vi "Convert VIP License to SBOM Licenses with SPDX Lookup.vi"(6 "Additional Custom Aliases (empty = defaults only)":T1[](array[typedef]), 7 "SPDX License List (JSON) (\"\" = use built-in)":path, 8 "error in (no error)":errorcluster, 11 "VIP License Type in":string) -> (0 "error out":errorcluster, 3 "License(s) out":refnum<class "CycloneDX License.lvclass">[](array[class]))   [LabVIEW 2017, in "VIP SBOM Support.lvlib"]
doc: "Tries to match the VIP license information against the SPDX license types and returns a license with the SPDX license set. If there's no match, returns the license by name."
uses:
  VIP SBOM Support.lvlib
  CycloneDX/CycloneDX License/CycloneDX License.lvclass
  C:/LabVIEW Working Directory/VIPC Software BOM/CycloneDX/CycloneDX JSON/CycloneDX JSON.lvclass
  VIP License Alias.ctl
  c58193e4-58a4-4b31-ba60-9ddf4fa8120d.vi
  <vilib>/JDP Science/JSONtext/Find Item.vi
  <vilib>/JDP Science/JSONtext/String Subset.vi
  <vilib>/JDP Science/JSONtext/Parsing/Parse Full Path or Item Name.vi
  <vilib>/JDP Science/JSONtext/Next JSON Value.vi
  <vilib>/JDP Science/JSONtext/support/Error Cluster From Code.vi
  <vilib>/JDP Science/JSONtext/Offset/Find Item Locations by Path.vi
  <vilib>/JDP Science/JSONtext/JSON text to Variant.vi
  CycloneDX/CycloneDX JSON/CycloneDX JSON.lvclass
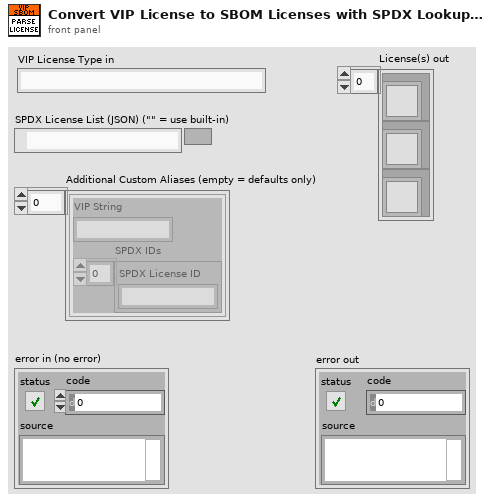
[diagram p1: front panel]
types:
  T1 = typedef "VIP SBOM Support.lvlib/VIP License Alias.ctl" = cluster{"VIP String":string, "SPDX IDs":string[]}
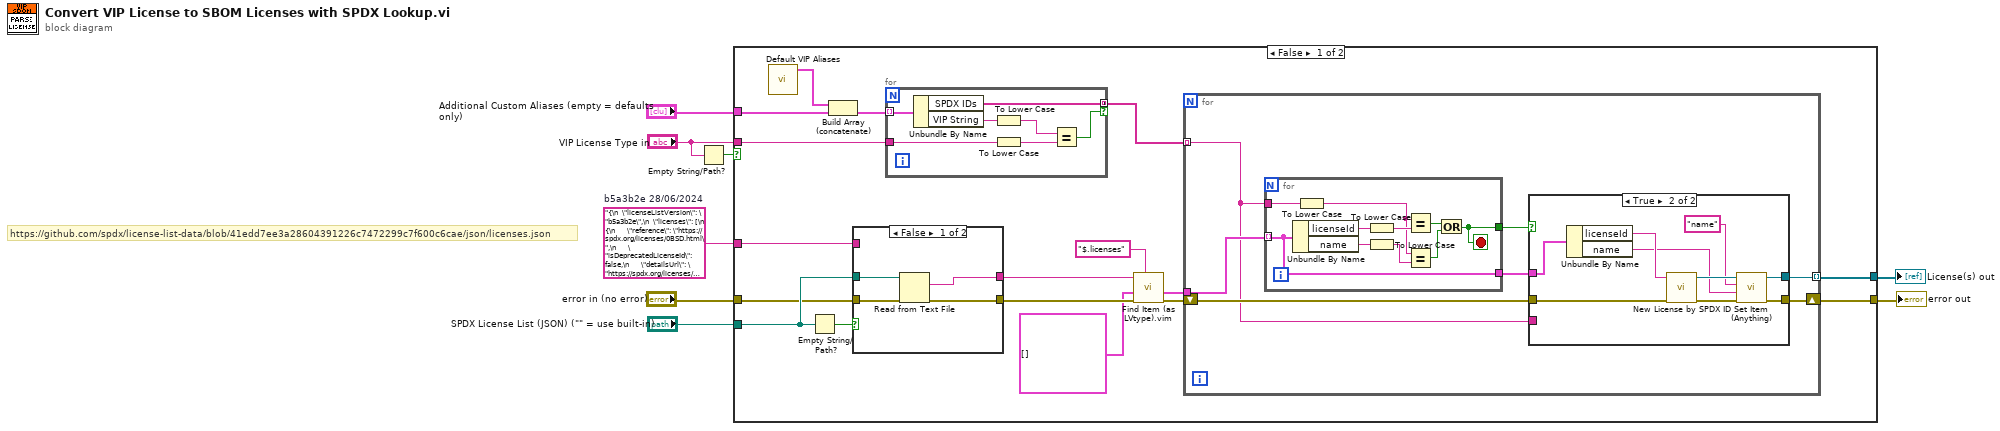
[diagram p0: block diagram]
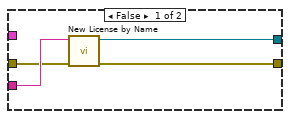
[diagram p3: hidden frame]
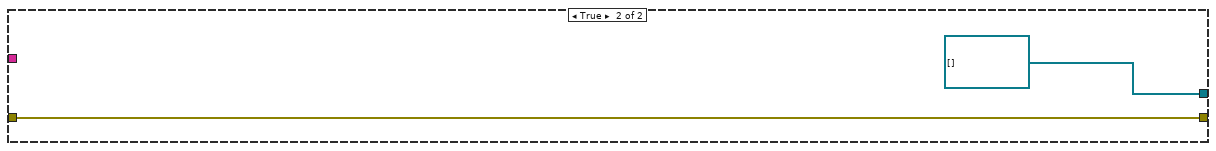
[diagram p4: hidden frame]
diagram:
  w2 = "{\n  \"licenseListVersion\": \"b5a3b2e\",\n  \"licenses\": [\n    {\n      \"reference\": \"https://spdx.org/licenses/0BSD.html\",\n      \"isDeprecatedLicenseId\": false,\n      \"detailsUrl\": \"https://spdx.org/licenses/0BSD.json\",\n      \"referenceNumber\": 430,\n      \"name\": \"BSD Zero Clause License\",\n      \"licenseId\": \"0BSD\",\n      \"seeAlso\": [\n        \"http://landley.net/toybox/license.html\",\n        \"https://opensource.org/licenses/0BSD\"\n      ],\n      \"isOsiApproved\": true\n    },\n    {\n      \"reference\": \"https://spdx.org/licenses/3D-Slicer-1.0.html\",\n      \"isDeprecatedLicenseId\": false,\n      \"detailsUrl\": \"https://spdx.org/licenses/3D-Slicer-1.0.json\",\n      \"referenceNumber\": 448,\n      \"name\": \"3D Slicer License v1.0\",\n      \"licenseId\": \"3D-Slicer-1.0\",\n      \"seeAlso\": [\n        \"https://slicer.org/LICENSE\",\n        \"https://github.com/Slicer/Slicer/blob/main/License.txt\"\n      ],\n      \"isOsiApproved\": false\n    },\n    {\n      \"reference\": \"https://spdx.org/licenses/AAL.html\",\n      \"isDeprecatedLicenseId\": false,\n      \"detailsUrl\": \"https://spdx.org/licenses/AAL.json\",\n      \"referenceNumber\": 515,\n      \"name\": \"Attribution Assurance License\",\n      \"licenseId\": \"AAL\",\n      \"seeAlso\": [\n        \"https://opensource.org/licenses/attribution\"\n      ],\n      \"isOsiApproved\": true\n    },\n    {\n      \"reference\": \"https://spdx.org/licenses/Abstyles.html\",\n      \"isDeprecatedLicenseId\": false,\n      \"detailsUrl\": \"https://spdx.org/licenses/Abstyles.json\",\n      \"referenceNumber\": 561,\n      \"name\": \"Abstyles License\",\n      \"licenseId\": \"Abstyles\",\n      \"seeAlso\": [\n        \"https://fedoraproject.org/wiki/Licensing/Abstyles\"\n      ],\n      \"isOsiApproved\": false\n    },\n    {\n      \"reference\": \"https://spdx.org/licenses/AdaCore-doc.html\",\n      \"isDeprecatedLicenseId\": false,\n      \"detailsUrl\": \"https://spdx.org/licenses/AdaCore-doc.json\",\n      \"referenceNumber\": 641,\n      \"name\": \"AdaCore Doc License\",\n      \"licenseId\": \"AdaCore-doc\",\n      \"seeAlso\": [\n        \"https://github.com/AdaCore/xmlada/blob/master/docs/index.rst\",\n        \"https://github.com/AdaCore/gnatcoll-core/blob/master/docs/index.rst\",\n        \"https://github.com/AdaCore/gnatcoll-db/blob/master/docs/index.rst\"\n      ],\n      \"isOsiApproved\": false\n    },\n    {\n      \"reference\": \"https://spdx.org/licenses/Adobe-2006.html\",\n      \"isDeprecatedLicenseId\": false,\n      \"detailsUrl\": \"https://spdx.org/licenses/Adobe-2006.json\",\n      \"referenceNumber\": 241,\n      \"name\": \"Adobe Systems Incorporated Source Code License Agreement\",\n      \"licenseId\": \"Adobe-2006\",\n      \"seeAlso\": [\n        \"https://fedoraproject.org/wiki/Licensing/AdobeLicense\"\n      ],\n      \"isOsiApproved\": false\n    },\n    {\n      \"reference\": \"https://spdx.org/licenses/Adobe-Display-PostScript.html\",\n      \"isDeprecatedLicenseId\": false,\n      \"detailsUrl\": \"https://spdx.org/licenses/Adobe-Display-PostScript.json\",\n      \"referenceNumber\": 198,\n      \"name\": \"Adobe Display PostScript License\",\n      \"licenseId\": \"Adobe-Display-PostScript\",\n      \"seeAlso\": [\n        \"https://gitlab.freedesktop.org/xorg/xserver/-/blob/master/COPYING?ref_type\\u003dheads#L752\"\n      ],\n      \"isOsiApproved\": false\n    },\n    {\n      \"reference\": \"https://spdx.org/licenses/Adobe-Glyph.html\",\n      \"isDeprecatedLicenseId\": false,\n      \"detailsUrl\": \"https://spdx.org/licenses/Adobe-Glyph.json\",\n      \"referenceNumber\": 506,\n      \"name\": \"Adobe Glyph List License\",\n      \"licenseId\": \"Adobe-Glyph\",\n      \"seeAlso\": [\n        \"https://fedoraproject.org/wiki/Licensing/MIT#AdobeGlyph\"\n      ],\n      \"isOsiApproved\": false\n    },\n    {\n      \"reference\": \"https://spdx.org/licenses/Adobe-Utopia.html\",\n      \"isDeprecatedLicenseId\": false,\n      \"detailsUrl\": \"https://spdx.org/licenses/Adobe-Utopia.json\",\n      \"referenceNumber\": 519,\n      \"name\": \"Adobe Utopia Font License\",\n      \"licenseId\": \"Adobe-Utopia\",\n      \"seeAlso\": [\n        \"https://gitlab.freedesktop.org/xorg/font/adobe-utopia-100dpi/-/blob/master/COPYING?ref_type\\u003dheads\"\n      ],\n      \"isOsiApproved\": false\n    },\n    {\n      \"reference\": \"https://spdx.org/licenses/ADSL.html\",\n      \"isDeprecatedLicenseId\": false,\n      \"detailsUrl\": \"https://spdx.org/licenses/ADSL.json\",\n      \"referenceNumber\": 266,\n      \"name\": \"Amazon Digital Services License\",\n      \"licenseId\": \"ADSL\",\n      \"seeAlso\": [\n        \"https://fedoraproject.org/wiki/Licensing/AmazonDigitalServicesLicense\"\n      ],\n      \"isOsiApproved\": false\n    },\n    {\n      \"reference\": \"https://spdx.org/licenses/AFL-1.1.html\",\n      \"isDeprecatedLicenseId\": false,\n      \"detailsUrl\": \"https://spdx.org/licenses/AFL-1.1.json\",\n      \"referenceNumber\": 120,\n      \"name\": \"Academic Free License v1.1\",\n      \"licenseId\": \"AFL-1.1\",\n      \"seeAlso\": [\n        \"http://opensource.linux-mirror.org/licenses/afl-1.1.txt\",\n        \"http://wayback.archive.org/web/20021004124254/http://www.opensource.org/licenses/academic.php\"\n      ],\n      \"isOsiApproved\": true,\n      \"isFsfLibre\": true\n    },\n    {\n      \"reference\": \"https://spdx.org/licenses/AFL-1.2.html\",\n      \"isDeprecatedLicenseId\": false,\n      \"detailsUrl\": \"https://spdx.org/licenses/AFL-1.2.json\",\n      \"referenceNumber\": 127,\n      \"name\": \"Academic Free License v1.2\",\n      \"licenseId\": \"AFL-1.2\",\n      \"seeAlso\": [\n        \"http://opensource.linux-mirror.org/licenses/afl-1.2.txt\",\n        \"http://wayback.archive.org/web/20021204204652/http://www.opensource.org/licenses/academic.php\"\n      ],\n      \"isOsiApproved\": true,\n      \"isFsfLibre\": true\n    },\n    {\n      \"reference\": \"https://spdx.org/licenses/AFL-2.0.html\",\n      \"isDeprecatedLicenseId\": false,\n      \"detailsUrl\": \"https://spdx.org/licenses/AFL-2.0.json\",\n      \"referenceNumber\": 371,\n      \"name\": \"Academic Free License v2.0\",\n      \"licenseId\": \"AFL-2.0\",\n      \"seeAlso\": [\n        \"http://wayback.archive.org/web/20060924134533/http://www.opensource.org/licenses/afl-2.0.txt\"\n      ],\n      \"isOsiApproved\": true,\n      \"isFsfLibre\": true\n    },\n    {\n      \"reference\": \"https://spdx.org/licenses/AFL-2.1.html\",\n      \"isDeprecatedLicenseId\": false,\n      \"detailsUrl\": \"https://spdx.org/licenses/AFL-2.1.json\",\n      \"referenceNumber\": 355,\n      \"name\": \"Academic Free License v2.1\",\n      \"licenseId\": \"AFL-2.1\",\n      \"seeAlso\": [\n        \"http://opensource.linux-mirror.org/licenses/afl-2.1.txt\"\n      ],\n      \"isOsiApproved\": true,\n      \"isFsfLibre\": true\n    },\n    {\n      \"reference\": \"https://spdx.org/licenses/AFL-3.0.html\",\n      \"isDeprecatedLicenseId\": false,\n      \"detailsUrl\": \"https://spdx.org/licenses/AFL-3.0.json\",\n      \"referenceNumber\": 169,\n      \"name\": \"Academic Free License v3.0\",\n      \"licenseId\": \"AFL-3.0\",\n      \"seeAlso\": [\n        \"http://www.rosenlaw.com/AFL3.0.htm\",\n        \"https://opensource.org/licenses/afl-3.0\"\n      ],\n      \"isOsiApproved\": true,\n      \"isFsfLibre\": true\n    },\n    {\n      \"reference\": \"https://spdx.org/licenses/Afmparse.html\",\n      \"isDeprecatedLicenseId\": false,\n      \"detailsUrl\": \"https://spdx.org/licenses/Afmparse.json\",\n      \"referenceNumber\": 485,\n      \"name\": \"Afmparse License\",\n      \"licenseId\": \"Afmparse\",\n      \"seeAlso\": [\n        \"https://fedoraproject.org/wiki/Licensing/Afmparse\"\n      ],\n      \"isOsiApproved\": false\n    },\n    {\n      \"reference\": \"https://spdx.org/licenses/AGPL-1.0.html\",\n      \"isDeprecatedLicenseId\": true,\n      \"detailsUrl\": \"https://spdx.org/licenses/AGPL-1.0.json\",\n      \"referenceNumber\": 251,\n      \"name\": \"Affero General Public License v1.0\",\n      \"licenseId\": \"AGPL-1.0\",\n      \"seeAlso\": [\n        \"http://www.affero.org/oagpl.html\"\n      ],\n      \"isOsiApproved\": false,\n      \"isFsfLibre\": true\n    },\n    {\n      \"reference\": \"https://spdx.org/licenses/AGPL-1.0-only.html\",\n      \"isDeprecatedLicenseId\": false,\n      \"detailsUrl\": \"https://spdx.org/licenses/AGPL-1.0-only.json\",\n      \"referenceNumber\": 552,\n      \"name\": \"Affero General Public License v1.0 only\",\n      \"licenseId\": \"AGPL-1.0-only\",\n      \"seeAlso\": [\n        \"http://www.affero.org/oagpl.html\"\n      ],\n      \"isOsiApproved\": false\n    },\n    {\n      \"reference\": \"https://spdx.org/licenses/AGPL-1.0-or-later.html\",\n      \"isDeprecatedLicenseId\": false,\n      \"detailsUrl\": \"https://spdx.org/licenses/AGPL-1.0-or-later.json\",\n      \"referenceNumber\": 608,\n      \"name\": \"Affero General Public License v1.0 or later\",\n      \"licenseId\": \"AGPL-1.0-or-later\",\n      \"seeAlso\": [\n        \"http://www.affero.org/oagpl.html\"\n      ],\n      \"isOsiApproved\": false\n    },\n    {\n      \"reference\": \"https://spdx.org/licenses/AGPL-3.0.html\",\n      \"isDeprecatedLicenseId\": true,\n      \"detailsUrl\": \"https://spdx.org/licenses/AGPL-3.0.json\",\n      \"referenceNumber\": 213,\n      \"name\": \"GNU Affero General Public License v3.0\",\n      \"licenseId\": \"AGPL-3.0\",\n      \"seeAlso\": [\n        \"https://www.gnu.org/licenses/agpl.txt\",\n        \"https://opensource.org/licenses/AGPL-3.0\"\n      ],\n      \"isOsiApproved\": true,\n      \"isFsfLibre\": true\n    },\n    {\n      \"reference\": \"https://spdx.org/licenses/AGPL-3.0-only.html\",\n      \"isDeprecatedLicenseId\": false,\n      \"detailsUrl\": \"https://spdx.org/licenses/AGPL-3.0-only.json\",\n      \"referenceNumber\": 2,\n      \"name\": \"GNU Affero General Public License v3.0 only\",\n      \"licenseId\": \"AGPL-3.0-only\",\n      \"seeAlso\": [\n        \"https://www.gnu.org/licenses/agpl.txt\",\n        \"https://opensource.org/licenses/AGPL-3.0\"\n      ],\n      \"isOsiApproved\": true,\n      \"isFsfLibre\": true\n    },\n    {\n      \"reference\": \"https://spdx.org/licenses/AGPL-3.0-or-later.html\",\n      \"isDeprecatedLicenseId\": false,\n      \"detailsUrl\": \"https://spdx.org/licenses/AGPL-3.0-or-later.json\",\n      \"referenceNumber\": 390,\n      \"name\": \"GNU Affero General Public License v3.0 or later\",\n      \"licenseId\": \"AGPL-3.0-or-later\",\n      \"seeAlso\": [\n        \"https://www.gnu.org/licenses/agpl.txt\",\n        \"https://opensource.org/licenses/AGPL-3.0\"\n      ],\n      \"isOsiApproved\": true,\n      \"isFsfLibre\": true\n    },\n    {\n      \"reference\": \"https://spdx.org/licenses/Aladdin.html\",\n      \"isDeprecatedLicenseId\": false,\n      \"detailsUrl\": \"https://spdx.org/licenses/Aladdin.json\",\n      \"referenceNumber\": 272,\n      \"name\": \"Aladdin Free Public License\",\n      \"licenseId\": \"Aladdin\",\n      \"seeAlso\": [\n        \"http://pages.cs.wisc.edu/~ghost/doc/AFPL/6.01/Public.htm\"\n      ],\n      \"isOsiApproved\": false,\n      \"isFsfLibre\": false\n    },\n    {\n      \"reference\": \"https://spdx.org/licenses/AMD-newlib.html\",\n      \"isDeprecatedLicenseId\": false,\n      \"detailsUrl\": \"https://spdx.org/licenses/AMD-newlib.json\",\n      \"referenceNumber\": 536,\n      \"name\": \"AMD newlib License\",\n      \"licenseId\": \"AMD-newlib\",\n      \"seeAlso\": [\n        \"https://sourceware.org/git/?p\\u003dnewlib-cygwin.git;a\\u003dblob;f\\u003dnewlib/libc/sys/a29khif/_close.S;h\\u003d04f52ae00de1dafbd9055ad8d73c5c697a3aae7f;hb\\u003dHEAD\"\n      ],\n      \"isOsiApproved\": false\n    },\n    {\n      \"reference\": \"https://spdx.org/licenses/AMDPLPA.html\",\n      \"isDeprecatedLicenseId\": false,\n      \"detailsUrl\": \"https://spdx.org/licenses/AMDPLPA.json\",\n      \"referenceNumber\": 440,\n      \"name\": \"AMD\\u0027s plpa_map.c License\",\n      \"licenseId\": \"AMDPLPA\",\n      \"seeAlso\": [\n        \"https://fedoraproject.org/wiki/Licensing/AMD_plpa_map_License\"\n      ],\n      \"isOsiApproved\": false\n    },\n    {\n      \"reference\": \"https://spdx.org/licenses/AML.html\",\n      \"isDeprecatedLicenseId\": false,\n      \"detailsUrl\": \"https://spdx.org/licenses/AML.json\",\n      \"referenceNumber\": 361,\n      \"name\": \"Apple MIT License\",\n      \"licenseId\": \"AML\",\n      \"seeAlso\": [\n        \"https://fedoraproject.org/wiki/Licensing/Apple_MIT_License\"\n      ],\n      \"isOsiApproved\": false\n    },\n    {\n      \"reference\": \"https://spdx.org/licenses/AML-glslang.html\",\n      \"isDeprecatedLicenseId\": false,\n      \"detailsUrl\": \"https://spdx.org/licenses/AML-glslang.json\",\n      \"referenceNumber\": 151,\n      \"name\": \"AML glslang variant License\",\n      \"licenseId\": \"AML-glslang\",\n      \"seeAlso\": [\n        \"https://github.com/KhronosGroup/glslang/blob/main/LICENSE.txt#L949\",\n        \"https://docs.omniverse.nvidia.com/install-guide/latest/common/licenses.html\"\n      ],\n      \"isOsiApproved\": false\n    },\n    {\n      \"reference\": \"https://spdx.org/licenses/AMPAS.html\",\n      \"isDeprecatedLicenseId\": false,\n      \"detailsUrl\": \"https://spdx.org/licenses/AMPAS.json\",\n      \"referenceNumber\": 276,\n      \"name\": \"Academy of Motion Picture Arts and Sciences BSD\",\n      \"licenseId\": \"AMPAS\",\n      \"seeAlso\": [\n        \"https://fedoraproject.org/wiki/Licensing/BSD#AMPASBSD\"\n      ],\n      \"isOsiApproved\": false\n    },\n    {\n      \"reference\": \"https://spdx.org/licenses/ANTLR-PD.html\",\n      \"isDeprecatedLicenseId\": false,\n      \"detailsUrl\": \"https://spdx.org/licenses/ANTLR-PD.json\",\n      \"referenceNumber\": 370,\n      \"name\": \"ANTLR Software Rights Notice\",\n      \"licenseId\": \"ANTLR-PD\",\n      \"seeAlso\": [\n        \"http://www.antlr2.org/license.html\"\n      ],\n      \"isOsiApproved\": false\n    },\n    {\n      \"reference\": \"https://spdx.org/licenses/ANTLR-PD-fallback.html\",\n      \"isDeprecatedLicenseId\": false,\n      \"detailsUrl\": \"https://spdx.org/licenses/ANTLR-PD-fallback.json\",\n      \"referenceNumber\": 10,\n      \"name\": \"ANTLR Software Rights Notice with license fallback\",\n      \"licenseId\": \"ANTLR-PD-fallback\",\n      \"seeAlso\": [\n        \"http://www.antlr2.org/license.html\"\n      ],\n      \"isOsiApproved\": false\n    },\n    {\n      \"reference\": \"https://spdx.org/licenses/any-OSI.html\",\n      \"isDeprecatedLicenseId\": false,\n      \"detailsUrl\": \"https://spdx.org/licenses/any-OSI.json\",\n      \"referenceNumber\": 297,\n      \"name\": \"Any OSI License\",\n      \"licenseId\": \"any-OSI\",\n      \"seeAlso\": [\n        \"https://metacpan.org/pod/Exporter::Tidy#LICENSE\"\n      ],\n      \"isOsiApproved\": false\n    },\n    {\n      \"reference\": \"https://spdx.org/licenses/Apache-1.0.html\",\n      \"isDeprecatedLicenseId\": false,\n      \"detailsUrl\": \"https://spdx.org/licenses/Apache-1.0.json\",\n      \"referenceNumber\": 521,\n      \"name\": \"Apache License 1.0\",\n      \"licenseId\": \"Apache-1.0\",\n      \"seeAlso\": [\n        \"http://www.apache.org/licenses/LICENSE-1.0\"\n      ],\n      \"isOsiApproved\": false,\n      \"isFsfLibre\": true\n    },\n    {\n      \"reference\": \"https://spdx.org/licenses/Apache-1.1.html\",\n      \"isDeprecatedLicenseId\": false,\n      \"detailsUrl\": \"https://spdx.org/licenses/Apache-1.1.json\",\n      \"referenceNumber\": 452,\n      \"name\": \"Apache License 1.1\",\n      \"licenseId\": \"Apache-1.1\",\n      \"seeAlso\": [\n        \"http://apache.org/licenses/LICENSE-1.1\",\n        \"https://opensource.org/licenses/Apache-1.1\"\n      ],\n      \"isOsiApproved\": true,\n      \"isFsfLibre\": true\n    },\n    {\n      \"reference\": \"https://spdx.org/licenses/Apache-2.0.html\",\n      \"isDeprecatedLicenseId\": false,\n      \"detailsUrl\": \"https://spdx.org/licenses/Apache-2.0.json\",\n      \"referenceNumber\": 168,\n      \"name\": \"Apache License 2.0\",\n      \"licenseId\": \"Apache-2.0\",\n      \"seeAlso\": [\n        \"https://www.apache.org/licenses/LICENSE-2.0\",\n        \"https://opensource.org/licenses/Apache-2.0\"\n      ],\n      \"isOsiApproved\": true,\n      \"isFsfLibre\": true\n    },\n    {\n      \"reference\": \"https://spdx.org/licenses/APAFML.html\",\n      \"isDeprecatedLicenseId\": false,\n      \"detailsUrl\": \"https://spdx.org/licenses/APAFML.json\",\n      \"referenceNumber\": 456,\n      \"name\": \"Adobe Postscript AFM License\",\n      \"licenseId\": \"APAFML\",\n      \"seeAlso\": [\n        \"https://fedoraproject.org/wiki/Licensing/AdobePostscriptAFM\"\n      ],\n      \"isOsiApproved\": false\n    },\n    {\n      \"reference\": \"https://spdx.org/licenses/APL-1.0.html\",\n      \"isDeprecatedLicenseId\": false,\n      \"detailsUrl\": \"https://spdx.org/licenses/APL-1.0.json\",\n      \"referenceNumber\": 58,\n      \"name\": \"Adaptive Public License 1.0\",\n      \"licenseId\": \"APL-1.0\",\n      \"seeAlso\": [\n        \"https://opensource.org/licenses/APL-1.0\"\n      ],\n      \"isOsiApproved\": true\n    },\n    {\n      \"reference\": \"https://spdx.org/licenses/App-s2p.html\",\n      \"isDeprecatedLicenseId\": false,\n      \"detailsUrl\": \"https://spdx.org/licenses/App-s2p.json\",\n      \"referenceNumber\": 186,\n      \"name\": \"App::s2p License\",\n      \"licenseId\": \"App-s2p\",\n      \"seeAlso\": [\n        \"https://fedoraproject.org/wiki/Licensing/App-s2p\"\n      ],\n      \"isOsiApproved\": false\n    },\n    {\n      \"reference\": \"https://spdx.org/licenses/APSL-1.0.html\",\n      \"isDeprecatedLicenseId\": false,\n      \"detailsUrl\": \"https://spdx.org/licenses/APSL-1.0.json\",\n      \"referenceNumber\": 166,\n      \"name\": \"Apple Public Source License 1.0\",\n      \"licenseId\": \"APSL-1.0\",\n      \"seeAlso\": [\n        \"https://fedoraproject.org/wiki/Licensing/Apple_Public_Source_License_1.0\"\n      ],\n      \"isOsiApproved\": true,\n      \"isFsfLibre\": false\n    },\n    {\n      \"reference\": \"https://spdx.org/licenses/APSL-1.1.html\",\n      \"isDeprecatedLicenseId\": false,\n      \"detailsUrl\": \"https://spdx.org/licenses/APSL-1.1.json\",\n      \"referenceNumber\": 114,\n      \"name\": \"Apple Public Source License 1.1\",\n      \"licenseId\": \"APSL-1.1\",\n      \"seeAlso\": [\n        \"http://www.opensource.apple.com/source/IOSerialFamily/IOSerialFamily-7/APPLE_LICENSE\"\n      ],\n      \"isOsiApproved\": true\n    },\n    {\n      \"reference\": \"https://spdx.org/licenses/APSL-1.2.html\",\n      \"isDeprecatedLicenseId\": false,\n      \"detailsUrl\": \"https://spdx.org/licenses/APSL-1.2.json\",\n      \"referenceNumber\": 393,\n      \"name\": \"Apple Public Source License 1.2\",\n      \"licenseId\": \"APSL-1.2\",\n      \"seeAlso\": [\n        \"http://www.samurajdata.se/opensource/mirror/licenses/apsl.php\"\n      ],\n      \"isOsiApproved\": true\n    },\n    {\n      \"reference\": \"https://spdx.org/licenses/APSL-2.0.html\",\n      \"isDeprecatedLicenseId\": false,\n      \"detailsUrl\": \"https://spdx.org/licenses/APSL-2.0.json\",\n      \"referenceNumber\": 267,\n      \"name\": \"Apple Public Source License 2.0\",\n      \"licenseId\": \"APSL-2.0\",\n      \"seeAlso\": [\n        \"http://www.opensource.apple.com/license/apsl/\"\n      ],\n      \"isOsiApproved\": true,\n      \"isFsfLibre\": true\n    },\n    {\n      \"reference\": \"https://spdx.org/licenses/Arphic-1999.html\",\n      \"isDeprecatedLicenseId\": false,\n      \"detailsUrl\": \"https://spdx.org/licenses/Arphic-1999.json\",\n      \"referenceNumber\": 117,\n      \"name\": \"Arphic Public License\",\n      \"licenseId\": \"Arphic-1999\",\n      \"seeAlso\": [\n        \"http://ftp.gnu.org/gnu/non-gnu/chinese-fonts-truetype/LICENSE\"\n      ],\n      \"isOsiApproved\": false\n    },\n    {\n      \"reference\": \"https://spdx.org/licenses/Artistic-1.0.html\",\n      \"isDeprecatedLicenseId\": false,\n      \"detailsUrl\": \"https://spdx.org/licenses/Artistic-1.0.json\",\n      \"referenceNumber\": 468,\n      \"name\": \"Artistic License 1.0\",\n      \"licenseId\": \"Artistic-1.0\",\n      \"seeAlso\": [\n        \"https://opensource.org/licenses/Artistic-1.0\"\n      ],\n      \"isOsiApproved\": true,\n      \"isFsfLibre\": false\n    },\n    {\n      \"reference\": \"https://spdx.org/licenses/Artistic-1.0-cl8.html\",\n      \"isDeprecatedLicenseId\": false,\n      \"detailsUrl\": \"https://spdx.org/licenses/Artistic-1.0-cl8.json\",\n      \"referenceNumber\": 507,\n      \"name\": \"Artistic License 1.0 w/clause 8\",\n      \"licenseId\": \"Artistic-1.0-cl8\",\n      \"seeAlso\": [\n        \"https://opensource.org/licenses/Artistic-1.0\"\n      ],\n      \"isOsiApproved\": true\n    },\n    {\n      \"reference\": \"https://spdx.org/licenses/Artistic-1.0-Perl.html\",\n      \"isDeprecatedLicenseId\": false,\n      \"detailsUrl\": \"https://spdx.org/licenses/Artistic-1.0-Perl.json\",\n      \"referenceNumber\": 574,\n      \"name\": \"Artistic License 1.0 (Perl)\",\n      \"licenseId\": \"Artistic-1.0-Perl\",\n      \"seeAlso\": [\n        \"http://dev.perl.org/licenses/artistic.html\"\n      ],\n      \"isOsiApproved\": true\n    },\n    {\n      \"reference\": \"https://spdx.org/licenses/Artistic-2.0.html\",\n      \"isDeprecatedLicenseId\": false,\n      \"detailsUrl\": \"https://spdx.org/licenses/Artistic-2.0.json\",\n      \"referenceNumber\": 232,\n      \"name\": \"Artistic License 2.0\",\n      \"licenseId\": \"Artistic-2.0\",\n      \"seeAlso\": [\n        \"http://www.perlfoundation.org/artistic_license_2_0\",\n        \"https://www.perlfoundation.org/artistic-license-20.html\",\n        \"https://opensource.org/licenses/artistic-license-2.0\"\n      ],\n      \"isOsiApproved\": true,\n      \"isFsfLibre\": true\n    },\n    {\n      \"reference\": \"https://spdx.org/licenses/ASWF-Digital-Assets-1.0.html\",\n      \"isDeprecatedLicenseId\": false,\n      \"detailsUrl\": \"https://spdx.org/licenses/ASWF-Digital-Assets-1.0.json\",\n      \"referenceNumber\": 577,\n      \"name\": \"ASWF Digital Assets License version 1.0\",\n      \"licenseId\": \"ASWF-Digital-Assets-1.0\",\n      \"seeAlso\": [\n        \"https://github.com/AcademySoftwareFoundation/foundation/blob/main/digital_assets/aswf_digital_assets_license_v1.0.txt\"\n      ],\n      \"isOsiApproved\": false\n    },\n    {\n      \"reference\": \"https://spdx.org/licenses/ASWF-Digital-Assets-1.1.html\",\n      \"isDeprecatedLicenseId\": false,\n      \"detailsUrl\": \"https://spdx.org/licenses/ASWF-Digital-Assets-1.1.json\",\n      \"referenceNumber\": 508,\n      \"name\": \"ASWF Digital Assets License 1.1\",\n      \"licenseId\": \"ASWF-Digital-Assets-1.1\",\n      \"seeAlso\": [\n        \"https://github.com/AcademySoftwareFoundation/foundation/blob/main/digital_assets/aswf_digital_assets_license_v1.1.txt\"\n      ],\n      \"isOsiApproved\": false\n    },\n    {\n      \"reference\": \"https://spdx.org/licenses/Baekmuk.html\",\n      \"isDeprecatedLicenseId\": false,\n      \"detailsUrl\": \"https://spdx.org/licenses/Baekmuk.json\",\n      \"referenceNumber\": 504,\n      \"name\": \"Baekmuk License\",\n      \"licenseId\": \"Baekmuk\",\n      \"seeAlso\": [\n        \"https://fedoraproject.org/wiki/Licensing:Baekmuk?rd\\u003dLicensing/Baekmuk\"\n      ],\n      \"isOsiApproved\": false\n    },\n    {\n      \"reference\": \"https://spdx.org/licenses/Bahyph.html\",\n      \"isDeprecatedLicenseId\": false,\n      \"detailsUrl\": \"https://spdx.org/licenses/Bahyph.json\",\n      \"referenceNumber\": 604,\n      \"name\": \"Bahyph License\",\n      \"licenseId\": \"Bahyph\",\n      \"seeAlso\": [\n        \"https://fedoraproject.org/wiki/Licensing/Bahyph\"\n      ],\n      \"isOsiApproved\": false\n    },\n    {\n      \"reference\": \"https://spdx.org/licenses/Barr.html\",\n      \"isDeprecatedLicenseId\": false,\n      \"detailsUrl\": \"https://spdx.org/licenses/Barr.json\",\n      \"referenceNumber\": 136,\n      \"name\": \"Barr License\",\n      \"licenseId\": \"Barr\",\n      \"seeAlso\": [\n        \"https://fedoraproject.org/wiki/Licensing/Barr\"\n      ],\n      \"isOsiApproved\": false\n    },\n    {\n      \"reference\": \"https://spdx.org/licenses/bcrypt-Solar-Designer.html\",\n      \"isDeprecatedLicenseId\": false,\n      \"detailsUrl\": \"https://spdx.org/licenses/bcrypt-Solar-Designer.json\",\n      \"referenceNumber\": 402,\n      \"name\": \"bcrypt Solar Designer License\",\n      \"licenseId\": \"bcrypt-Solar-Designer\",\n      \"seeAlso\": [\n        \"https://github.com/bcrypt-ruby/bcrypt-ruby/blob/master/ext/mri/crypt_blowfish.c\"\n      ],\n      \"isOsiApproved\": false\n    },\n    {\n      \"reference\": \"https://spdx.org/licenses/Beerware.html\",\n      \"isDeprecatedLicenseId\": false,\n      \"detailsUrl\": \"https://spdx.org/licenses/Beerware.json\",\n      \"referenceNumber\": 303,\n      \"name\": \"Beerware License\",\n      \"licenseId\": \"Beerware\",\n      \"seeAlso\": [\n        \"https://fedoraproject.org/wiki/Licensing/Beerware\",\n        \"https://people.freebsd.org/~phk/\"\n      ],\n      \"isOsiApproved\": false\n    },\n    {\n      \"reference\": \"https://spdx.org/licenses/Bitstream-Charter.html\",\n      \"isDeprecatedLicenseId\": false,\n      \"detailsUrl\": \"https://spdx.org/licenses/Bitstream-Charter.json\",\n      \"referenceNumber\": 441,\n      \"name\": \"Bitstream Charter Font License\",\n      \"licenseId\": \"Bitstream-Charter\",\n      \"seeAlso\": [\n        \"https://fedoraproject.org/wiki/Licensing/Charter#License_Text\",\n        \"https://raw.githubusercontent.com/blackhole89/notekit/master/data/fonts/Charter%20license.txt\"\n      ],\n      \"isOsiApproved\": false\n    },\n    {\n      \"reference\": \"https://spdx.org/licenses/Bitstream-Vera.html\",\n      \"isDeprecatedLicenseId\": false,\n      \"detailsUrl\": \"https://spdx.org/licenses/Bitstream-Vera.json\",\n      \"referenceNumber\": 579,\n      \"name\": \"Bitstream Vera Font License\",\n      \"licenseId\": \"Bitstream-Vera\",\n      \"seeAlso\": [\n        \"https://web.archive.org/web/20080207013128/http://www.gnome.org/fonts/\",\n        \"https://docubrain.com/sites/default/files/licenses/bitstream-vera.html\"\n      ],\n      \"isOsiApproved\": false\n    },\n    {\n      \"reference\": \"https://spdx.org/licenses/BitTorrent-1.0.html\",\n      \"isDeprecatedLicenseId\": false,\n      \"detailsUrl\": \"https://spdx.org/licenses/BitTorrent-1.0.json\",\n      \"referenceNumber\": 47,\n      \"name\": \"BitTorrent Open Source License v1.0\",\n      \"licenseId\": \"BitTorrent-1.0\",\n      \"seeAlso\": [\n        \"http://sources.gentoo.org/cgi-bin/viewvc.cgi/gentoo-x86/licenses/BitTorrent?r1\\u003d1.1\\u0026r2\\u003d1.1.1.1\\u0026diff_format\\u003ds\"\n      ],\n      \"isOsiApproved\": false\n    },\n    {\n      \"reference\": \"https://spdx.org/licenses/BitTorrent-1.1.html\",\n      \"isDeprecatedLicenseId\": false,\n      \"detailsUrl\": \"https://spdx.org/licenses/BitTorrent-1.1.json\",\n      \"referenceNumber\": 387,\n      \"name\": \"BitTorrent Open Source License v1.1\",\n      \"licenseId\": \"BitTorrent-1.1\",\n      \"seeAlso\": [\n        \"http://directory.fsf.org/wiki/License:BitTorrentOSL1.1\"\n      ],\n      \"isOsiApproved\": false,\n      \"isFsfLibre\": true\n    },\n    {\n      \"reference\": \"https://spdx.org/licenses/blessing.html\",\n      \"isDeprecatedLicenseId\": false,\n      \"detailsUrl\": \"https://spdx.org/licenses/blessing.json\",\n      \"referenceNumber\": 21,\n      \"name\": \"SQLite Blessing\",\n      \"licenseId\": \"blessing\",\n      \"seeAlso\": [\n        \"https://www.sqlite.org/src/artifact/e33a4df7e32d742a?ln\\u003d4-9\",\n        \"https://sqlite.org/src/artifact/df5091916dbb40e6\"\n      ],\n      \"isOsiApproved\": false\n    },\n    {\n      \"reference\": \"https://spdx.org/licenses/BlueOak-1.0.0.html\",\n      \"isDeprecatedLicenseId\": false,\n      \"detailsUrl\": \"https://spdx.org/licenses/BlueOak-1.0.0.json\",\n      \"referenceNumber\": 620,\n      \"name\": \"Blue Oak Model License 1.0.0\",\n      \"licenseId\": \"BlueOak-1.0.0\",\n      \"seeAlso\": [\n        \"https://blueoakcouncil.org/license/1.0.0\"\n      ],\n      \"isOsiApproved\": true\n    },\n    {\n      \"reference\": \"https://spdx.org/licenses/Boehm-GC.html\",\n      \"isDeprecatedLicenseId\": false,\n      \"detailsUrl\": \"https://spdx.org/licenses/Boehm-GC.json\",\n      \"referenceNumber\": 530,\n      \"name\": \"Boehm-Demers-Weiser GC License\",\n      \"licenseId\": \"Boehm-GC\",\n      \"seeAlso\": [\n        \"https://fedoraproject.org/wiki/Licensing:MIT#Another_Minimal_variant_(found_in_libatomic_ops)\",\n        \"https://github.com/uim/libgcroots/blob/master/COPYING\",\n        \"https://github.com/ivmai/libatomic_ops/blob/master/LICENSE\"\n      ],\n      \"isOsiApproved\": false\n    },\n    {\n      \"reference\": \"https://spdx.org/licenses/Borceux.html\",\n      \"isDeprecatedLicenseId\": false,\n      \"detailsUrl\": \"https://spdx.org/licenses/Borceux.json\",\n      \"referenceNumber\": 190,\n      \"name\": \"Borceux license\",\n      \"licenseId\": \"Borceux\",\n      \"seeAlso\": [\n        \"https://fedoraproject.org/wiki/Licensing/Borceux\"\n      ],\n      \"isOsiApproved\": false\n    },\n    {\n      \"reference\": \"https://spdx.org/licenses/Brian-Gladman-2-Clause.html\",\n      \"isDeprecatedLicenseId\": false,\n      \"detailsUrl\": \"https://spdx.org/licenses/Brian-Gladman-2-Clause.json\",\n      \"referenceNumber\": 52,\n      \"name\": \"Brian Gladman 2-Clause License\",\n      \"licenseId\": \"Brian-Gladman-2-Clause\",\n      \"seeAlso\": [\n        \"https://github.com/krb5/krb5/blob/krb5-1.21.2-final/NOTICE#L140-L156\",\n        \"https://web.mit.edu/kerberos/krb5-1.21/doc/mitK5license.html\"\n      ],\n      \"isOsiApproved\": false\n    },\n    {\n      \"reference\": \"https://spdx.org/licenses/Brian-Gladman-3-Clause.html\",\n      \"isDeprecatedLicenseId\": false,\n      \"detailsUrl\": \"https://spdx.org/licenses/Brian-Gladman-3-Clause.json\",\n      \"referenceNumber\": 201,\n      \"name\": \"Brian Gladman 3-Clause License\",\n      \"licenseId\": \"Brian-Gladman-3-Clause\",\n      \"seeAlso\": [\n        \"https://github.com/SWI-Prolog/packages-clib/blob/master/sha1/brg_endian.h\"\n      ],\n      \"isOsiApproved\": false\n    },\n    {\n      \"reference\": \"https://spdx.org/licenses/BSD-1-Clause.html\",\n      \"isDeprecatedLicenseId\": false,\n      \"detailsUrl\": \"https://spdx.org/licenses/BSD-1-Clause.json\",\n      \"referenceNumber\": 404,\n      \"name\": \"BSD 1-Clause License\",\n      \"licenseId\": \"BSD-1-Clause\",\n      \"seeAlso\": [\n        \"https://svnweb.freebsd.org/base/head/include/ifaddrs.h?revision\\u003d326823\"\n      ],\n      \"isOsiApproved\": true\n    },\n    {\n      \"reference\": \"https://spdx.org/licenses/BSD-2-Clause.html\",\n      \"isDeprecatedLicenseId\": false,\n      \"detailsUrl\": \"https://spdx.org/licenses/BSD-2-Clause.json\",\n      \"referenceNumber\": 425,\n      \"name\": \"BSD 2-Clause \\\"Simplified\\\" License\",\n      \"licenseId\": \"BSD-2-Clause\",\n      \"seeAlso\": [\n        \"https://opensource.org/licenses/BSD-2-Clause\"\n      ],\n      \"isOsiApproved\": true,\n      \"isFsfLibre\": true\n    },\n    {\n      \"reference\": \"https://spdx.org/licenses/BSD-2-Clause-Darwin.html\",\n      \"isDeprecatedLicenseId\": false,\n      \"detailsUrl\": \"https://spdx.org/licenses/BSD-2-Clause-Darwin.json\",\n      \"referenceNumber\": 435,\n      \"name\": \"BSD 2-Clause - Ian Darwin variant\",\n      \"licenseId\": \"BSD-2-Clause-Darwin\",\n      \"seeAlso\": [\n        \"https://github.com/file/file/blob/master/COPYING\"\n      ],\n      \"isOsiApproved\": false\n    },\n    {\n      \"reference\": \"https://spdx.org/licenses/BSD-2-Clause-first-lines.html\",\n      \"isDeprecatedLicenseId\": false,\n      \"detailsUrl\": \"https://spdx.org/licenses/BSD-2-Clause-first-lines.json\",\n      \"referenceNumber\": 5,\n      \"name\": \"BSD 2-Clause - first lines requirement\",\n      \"licenseId\": \"BSD-2-Clause-first-lines\",\n      \"seeAlso\": [\n        \"https://github.com/krb5/krb5/blob/krb5-1.21.2-final/NOTICE#L664-L690\",\n        \"https://web.mit.edu/kerberos/krb5-1.21/doc/mitK5license.html\"\n      ],\n      \"isOsiApproved\": false\n    },\n    {\n      \"reference\": \"https://spdx.org/licenses/BSD-2-Clause-FreeBSD.html\",\n      \"isDeprecatedLicenseId\": true,\n      \"detailsUrl\": \"https://spdx.org/licenses/BSD-2-Clause-FreeBSD.json\",\n      \"referenceNumber\": 126,\n      \"name\": \"BSD 2-Clause FreeBSD License\",\n      \"licenseId\": \"BSD-2-Clause-FreeBSD\",\n      \"seeAlso\": [\n        \"http://www.freebsd.org/copyright/freebsd-license.html\"\n      ],\n      \"isOsiApproved\": false,\n      \"isFsfLibre\": true\n    },\n    {\n      \"reference\": \"https://spdx.org/licenses/BSD-2-Clause-NetBSD.html\",\n      \"isDeprecatedLicenseId\": true,\n      \"detailsUrl\": \"https://spdx.org/licenses/BSD-2-Clause-NetBSD.json\",\n      \"referenceNumber\": 446,\n      \"name\": \"BSD 2-Clause NetBSD License\",\n      \"licenseId\": \"BSD-2-Clause-NetBSD\",\n      \"seeAlso\": [\n        \"http://www.netbsd.org/about/redistribution.html#default\"\n      ],\n      \"isOsiApproved\": false,\n      \"isFsfLibre\": true\n    },\n    {\n      \"reference\": \"https://spdx.org/licenses/BSD-2-Clause-Patent.html\",\n      \"isDeprecatedLicenseId\": false,\n      \"detailsUrl\": \"https://spdx.org/licenses/BSD-2-Clause-Patent.json\",\n      \"referenceNumber\": 510,\n      \"name\": \"BSD-2-Clause Plus Patent License\",\n      \"licenseId\": \"BSD-2-Clause-Patent\",\n      \"seeAlso\": [\n        \"https://opensource.org/licenses/BSDplusPatent\"\n      ],\n      \"isOsiApproved\": true\n    },\n    {\n      \"reference\": \"https://spdx.org/licenses/BSD-2-Clause-Views.html\",\n      \"isDeprecatedLicenseId\": false,\n      \"detailsUrl\": \"https://spdx.org/licenses/BSD-2-Clause-Views.json\",\n      \"referenceNumber\": 654,\n      \"name\": \"BSD 2-Clause with views sentence\",\n      \"licenseId\": \"BSD-2-Clause-Views\",\n      \"seeAlso\": [\n        \"http://www.freebsd.org/copyright/freebsd-license.html\",\n        \"https://people.freebsd.org/~ivoras/wine/patch-wine-nvidia.sh\",\n        \"https://github.com/protegeproject/protege/blob/master/license.txt\"\n      ],\n      \"isOsiApproved\": false\n    },\n    {\n      \"reference\": \"https://spdx.org/licenses/BSD-3-Clause.html\",\n      \"isDeprecatedLicenseId\": false,\n      \"detailsUrl\": \"https://spdx.org/licenses/BSD-3-Clause.json\",\n      \"referenceNumber\": 442,\n      \"name\": \"BSD 3-Clause \\\"New\\\" or \\\"Revised\\\" License\",\n      \"licenseId\": \"BSD-3-Clause\",\n      \"seeAlso\": [\n        \"https://opensource.org/licenses/BSD-3-Clause\",\n        \"https://www.eclipse.org/org/documents/edl-v10.php\"\n      ],\n      \"isOsiApproved\": true,\n      \"isFsfLibre\": true\n    },\n    {\n      \"reference\": \"https://spdx.org/licenses/BSD-3-Clause-acpica.html\",\n      \"isDeprecatedLicenseId\": false,\n      \"detailsUrl\": \"https://spdx.org/licenses/BSD-3-Clause-acpica.json\",\n      \"referenceNumber\": 306,\n      \"name\": \"BSD 3-Clause acpica variant\",\n      \"licenseId\": \"BSD-3-Clause-acpica\",\n      \"seeAlso\": [\n        \"https://github.com/acpica/acpica/blob/master/source/common/acfileio.c#L119\"\n      ],\n      \"isOsiApproved\": false\n    },\n    {\n      \"reference\": \"https://spdx.org/licenses/BSD-3-Clause-Attribution.html\",\n      \"isDeprecatedLicenseId\": false,\n      \"detailsUrl\": \"https://spdx.org/licenses/BSD-3-Clause-Attribution.json\",\n      \"referenceNumber\": 39,\n      \"name\": \"BSD with attribution\",\n      \"licenseId\": \"BSD-3-Clause-Attribution\",\n      \"seeAlso\": [\n        \"https://fedoraproject.org/wiki/Licensing/BSD_with_Attribution\"\n      ],\n      \"isOsiApproved\": false\n    },\n    {\n      \"reference\": \"https://spdx.org/licenses/BSD-3-Clause-Clear.html\",\n      \"isDeprecatedLicenseId\": false,\n      \"detailsUrl\": \"https://spdx.org/licenses/BSD-3-Clause-Clear.json\",\n      \"referenceNumber\": 332,\n      \"name\": \"BSD 3-Clause Clear License\",\n      \"licenseId\": \"BSD-3-Clause-Clear\",\n      \"seeAlso\": [\n        \"http://labs.metacarta.com/license-explanation.html#license\"\n      ],\n      \"isOsiApproved\": false,\n      \"isFsfLibre\": true\n    },\n    {\n      \"reference\": \"https://spdx.org/licenses/BSD-3-Clause-flex.html\",\n      \"isDeprecatedLicenseId\": false,\n      \"detailsUrl\": \"https://spdx.org/licenses/BSD-3-Clause-flex.json\",\n      \"referenceNumber\": 135,\n      \"name\": \"BSD 3-Clause Flex variant\",\n      \"licenseId\": \"BSD-3-Clause-flex\",\n      \"seeAlso\": [\n        \"https://github.com/westes/flex/blob/master/COPYING\"\n      ],\n      \"isOsiApproved\": false\n    },\n    {\n      \"reference\": \"https://spdx.org/licenses/BSD-3-Clause-HP.html\",\n      \"isDeprecatedLicenseId\": false,\n      \"detailsUrl\": \"https://spdx.org/licenses/BSD-3-Clause-HP.json\",\n      \"referenceNumber\": 380,\n      \"name\": \"Hewlett-Packard BSD variant license\",\n      \"licenseId\": \"BSD-3-Clause-HP\",\n      \"seeAlso\": [\n        \"https://github.com/zdohnal/hplip/blob/master/COPYING#L939\"\n      ],\n      \"isOsiApproved\": false\n    },\n    {\n      \"reference\": \"https://spdx.org/licenses/BSD-3-Clause-LBNL.html\",\n      \"isDeprecatedLicenseId\": false,\n      \"detailsUrl\": \"https://spdx.org/licenses/BSD-3-Clause-LBNL.json\",\n      \"referenceNumber\": 433,\n      \"name\": \"Lawrence Berkeley National Labs BSD variant license\",\n      \"licenseId\": \"BSD-3-Clause-LBNL\",\n      \"seeAlso\": [\n        \"https://fedoraproject.org/wiki/Licensing/LBNLBSD\"\n      ],\n      \"isOsiApproved\": true\n    },\n    {\n      \"reference\": \"https://spdx.org/licenses/BSD-3-Clause-Modification.html\",\n      \"isDeprecatedLicenseId\": false,\n      \"detailsUrl\": \"https://spdx.org/licenses/BSD-3-Clause-Modification.json\",\n      \"referenceNumber\": 603,\n      \"name\": \"BSD 3-Clause Modification\",\n      \"licenseId\": \"BSD-3-Clause-Modification\",\n      \"seeAlso\": [\n        \"https://fedoraproject.org/wiki/Licensing:BSD#Modification_Variant\"\n      ],\n      \"isOsiApproved\": false\n    },\n    {\n      \"reference\": \"https://spdx.org/licenses/BSD-3-Clause-No-Military-License.html\",\n      \"isDeprecatedLicenseId\": false,\n      \"detailsUrl\": \"https://spdx.org/licenses/BSD-3-Clause-No-Military-License.json\",\n      \"referenceNumber\": 478,\n      \"name\": \"BSD 3-Clause No Military License\",\n      \"licenseId\": \"BSD-3-Clause-No-Military-License\",\n      \"seeAlso\": [\n        \"https://gitlab.syncad.com/hive/dhive/-/blob/master/LICENSE\",\n        \"https://github.com/greymass/swift-eosio/blob/master/LICENSE\"\n      ],\n      \"isOsiApproved\": false\n    },\n    {\n      \"reference\": \"https://spdx.org/licenses/BSD-3-Clause-No-Nuclear-License.html\",\n      \"isDeprecatedLicenseId\": false,\n      \"detailsUrl\": \"https://spdx.org/licenses/BSD-3-Clause-No-Nuclear-License.json\",\n      \"referenceNumber\": 17,\n      \"name\": \"BSD 3-Clause No Nuclear License\",\n      \"licenseId\": \"BSD-3-Clause-No-Nuclear-License\",\n      \"seeAlso\": [\n        \"http://download.oracle.com/otn-pub/java/licenses/bsd.txt\"\n      ],\n      \"isOsiApproved\": false\n    },\n    {\n      \"reference\": \"https://spdx.org/licenses/BSD-3-Clause-No-Nuclear-License-2014.html\",\n      \"isDeprecatedLicenseId\": false,\n      \"detailsUrl\": \"https://spdx.org/licenses/BSD-3-Clause-No-Nuclear-License-2014.json\",\n      \"referenceNumber\": 551,\n      \"name\": \"BSD 3-Clause No Nuclear License 2014\",\n      \"licenseId\": \"BSD-3-Clause-No-Nuclear-License-2014\",\n      \"seeAlso\": [\n        \"https://java.net/projects/javaeetutorial/pages/BerkeleyLicense\"\n      ],\n      \"isOsiApproved\": false\n    },\n    {\n      \"reference\": \"https://spdx.org/licenses/BSD-3-Clause-No-Nuclear-Warranty.html\",\n      \"isDeprecatedLicenseId\": false,\n      \"detailsUrl\": \"https://spdx.org/licenses/BSD-3-Clause-No-Nuclear-Warranty.json\",\n      \"referenceNumber\": 599,\n      \"name\": \"BSD 3-Clause No Nuclear Warranty\",\n      \"licenseId\": \"BSD-3-Clause-No-Nuclear-Warranty\",\n      \"seeAlso\": [\n        \"https://jogamp.org/git/?p\\u003dgluegen.git;a\\u003dblob_plain;f\\u003dLICENSE.txt\"\n      ],\n      \"isOsiApproved\": false\n    },\n    {\n      \"reference\": \"https://spdx.org/licenses/BSD-3-Clause-Open-MPI.html\",\n      \"isDeprecatedLicenseId\": false,\n      \"detailsUrl\": \"https://spdx.org/licenses/BSD-3-Clause-Open-MPI.json\",\n      \"referenceNumber\": 615,\n      \"name\": \"BSD 3-Clause Open MPI variant\",\n      \"licenseId\": \"BSD-3-Clause-Open-MPI\",\n      \"seeAlso\": [\n        \"https://www.open-mpi.org/community/license.php\",\n        \"http://www.netlib.org/lapack/LICENSE.txt\"\n      ],\n      \"isOsiApproved\": false\n    },\n    {\n      \"reference\": \"https://spdx.org/licenses/BSD-3-Clause-Sun.html\",\n      \"isDeprecatedLicenseId\": false,\n      \"detailsUrl\": \"https://spdx.org/licenses/BSD-3-Clause-Sun.json\",\n      \"referenceNumber\": 316,\n      \"name\": \"BSD 3-Clause Sun Microsystems\",\n      \"licenseId\": \"BSD-3-Clause-Sun\",\n      \"seeAlso\": [\n        \"https://github.com/xmlark/msv/blob/b9316e2f2270bc1606952ea4939ec87fbba157f3/xsdlib/src/main/java/com/sun/msv/datatype/regexp/InternalImpl.java\"\n      ],\n      \"isOsiApproved\": false\n    },\n    {\n      \"reference\": \"https://spdx.org/licenses/BSD-4-Clause.html\",\n      \"isDeprecatedLicenseId\": false,\n      \"detailsUrl\": \"https://spdx.org/licenses/BSD-4-Clause.json\",\n      \"referenceNumber\": 652,\n      \"name\": \"BSD 4-Clause \\\"Original\\\" or \\\"Old\\\" License\",\n      \"licenseId\": \"BSD-4-Clause\",\n      \"seeAlso\": [\n        \"http://directory.fsf.org/wiki/License:BSD_4Clause\"\n      ],\n      \"isOsiApproved\": false,\n      \"isFsfLibre\": true\n    },\n    {\n      \"reference\": \"https://spdx.org/licenses/BSD-4-Clause-Shortened.html\",\n      \"isDeprecatedLicenseId\": false,\n      \"detailsUrl\": \"https://spdx.org/licenses/BSD-4-Clause-Shortened.json\",\n      \"referenceNumber\": 216,\n      \"name\": \"BSD 4 Clause Shortened\",\n      \"licenseId\": \"BSD-4-Clause-Shortened\",\n      \"seeAlso\": [\n        \"https://metadata.ftp-master.debian.org/changelogs//main/a/arpwatch/arpwatch_2.1a15-7_copyright\"\n      ],\n      \"isOsiApproved\": false\n    },\n    {\n      \"reference\": \"https://spdx.org/licenses/BSD-4-Clause-UC.html\",\n      \"isDeprecatedLicenseId\": false,\n      \"detailsUrl\": \"https://spdx.org/licenses/BSD-4-Clause-UC.json\",\n      \"referenceNumber\": 291,\n      \"name\": \"BSD-4-Clause (University of California-Specific)\",\n      \"licenseId\": \"BSD-4-Clause-UC\",\n      \"seeAlso\": [\n        \"http://www.freebsd.org/copyright/license.html\"\n      ],\n      \"isOsiApproved\": false\n    },\n    {\n      \"reference\": \"https://spdx.org/licenses/BSD-4.3RENO.html\",\n      \"isDeprecatedLicenseId\": false,\n      \"detailsUrl\": \"https://spdx.org/licenses/BSD-4.3RENO.json\",\n      \"referenceNumber\": 550,\n      \"name\": \"BSD 4.3 RENO License\",\n      \"licenseId\": \"BSD-4.3RENO\",\n      \"seeAlso\": [\n        \"https://sourceware.org/git/?p\\u003dbinutils-gdb.git;a\\u003dblob;f\\u003dlibiberty/strcasecmp.c;h\\u003d131d81c2ce7881fa48c363dc5bf5fb302c61ce0b;hb\\u003dHEAD\",\n        \"https://git.openldap.org/openldap/openldap/-/blob/master/COPYRIGHT#L55-63\"\n      ],\n      \"isOsiApproved\": false\n    },\n    {\n      \"reference\": \"https://spdx.org/licenses/BSD-4.3TAHOE.html\",\n      \"isDeprecatedLicenseId\": false,\n      \"detailsUrl\": \"https://spdx.org/licenses/BSD-4.3TAHOE.json\",\n      \"referenceNumber\": 109,\n      \"name\": \"BSD 4.3 TAHOE License\",\n      \"licenseId\": \"BSD-4.3TAHOE\",\n      \"seeAlso\": [\n        \"https://github.com/389ds/389-ds-base/blob/main/ldap/include/sysexits-compat.h#L15\",\n        \"https://git.savannah.gnu.org/cgit/indent.git/tree/doc/indent.texi?id\\u003da74c6b4ee49397cf330b333da1042bffa60ed14f#n1788\"\n      ],\n      \"isOsiApproved\": false\n    },\n    {\n      \"reference\": \"https://spdx.org/licenses/BSD-Advertising-Acknowledgement.html\",\n      \"isDeprecatedLicenseId\": false,\n      \"detailsUrl\": \"https://spdx.org/licenses/BSD-Advertising-Acknowledgement.json\",\n      \"referenceNumber\": 605,\n      \"name\": \"BSD Advertising Acknowledgement License\",\n      \"licenseId\": \"BSD-Advertising-Acknowledgement\",\n      \"seeAlso\": [\n        \"https://github.com/python-excel/xlrd/blob/master/LICENSE#L33\"\n      ],\n      \"isOsiApproved\": false\n    },\n    {\n      \"reference\": \"https://spdx.org/licenses/BSD-Attribution-HPND-disclaimer.html\",\n      \"isDeprecatedLicenseId\": false,\n      \"detailsUrl\": \"https://spdx.org/licenses/BSD-Attribution-HPND-disclaimer.json\",\n      \"referenceNumber\": 206,\n      \"name\": \"BSD with Attribution and HPND disclaimer\",\n      \"licenseId\": \"BSD-Attribution-HPND-disclaimer\",\n      \"seeAlso\": [\n        \"https://github.com/cyrusimap/cyrus-sasl/blob/master/COPYING\"\n      ],\n      \"isOsiApproved\": false\n    },\n    {\n      \"reference\": \"https://spdx.org/licenses/BSD-Inferno-Nettverk.html\",\n      \"isDeprecatedLicenseId\": false,\n      \"detailsUrl\": \"https://spdx.org/licenses/BSD-Inferno-Nettverk.json\",\n      \"referenceNumber\": 183,\n      \"name\": \"BSD-Inferno-Nettverk\",\n      \"licenseId\": \"BSD-Inferno-Nettverk\",\n      \"seeAlso\": [\n        \"https://www.inet.no/dante/LICENSE\"\n      ],\n      \"isOsiApproved\": false\n    },\n    {\n      \"reference\": \"https://spdx.org/licenses/BSD-Protection.html\",\n      \"isDeprecatedLicenseId\": false,\n      \"detailsUrl\": \"https://spdx.org/licenses/BSD-Protection.json\",\n      \"referenceNumber\": 115,\n      \"name\": \"BSD Protection License\",\n      \"licenseId\": \"BSD-Protection\",\n      \"seeAlso\": [\n        \"https://fedoraproject.org/wiki/Licensing/BSD_Protection_License\"\n      ],\n      \"isOsiApproved\": false\n    },\n    {\n      \"reference\": \"https://spdx.org/licenses/BSD-Source-beginning-file.html\",\n      \"isDeprecatedLicenseId\": false,\n      \"detailsUrl\": \"https://spdx.org/licenses/BSD-Source-beginning-file.json\",\n      \"referenceNumber\": 362,\n      \"name\": \"BSD Source Code Attribution - beginning of file variant\",\n      \"licenseId\": \"BSD-Source-beginning-file\",\n      \"seeAlso\": [\n        \"https://github.com/lattera/freebsd/blob/master/sys/cam/cam.c#L4\"\n      ],\n      \"isOsiApproved\": false\n    },\n    {\n      \"reference\": \"https://spdx.org/licenses/BSD-Source-Code.html\",\n      \"isDeprecatedLicenseId\": false,\n      \"detailsUrl\": \"https://spdx.org/licenses/BSD-Source-Code.json\",\n      \"referenceNumber\": 146,\n      \"name\": \"BSD Source Code Attribution\",\n      \"licenseId\": \"BSD-Source-Code\",\n      \"seeAlso\": [\n        \"https://github.com/robbiehanson/CocoaHTTPServer/blob/master/LICENSE.txt\"\n      ],\n      \"isOsiApproved\": false\n    },\n    {\n      \"reference\": \"https://spdx.org/licenses/BSD-Systemics.html\",\n      \"isDeprecatedLicenseId\": false,\n      \"detailsUrl\": \"https://spdx.org/licenses/BSD-Systemics.json\",\n      \"referenceNumber\": 499,\n      \"name\": \"Systemics BSD variant license\",\n      \"licenseId\": \"BSD-Systemics\",\n      \"seeAlso\": [\n        \"https://metacpan.org/release/DPARIS/Crypt-DES-2.07/source/COPYRIGHT\"\n      ],\n      \"isOsiApproved\": false\n    },\n    {\n      \"reference\": \"https://spdx.org/licenses/BSD-Systemics-W3Works.html\",\n      \"isDeprecatedLicenseId\": false,\n      \"detailsUrl\": \"https://spdx.org/licenses/BSD-Systemics-W3Works.json\",\n      \"referenceNumber\": 299,\n      \"name\": \"Systemics W3Works BSD variant license\",\n      \"licenseId\": \"BSD-Systemics-W3Works\",\n      \"seeAlso\": [\n        \"https://metacpan.org/release/DPARIS/Crypt-Blowfish-2.14/source/COPYRIGHT#L7\"\n      ],\n      \"isOsiApproved\": false\n    },\n    {\n      \"reference\": \"https://spdx.org/licenses/BSL-1.0.html\",\n      \"isDeprecatedLicenseId\": false,\n      \"detailsUrl\": \"https://spdx.org/licenses/BSL-1.0.json\",\n      \"referenceNumber\": 313,\n      \"name\": \"Boost Software License 1.0\",\n      \"licenseId\": \"BSL-1.0\",\n      \"seeAlso\": [\n        \"http://www.boost.org/LICENSE_1_0.txt\",\n        \"https://opensource.org/licenses/BSL-1.0\"\n      ],\n      \"isOsiApproved\": true,\n      \"isFsfLibre\": true\n    },\n    {\n      \"reference\": \"https://spdx.org/licenses/BUSL-1.1.html\",\n      \"isDeprecatedLicenseId\": false,\n      \"detailsUrl\": \"https://spdx.org/licenses/BUSL-1.1.json\",\n      \"referenceNumber\": 558,\n      \"name\": \"Business Source License 1.1\",\n      \"licenseId\": \"BUSL-1.1\",\n      \"seeAlso\": [\n        \"https://mariadb.com/bsl11/\"\n      ],\n      \"isOsiApproved\": false\n    },\n    {\n      \"reference\": \"https://spdx.org/licenses/bzip2-1.0.5.html\",\n      \"isDeprecatedLicenseId\": true,\n      \"detailsUrl\": \"https://spdx.org/licenses/bzip2-1.0.5.json\",\n      \"referenceNumber\": 71,\n      \"name\": \"bzip2 and libbzip2 License v1.0.5\",\n      \"licenseId\": \"bzip2-1.0.5\",\n      \"seeAlso\": [\n        \"https://sourceware.org/bzip2/1.0.5/bzip2-manual-1.0.5.html\",\n        \"http://bzip.org/1.0.5/bzip2-manual-1.0.5.html\"\n      ],\n      \"isOsiApproved\": false\n    },\n    {\n      \"reference\": \"https://spdx.org/licenses/bzip2-1.0.6.html\",\n      \"isDeprecatedLicenseId\": false,\n      \"detailsUrl\": \"https://spdx.org/licenses/bzip2-1.0.6.json\",\n      \"referenceNumber\": 113,\n      \"name\": \"bzip2 and libbzip2 License v1.0.6\",\n      \"licenseId\": \"bzip2-1.0.6\",\n      \"seeAlso\": [\n        \"https://sourceware.org/git/?p\\u003dbzip2.git;a\\u003dblob;f\\u003dLICENSE;hb\\u003dbzip2-1.0.6\",\n        \"http://bzip.org/1.0.5/bzip2-manual-1.0.5.html\",\n        \"https://sourceware.org/cgit/valgrind/tree/mpi/libmpiwrap.c\"\n      ],\n      \"isOsiApproved\": false\n    },\n    {\n      \"reference\": \"https://spdx.org/licenses/C-UDA-1.0.html\",\n      \"isDeprecatedLicenseId\": false,\n      \"detailsUrl\": \"https://spdx.org/licenses/C-UDA-1.0.json\",\n      \"referenceNumber\": 225,\n      \"name\": \"Computational Use of Data Agreement v1.0\",\n      \"licenseId\": \"C-UDA-1.0\",\n      \"seeAlso\": [\n        \"https://github.com/microsoft/Computational-Use-of-Data-Agreement/blob/master/C-UDA-1.0.md\",\n        \"https://cdla.dev/computational-use-of-data-agreement-v1-0/\"\n      ],\n      \"isOsiApproved\": false\n    },\n    {\n      \"reference\": \"https://spdx.org/licenses/CAL-1.0.html\",\n      \"isDeprecatedLicenseId\": false,\n      \"detailsUrl\": \"https://spdx.org/licenses/CAL-1.0.json\",\n      \"referenceNumber\": 658,\n      \"name\": \"Cryptographic Autonomy License 1.0\",\n      \"licenseId\": \"CAL-1.0\",\n      \"seeAlso\": [\n        \"http://cryptographicautonomylicense.com/license-text.html\",\n        \"https://opensource.org/licenses/CAL-1.0\"\n      ],\n      \"isOsiApproved\": true\n    },\n    {\n      \"reference\": \"https://spdx.org/licenses/CAL-1.0-Combined-Work-Exception.html\",\n      \"isDeprecatedLicenseId\": false,\n      \"detailsUrl\": \"https://spdx.org/licenses/CAL-1.0-Combined-Work-Exception.json\",\n      \"referenceNumber\": 269,\n      \"name\": \"Cryptographic Autonomy License 1.0 (Combined Work Exception)\",\n      \"licenseId\": \"CAL-1.0-Combined-Work-Exception\",\n      \"seeAlso\": [\n        \"http://cryptographicautonomylicense.com/license-text.html\",\n        \"https://opensource.org/licenses/CAL-1.0\"\n      ],\n      \"isOsiApproved\": true\n    },\n    {\n      \"reference\": \"https://spdx.org/licenses/Caldera.html\",\n      \"isDeprecatedLicenseId\": false,\n      \"detailsUrl\": \"https://spdx.org/licenses/Caldera.json\",\n      \"referenceNumber\": 321,\n      \"name\": \"Caldera License\",\n      \"licenseId\": \"Caldera\",\n      \"seeAlso\": [\n        \"http://www.lemis.com/grog/UNIX/ancient-source-all.pdf\"\n      ],\n      \"isOsiApproved\": false\n    },\n    {\n      \"reference\": \"https://spdx.org/licenses/Caldera-no-preamble.html\",\n      \"isDeprecatedLicenseId\": false,\n      \"detailsUrl\": \"https://spdx.org/licenses/Caldera-no-preamble.json\",\n      \"referenceNumber\": 245,\n      \"name\": \"Caldera License (without preamble)\",\n      \"licenseId\": \"Caldera-no-preamble\",\n      \"seeAlso\": [\n        \"https://github.com/apache/apr/blob/trunk/LICENSE#L298C6-L298C29\"\n      ],\n      \"isOsiApproved\": false\n    },\n    {\n      \"reference\": \"https://spdx.org/licenses/Catharon.html\",\n      \"isDeprecatedLicenseId\": false,\n      \"detailsUrl\": \"https://spdx.org/licenses/Catharon.json\",\n      \"referenceNumber\": 252,\n      \"name\": \"Catharon License\",\n      \"licenseId\": \"Catharon\",\n      \"seeAlso\": [\n        \"https://github.com/scummvm/scummvm/blob/v2.8.0/LICENSES/CatharonLicense.txt\"\n      ],\n      \"isOsiApproved\": false\n    },\n    {\n      \"reference\": \"https://spdx.org/licenses/CATOSL-1.1.html\",\n      \"isDeprecatedLicenseId\": false,\n      \"detailsUrl\": \"https://spdx.org/licenses/CATOSL-1.1.json\",\n      \"referenceNumber\": 94,\n      \"name\": \"Computer Associates Trusted Open Source License 1.1\",\n      \"licenseId\": \"CATOSL-1.1\",\n      \"seeAlso\": [\n        \"https://opensource.org/licenses/CATOSL-1.1\"\n      ],\n      \"isOsiApproved\": true\n    },\n    {\n      \"reference\": \"https://spdx.org/licenses/CC-BY-1.0.html\",\n      \"isDeprecatedLicenseId\": false,\n      \"detailsUrl\": \"https://spdx.org/licenses/CC-BY-1.0.json\",\n      \"referenceNumber\": 431,\n      \"name\": \"Creative Commons Attribution 1.0 Generic\",\n      \"licenseId\": \"CC-BY-1.0\",\n      \"seeAlso\": [\n        \"https://creativecommons.org/licenses/by/1.0/legalcode\"\n      ],\n      \"isOsiApproved\": false\n    },\n    {\n      \"reference\": \"https://spdx.org/licenses/CC-BY-2.0.html\",\n      \"isDeprecatedLicenseId\": false,\n      \"detailsUrl\": \"https://spdx.org/licenses/CC-BY-2.0.json\",\n      \"referenceNumber\": 237,\n      \"name\": \"Creative Commons Attribution 2.0 Generic\",\n      \"licenseId\": \"CC-BY-2.0\",\n      \"seeAlso\": [\n        \"https://creativecommons.org/licenses/by/2.0/legalcode\"\n      ],\n      \"isOsiApproved\": false\n    },\n    {\n      \"reference\": \"https://spdx.org/licenses/CC-BY-2.5.html\",\n      \"isDeprecatedLicenseId\": false,\n      \"detailsUrl\": \"https://spdx.org/licenses/CC-BY-2.5.json\",\n      \"referenceNumber\": 144,\n      \"name\": \"Creative Commons Attribution 2.5 Generic\",\n      \"licenseId\": \"CC-BY-2.5\",\n      \"seeAlso\": [\n        \"https://creativecommons.org/licenses/by/2.5/legalcode\"\n      ],\n      \"isOsiApproved\": false\n    },\n    {\n      \"reference\": \"https://spdx.org/licenses/CC-BY-2.5-AU.html\",\n      \"isDeprecatedLicenseId\": false,\n      \"detailsUrl\": \"https://spdx.org/licenses/CC-BY-2.5-AU.json\",\n      \"referenceNumber\": 184,\n      \"name\": \"Creative Commons Attribution 2.5 Australia\",\n      \"licenseId\": \"CC-BY-2.5-AU\",\n      \"seeAlso\": [\n        \"https://creativecommons.org/licenses/by/2.5/au/legalcode\"\n      ],\n      \"isOsiApproved\": false\n    },\n    {\n      \"reference\": \"https://spdx.org/licenses/CC-BY-3.0.html\",\n      \"isDeprecatedLicenseId\": false,\n      \"detailsUrl\": \"https://spdx.org/licenses/CC-BY-3.0.json\",\n      \"referenceNumber\": 36,\n      \"name\": \"Creative Commons Attribution 3.0 Unported\",\n      \"licenseId\": \"CC-BY-3.0\",\n      \"seeAlso\": [\n        \"https://creativecommons.org/licenses/by/3.0/legalcode\"\n      ],\n      \"isOsiApproved\": false\n    },\n    {\n      \"reference\": \"https://spdx.org/licenses/CC-BY-3.0-AT.html\",\n      \"isDeprecatedLicenseId\": false,\n      \"detailsUrl\": \"https://spdx.org/licenses/CC-BY-3.0-AT.json\",\n      \"referenceNumber\": 165,\n      \"name\": \"Creative Commons Attribution 3.0 Austria\",\n      \"licenseId\": \"CC-BY-3.0-AT\",\n      \"seeAlso\": [\n        \"https://creativecommons.org/licenses/by/3.0/at/legalcode\"\n      ],\n      \"isOsiApproved\": false\n    },\n    {\n      \"reference\": \"https://spdx.org/licenses/CC-BY-3.0-AU.html\",\n      \"isDeprecatedLicenseId\": false,\n      \"detailsUrl\": \"https://spdx.org/licenses/CC-BY-3.0-AU.json\",\n      \"referenceNumber\": 295,\n      \"name\": \"Creative Commons Attribution 3.0 Australia\",\n      \"licenseId\": \"CC-BY-3.0-AU\",\n      \"seeAlso\": [\n        \"https://creativecommons.org/licenses/by/3.0/au/legalcode\"\n      ],\n      \"isOsiApproved\": false\n    },\n    {\n      \"reference\": \"https://spdx.org/licenses/CC-BY-3.0-DE.html\",\n      \"isDeprecatedLicenseId\": false,\n      \"detailsUrl\": \"https://spdx.org/licenses/CC-BY-3.0-DE.json\",\n      \"referenceNumber\": 638,\n      \"name\": \"Creative Commons Attribution 3.0 Germany\",\n      \"licenseId\": \"CC-BY-3.0-DE\",\n      \"seeAlso\": [\n        \"https://creativecommons.org/licenses/by/3.0/de/legalcode\"\n      ],\n      \"isOsiApproved\": false\n    },\n    {\n      \"reference\": \"https://spdx.org/licenses/CC-BY-3.0-IGO.html\",\n      \"isDeprecatedLicenseId\": false,\n      \"detailsUrl\": \"https://spdx.org/licenses/CC-BY-3.0-IGO.json\",\n      \"referenceNumber\": 317,\n      \"name\": \"Creative Commons Attribution 3.0 IGO\",\n      \"licenseId\": \"CC-BY-3.0-IGO\",\n      \"seeAlso\": [\n        \"https://creativecommons.org/licenses/by/3.0/igo/legalcode\"\n      ],\n      \"isOsiApproved\": false\n    },\n    {\n      \"reference\": \"https://spdx.org/licenses/CC-BY-3.0-NL.html\",\n      \"isDeprecatedLicenseId\": false,\n      \"detailsUrl\": \"https://spdx.org/licenses/CC-BY-3.0-NL.json\",\n      \"referenceNumber\": 121,\n      \"name\": \"Creative Commons Attribution 3.0 Netherlands\",\n      \"licenseId\": \"CC-BY-3.0-NL\",\n      \"seeAlso\": [\n        \"https://creativecommons.org/licenses/by/3.0/nl/legalcode\"\n      ],\n      \"isOsiApproved\": false\n    },\n    {\n      \"reference\": \"https://spdx.org/licenses/CC-BY-3.0-US.html\",\n      \"isDeprecatedLicenseId\": false,\n      \"detailsUrl\": \"https://spdx.org/licenses/CC-BY-3.0-US.json\",\n      \"referenceNumber\": 130,\n      \"name\": \"Creative Commons Attribution 3.0 United States\",\n      \"licenseId\": \"CC-BY-3.0-US\",\n      \"seeAlso\": [\n        \"https://creativecommons.org/licenses/by/3.0/us/legalcode\"\n      ],\n      \"isOsiApproved\": false\n    },\n    {\n      \"reference\": \"https://spdx.org/licenses/CC-BY-4.0.html\",\n      \"isDeprecatedLicenseId\": false,\n      \"detailsUrl\": \"https://spdx.org/licenses/CC-BY-4.0.json\",\n      \"referenceNumber\": 443,\n      \"name\": \"Creative Commons Attribution 4.0 International\",\n      \"licenseId\": \"CC-BY-4.0\",\n      \"seeAlso\": [\n        \"https://creativecommons.org/licenses/by/4.0/legalcode\"\n      ],\n      \"isOsiApproved\": false,\n      \"isFsfLibre\": true\n    },\n    {\n      \"reference\": \"https://spdx.org/licenses/CC-BY-NC-1.0.html\",\n      \"isDeprecatedLicenseId\": false,\n      \"detailsUrl\": \"https://spdx.org/licenses/CC-BY-NC-1.0.json\",\n      \"referenceNumber\": 644,\n      \"name\": \"Creative Commons Attribution Non Commercial 1.0 Generic\",\n      \"licenseId\": \"CC-BY-NC-1.0\",\n      \"seeAlso\": [\n        \"https://creativecommons.org/licenses/by-nc/1.0/legalcode\"\n      ],\n      \"isOsiApproved\": false,\n      \"isFsfLibre\": false\n    },\n    {\n      \"reference\": \"https://spdx.org/licenses/CC-BY-NC-2.0.html\",\n      \"isDeprecatedLicenseId\": false,\n      \"detailsUrl\": \"https://spdx.org/licenses/CC-BY-NC-2.0.json\",\n      \"referenceNumber\": 242,\n      \"name\": \"Creative Commons Attribution Non Commercial 2.0 Generic\",\n      \"licenseId\": \"CC-BY-NC-2.0\",\n      \"seeAlso\": [\n        \"https://creativecommons.org/licenses/by-nc/2.0/legalcode\"\n      ],\n      \"isOsiApproved\": false,\n      \"isFsfLibre\": false\n    },\n    {\n      \"reference\": \"https://spdx.org/licenses/CC-BY-NC-2.5.html\",\n      \"isDeprecatedLicenseId\": false,\n      \"detailsUrl\": \"https://spdx.org/licenses/CC-BY-NC-2.5.json\",\n      \"referenceNumber\": 349,\n      \"name\": \"Creative Commons Attribution Non Commercial 2.5 Generic\",\n      \"licenseId\": \"CC-BY-NC-2.5\",\n      \"seeAlso\": [\n        \"https://creativecommons.org/licenses/by-nc/2.5/legalcode\"\n      ],\n      \"isOsiApproved\": false,\n      \"isFsfLibre\": false\n    },\n    {\n      \"reference\": \"https://spdx.org/licenses/CC-BY-NC-3.0.html\",\n      \"isDeprecatedLicenseId\": false,\n      \"detailsUrl\": \"https://spdx.org/licenses/CC-BY-NC-3.0.json\",\n      \"referenceNumber\": 152,\n      \"name\": \"Creative Commons Attribution Non Commercial 3.0 Unported\",\n      \"licenseId\": \"CC-BY-NC-3.0\",\n      \"seeAlso\": [\n        \"https://creativecommons.org/licenses/by-nc/3.0/legalcode\"\n      ],\n      \"isOsiApproved\": false,\n      \"isFsfLibre\": false\n    },\n    {\n      \"reference\": \"https://spdx.org/licenses/CC-BY-NC-3.0-DE.html\",\n      \"isDeprecatedLicenseId\": false,\n      \"detailsUrl\": \"https://spdx.org/licenses/CC-BY-NC-3.0-DE.json\",\n      \"referenceNumber\": 263,\n      \"name\": \"Creative Commons Attribution Non Commercial 3.0 Germany\",\n      \"licenseId\": \"CC-BY-NC-3.0-DE\",\n      \"seeAlso\": [\n        \"https://creativecommons.org/licenses/by-nc/3.0/de/legalcode\"\n      ],\n      \"isOsiApproved\": false\n    },\n    {\n      \"reference\": \"https://spdx.org/licenses/CC-BY-NC-4.0.html\",\n      \"isDeprecatedLicenseId\": false,\n      \"detailsUrl\": \"https://spdx.org/licenses/CC-BY-NC-4.0.json\",\n      \"referenceNumber\": 397,\n      \"name\": \"Creative Commons Attribution Non Commercial 4.0 International\",\n      \"licenseId\": \"CC-BY-NC-4.0\",\n      \"seeAlso\": [\n        \"https://creativecommons.org/licenses/by-nc/4.0/legalcode\"\n      ],\n      \"isOsiApproved\": false,\n      \"isFsfLibre\": false\n    },\n    {\n      \"reference\": \"https://spdx.org/licenses/CC-BY-NC-ND-1.0.html\",\n      \"isDeprecatedLicenseId\": false,\n      \"detailsUrl\": \"https://spdx.org/licenses/CC-BY-NC-ND-1.0.json\",\n      \"referenceNumber\": 417,\n      \"name\": \"Creative Commons Attribution Non Commercial No Derivatives 1.0 Generic\",\n      \"licenseId\": \"CC-BY-NC-ND-1.0\",\n      \"seeAlso\": [\n        \"https://creativecommons.org/licenses/by-nd-nc/1.0/legalcode\"\n      ],\n      \"isOsiApproved\": false\n    },\n    {\n      \"reference\": \"https://spdx.org/licenses/CC-BY-NC-ND-2.0.html\",\n      \"isDeprecatedLicenseId\": false,\n      \"detailsUrl\": \"https://spdx.org/licenses/CC-BY-NC-ND-2.0.json\",\n      \"referenceNumber\": 513,\n      \"name\": \"Creative Commons Attribution Non Commercial No Derivatives 2.0 Generic\",\n      \"licenseId\": \"CC-BY-NC-ND-2.0\",\n      \"seeAlso\": [\n        \"https://creativecommons.org/licenses/by-nc-nd/2.0/legalcode\"\n      ],\n      \"isOsiApproved\": false\n    },\n    {\n      \"reference\": \"https://spdx.org/licenses/CC-BY-NC-ND-2.5.html\",\n      \"isDeprecatedLicenseId\": false,\n      \"detailsUrl\": \"https://spdx.org/licenses/CC-BY-NC-ND-2.5.json\",\n      \"referenceNumber\": 233,\n      \"name\": \"Creative Commons Attribution Non Commercial No Derivatives 2.5 Generic\",\n      \"licenseId\": \"CC-BY-NC-ND-2.5\",\n      \"seeAlso\": [\n        \"https://creativecommons.org/licenses/by-nc-nd/2.5/legalcode\"\n      ],\n      \"isOsiApproved\": false\n    },\n    {\n      \"reference\": \"https://spdx.org/licenses/CC-BY-NC-ND-3.0.html\",\n      \"isDeprecatedLicenseId\": false,\n      \"detailsUrl\": \"https://spdx.org/licenses/CC-BY-NC-ND-3.0.json\",\n      \"referenceNumber\": 556,\n      \"name\": \"Creative Commons Attribution Non Commercial No Derivatives 3.0 Unported\",\n      \"licenseId\": \"CC-BY-NC-ND-3.0\",\n      \"seeAlso\": [\n        \"https://creativecommons.org/licenses/by-nc-nd/3.0/legalcode\"\n      ],\n      \"isOsiApproved\": false\n    },\n    {\n      \"reference\": \"https://spdx.org/licenses/CC-BY-NC-ND-3.0-DE.html\",\n      \"isDeprecatedLicenseId\": false,\n      \"detailsUrl\": \"https://spdx.org/licenses/CC-BY-NC-ND-3.0-DE.json\",\n      \"referenceNumber\": 569,\n      \"name\": \"Creative Commons Attribution Non Commercial No Derivatives 3.0 Germany\",\n      \"licenseId\": \"CC-BY-NC-ND-3.0-DE\",\n      \"seeAlso\": [\n        \"https://creativecommons.org/licenses/by-nc-nd/3.0/de/legalcode\"\n      ],\n      \"isOsiApproved\": false\n    },\n    {\n      \"reference\": \"https://spdx.org/licenses/CC-BY-NC-ND-3.0-IGO.html\",\n      \"isDeprecatedLicenseId\": false,\n      \"detailsUrl\": \"https://spdx.org/licenses/CC-BY-NC-ND-3.0-IGO.json\",\n      \"referenceNumber\": 607,\n      \"name\": \"Creative Commons Attribution Non Commercial No Derivatives 3.0 IGO\",\n      \"licenseId\": \"CC-BY-NC-ND-3.0-IGO\",\n      \"seeAlso\": [\n        \"https://creativecommons.org/licenses/by-nc-nd/3.0/igo/legalcode\"\n      ],\n      \"isOsiApproved\": false\n    },\n    {\n      \"reference\": \"https://spdx.org/licenses/CC-BY-NC-ND-4.0.html\",\n      \"isDeprecatedLicenseId\": false,\n      \"detailsUrl\": \"https://spdx.org/licenses/CC-BY-NC-ND-4.0.json\",\n      \"referenceNumber\": 334,\n      \"name\": \"Creative Commons Attribution Non Commercial No Derivatives 4.0 International\",\n      \"licenseId\": \"CC-BY-NC-ND-4.0\",\n      \"seeAlso\": [\n        \"https://creativecommons.org/licenses/by-nc-nd/4.0/legalcode\"\n      ],\n      \"isOsiApproved\": false\n    },\n    {\n      \"reference\": \"https://spdx.org/licenses/CC-BY-NC-SA-1.0.html\",\n      \"isDeprecatedLicenseId\": false,\n      \"detailsUrl\": \"https://spdx.org/licenses/CC-BY-NC-SA-1.0.json\",\n      \"referenceNumber\": 42,\n      \"name\": \"Creative Commons Attribution Non Commercial Share Alike 1.0 Generic\",\n      \"licenseId\": \"CC-BY-NC-SA-1.0\",\n      \"seeAlso\": [\n        \"https://creativecommons.org/licenses/by-nc-sa/1.0/legalcode\"\n      ],\n      \"isOsiApproved\": false\n    },\n    {\n      \"reference\": \"https://spdx.org/licenses/CC-BY-NC-SA-2.0.html\",\n      \"isDeprecatedLicenseId\": false,\n      \"detailsUrl\": \"https://spdx.org/licenses/CC-BY-NC-SA-2.0.json\",\n      \"referenceNumber\": 420,\n      \"name\": \"Creative Commons Attribution Non Commercial Share Alike 2.0 Generic\",\n      \"licenseId\": \"CC-BY-NC-SA-2.0\",\n      \"seeAlso\": [\n        \"https://creativecommons.org/licenses/by-nc-sa/2.0/legalcode\"\n      ],\n      \"isOsiApproved\": false\n    },\n    {\n      \"reference\": \"https://spdx.org/licenses/CC-BY-NC-SA-2.0-DE.html\",\n      \"isDeprecatedLicenseId\": false,\n      \"detailsUrl\": \"https://spdx.org/licenses/CC-BY-NC-SA-2.0-DE.json\",\n      \"referenceNumber\": 381,\n      \"name\": \"Creative Commons Attribution Non Commercial Share Alike 2.0 Germany\",\n      \"licenseId\": \"CC-BY-NC-SA-2.0-DE\",\n      \"seeAlso\": [\n        \"https://creativecommons.org/licenses/by-nc-sa/2.0/de/legalcode\"\n      ],\n      \"isOsiApproved\": false\n    },\n    {\n      \"reference\": \"https://spdx.org/licenses/CC-BY-NC-SA-2.0-FR.html\",\n      \"isDeprecatedLicenseId\": false,\n      \"detailsUrl\": \"https://spdx.org/licenses/CC-BY-NC-SA-2.0-FR.json\",\n      \"referenceNumber\": 226,\n      \"name\": \"Creative Commons Attribution-NonCommercial-ShareAlike 2.0 France\",\n      \"licenseId\": \"CC-BY-NC-SA-2.0-FR\",\n      \"seeAlso\": [\n        \"https://creativecommons.org/licenses/by-nc-sa/2.0/fr/legalcode\"\n      ],\n      \"isOsiApproved\": false\n    },\n    {\n      \"reference\": \"https://spdx.org/licenses/CC-BY-NC-SA-2.0-UK.html\",\n      \"isDeprecatedLicenseId\": false,\n      \"detailsUrl\": \"https://spdx.org/licenses/CC-BY-NC-SA-2.0-UK.json\",\n      \"referenceNumber\": 590,\n      \"name\": \"Creative Commons Attribution Non Commercial Share Alike 2.0 England and Wales\",\n      \"licenseId\": \"CC-BY-NC-SA-2.0-UK\",\n      \"seeAlso\": [\n        \"https://creativecommons.org/licenses/by-nc-sa/2.0/uk/legalcode\"\n      ],\n      \"isOsiApproved\": false\n    },\n    {\n      \"reference\": \"https://spdx.org/licenses/CC-BY-NC-SA-2.5.html\",\n      \"isDeprecatedLicenseId\": false,\n      \"detailsUrl\": \"https://spdx.org/licenses/CC-BY-NC-SA-2.5.json\",\n      \"referenceNumber\": 66,\n      \"name\": \"Creative Commons Attribution Non Commercial Share Alike 2.5 Generic\",\n      \"licenseId\": \"CC-BY-NC-SA-2.5\",\n      \"seeAlso\": [\n        \"https://creativecommons.org/licenses/by-nc-sa/2.5/legalcode\"\n      ],\n      \"isOsiApproved\": false\n    },\n    {\n      \"reference\": \"https://spdx.org/licenses/CC-BY-NC-SA-3.0.html\",\n      \"isDeprecatedLicenseId\": false,\n      \"detailsUrl\": \"https://spdx.org/licenses/CC-BY-NC-SA-3.0.json\",\n      \"referenceNumber\": 374,\n      \"name\": \"Creative Commons Attribution Non Commercial Share Alike 3.0 Unported\",\n      \"licenseId\": \"CC-BY-NC-SA-3.0\",\n      \"seeAlso\": [\n        \"https://creativecommons.org/licenses/by-nc-sa/3.0/legalcode\"\n      ],\n      \"isOsiApproved\": false\n    },\n    {\n      \"reference\": \"https://spdx.org/licenses/CC-BY-NC-SA-3.0-DE.html\",\n      \"isDeprecatedLicenseId\": false,\n      \"detailsUrl\": \"https://spdx.org/licenses/CC-BY-NC-SA-3.0-DE.json\",\n      \"referenceNumber\": 172,\n      \"name\": \"Creative Commons Attribution Non Commercial Share Alike 3.0 Germany\",\n      \"licenseId\": \"CC-BY-NC-SA-3.0-DE\",\n      \"seeAlso\": [\n        \"https://creativecommons.org/licenses/by-nc-sa/3.0/de/legalcode\"\n      ],\n      \"isOsiApproved\": false\n    },\n    {\n      \"reference\": \"https://spdx.org/licenses/CC-BY-NC-SA-3.0-IGO.html\",\n      \"isDeprecatedLicenseId\": false,\n      \"detailsUrl\": \"https://spdx.org/licenses/CC-BY-NC-SA-3.0-IGO.json\",\n      \"referenceNumber\": 154,\n      \"name\": \"Creative Commons Attribution Non Commercial Share Alike 3.0 IGO\",\n      \"licenseId\": \"CC-BY-NC-SA-3.0-IGO\",\n      \"seeAlso\": [\n        \"https://creativecommons.org/licenses/by-nc-sa/3.0/igo/legalcode\"\n      ],\n      \"isOsiApproved\": false\n    },\n    {\n      \"reference\": \"https://spdx.org/licenses/CC-BY-NC-SA-4.0.html\",\n      \"isDeprecatedLicenseId\": false,\n      \"detailsUrl\": \"https://spdx.org/licenses/CC-BY-NC-SA-4.0.json\",\n      \"referenceNumber\": 142,\n      \"name\": \"Creative Commons Attribution Non Commercial Share Alike 4.0 International\",\n      \"licenseId\": \"CC-BY-NC-SA-4.0\",\n      \"seeAlso\": [\n        \"https://creativecommons.org/licenses/by-nc-sa/4.0/legalcode\"\n      ],\n      \"isOsiApproved\": false\n    },\n    {\n      \"reference\": \"https://spdx.org/licenses/CC-BY-ND-1.0.html\",\n      \"isDeprecatedLicenseId\": false,\n      \"detailsUrl\": \"https://spdx.org/licenses/CC-BY-ND-1.0.json\",\n      \"referenceNumber\": 98,\n      \"name\": \"Creative Commons Attribution No Derivatives 1.0 Generic\",\n      \"licenseId\": \"CC-BY-ND-1.0\",\n      \"seeAlso\": [\n        \"https://creativecommons.org/licenses/by-nd/1.0/legalcode\"\n      ],\n      \"isOsiApproved\": false,\n      \"isFsfLibre\": false\n    },\n    {\n      \"reference\": \"https://spdx.org/licenses/CC-BY-ND-2.0.html\",\n      \"isDeprecatedLicenseId\": false,\n      \"detailsUrl\": \"https://spdx.org/licenses/CC-BY-ND-2.0.json\",\n      \"referenceNumber\": 7,\n      \"name\": \"Creative Commons Attribution No Derivatives 2.0 Generic\",\n      \"licenseId\": \"CC-BY-ND-2.0\",\n      \"seeAlso\": [\n        \"https://creativecommons.org/licenses/by-nd/2.0/legalcode\"\n      ],\n      \"isOsiApproved\": false,\n      \"isFsfLibre\": false\n    },\n    {\n      \"reference\": \"https://spdx.org/licenses/CC-BY-ND-2.5.html\",\n      \"isDeprecatedLicenseId\": false,\n      \"detailsUrl\": \"https://spdx.org/licenses/CC-BY-ND-2.5.json\",\n      \"referenceNumber\": 228,\n      \"name\": \"Creative Commons Attribution No Derivatives 2.5 Generic\",\n      \"licenseId\": \"CC-BY-ND-2.5\",\n      \"seeAlso\": [\n        \"https://creativecommons.org/licenses/by-nd/2.5/legalcode\"\n      ],\n      \"isOsiApproved\": false,\n      \"isFsfLibre\": false\n    },\n    {\n      \"reference\": \"https://spdx.org/licenses/CC-BY-ND-3.0.html\",\n      \"isDeprecatedLicenseId\": false,\n      \"detailsUrl\": \"https://spdx.org/licenses/CC-BY-ND-3.0.json\",\n      \"referenceNumber\": 258,\n      \"name\": \"Creative Commons Attribution No Derivatives 3.0 Unported\",\n      \"licenseId\": \"CC-BY-ND-3.0\",\n      \"seeAlso\": [\n        \"https://creativecommons.org/licenses/by-nd/3.0/legalcode\"\n      ],\n      \"isOsiApproved\": false,\n      \"isFsfLibre\": false\n    },\n    {\n      \"reference\": \"https://spdx.org/licenses/CC-BY-ND-3.0-DE.html\",\n      \"isDeprecatedLicenseId\": false,\n      \"detailsUrl\": \"https://spdx.org/licenses/CC-BY-ND-3.0-DE.json\",\n      \"referenceNumber\": 222,\n      \"name\": \"Creative Commons Attribution No Derivatives 3.0 Germany\",\n      \"licenseId\": \"CC-BY-ND-3.0-DE\",\n      \"seeAlso\": [\n        \"https://creativecommons.org/licenses/by-nd/3.0/de/legalcode\"\n      ],\n      \"isOsiApproved\": false\n    },\n    {\n      \"reference\": \"https://spdx.org/licenses/CC-BY-ND-4.0.html\",\n      \"isDeprecatedLicenseId\": false,\n      \"detailsUrl\": \"https://spdx.org/licenses/CC-BY-ND-4.0.json\",\n      \"referenceNumber\": 125,\n      \"name\": \"Creative Commons Attribution No Derivatives 4.0 International\",\n      \"licenseId\": \"CC-BY-ND-4.0\",\n      \"seeAlso\": [\n        \"https://creativecommons.org/licenses/by-nd/4.0/legalcode\"\n      ],\n      \"isOsiApproved\": false,\n      \"isFsfLibre\": false\n    },\n    {\n      \"reference\": \"https://spdx.org/licenses/CC-BY-SA-1.0.html\",\n      \"isDeprecatedLicenseId\": false,\n      \"detailsUrl\": \"https://spdx.org/licenses/CC-BY-SA-1.0.json\",\n      \"referenceNumber\": 254,\n      \"name\": \"Creative Commons Attribution Share Alike 1.0 Generic\",\n      \"licenseId\": \"CC-BY-SA-1.0\",\n      \"seeAlso\": [\n        \"https://creativecommons.org/licenses/by-sa/1.0/legalcode\"\n      ],\n      \"isOsiApproved\": false\n    },\n    {\n      \"reference\": \"https://spdx.org/licenses/CC-BY-SA-2.0.html\",\n      \"isDeprecatedLicenseId\": false,\n      \"detailsUrl\": \"https://spdx.org/licenses/CC-BY-SA-2.0.json\",\n      \"referenceNumber\": 192,\n      \"name\": \"Creative Commons Attribution Share Alike 2.0 Generic\",\n      \"licenseId\": \"CC-BY-SA-2.0\",\n      \"seeAlso\": [\n        \"https://creativecommons.org/licenses/by-sa/2.0/legalcode\"\n      ],\n      \"isOsiApproved\": false\n    },\n    {\n      \"reference\": \"https://spdx.org/licenses/CC-BY-SA-2.0-UK.html\",\n      \"isDeprecatedLicenseId\": false,\n      \"detailsUrl\": \"https://spdx.org/licenses/CC-BY-SA-2.0-UK.json\",\n      \"referenceNumber\": 134,\n      \"name\": \"Creative Commons Attribution Share Alike 2.0 England and Wales\",\n      \"licenseId\": \"CC-BY-SA-2.0-UK\",\n      \"seeAlso\": [\n        \"https://creativecommons.org/licenses/by-sa/2.0/uk/legalcode\"\n      ],\n      \"isOsiApproved\": false\n    },\n    {\n      \"reference\": \"https://spdx.org/licenses/CC-BY-SA-2.1-JP.html\",\n      \"isDeprecatedLicenseId\": false,\n      \"detailsUrl\": \"https://spdx.org/licenses/CC-BY-SA-2.1-JP.json\",\n      \"referenceNumber\": 461,\n      \"name\": \"Creative Commons Attribution Share Alike 2.1 Japan\",\n      \"licenseId\": \"CC-BY-SA-2.1-JP\",\n      \"seeAlso\": [\n        \"https://creativecommons.org/licenses/by-sa/2.1/jp/legalcode\"\n      ],\n      \"isOsiApproved\": false\n    },\n    {\n      \"reference\": \"https://spdx.org/licenses/CC-BY-SA-2.5.html\",\n      \"isDeprecatedLicenseId\": false,\n      \"detailsUrl\": \"https://spdx.org/licenses/CC-BY-SA-2.5.json\",\n      \"referenceNumber\": 503,\n      \"name\": \"Creative Commons Attribution Share Alike 2.5 Generic\",\n      \"licenseId\": \"CC-BY-SA-2.5\",\n      \"seeAlso\": [\n        \"https://creativecommons.org/licenses/by-sa/2.5/legalcode\"\n      ],\n      \"isOsiApproved\": false\n    },\n    {\n      \"reference\": \"https://spdx.org/licenses/CC-BY-SA-3.0.html\",\n      \"isDeprecatedLicenseId\": false,\n      \"detailsUrl\": \"https://spdx.org/licenses/CC-BY-SA-3.0.json\",\n      \"referenceNumber\": 26,\n      \"name\": \"Creative Commons Attribution Share Alike 3.0 Unported\",\n      \"licenseId\": \"CC-BY-SA-3.0\",\n      \"seeAlso\": [\n        \"https://creativecommons.org/licenses/by-sa/3.0/legalcode\"\n      ],\n      \"isOsiApproved\": false\n    },\n    {\n      \"reference\": \"https://spdx.org/licenses/CC-BY-SA-3.0-AT.html\",\n      \"isDeprecatedLicenseId\": false,\n      \"detailsUrl\": \"https://spdx.org/licenses/CC-BY-SA-3.0-AT.json\",\n      \"referenceNumber\": 549,\n      \"name\": \"Creative Commons Attribution Share Alike 3.0 Austria\",\n      \"licenseId\": \"CC-BY-SA-3.0-AT\",\n      \"seeAlso\": [\n        \"https://creativecommons.org/licenses/by-sa/3.0/at/legalcode\"\n      ],\n      \"isOsiApproved\": false\n    },\n    {\n      \"reference\": \"https://spdx.org/licenses/CC-BY-SA-3.0-DE.html\",\n      \"isDeprecatedLicenseId\": false,\n      \"detailsUrl\": \"https://spdx.org/licenses/CC-BY-SA-3.0-DE.json\",\n      \"referenceNumber\": 546,\n      \"name\": \"Creative Commons Attribution Share Alike 3.0 Germany\",\n      \"licenseId\": \"CC-BY-SA-3.0-DE\",\n      \"seeAlso\": [\n        \"https://creativecommons.org/licenses/by-sa/3.0/de/legalcode\"\n      ],\n      \"isOsiApproved\": false\n    },\n    {\n      \"reference\": \"https://spdx.org/licenses/CC-BY-SA-3.0-IGO.html\",\n      \"isDeprecatedLicenseId\": false,\n      \"detailsUrl\": \"https://spdx.org/licenses/CC-BY-SA-3.0-IGO.json\",\n      \"referenceNumber\": 572,\n      \"name\": \"Creative Commons Attribution-ShareAlike 3.0 IGO\",\n      \"licenseId\": \"CC-BY-SA-3.0-IGO\",\n      \"seeAlso\": [\n        \"https://creativecommons.org/licenses/by-sa/3.0/igo/legalcode\"\n      ],\n      \"isOsiApproved\": false\n    },\n    {\n      \"reference\": \"https://spdx.org/licenses/CC-BY-SA-4.0.html\",\n      \"isDeprecatedLicenseId\": false,\n      \"detailsUrl\": \"https://spdx.org/licenses/CC-BY-SA-4.0.json\",\n      \"referenceNumber\": 582,\n      \"name\": \"Creative Commons Attribution Share Alike 4.0 International\",\n      \"licenseId\": \"CC-BY-SA-4.0\",\n      \"seeAlso\": [\n        \"https://creativecommons.org/licenses/by-sa/4.0/legalcode\"\n      ],\n      \"isOsiApproved\": false,\n      \"isFsfLibre\": true\n    },\n    {\n      \"reference\": \"https://spdx.org/licenses/CC-PDDC.html\",\n      \"isDeprecatedLicenseId\": false,\n      \"detailsUrl\": \"https://spdx.org/licenses/CC-PDDC.json\",\n      \"referenceNumber\": 624,\n      \"name\": \"Creative Commons Public Domain Dedication and Certification\",\n      \"licenseId\": \"CC-PDDC\",\n      \"seeAlso\": [\n        \"https://creativecommons.org/licenses/publicdomain/\"\n      ],\n      \"isOsiApproved\": false\n    },\n    {\n      \"reference\": \"https://spdx.org/licenses/CC0-1.0.html\",\n      \"isDeprecatedLicenseId\": false,\n      \"detailsUrl\": \"https://spdx.org/licenses/CC0-1.0.json\",\n      \"referenceNumber\": 262,\n      \"name\": \"Creative Commons Zero v1.0 Universal\",\n      \"licenseId\": \"CC0-1.0\",\n      \"seeAlso\": [\n        \"https://creativecommons.org/publicdomain/zero/1.0/legalcode\"\n      ],\n      \"isOsiApproved\": false,\n      \"isFsfLibre\": true\n    },\n    {\n      \"reference\": \"https://spdx.org/licenses/CDDL-1.0.html\",\n      \"isDeprecatedLicenseId\": false,\n      \"detailsUrl\": \"https://spdx.org/licenses/CDDL-1.0.json\",\n      \"referenceNumber\": 562,\n      \"name\": \"Common Development and Distribution License 1.0\",\n      \"licenseId\": \"CDDL-1.0\",\n      \"seeAlso\": [\n        \"https://opensource.org/licenses/cddl1\"\n      ],\n      \"isOsiApproved\": true,\n      \"isFsfLibre\": true\n    },\n    {\n      \"reference\": \"https://spdx.org/licenses/CDDL-1.1.html\",\n      \"isDeprecatedLicenseId\": false,\n      \"detailsUrl\": \"https://spdx.org/licenses/CDDL-1.1.json\",\n      \"referenceNumber\": 85,\n      \"name\": \"Common Development and Distribution License 1.1\",\n      \"licenseId\": \"CDDL-1.1\",\n      \"seeAlso\": [\n        \"http://glassfish.java.net/public/CDDL+GPL_1_1.html\",\n        \"https://javaee.github.io/glassfish/LICENSE\"\n      ],\n      \"isOsiApproved\": false\n    },\n    {\n      \"reference\": \"https://spdx.org/licenses/CDL-1.0.html\",\n      \"isDeprecatedLicenseId\": false,\n      \"detailsUrl\": \"https://spdx.org/licenses/CDL-1.0.json\",\n      \"referenceNumber\": 22,\n      \"name\": \"Common Documentation License 1.0\",\n      \"licenseId\": \"CDL-1.0\",\n      \"seeAlso\": [\n        \"http://www.opensource.apple.com/cdl/\",\n        \"https://fedoraproject.org/wiki/Licensing/Common_Documentation_License\",\n        \"https://www.gnu.org/licenses/license-list.html#ACDL\"\n      ],\n      \"isOsiApproved\": false\n    },\n    {\n      \"reference\": \"https://spdx.org/licenses/CDLA-Permissive-1.0.html\",\n      \"isDeprecatedLicenseId\": false,\n      \"detailsUrl\": \"https://spdx.org/licenses/CDLA-Permissive-1.0.json\",\n      \"referenceNumber\": 445,\n      \"name\": \"Community Data License Agreement Permissive 1.0\",\n      \"licenseId\": \"CDLA-Permissive-1.0\",\n      \"seeAlso\": [\n        \"https://cdla.io/permissive-1-0\"\n      ],\n      \"isOsiApproved\": false\n    },\n    {\n      \"reference\": \"https://spdx.org/licenses/CDLA-Permissive-2.0.html\",\n      \"isDeprecatedLicenseId\": false,\n      \"detailsUrl\": \"https://spdx.org/licenses/CDLA-Permissive-2.0.json\",\n      \"referenceNumber\": 110,\n      \"name\": \"Community Data License Agreement Permissive 2.0\",\n      \"licenseId\": \"CDLA-Permissive-2.0\",\n      \"seeAlso\": [\n        \"https://cdla.dev/permissive-2-0\"\n      ],\n      \"isOsiApproved\": false\n    },\n    {\n      \"reference\": \"https://spdx.org/licenses/CDLA-Sharing-1.0.html\",\n      \"isDeprecatedLicenseId\": false,\n      \"detailsUrl\": \"https://spdx.org/licenses/CDLA-Sharing-1.0.json\",\n      \"referenceNumber\": 336,\n      \"name\": \"Community Data License Agreement Sharing 1.0\",\n      \"licenseId\": \"CDLA-Sharing-1.0\",\n      \"seeAlso\": [\n        \"https://cdla.io/sharing-1-0\"\n      ],\n      \"isOsiApproved\": false\n    },\n    {\n      \"reference\": \"https://spdx.org/licenses/CECILL-1.0.html\",\n      \"isDeprecatedLicenseId\": false,\n      \"detailsUrl\": \"https://spdx.org/licenses/CECILL-1.0.json\",\n      \"referenceNumber\": 124,\n      \"name\": \"CeCILL Free Software License Agreement v1.0\",\n      \"licenseId\": \"CECILL-1.0\",\n      \"seeAlso\": [\n        \"http://www.cecill.info/licences/Licence_CeCILL_V1-fr.html\"\n      ],\n      \"isOsiApproved\": false\n    },\n    {\n      \"reference\": \"https://spdx.org/licenses/CECILL-1.1.html\",\n      \"isDeprecatedLicenseId\": false,\n      \"detailsUrl\": \"https://spdx.org/licenses/CECILL-1.1.json\",\n      \"referenceNumber\": 568,\n      \"name\": \"CeCILL Free Software License Agreement v1.1\",\n      \"licenseId\": \"CECILL-1.1\",\n      \"seeAlso\": [\n        \"http://www.cecill.info/licences/Licence_CeCILL_V1.1-US.html\"\n      ],\n      \"isOsiApproved\": false\n    },\n    {\n      \"reference\": \"https://spdx.org/licenses/CECILL-2.0.html\",\n      \"isDeprecatedLicenseId\": false,\n      \"detailsUrl\": \"https://spdx.org/licenses/CECILL-2.0.json\",\n      \"referenceNumber\": 598,\n      \"name\": \"CeCILL Free Software License Agreement v2.0\",\n      \"licenseId\": \"CECILL-2.0\",\n      \"seeAlso\": [\n        \"http://www.cecill.info/licences/Licence_CeCILL_V2-en.html\"\n      ],\n      \"isOsiApproved\": false,\n      \"isFsfLibre\": true\n    },\n    {\n      \"reference\": \"https://spdx.org/licenses/CECILL-2.1.html\",\n      \"isDeprecatedLicenseId\": false,\n      \"detailsUrl\": \"https://spdx.org/licenses/CECILL-2.1.json\",\n      \"referenceNumber\": 501,\n      \"name\": \"CeCILL Free Software License Agreement v2.1\",\n      \"licenseId\": \"CECILL-2.1\",\n      \"seeAlso\": [\n        \"http://www.cecill.info/licences/Licence_CeCILL_V2.1-en.html\"\n      ],\n      \"isOsiApproved\": true\n    },\n    {\n      \"reference\": \"https://spdx.org/licenses/CECILL-B.html\",\n      \"isDeprecatedLicenseId\": false,\n      \"detailsUrl\": \"https://spdx.org/licenses/CECILL-B.json\",\n      \"referenceNumber\": 554,\n      \"name\": \"CeCILL-B Free Software License Agreement\",\n      \"licenseId\": \"CECILL-B\",\n      \"seeAlso\": [\n        \"http://www.cecill.info/licences/Licence_CeCILL-B_V1-en.html\"\n      ],\n      \"isOsiApproved\": false,\n      \"isFsfLibre\": true\n    },\n    {\n      \"reference\": \"https://spdx.org/licenses/CECILL-C.html\",\n      \"isDeprecatedLicenseId\": false,\n      \"detailsUrl\": \"https://spdx.org/licenses/CECILL-C.json\",\n      \"referenceNumber\": 278,\n      \"name\": \"CeCILL-C Free Software License Agreement\",\n      \"licenseId\": \"CECILL-C\",\n      \"seeAlso\": [\n        \"http://www.cecill.info/licences/Licence_CeCILL-C_V1-en.html\"\n      ],\n      \"isOsiApproved\": false,\n      \"isFsfLibre\": true\n    },\n    {\n      \"reference\": \"https://spdx.org/licenses/CERN-OHL-1.1.html\",\n      \"isDeprecatedLicenseId\": false,\n      \"detailsUrl\": \"https://spdx.org/licenses/CERN-OHL-1.1.json\",\n      \"referenceNumber\": 367,\n      \"name\": \"CERN Open Hardware Licence v1.1\",\n      \"licenseId\": \"CERN-OHL-1.1\",\n      \"seeAlso\": [\n        \"https://www.ohwr.org/project/licenses/wikis/cern-ohl-v1.1\"\n      ],\n      \"isOsiApproved\": false\n    },\n    {\n      \"reference\": \"https://spdx.org/licenses/CERN-OHL-1.2.html\",\n      \"isDeprecatedLicenseId\": false,\n      \"detailsUrl\": \"https://spdx.org/licenses/CERN-OHL-1.2.json\",\n      \"referenceNumber\": 415,\n      \"name\": \"CERN Open Hardware Licence v1.2\",\n      \"licenseId\": \"CERN-OHL-1.2\",\n      \"seeAlso\": [\n        \"https://www.ohwr.org/project/licenses/wikis/cern-ohl-v1.2\"\n      ],\n      \"isOsiApproved\": false\n    },\n    {\n      \"reference\": \"https://spdx.org/licenses/CERN-OHL-P-2.0.html\",\n      \"isDeprecatedLicenseId\": false,\n      \"detailsUrl\": \"https://spdx.org/licenses/CERN-OHL-P-2.0.json\",\n      \"referenceNumber\": 96,\n      \"name\": \"CERN Open Hardware Licence Version 2 - Permissive\",\n      \"licenseId\": \"CERN-OHL-P-2.0\",\n      \"seeAlso\": [\n        \"https://www.ohwr.org/project/cernohl/wikis/Documents/CERN-OHL-version-2\"\n      ],\n      \"isOsiApproved\": true\n    },\n    {\n      \"reference\": \"https://spdx.org/licenses/CERN-OHL-S-2.0.html\",\n      \"isDeprecatedLicenseId\": false,\n      \"detailsUrl\": \"https://spdx.org/licenses/CERN-OHL-S-2.0.json\",\n      \"referenceNumber\": 326,\n      \"name\": \"CERN Open Hardware Licence Version 2 - Strongly Reciprocal\",\n      \"licenseId\": \"CERN-OHL-S-2.0\",\n      \"seeAlso\": [\n        \"https://www.ohwr.org/project/cernohl/wikis/Documents/CERN-OHL-version-2\"\n      ],\n      \"isOsiApproved\": true\n    },\n    {\n      \"reference\": \"https://spdx.org/licenses/CERN-OHL-W-2.0.html\",\n      \"isDeprecatedLicenseId\": false,\n      \"detailsUrl\": \"https://spdx.org/licenses/CERN-OHL-W-2.0.json\",\n      \"referenceNumber\": 589,\n      \"name\": \"CERN Open Hardware Licence Version 2 - Weakly Reciprocal\",\n      \"licenseId\": \"CERN-OHL-W-2.0\",\n      \"seeAlso\": [\n        \"https://www.ohwr.org/project/cernohl/wikis/Documents/CERN-OHL-version-2\"\n      ],\n      \"isOsiApproved\": true\n    },\n    {\n      \"reference\": \"https://spdx.org/licenses/CFITSIO.html\",\n      \"isDeprecatedLicenseId\": false,\n      \"detailsUrl\": \"https://spdx.org/licenses/CFITSIO.json\",\n      \"referenceNumber\": 178,\n      \"name\": \"CFITSIO License\",\n      \"licenseId\": \"CFITSIO\",\n      \"seeAlso\": [\n        \"https://heasarc.gsfc.nasa.gov/docs/software/fitsio/c/f_user/node9.html\",\n        \"https://heasarc.gsfc.nasa.gov/docs/software/ftools/fv/doc/license.html\"\n      ],\n      \"isOsiApproved\": false\n    },\n    {\n      \"reference\": \"https://spdx.org/licenses/check-cvs.html\",\n      \"isDeprecatedLicenseId\": false,\n      \"detailsUrl\": \"https://spdx.org/licenses/check-cvs.json\",\n      \"referenceNumber\": 28,\n      \"name\": \"check-cvs License\",\n      \"licenseId\": \"check-cvs\",\n      \"seeAlso\": [\n        \"http://cvs.savannah.gnu.org/viewvc/cvs/ccvs/contrib/check_cvs.in?revision\\u003d1.1.4.3\\u0026view\\u003dmarkup\\u0026pathrev\\u003dcvs1-11-23#l2\"\n      ],\n      \"isOsiApproved\": false\n    },\n    {\n      \"reference\": \"https://spdx.org/licenses/checkmk.html\",\n      \"isDeprecatedLicenseId\": false,\n      \"detailsUrl\": \"https://spdx.org/licenses/checkmk.json\",\n      \"referenceNumber\": 57,\n      \"name\": \"Checkmk License\",\n      \"licenseId\": \"checkmk\",\n      \"seeAlso\": [\n        \"https://github.com/libcheck/check/blob/master/checkmk/checkmk.in\"\n      ],\n      \"isOsiApproved\": false\n    },\n    {\n      \"reference\": \"https://spdx.org/licenses/ClArtistic.html\",\n      \"isDeprecatedLicenseId\": false,\n      \"detailsUrl\": \"https://spdx.org/licenses/ClArtistic.json\",\n      \"referenceNumber\": 592,\n      \"name\": \"Clarified Artistic License\",\n      \"licenseId\": \"ClArtistic\",\n      \"seeAlso\": [\n        \"http://gianluca.dellavedova.org/2011/01/03/clarified-artistic-license/\",\n        \"http://www.ncftp.com/ncftp/doc/LICENSE.txt\"\n      ],\n      \"isOsiApproved\": false,\n      \"isFsfLibre\": true\n    },\n    {\n      \"reference\": \"https://spdx.org/licenses/Clips.html\",\n      \"isDeprecatedLicenseId\": false,\n      \"detailsUrl\": \"https://spdx.org/licenses/Clips.json\",\n      \"referenceNumber\": 143,\n      \"name\": \"Clips License\",\n      \"licenseId\": \"Clips\",\n      \"seeAlso\": [\n        \"https://github.com/DrItanium/maya/blob/master/LICENSE.CLIPS\"\n      ],\n      \"isOsiApproved\": false\n    },\n    {\n      \"reference\": \"https://spdx.org/licenses/CMU-Mach.html\",\n      \"isDeprecatedLicenseId\": false,\n      \"detailsUrl\": \"https://spdx.org/licenses/CMU-Mach.json\",\n      \"referenceNumber\": 119,\n      \"name\": \"CMU Mach License\",\n      \"licenseId\": \"CMU-Mach\",\n      \"seeAlso\": [\n        \"https://www.cs.cmu.edu/~410/licenses.html\"\n      ],\n      \"isOsiApproved\": false\n    },\n    {\n      \"reference\": \"https://spdx.org/licenses/CMU-Mach-nodoc.html\",\n      \"isDeprecatedLicenseId\": false,\n      \"detailsUrl\": \"https://spdx.org/licenses/CMU-Mach-nodoc.json\",\n      \"referenceNumber\": 524,\n      \"name\": \"CMU    Mach - no notices-in-documentation variant\",\n      \"licenseId\": \"CMU-Mach-nodoc\",\n      \"seeAlso\": [\n        \"https://github.com/krb5/krb5/blob/krb5-1.21.2-final/NOTICE#L718-L728\",\n        \"https://web.mit.edu/kerberos/krb5-1.21/doc/mitK5license.html\"\n      ],\n      \"isOsiApproved\": false\n    },\n    {\n      \"reference\": \"https://spdx.org/licenses/CNRI-Jython.html\",\n      \"isDeprecatedLicenseId\": false,\n      \"detailsUrl\": \"https://spdx.org/licenses/CNRI-Jython.json\",\n      \"referenceNumber\": 281,\n      \"name\": \"CNRI Jython License\",\n      \"licenseId\": \"CNRI-Jython\",\n      \"seeAlso\": [\n        \"http://www.jython.org/license.html\"\n      ],\n      \"isOsiApproved\": false\n    },\n    {\n      \"reference\": \"https://spdx.org/licenses/CNRI-Python.html\",\n      \"isDeprecatedLicenseId\": false,\n      \"detailsUrl\": \"https://spdx.org/licenses/CNRI-Python.json\",\n      \"referenceNumber\": 623,\n      \"name\": \"CNRI Python License\",\n      \"licenseId\": \"CNRI-Python\",\n      \"seeAlso\": [\n        \"https://opensource.org/licenses/CNRI-Python\"\n      ],\n      \"isOsiApproved\": true\n    },\n    {\n      \"reference\": \"https://spdx.org/licenses/CNRI-Python-GPL-Compatible.html\",\n      \"isDeprecatedLicenseId\": false,\n      \"detailsUrl\": \"https://spdx.org/licenses/CNRI-Python-GPL-Compatible.json\",\n      \"referenceNumber\": 173,\n      \"name\": \"CNRI Python Open Source GPL Compatible License Agreement\",\n      \"licenseId\": \"CNRI-Python-GPL-Compatible\",\n      \"seeAlso\": [\n        \"http://www.python.org/download/releases/1.6.1/download_win/\"\n      ],\n      \"isOsiApproved\": false\n    },\n    {\n      \"reference\": \"https://spdx.org/licenses/COIL-1.0.html\",\n      \"isDeprecatedLicenseId\": false,\n      \"detailsUrl\": \"https://spdx.org/licenses/COIL-1.0.json\",\n      \"referenceNumber\": 573,\n      \"name\": \"Copyfree Open Innovation License\",\n      \"licenseId\": \"COIL-1.0\",\n      \"seeAlso\": [\n        \"https://coil.apotheon.org/plaintext/01.0.txt\"\n      ],\n      \"isOsiApproved\": false\n    },\n    {\n      \"reference\": \"https://spdx.org/licenses/Community-Spec-1.0.html\",\n      \"isDeprecatedLicenseId\": false,\n      \"detailsUrl\": \"https://spdx.org/licenses/Community-Spec-1.0.json\",\n      \"referenceNumber\": 385,\n      \"name\": \"Community Specification License 1.0\",\n      \"licenseId\": \"Community-Spec-1.0\",\n      \"seeAlso\": [\n        \"https://github.com/CommunitySpecification/1.0/blob/master/1._Community_Specification_License-v1.md\"\n      ],\n      \"isOsiApproved\": false\n    },\n    {\n      \"reference\": \"https://spdx.org/licenses/Condor-1.1.html\",\n      \"isDeprecatedLicenseId\": false,\n      \"detailsUrl\": \"https://spdx.org/licenses/Condor-1.1.json\",\n      \"referenceNumber\": 208,\n      \"name\": \"Condor Public License v1.1\",\n      \"licenseId\": \"Condor-1.1\",\n      \"seeAlso\": [\n        \"http://research.cs.wisc.edu/condor/license.html#condor\",\n        \"http://web.archive.org/web/20111123062036/http://research.cs.wisc.edu/condor/license.html#condor\"\n      ],\n      \"isOsiApproved\": false,\n      \"isFsfLibre\": true\n    },\n    {\n      \"reference\": \"https://spdx.org/licenses/copyleft-next-0.3.0.html\",\n      \"isDeprecatedLicenseId\": false,\n      \"detailsUrl\": \"https://spdx.org/licenses/copyleft-next-0.3.0.json\",\n      \"referenceNumber\": 427,\n      \"name\": \"copyleft-next 0.3.0\",\n      \"licenseId\": \"copyleft-next-0.3.0\",\n      \"seeAlso\": [\n        \"https://github.com/copyleft-next/copyleft-next/blob/master/Releases/copyleft-next-0.3.0\"\n      ],\n      \"isOsiApproved\": false\n    },\n    {\n      \"reference\": \"https://spdx.org/licenses/copyleft-next-0.3.1.html\",\n      \"isDeprecatedLicenseId\": false,\n      \"detailsUrl\": \"https://spdx.org/licenses/copyleft-next-0.3.1.json\",\n      \"referenceNumber\": 649,\n      \"name\": \"copyleft-next 0.3.1\",\n      \"licenseId\": \"copyleft-next-0.3.1\",\n      \"seeAlso\": [\n        \"https://github.com/copyleft-next/copyleft-next/blob/master/Releases/copyleft-next-0.3.1\"\n      ],\n      \"isOsiApproved\": false\n    },\n    {\n      \"reference\": \"https://spdx.org/licenses/Cornell-Lossless-JPEG.html\",\n      \"isDeprecatedLicenseId\": false,\n      \"detailsUrl\": \"https://spdx.org/licenses/Cornell-Lossless-JPEG.json\",\n      \"referenceNumber\": 181,\n      \"name\": \"Cornell Lossless JPEG License\",\n      \"licenseId\": \"Cornell-Lossless-JPEG\",\n      \"seeAlso\": [\n        \"https://android.googlesource.com/platform/external/dng_sdk/+/refs/heads/master/source/dng_lossless_jpeg.cpp#16\",\n        \"https://www.mssl.ucl.ac.uk/~mcrw/src/20050920/proto.h\",\n        \"https://gitlab.freedesktop.org/libopenraw/libopenraw/blob/master/lib/ljpegdecompressor.cpp#L32\"\n      ],\n      \"isOsiApproved\": false\n    },\n    {\n      \"reference\": \"https://spdx.org/licenses/CPAL-1.0.html\",\n      \"isDeprecatedLicenseId\": false,\n      \"detailsUrl\": \"https://spdx.org/licenses/CPAL-1.0.json\",\n      \"referenceNumber\": 230,\n      \"name\": \"Common Public Attribution License 1.0\",\n      \"licenseId\": \"CPAL-1.0\",\n      \"seeAlso\": [\n        \"https://opensource.org/licenses/CPAL-1.0\"\n      ],\n      \"isOsiApproved\": true,\n      \"isFsfLibre\": true\n    },\n    {\n      \"reference\": \"https://spdx.org/licenses/CPL-1.0.html\",\n      \"isDeprecatedLicenseId\": false,\n      \"detailsUrl\": \"https://spdx.org/licenses/CPL-1.0.json\",\n      \"referenceNumber\": 97,\n      \"name\": \"Common Public License 1.0\",\n      \"licenseId\": \"CPL-1.0\",\n      \"seeAlso\": [\n        \"https://opensource.org/licenses/CPL-1.0\"\n      ],\n      \"isOsiApproved\": true,\n      \"isFsfLibre\": true\n    },\n    {\n      \"reference\": \"https://spdx.org/licenses/CPOL-1.02.html\",\n      \"isDeprecatedLicenseId\": false,\n      \"detailsUrl\": \"https://spdx.org/licenses/CPOL-1.02.json\",\n      \"referenceNumber\": 399,\n      \"name\": \"Code Project Open License 1.02\",\n      \"licenseId\": \"CPOL-1.02\",\n      \"seeAlso\": [\n        \"http://www.codeproject.com/info/cpol10.aspx\"\n      ],\n      \"isOsiApproved\": false,\n      \"isFsfLibre\": false\n    },\n    {\n      \"reference\": \"https://spdx.org/licenses/Cronyx.html\",\n      \"isDeprecatedLicenseId\": false,\n      \"detailsUrl\": \"https://spdx.org/licenses/Cronyx.json\",\n      \"referenceNumber\": 535,\n      \"name\": \"Cronyx License\",\n      \"licenseId\": \"Cronyx\",\n      \"seeAlso\": [\n        \"https://gitlab.freedesktop.org/xorg/font/alias/-/blob/master/COPYING\",\n        \"https://gitlab.freedesktop.org/xorg/font/cronyx-cyrillic/-/blob/master/COPYING\",\n        \"https://gitlab.freedesktop.org/xorg/font/misc-cyrillic/-/blob/master/COPYING\",\n        \"https://gitlab.freedesktop.org/xorg/font/screen-cyrillic/-/blob/master/COPYING\"\n      ],\n      \"isOsiApproved\": false\n    },\n    {\n      \"reference\": \"https://spdx.org/licenses/Crossword.html\",\n      \"isDeprecatedLicenseId\": false,\n      \"detailsUrl\": \"https://spdx.org/licenses/Crossword.json\",\n      \"referenceNumber\": 482,\n      \"name\": \"Crossword License\",\n      \"licenseId\": \"Crossword\",\n      \"seeAlso\": [\n        \"https://fedoraproject.org/wiki/Licensing/Crossword\"\n      ],\n      \"isOsiApproved\": false\n    },\n    {\n      \"reference\": \"https://spdx.org/licenses/CrystalStacker.html\",\n      \"isDeprecatedLicenseId\": false,\n      \"detailsUrl\": \"https://spdx.org/licenses/CrystalStacker.json\",\n      \"referenceNumber\": 236,\n      \"name\": \"CrystalStacker License\",\n      \"licenseId\": \"CrystalStacker\",\n      \"seeAlso\": [\n        \"https://fedoraproject.org/wiki/Licensing:CrystalStacker?rd\\u003dLicensing/CrystalStacker\"\n      ],\n      \"isOsiApproved\": false\n    },\n    {\n      \"reference\": \"https://spdx.org/licenses/CUA-OPL-1.0.html\",\n      \"isDeprecatedLicenseId\": false,\n      \"detailsUrl\": \"https://spdx.org/licenses/CUA-OPL-1.0.json\",\n      \"referenceNumber\": 275,\n      \"name\": \"CUA Office Public License v1.0\",\n      \"licenseId\": \"CUA-OPL-1.0\",\n      \"seeAlso\": [\n        \"https://opensource.org/licenses/CUA-OPL-1.0\"\n      ],\n      \"isOsiApproved\": true\n    },\n    {\n      \"reference\": \"https://spdx.org/licenses/Cube.html\",\n      \"isDeprecatedLicenseId\": false,\n      \"detailsUrl\": \"https://spdx.org/licenses/Cube.json\",\n      \"referenceNumber\": 270,\n      \"name\": \"Cube License\",\n      \"licenseId\": \"Cube\",\n      \"seeAlso\": [\n        \"https://fedoraproject.org/wiki/Licensing/Cube\"\n      ],\n      \"isOsiApproved\": false\n    },\n    {\n      \"reference\": \"https://spdx.org/licenses/curl.html\",\n      \"isDeprecatedLicenseId\": false,\n      \"detailsUrl\": \"https://spdx.org/licenses/curl.json\",\n      \"referenceNumber\": 118,\n      \"name\": \"curl License\",\n      \"licenseId\": \"curl\",\n      \"seeAlso\": [\n        \"https://github.com/bagder/curl/blob/master/COPYING\"\n      ],\n      \"isOsiApproved\": false\n    },\n    {\n      \"reference\": \"https://spdx.org/licenses/cve-tou.html\",\n      \"isDeprecatedLicenseId\": false,\n      \"detailsUrl\": \"https://spdx.org/licenses/cve-tou.json\",\n      \"referenceNumber\": 74,\n      \"name\": \"Common Vulnerability Enumeration ToU License\",\n      \"licenseId\": \"cve-tou\",\n      \"seeAlso\": [\n        \"https://www.cve.org/Legal/TermsOfUse\"\n      ],\n      \"isOsiApproved\": false\n    },\n    {\n      \"reference\": \"https://spdx.org/licenses/D-FSL-1.0.html\",\n      \"isDeprecatedLicenseId\": false,\n      \"detailsUrl\": \"https://spdx.org/licenses/D-FSL-1.0.json\",\n      \"referenceNumber\": 490,\n      \"name\": \"Deutsche Freie Software Lizenz\",\n      \"licenseId\": \"D-FSL-1.0\",\n      \"seeAlso\": [\n        \"http://www.dipp.nrw.de/d-fsl/lizenzen/\",\n        \"http://www.dipp.nrw.de/d-fsl/index_html/lizenzen/de/D-FSL-1_0_de.txt\",\n        \"http://www.dipp.nrw.de/d-fsl/index_html/lizenzen/en/D-FSL-1_0_en.txt\",\n        \"https://www.hbz-nrw.de/produkte/open-access/lizenzen/dfsl\",\n        \"https://www.hbz-nrw.de/produkte/open-access/lizenzen/dfsl/deutsche-freie-software-lizenz\",\n        \"https://www.hbz-nrw.de/produkte/open-access/lizenzen/dfsl/german-free-software-license\",\n        \"https://www.hbz-nrw.de/produkte/open-access/lizenzen/dfsl/D-FSL-1_0_de.txt/at_download/file\",\n        \"https://www.hbz-nrw.de/produkte/open-access/lizenzen/dfsl/D-FSL-1_0_en.txt/at_download/file\"\n      ],\n      \"isOsiApproved\": false\n    },\n    {\n      \"reference\": \"https://spdx.org/licenses/DEC-3-Clause.html\",\n      \"isDeprecatedLicenseId\": false,\n      \"detailsUrl\": \"https://spdx.org/licenses/DEC-3-Clause.json\",\n      \"referenceNumber\": 494,\n      \"name\": \"DEC 3-Clause License\",\n      \"licenseId\": \"DEC-3-Clause\",\n      \"seeAlso\": [\n        \"https://gitlab.freedesktop.org/xorg/xserver/-/blob/master/COPYING?ref_type\\u003dheads#L239\"\n      ],\n      \"isOsiApproved\": false\n    },\n    {\n      \"reference\": \"https://spdx.org/licenses/diffmark.html\",\n      \"isDeprecatedLicenseId\": false,\n      \"detailsUrl\": \"https://spdx.org/licenses/diffmark.json\",\n      \"referenceNumber\": 584,\n      \"name\": \"diffmark license\",\n      \"licenseId\": \"diffmark\",\n      \"seeAlso\": [\n        \"https://fedoraproject.org/wiki/Licensing/diffmark\"\n      ],\n      \"isOsiApproved\": false\n    },\n    {\n      \"reference\": \"https://spdx.org/licenses/DL-DE-BY-2.0.html\",\n      \"isDeprecatedLicenseId\": false,\n      \"detailsUrl\": \"https://spdx.org/licenses/DL-DE-BY-2.0.json\",\n      \"referenceNumber\": 560,\n      \"name\": \"Data licence Germany – attribution – version 2.0\",\n      \"licenseId\": \"DL-DE-BY-2.0\",\n      \"seeAlso\": [\n        \"https://www.govdata.de/dl-de/by-2-0\"\n      ],\n      \"isOsiApproved\": false\n    },\n    {\n      \"reference\": \"https://spdx.org/licenses/DL-DE-ZERO-2.0.html\",\n      \"isDeprecatedLicenseId\": false,\n      \"detailsUrl\": \"https://spdx.org/licenses/DL-DE-ZERO-2.0.json\",\n      \"referenceNumber\": 86,\n      \"name\": \"Data licence Germany – zero – version 2.0\",\n      \"licenseId\": \"DL-DE-ZERO-2.0\",\n      \"seeAlso\": [\n        \"https://www.govdata.de/dl-de/zero-2-0\"\n      ],\n      \"isOsiApproved\": false\n    },\n    {\n      \"reference\": \"https://spdx.org/licenses/DOC.html\",\n      \"isDeprecatedLicenseId\": false,\n      \"detailsUrl\": \"https://spdx.org/licenses/DOC.json\",\n      \"referenceNumber\": 426,\n      \"name\": \"DOC License\",\n      \"licenseId\": \"DOC\",\n      \"seeAlso\": [\n        \"http://www.cs.wustl.edu/~schmidt/ACE-copying.html\",\n        \"https://www.dre.vanderbilt.edu/~schmidt/ACE-copying.html\"\n      ],\n      \"isOsiApproved\": false\n    },\n    {\n      \"reference\": \"https://spdx.org/licenses/Dotseqn.html\",\n      \"isDeprecatedLicenseId\": false,\n      \"detailsUrl\": \"https://spdx.org/licenses/Dotseqn.json\",\n      \"referenceNumber\": 525,\n      \"name\": \"Dotseqn License\",\n      \"licenseId\": \"Dotseqn\",\n      \"seeAlso\": [\n        \"https://fedoraproject.org/wiki/Licensing/Dotseqn\"\n      ],\n      \"isOsiApproved\": false\n    },\n    {\n      \"reference\": \"https://spdx.org/licenses/DRL-1.0.html\",\n      \"isDeprecatedLicenseId\": false,\n      \"detailsUrl\": \"https://spdx.org/licenses/DRL-1.0.json\",\n      \"referenceNumber\": 61,\n      \"name\": \"Detection Rule License 1.0\",\n      \"licenseId\": \"DRL-1.0\",\n      \"seeAlso\": [\n        \"https://github.com/Neo23x0/sigma/blob/master/LICENSE.Detection.Rules.md\"\n      ],\n      \"isOsiApproved\": false\n    },\n    {\n      \"reference\": \"https://spdx.org/licenses/DRL-1.1.html\",\n      \"isDeprecatedLicenseId\": false,\n      \"detailsUrl\": \"https://spdx.org/licenses/DRL-1.1.json\",\n      \"referenceNumber\": 646,\n      \"name\": \"Detection Rule License 1.1\",\n      \"licenseId\": \"DRL-1.1\",\n      \"seeAlso\": [\n        \"https://github.com/SigmaHQ/Detection-Rule-License/blob/6ec7fbde6101d101b5b5d1fcb8f9b69fbc76c04a/LICENSE.Detection.Rules.md\"\n      ],\n      \"isOsiApproved\": false\n    },\n    {\n      \"reference\": \"https://spdx.org/licenses/DSDP.html\",\n      \"isDeprecatedLicenseId\": false,\n      \"detailsUrl\": \"https://spdx.org/licenses/DSDP.json\",\n      \"referenceNumber\": 15,\n      \"name\": \"DSDP License\",\n      \"licenseId\": \"DSDP\",\n      \"seeAlso\": [\n        \"https://fedoraproject.org/wiki/Licensing/DSDP\"\n      ],\n      \"isOsiApproved\": false\n    },\n    {\n      \"reference\": \"https://spdx.org/licenses/dtoa.html\",\n      \"isDeprecatedLicenseId\": false,\n      \"detailsUrl\": \"https://spdx.org/licenses/dtoa.json\",\n      \"referenceNumber\": 544,\n      \"name\": \"David M. Gay dtoa License\",\n      \"licenseId\": \"dtoa\",\n      \"seeAlso\": [\n        \"https://github.com/SWI-Prolog/swipl-devel/blob/master/src/os/dtoa.c\",\n        \"https://sourceware.org/git/?p\\u003dnewlib-cygwin.git;a\\u003dblob;f\\u003dnewlib/libc/stdlib/mprec.h;hb\\u003dHEAD\"\n      ],\n      \"isOsiApproved\": false\n    },\n    {\n      \"reference\": \"https://spdx.org/licenses/dvipdfm.html\",\n      \"isDeprecatedLicenseId\": false,\n      \"detailsUrl\": \"https://spdx.org/licenses/dvipdfm.json\",\n      \"referenceNumber\": 358,\n      \"name\": \"dvipdfm License\",\n      \"licenseId\": \"dvipdfm\",\n      \"seeAlso\": [\n        \"https://fedoraproject.org/wiki/Licensing/dvipdfm\"\n      ],\n      \"isOsiApproved\": false\n    },\n    {\n      \"reference\": \"https://spdx.org/licenses/ECL-1.0.html\",\n      \"isDeprecatedLicenseId\": false,\n      \"detailsUrl\": \"https://spdx.org/licenses/ECL-1.0.json\",\n      \"referenceNumber\": 470,\n      \"name\": \"Educational Community License v1.0\",\n      \"licenseId\": \"ECL-1.0\",\n      \"seeAlso\": [\n        \"https://opensource.org/licenses/ECL-1.0\"\n      ],\n      \"isOsiApproved\": true\n    },\n    {\n      \"reference\": \"https://spdx.org/licenses/ECL-2.0.html\",\n      \"isDeprecatedLicenseId\": false,\n      \"detailsUrl\": \"https://spdx.org/licenses/ECL-2.0.json\",\n      \"referenceNumber\": 256,\n      \"name\": \"Educational Community License v2.0\",\n      \"licenseId\": \"ECL-2.0\",\n      \"seeAlso\": [\n        \"https://opensource.org/licenses/ECL-2.0\"\n      ],\n      \"isOsiApproved\": true,\n      \"isFsfLibre\": true\n    },\n    {\n      \"reference\": \"https://spdx.org/licenses/eCos-2.0.html\",\n      \"isDeprecatedLicenseId\": true,\n      \"detailsUrl\": \"https://spdx.org/licenses/eCos-2.0.json\",\n      \"referenceNumber\": 211,\n      \"name\": \"eCos license version 2.0\",\n      \"licenseId\": \"eCos-2.0\",\n      \"seeAlso\": [\n        \"https://www.gnu.org/licenses/ecos-license.html\"\n      ],\n      \"isOsiApproved\": false,\n      \"isFsfLibre\": true\n    },\n    {\n      \"reference\": \"https://spdx.org/licenses/EFL-1.0.html\",\n      \"isDeprecatedLicenseId\": false,\n      \"detailsUrl\": \"https://spdx.org/licenses/EFL-1.0.json\",\n      \"referenceNumber\": 422,\n      \"name\": \"Eiffel Forum License v1.0\",\n      \"licenseId\": \"EFL-1.0\",\n      \"seeAlso\": [\n        \"http://www.eiffel-nice.org/license/forum.txt\",\n        \"https://opensource.org/licenses/EFL-1.0\"\n      ],\n      \"isOsiApproved\": true\n    },\n    {\n      \"reference\": \"https://spdx.org/licenses/EFL-2.0.html\",\n      \"isDeprecatedLicenseId\": false,\n      \"detailsUrl\": \"https://spdx.org/licenses/EFL-2.0.json\",\n      \"referenceNumber\": 107,\n      \"name\": \"Eiffel Forum License v2.0\",\n      \"licenseId\": \"EFL-2.0\",\n      \"seeAlso\": [\n        \"http://www.eiffel-nice.org/license/eiffel-forum-license-2.html\",\n        \"https://opensource.org/licenses/EFL-2.0\"\n      ],\n      \"isOsiApproved\": true,\n      \"isFsfLibre\": true\n    },\n    {\n      \"reference\": \"https://spdx.org/licenses/eGenix.html\",\n      \"isDeprecatedLicenseId\": false,\n      \"detailsUrl\": \"https://spdx.org/licenses/eGenix.json\",\n      \"referenceNumber\": 29,\n      \"name\": \"eGenix.com Public License 1.1.0\",\n      \"licenseId\": \"eGenix\",\n      \"seeAlso\": [\n        \"http://www.egenix.com/products/eGenix.com-Public-License-1.1.0.pdf\",\n        \"https://fedoraproject.org/wiki/Licensing/eGenix.com_Public_License_1.1.0\"\n      ],\n      \"isOsiApproved\": false\n    },\n    {\n      \"reference\": \"https://spdx.org/licenses/Elastic-2.0.html\",\n      \"isDeprecatedLicenseId\": false,\n      \"detailsUrl\": \"https://spdx.org/licenses/Elastic-2.0.json\",\n      \"referenceNumber\": 264,\n      \"name\": \"Elastic License 2.0\",\n      \"licenseId\": \"Elastic-2.0\",\n      \"seeAlso\": [\n        \"https://www.elastic.co/licensing/elastic-license\",\n        \"https://github.com/elastic/elasticsearch/blob/master/licenses/ELASTIC-LICENSE-2.0.txt\"\n      ],\n      \"isOsiApproved\": false\n    },\n    {\n      \"reference\": \"https://spdx.org/licenses/Entessa.html\",\n      \"isDeprecatedLicenseId\": false,\n      \"detailsUrl\": \"https://spdx.org/licenses/Entessa.json\",\n      \"referenceNumber\": 247,\n      \"name\": \"Entessa Public License v1.0\",\n      \"licenseId\": \"Entessa\",\n      \"seeAlso\": [\n        \"https://opensource.org/licenses/Entessa\"\n      ],\n      \"isOsiApproved\": true\n    },\n    {\n      \"reference\": \"https://spdx.org/licenses/EPICS.html\",\n      \"isDeprecatedLicenseId\": false,\n      \"detailsUrl\": \"https://spdx.org/licenses/EPICS.json\",\n      \"referenceNumber\": 141,\n      \"name\": \"EPICS Open License\",\n      \"licenseId\": \"EPICS\",\n      \"seeAlso\": [\n        \"https://epics.anl.gov/license/open.php\"\n      ],\n      \"isOsiApproved\": false\n    },\n    {\n      \"reference\": \"https://spdx.org/licenses/EPL-1.0.html\",\n      \"isDeprecatedLicenseId\": false,\n      \"detailsUrl\": \"https://spdx.org/licenses/EPL-1.0.json\",\n      \"referenceNumber\": 346,\n      \"name\": \"Eclipse Public License 1.0\",\n      \"licenseId\": \"EPL-1.0\",\n      \"seeAlso\": [\n        \"http://www.eclipse.org/legal/epl-v10.html\",\n        \"https://opensource.org/licenses/EPL-1.0\"\n      ],\n      \"isOsiApproved\": true,\n      \"isFsfLibre\": true\n    },\n    {\n      \"reference\": \"https://spdx.org/licenses/EPL-2.0.html\",\n      \"isDeprecatedLicenseId\": false,\n      \"detailsUrl\": \"https://spdx.org/licenses/EPL-2.0.json\",\n      \"referenceNumber\": 523,\n      \"name\": \"Eclipse Public License 2.0\",\n      \"licenseId\": \"EPL-2.0\",\n      \"seeAlso\": [\n        \"https://www.eclipse.org/legal/epl-2.0\",\n        \"https://www.opensource.org/licenses/EPL-2.0\"\n      ],\n      \"isOsiApproved\": true,\n      \"isFsfLibre\": true\n    },\n    {\n      \"reference\": \"https://spdx.org/licenses/ErlPL-1.1.html\",\n      \"isDeprecatedLicenseId\": false,\n      \"detailsUrl\": \"https://spdx.org/licenses/ErlPL-1.1.json\",\n      \"referenceNumber\": 580,\n      \"name\": \"Erlang Public License v1.1\",\n      \"licenseId\": \"ErlPL-1.1\",\n      \"seeAlso\": [\n        \"http://www.erlang.org/EPLICENSE\"\n      ],\n      \"isOsiApproved\": false\n    },\n    {\n      \"reference\": \"https://spdx.org/licenses/etalab-2.0.html\",\n      \"isDeprecatedLicenseId\": false,\n      \"detailsUrl\": \"https://spdx.org/licenses/etalab-2.0.json\",\n      \"referenceNumber\": 444,\n      \"name\": \"Etalab Open License 2.0\",\n      \"licenseId\": \"etalab-2.0\",\n      \"seeAlso\": [\n        \"https://github.com/DISIC/politique-de-contribution-open-source/blob/master/LICENSE.pdf\",\n        \"https://raw.githubusercontent.com/DISIC/politique-de-contribution-open-source/master/LICENSE\"\n      ],\n      \"isOsiApproved\": false\n    },\n    {\n      \"reference\": \"https://spdx.org/licenses/EUDatagrid.html\",\n      \"isDeprecatedLicenseId\": false,\n      \"detailsUrl\": \"https://spdx.org/licenses/EUDatagrid.json\",\n      \"referenceNumber\": 463,\n      \"name\": \"EU DataGrid Software License\",\n      \"licenseId\": \"EUDatagrid\",\n      \"seeAlso\": [\n        \"http://eu-datagrid.web.cern.ch/eu-datagrid/license.html\",\n        \"https://opensource.org/licenses/EUDatagrid\"\n      ],\n      \"isOsiApproved\": true,\n      \"isFsfLibre\": true\n    },\n    {\n      \"reference\": \"https://spdx.org/licenses/EUPL-1.0.html\",\n      \"isDeprecatedLicenseId\": false,\n      \"detailsUrl\": \"https://spdx.org/licenses/EUPL-1.0.json\",\n      \"referenceNumber\": 639,\n      \"name\": \"European Union Public License 1.0\",\n      \"licenseId\": \"EUPL-1.0\",\n      \"seeAlso\": [\n        \"http://ec.europa.eu/idabc/en/document/7330.html\",\n        \"http://ec.europa.eu/idabc/servlets/Doc027f.pdf?id\\u003d31096\"\n      ],\n      \"isOsiApproved\": false\n    },\n    {\n      \"reference\": \"https://spdx.org/licenses/EUPL-1.1.html\",\n      \"isDeprecatedLicenseId\": false,\n      \"detailsUrl\": \"https://spdx.org/licenses/EUPL-1.1.json\",\n      \"referenceNumber\": 610,\n      \"name\": \"European Union Public License 1.1\",\n      \"licenseId\": \"EUPL-1.1\",\n      \"seeAlso\": [\n        \"https://joinup.ec.europa.eu/software/page/eupl/licence-eupl\",\n        \"https://joinup.ec.europa.eu/sites/default/files/custom-page/attachment/eupl1.1.-licence-en_0.pdf\",\n        \"https://opensource.org/licenses/EUPL-1.1\"\n      ],\n      \"isOsiApproved\": true,\n      \"isFsfLibre\": true\n    },\n    {\n      \"reference\": \"https://spdx.org/licenses/EUPL-1.2.html\",\n      \"isDeprecatedLicenseId\": false,\n      \"detailsUrl\": \"https://spdx.org/licenses/EUPL-1.2.json\",\n      \"referenceNumber\": 150,\n      \"name\": \"European Union Public License 1.2\",\n      \"licenseId\": \"EUPL-1.2\",\n      \"seeAlso\": [\n        \"https://joinup.ec.europa.eu/page/eupl-text-11-12\",\n        \"https://joinup.ec.europa.eu/sites/default/files/custom-page/attachment/eupl_v1.2_en.pdf\",\n        \"https://joinup.ec.europa.eu/sites/default/files/custom-page/attachment/2020-03/EUPL-1.2%20EN.txt\",\n        \"https://joinup.ec.europa.eu/sites/default/files/inline-files/EUPL%20v1_2%20EN(1).txt\",\n        \"http://eur-lex.europa.eu/legal-content/EN/TXT/HTML/?uri\\u003dCELEX:32017D0863\",\n        \"https://opensource.org/licenses/EUPL-1.2\"\n      ],\n      \"isOsiApproved\": true,\n      \"isFsfLibre\": true\n    },\n    {\n      \"reference\": \"https://spdx.org/licenses/Eurosym.html\",\n      \"isDeprecatedLicenseId\": false,\n      \"detailsUrl\": \"https://spdx.org/licenses/Eurosym.json\",\n      \"referenceNumber\": 388,\n      \"name\": \"Eurosym License\",\n      \"licenseId\": \"Eurosym\",\n      \"seeAlso\": [\n        \"https://fedoraproject.org/wiki/Licensing/Eurosym\"\n      ],\n      \"isOsiApproved\": false\n    },\n    {\n      \"reference\": \"https://spdx.org/licenses/Fair.html\",\n      \"isDeprecatedLicenseId\": false,\n      \"detailsUrl\": \"https://spdx.org/licenses/Fair.json\",\n      \"referenceNumber\": 483,\n      \"name\": \"Fair License\",\n      \"licenseId\": \"Fair\",\n      \"seeAlso\": [\n        \"https://web.archive.org/web/20150926120323/http://fairlicense.org/\",\n        \"https://opensource.org/licenses/Fair\"\n      ],\n      \"isOsiApproved\": true\n    },\n    {\n      \"reference\": \"https://spdx.org/licenses/FBM.html\",\n      \"isDeprecatedLicenseId\": false,\n      \"detailsUrl\": \"https://spdx.org/licenses/FBM.json\",\n      \"referenceNumber\": 27,\n      \"name\": \"Fuzzy Bitmap License\",\n      \"licenseId\": \"FBM\",\n      \"seeAlso\": [\n        \"https://github.com/SWI-Prolog/packages-xpce/blob/161a40cd82004f731ba48024f9d30af388a7edf5/src/img/gifwrite.c#L21-L26\"\n      ],\n      \"isOsiApproved\": false\n    },\n    {\n      \"reference\": \"https://spdx.org/licenses/FDK-AAC.html\",\n      \"isDeprecatedLicenseId\": false,\n      \"detailsUrl\": \"https://spdx.org/licenses/FDK-AAC.json\",\n      \"referenceNumber\": 625,\n      \"name\": \"Fraunhofer FDK AAC Codec Library\",\n      \"licenseId\": \"FDK-AAC\",\n      \"seeAlso\": [\n        \"https://fedoraproject.org/wiki/Licensing/FDK-AAC\",\n        \"https://directory.fsf.org/wiki/License:Fdk\"\n      ],\n      \"isOsiApproved\": false\n    },\n    {\n      \"reference\": \"https://spdx.org/licenses/Ferguson-Twofish.html\",\n      \"isDeprecatedLicenseId\": false,\n      \"detailsUrl\": \"https://spdx.org/licenses/Ferguson-Twofish.json\",\n      \"referenceNumber\": 45,\n      \"name\": \"Ferguson Twofish License\",\n      \"licenseId\": \"Ferguson-Twofish\",\n      \"seeAlso\": [\n        \"https://github.com/wernerd/ZRTPCPP/blob/6b3cd8e6783642292bad0c21e3e5e5ce45ff3e03/cryptcommon/twofish.c#L113C3-L127\"\n      ],\n      \"isOsiApproved\": false\n    },\n    {\n      \"reference\": \"https://spdx.org/licenses/Frameworx-1.0.html\",\n      \"isDeprecatedLicenseId\": false,\n      \"detailsUrl\": \"https://spdx.org/licenses/Frameworx-1.0.json\",\n      \"referenceNumber\": 51,\n      \"name\": \"Frameworx Open License 1.0\",\n      \"licenseId\": \"Frameworx-1.0\",\n      \"seeAlso\": [\n        \"https://opensource.org/licenses/Frameworx-1.0\"\n      ],\n      \"isOsiApproved\": true\n    },\n    {\n      \"reference\": \"https://spdx.org/licenses/FreeBSD-DOC.html\",\n      \"isDeprecatedLicenseId\": false,\n      \"detailsUrl\": \"https://spdx.org/licenses/FreeBSD-DOC.json\",\n      \"referenceNumber\": 637,\n      \"name\": \"FreeBSD Documentation License\",\n      \"licenseId\": \"FreeBSD-DOC\",\n      \"seeAlso\": [\n        \"https://www.freebsd.org/copyright/freebsd-doc-license/\"\n      ],\n      \"isOsiApproved\": false\n    },\n    {\n      \"reference\": \"https://spdx.org/licenses/FreeImage.html\",\n      \"isDeprecatedLicenseId\": false,\n      \"detailsUrl\": \"https://spdx.org/licenses/FreeImage.json\",\n      \"referenceNumber\": 139,\n      \"name\": \"FreeImage Public License v1.0\",\n      \"licenseId\": \"FreeImage\",\n      \"seeAlso\": [\n        \"http://freeimage.sourceforge.net/freeimage-license.txt\"\n      ],\n      \"isOsiApproved\": false\n    },\n    {\n      \"reference\": \"https://spdx.org/licenses/FSFAP.html\",\n      \"isDeprecatedLicenseId\": false,\n      \"detailsUrl\": \"https://spdx.org/licenses/FSFAP.json\",\n      \"referenceNumber\": 271,\n      \"name\": \"FSF All Permissive License\",\n      \"licenseId\": \"FSFAP\",\n      \"seeAlso\": [\n        \"https://www.gnu.org/prep/maintain/html_node/License-Notices-for-Other-Files.html\"\n      ],\n      \"isOsiApproved\": false,\n      \"isFsfLibre\": true\n    },\n    {\n      \"reference\": \"https://spdx.org/licenses/FSFAP-no-warranty-disclaimer.html\",\n      \"isDeprecatedLicenseId\": false,\n      \"detailsUrl\": \"https://spdx.org/licenses/FSFAP-no-warranty-disclaimer.json\",\n      \"referenceNumber\": 324,\n      \"name\": \"FSF All Permissive License (without Warranty)\",\n      \"licenseId\": \"FSFAP-no-warranty-disclaimer\",\n      \"seeAlso\": [\n        \"https://git.savannah.gnu.org/cgit/wget.git/tree/util/trunc.c?h\\u003dv1.21.3\\u0026id\\u003d40747a11e44ced5a8ac628a41f879ced3e2ebce9#n6\"\n      ],\n      \"isOsiApproved\": false\n    },\n    {\n      \"reference\": \"https://spdx.org/licenses/FSFUL.html\",\n      \"isDeprecatedLicenseId\": false,\n      \"detailsUrl\": \"https://spdx.org/licenses/FSFUL.json\",\n      \"referenceNumber\": 454,\n      \"name\": \"FSF Unlimited License\",\n      \"licenseId\": \"FSFUL\",\n      \"seeAlso\": [\n        \"https://fedoraproject.org/wiki/Licensing/FSF_Unlimited_License\"\n      ],\n      \"isOsiApproved\": false\n    },\n    {\n      \"reference\": \"https://spdx.org/licenses/FSFULLR.html\",\n      \"isDeprecatedLicenseId\": false,\n      \"detailsUrl\": \"https://spdx.org/licenses/FSFULLR.json\",\n      \"referenceNumber\": 533,\n      \"name\": \"FSF Unlimited License (with License Retention)\",\n      \"licenseId\": \"FSFULLR\",\n      \"seeAlso\": [\n        \"https://fedoraproject.org/wiki/Licensing/FSF_Unlimited_License#License_Retention_Variant\"\n      ],\n      \"isOsiApproved\": false\n    },\n    {\n      \"reference\": \"https://spdx.org/licenses/FSFULLRWD.html\",\n      \"isDeprecatedLicenseId\": false,\n      \"detailsUrl\": \"https://spdx.org/licenses/FSFULLRWD.json\",\n      \"referenceNumber\": 566,\n      \"name\": \"FSF Unlimited License (With License Retention and Warranty Disclaimer)\",\n      \"licenseId\": \"FSFULLRWD\",\n      \"seeAlso\": [\n        \"https://lists.gnu.org/archive/html/autoconf/2012-04/msg00061.html\"\n      ],\n      \"isOsiApproved\": false\n    },\n    {\n      \"reference\": \"https://spdx.org/licenses/FTL.html\",\n      \"isDeprecatedLicenseId\": false,\n      \"detailsUrl\": \"https://spdx.org/licenses/FTL.json\",\n      \"referenceNumber\": 394,\n      \"name\": \"Freetype Project License\",\n      \"licenseId\": \"FTL\",\n      \"seeAlso\": [\n        \"http://freetype.fis.uniroma2.it/FTL.TXT\",\n        \"http://git.savannah.gnu.org/cgit/freetype/freetype2.git/tree/docs/FTL.TXT\",\n        \"http://gitlab.freedesktop.org/freetype/freetype/-/raw/master/docs/FTL.TXT\"\n      ],\n      \"isOsiApproved\": false,\n      \"isFsfLibre\": true\n    },\n    {\n      \"reference\": \"https://spdx.org/licenses/Furuseth.html\",\n      \"isDeprecatedLicenseId\": false,\n      \"detailsUrl\": \"https://spdx.org/licenses/Furuseth.json\",\n      \"referenceNumber\": 396,\n      \"name\": \"Furuseth License\",\n      \"licenseId\": \"Furuseth\",\n      \"seeAlso\": [\n        \"https://git.openldap.org/openldap/openldap/-/blob/master/COPYRIGHT?ref_type\\u003dheads#L39-51\"\n      ],\n      \"isOsiApproved\": false\n    },\n    {\n      \"reference\": \"https://spdx.org/licenses/fwlw.html\",\n      \"isDeprecatedLicenseId\": false,\n      \"detailsUrl\": \"https://spdx.org/licenses/fwlw.json\",\n      \"referenceNumber\": 203,\n      \"name\": \"fwlw License\",\n      \"licenseId\": \"fwlw\",\n      \"seeAlso\": [\n        \"https://mirrors.nic.cz/tex-archive/macros/latex/contrib/fwlw/README\"\n      ],\n      \"isOsiApproved\": false\n    },\n    {\n      \"reference\": \"https://spdx.org/licenses/GCR-docs.html\",\n      \"isDeprecatedLicenseId\": false,\n      \"detailsUrl\": \"https://spdx.org/licenses/GCR-docs.json\",\n      \"referenceNumber\": 418,\n      \"name\": \"Gnome GCR Documentation License\",\n      \"licenseId\": \"GCR-docs\",\n      \"seeAlso\": [\n        \"https://github.com/GNOME/gcr/blob/master/docs/COPYING\"\n      ],\n      \"isOsiApproved\": false\n    },\n    {\n      \"reference\": \"https://spdx.org/licenses/GD.html\",\n      \"isDeprecatedLicenseId\": false,\n      \"detailsUrl\": \"https://spdx.org/licenses/GD.json\",\n      \"referenceNumber\": 352,\n      \"name\": \"GD License\",\n      \"licenseId\": \"GD\",\n      \"seeAlso\": [\n        \"https://libgd.github.io/manuals/2.3.0/files/license-txt.html\"\n      ],\n      \"isOsiApproved\": false\n    },\n    {\n      \"reference\": \"https://spdx.org/licenses/GFDL-1.1.html\",\n      \"isDeprecatedLicenseId\": true,\n      \"detailsUrl\": \"https://spdx.org/licenses/GFDL-1.1.json\",\n      \"referenceNumber\": 368,\n      \"name\": \"GNU Free Documentation License v1.1\",\n      \"licenseId\": \"GFDL-1.1\",\n      \"seeAlso\": [\n        \"https://www.gnu.org/licenses/old-licenses/fdl-1.1.txt\"\n      ],\n      \"isOsiApproved\": false,\n      \"isFsfLibre\": true\n    },\n    {\n      \"reference\": \"https://spdx.org/licenses/GFDL-1.1-invariants-only.html\",\n      \"isDeprecatedLicenseId\": false,\n      \"detailsUrl\": \"https://spdx.org/licenses/GFDL-1.1-invariants-only.json\",\n      \"referenceNumber\": 616,\n      \"name\": \"GNU Free Documentation License v1.1 only - invariants\",\n      \"licenseId\": \"GFDL-1.1-invariants-only\",\n      \"seeAlso\": [\n        \"https://www.gnu.org/licenses/old-licenses/fdl-1.1.txt\"\n      ],\n      \"isOsiApproved\": false\n    },\n    {\n      \"reference\": \"https://spdx.org/licenses/GFDL-1.1-invariants-or-later.html\",\n      \"isDeprecatedLicenseId\": false,\n      \"detailsUrl\": \"https://spdx.org/licenses/GFDL-1.1-invariants-or-later.json\",\n      \"referenceNumber\": 365,\n      \"name\": \"GNU Free Documentation License v1.1 or later - invariants\",\n      \"licenseId\": \"GFDL-1.1-invariants-or-later\",\n      \"seeAlso\": [\n        \"https://www.gnu.org/licenses/old-licenses/fdl-1.1.txt\"\n      ],\n      \"isOsiApproved\": false\n    },\n    {\n      \"reference\": \"https://spdx.org/licenses/GFDL-1.1-no-invariants-only.html\",\n      \"isDeprecatedLicenseId\": false,\n      \"detailsUrl\": \"https://spdx.org/licenses/GFDL-1.1-no-invariants-only.json\",\n      \"referenceNumber\": 373,\n      \"name\": \"GNU Free Documentation License v1.1 only - no invariants\",\n      \"licenseId\": \"GFDL-1.1-no-invariants-only\",\n      \"seeAlso\": [\n        \"https://www.gnu.org/licenses/old-licenses/fdl-1.1.txt\"\n      ],\n      \"isOsiApproved\": false\n    },\n    {\n      \"reference\": \"https://spdx.org/licenses/GFDL-1.1-no-invariants-or-later.html\",\n      \"isDeprecatedLicenseId\": false,\n      \"detailsUrl\": \"https://spdx.org/licenses/GFDL-1.1-no-invariants-or-later.json\",\n      \"referenceNumber\": 234,\n      \"name\": \"GNU Free Documentation License v1.1 or later - no invariants\",\n      \"licenseId\": \"GFDL-1.1-no-invariants-or-later\",\n      \"seeAlso\": [\n        \"https://www.gnu.org/licenses/old-licenses/fdl-1.1.txt\"\n      ],\n      \"isOsiApproved\": false\n    },\n    {\n      \"reference\": \"https://spdx.org/licenses/GFDL-1.1-only.html\",\n      \"isDeprecatedLicenseId\": false,\n      \"detailsUrl\": \"https://spdx.org/licenses/GFDL-1.1-only.json\",\n      \"referenceNumber\": 405,\n      \"name\": \"GNU Free Documentation License v1.1 only\",\n      \"licenseId\": \"GFDL-1.1-only\",\n      \"seeAlso\": [\n        \"https://www.gnu.org/licenses/old-licenses/fdl-1.1.txt\"\n      ],\n      \"isOsiApproved\": false,\n      \"isFsfLibre\": true\n    },\n    {\n      \"reference\": \"https://spdx.org/licenses/GFDL-1.1-or-later.html\",\n      \"isDeprecatedLicenseId\": false,\n      \"detailsUrl\": \"https://spdx.org/licenses/GFDL-1.1-or-later.json\",\n      \"referenceNumber\": 93,\n      \"name\": \"GNU Free Documentation License v1.1 or later\",\n      \"licenseId\": \"GFDL-1.1-or-later\",\n      \"seeAlso\": [\n        \"https://www.gnu.org/licenses/old-licenses/fdl-1.1.txt\"\n      ],\n      \"isOsiApproved\": false,\n      \"isFsfLibre\": true\n    },\n    {\n      \"reference\": \"https://spdx.org/licenses/GFDL-1.2.html\",\n      \"isDeprecatedLicenseId\": true,\n      \"detailsUrl\": \"https://spdx.org/licenses/GFDL-1.2.json\",\n      \"referenceNumber\": 512,\n      \"name\": \"GNU Free Documentation License v1.2\",\n      \"licenseId\": \"GFDL-1.2\",\n      \"seeAlso\": [\n        \"https://www.gnu.org/licenses/old-licenses/fdl-1.2.txt\"\n      ],\n      \"isOsiApproved\": false,\n      \"isFsfLibre\": true\n    },\n    {\n      \"reference\": \"https://spdx.org/licenses/GFDL-1.2-invariants-only.html\",\n      \"isDeprecatedLicenseId\": false,\n      \"detailsUrl\": \"https://spdx.org/licenses/GFDL-1.2-invariants-only.json\",\n      \"referenceNumber\": 411,\n      \"name\": \"GNU Free Documentation License v1.2 only - invariants\",\n      \"licenseId\": \"GFDL-1.2-invariants-only\",\n      \"seeAlso\": [\n        \"https://www.gnu.org/licenses/old-licenses/fdl-1.2.txt\"\n      ],\n      \"isOsiApproved\": false\n    },\n    {\n      \"reference\": \"https://spdx.org/licenses/GFDL-1.2-invariants-or-later.html\",\n      \"isDeprecatedLicenseId\": false,\n      \"detailsUrl\": \"https://spdx.org/licenses/GFDL-1.2-invariants-or-later.json\",\n      \"referenceNumber\": 645,\n      \"name\": \"GNU Free Documentation License v1.2 or later - invariants\",\n      \"licenseId\": \"GFDL-1.2-invariants-or-later\",\n      \"seeAlso\": [\n        \"https://www.gnu.org/licenses/old-licenses/fdl-1.2.txt\"\n      ],\n      \"isOsiApproved\": false\n    },\n    {\n      \"reference\": \"https://spdx.org/licenses/GFDL-1.2-no-invariants-only.html\",\n      \"isDeprecatedLicenseId\": false,\n      \"detailsUrl\": \"https://spdx.org/licenses/GFDL-1.2-no-invariants-only.json\",\n      \"referenceNumber\": 509,\n      \"name\": \"GNU Free Documentation License v1.2 only - no invariants\",\n      \"licenseId\": \"GFDL-1.2-no-invariants-only\",\n      \"seeAlso\": [\n        \"https://www.gnu.org/licenses/old-licenses/fdl-1.2.txt\"\n      ],\n      \"isOsiApproved\": false\n    },\n    {\n      \"reference\": \"https://spdx.org/licenses/GFDL-1.2-no-invariants-or-later.html\",\n      \"isDeprecatedLicenseId\": false,\n      \"detailsUrl\": \"https://spdx.org/licenses/GFDL-1.2-no-invariants-or-later.json\",\n      \"referenceNumber\": 450,\n      \"name\": \"GNU Free Documentation License v1.2 or later - no invariants\",\n      \"licenseId\": \"GFDL-1.2-no-invariants-or-later\",\n      \"seeAlso\": [\n        \"https://www.gnu.org/licenses/old-licenses/fdl-1.2.txt\"\n      ],\n      \"isOsiApproved\": false\n    },\n    {\n      \"reference\": \"https://spdx.org/licenses/GFDL-1.2-only.html\",\n      \"isDeprecatedLicenseId\": false,\n      \"detailsUrl\": \"https://spdx.org/licenses/GFDL-1.2-only.json\",\n      \"referenceNumber\": 541,\n      \"name\": \"GNU Free Documentation License v1.2 only\",\n      \"licenseId\": \"GFDL-1.2-only\",\n      \"seeAlso\": [\n        \"https://www.gnu.org/licenses/old-licenses/fdl-1.2.txt\"\n      ],\n      \"isOsiApproved\": false,\n      \"isFsfLibre\": true\n    },\n    {\n      \"reference\": \"https://spdx.org/licenses/GFDL-1.2-or-later.html\",\n      \"isDeprecatedLicenseId\": false,\n      \"detailsUrl\": \"https://spdx.org/licenses/GFDL-1.2-or-later.json\",\n      \"referenceNumber\": 480,\n      \"name\": \"GNU Free Documentation License v1.2 or later\",\n      \"licenseId\": \"GFDL-1.2-or-later\",\n      \"seeAlso\": [\n        \"https://www.gnu.org/licenses/old-licenses/fdl-1.2.txt\"\n      ],\n      \"isOsiApproved\": false,\n      \"isFsfLibre\": true\n    },\n    {\n      \"reference\": \"https://spdx.org/licenses/GFDL-1.3.html\",\n      \"isDeprecatedLicenseId\": true,\n      \"detailsUrl\": \"https://spdx.org/licenses/GFDL-1.3.json\",\n      \"referenceNumber\": 339,\n      \"name\": \"GNU Free Documentation License v1.3\",\n      \"licenseId\": \"GFDL-1.3\",\n      \"seeAlso\": [\n        \"https://www.gnu.org/licenses/fdl-1.3.txt\"\n      ],\n      \"isOsiApproved\": false,\n      \"isFsfLibre\": true\n    },\n    {\n      \"reference\": \"https://spdx.org/licenses/GFDL-1.3-invariants-only.html\",\n      \"isDeprecatedLicenseId\": false,\n      \"detailsUrl\": \"https://spdx.org/licenses/GFDL-1.3-invariants-only.json\",\n      \"referenceNumber\": 354,\n      \"name\": \"GNU Free Documentation License v1.3 only - invariants\",\n      \"licenseId\": \"GFDL-1.3-invariants-only\",\n      \"seeAlso\": [\n        \"https://www.gnu.org/licenses/fdl-1.3.txt\"\n      ],\n      \"isOsiApproved\": false\n    },\n    {\n      \"reference\": \"https://spdx.org/licenses/GFDL-1.3-invariants-or-later.html\",\n      \"isDeprecatedLicenseId\": false,\n      \"detailsUrl\": \"https://spdx.org/licenses/GFDL-1.3-invariants-or-later.json\",\n      \"referenceNumber\": 466,\n      \"name\": \"GNU Free Documentation License v1.3 or later - invariants\",\n      \"licenseId\": \"GFDL-1.3-invariants-or-later\",\n      \"seeAlso\": [\n        \"https://www.gnu.org/licenses/fdl-1.3.txt\"\n      ],\n      \"isOsiApproved\": false\n    },\n    {\n      \"reference\": \"https://spdx.org/licenses/GFDL-1.3-no-invariants-only.html\",\n      \"isDeprecatedLicenseId\": false,\n      \"detailsUrl\": \"https://spdx.org/licenses/GFDL-1.3-no-invariants-only.json\",\n      \"referenceNumber\": 224,\n      \"name\": \"GNU Free Documentation License v1.3 only - no invariants\",\n      \"licenseId\": \"GFDL-1.3-no-invariants-only\",\n      \"seeAlso\": [\n        \"https://www.gnu.org/licenses/fdl-1.3.txt\"\n      ],\n      \"isOsiApproved\": false\n    },\n    {\n      \"reference\": \"https://spdx.org/licenses/GFDL-1.3-no-invariants-or-later.html\",\n      \"isDeprecatedLicenseId\": false,\n      \"detailsUrl\": \"https://spdx.org/licenses/GFDL-1.3-no-invariants-or-later.json\",\n      \"referenceNumber\": 493,\n      \"name\": \"GNU Free Documentation License v1.3 or later - no invariants\",\n      \"licenseId\": \"GFDL-1.3-no-invariants-or-later\",\n      \"seeAlso\": [\n        \"https://www.gnu.org/licenses/fdl-1.3.txt\"\n      ],\n      \"isOsiApproved\": false\n    },\n    {\n      \"reference\": \"https://spdx.org/licenses/GFDL-1.3-only.html\",\n      \"isDeprecatedLicenseId\": false,\n      \"detailsUrl\": \"https://spdx.org/licenses/GFDL-1.3-only.json\",\n      \"referenceNumber\": 500,\n      \"name\": \"GNU Free Documentation License v1.3 only\",\n      \"licenseId\": \"GFDL-1.3-only\",\n      \"seeAlso\": [\n        \"https://www.gnu.org/licenses/fdl-1.3.txt\"\n      ],\n      \"isOsiApproved\": false,\n      \"isFsfLibre\": true\n    },\n    {\n      \"reference\": \"https://spdx.org/licenses/GFDL-1.3-or-later.html\",\n      \"isDeprecatedLicenseId\": false,\n      \"detailsUrl\": \"https://spdx.org/licenses/GFDL-1.3-or-later.json\",\n      \"referenceNumber\": 414,\n      \"name\": \"GNU Free Documentation License v1.3 or later\",\n      \"licenseId\": \"GFDL-1.3-or-later\",\n      \"seeAlso\": [\n        \"https://www.gnu.org/licenses/fdl-1.3.txt\"\n      ],\n      \"isOsiApproved\": false,\n      \"isFsfLibre\": true\n    },\n    {\n      \"reference\": \"https://spdx.org/licenses/Giftware.html\",\n      \"isDeprecatedLicenseId\": false,\n      \"detailsUrl\": \"https://spdx.org/licenses/Giftware.json\",\n      \"referenceNumber\": 391,\n      \"name\": \"Giftware License\",\n      \"licenseId\": \"Giftware\",\n      \"seeAlso\": [\n        \"http://liballeg.org/license.html#allegro-4-the-giftware-license\"\n      ],\n      \"isOsiApproved\": false\n    },\n    {\n      \"reference\": \"https://spdx.org/licenses/GL2PS.html\",\n      \"isDeprecatedLicenseId\": false,\n      \"detailsUrl\": \"https://spdx.org/licenses/GL2PS.json\",\n      \"referenceNumber\": 648,\n      \"name\": \"GL2PS License\",\n      \"licenseId\": \"GL2PS\",\n      \"seeAlso\": [\n        \"http://www.geuz.org/gl2ps/COPYING.GL2PS\"\n      ],\n      \"isOsiApproved\": false\n    },\n    {\n      \"reference\": \"https://spdx.org/licenses/Glide.html\",\n      \"isDeprecatedLicenseId\": false,\n      \"detailsUrl\": \"https://spdx.org/licenses/Glide.json\",\n      \"referenceNumber\": 95,\n      \"name\": \"3dfx Glide License\",\n      \"licenseId\": \"Glide\",\n      \"seeAlso\": [\n        \"http://www.users.on.net/~triforce/glidexp/COPYING.txt\"\n      ],\n      \"isOsiApproved\": false\n    },\n    {\n      \"reference\": \"https://spdx.org/licenses/Glulxe.html\",\n      \"isDeprecatedLicenseId\": false,\n      \"detailsUrl\": \"https://spdx.org/licenses/Glulxe.json\",\n      \"referenceNumber\": 538,\n      \"name\": \"Glulxe License\",\n      \"licenseId\": \"Glulxe\",\n      \"seeAlso\": [\n        \"https://fedoraproject.org/wiki/Licensing/Glulxe\"\n      ],\n      \"isOsiApproved\": false\n    },\n    {\n      \"reference\": \"https://spdx.org/licenses/GLWTPL.html\",\n      \"isDeprecatedLicenseId\": false,\n      \"detailsUrl\": \"https://spdx.org/licenses/GLWTPL.json\",\n      \"referenceNumber\": 37,\n      \"name\": \"Good Luck With That Public License\",\n      \"licenseId\": \"GLWTPL\",\n      \"seeAlso\": [\n        \"https://github.com/me-shaon/GLWTPL/commit/da5f6bc734095efbacb442c0b31e33a65b9d6e85\"\n      ],\n      \"isOsiApproved\": false\n    },\n    {\n      \"reference\": \"https://spdx.org/licenses/gnuplot.html\",\n      \"isDeprecatedLicenseId\": false,\n      \"detailsUrl\": \"https://spdx.org/licenses/gnuplot.json\",\n      \"referenceNumber\": 453,\n      \"name\": \"gnuplot License\",\n      \"licenseId\": \"gnuplot\",\n      \"seeAlso\": [\n        \"https://fedoraproject.org/wiki/Licensing/Gnuplot\"\n      ],\n      \"isOsiApproved\": false,\n      \"isFsfLibre\": true\n    },\n    {\n      \"reference\": \"https://spdx.org/licenses/GPL-1.0.html\",\n      \"isDeprecatedLicenseId\": true,\n      \"detailsUrl\": \"https://spdx.org/licenses/GPL-1.0.json\",\n      \"referenceNumber\": 319,\n      \"name\": \"GNU General Public License v1.0 only\",\n      \"licenseId\": \"GPL-1.0\",\n      \"seeAlso\": [\n        \"https://www.gnu.org/licenses/old-licenses/gpl-1.0-standalone.html\"\n      ],\n      \"isOsiApproved\": false\n    },\n    {\n      \"reference\": \"https://spdx.org/licenses/GPL-1.0+.html\",\n      \"isDeprecatedLicenseId\": true,\n      \"detailsUrl\": \"https://spdx.org/licenses/GPL-1.0+.json\",\n      \"referenceNumber\": 273,\n      \"name\": \"GNU General Public License v1.0 or later\",\n      \"licenseId\": \"GPL-1.0+\",\n      \"seeAlso\": [\n        \"https://www.gnu.org/licenses/old-licenses/gpl-1.0-standalone.html\"\n      ],\n      \"isOsiApproved\": false\n    },\n    {\n      \"reference\": \"https://spdx.org/licenses/GPL-1.0-only.html\",\n      \"isDeprecatedLicenseId\": false,\n      \"detailsUrl\": \"https://spdx.org/licenses/GPL-1.0-only.json\",\n      \"referenceNumber\": 123,\n      \"name\": \"GNU General Public License v1.0 only\",\n      \"licenseId\": \"GPL-1.0-only\",\n      \"seeAlso\": [\n        \"https://www.gnu.org/licenses/old-licenses/gpl-1.0-standalone.html\"\n      ],\n      \"isOsiApproved\": false\n    },\n    {\n      \"reference\": \"https://spdx.org/licenses/GPL-1.0-or-later.html\",\n      \"isDeprecatedLicenseId\": false,\n      \"detailsUrl\": \"https://spdx.org/licenses/GPL-1.0-or-later.json\",\n      \"referenceNumber\": 138,\n      \"name\": \"GNU General Public License v1.0 or later\",\n      \"licenseId\": \"GPL-1.0-or-later\",\n      \"seeAlso\": [\n        \"https://www.gnu.org/licenses/old-licenses/gpl-1.0-standalone.html\"\n      ],\n      \"isOsiApproved\": false\n    },\n    {\n      \"reference\": \"https://spdx.org/licenses/GPL-2.0.html\",\n      \"isDeprecatedLicenseId\": true,\n      \"detailsUrl\": \"https://spdx.org/licenses/GPL-2.0.json\",\n      \"referenceNumber\": 159,\n      \"name\": \"GNU General Public License v2.0 only\",\n      \"licenseId\": \"GPL-2.0\",\n      \"seeAlso\": [\n        \"https://www.gnu.org/licenses/old-licenses/gpl-2.0-standalone.html\",\n        \"https://opensource.org/licenses/GPL-2.0\"\n      ],\n      \"isOsiApproved\": true,\n      \"isFsfLibre\": true\n    },\n    {\n      \"reference\": \"https://spdx.org/licenses/GPL-2.0+.html\",\n      \"isDeprecatedLicenseId\": true,\n      \"detailsUrl\": \"https://spdx.org/licenses/GPL-2.0+.json\",\n      \"referenceNumber\": 633,\n      \"name\": \"GNU General Public License v2.0 or later\",\n      \"licenseId\": \"GPL-2.0+\",\n      \"seeAlso\": [\n        \"https://www.gnu.org/licenses/old-licenses/gpl-2.0-standalone.html\",\n        \"https://opensource.org/licenses/GPL-2.0\"\n      ],\n      \"isOsiApproved\": true,\n      \"isFsfLibre\": true\n    },\n    {\n      \"reference\": \"https://spdx.org/licenses/GPL-2.0-only.html\",\n      \"isDeprecatedLicenseId\": false,\n      \"detailsUrl\": \"https://spdx.org/licenses/GPL-2.0-only.json\",\n      \"referenceNumber\": 318,\n      \"name\": \"GNU General Public License v2.0 only\",\n      \"licenseId\": \"GPL-2.0-only\",\n      \"seeAlso\": [\n        \"https://www.gnu.org/licenses/old-licenses/gpl-2.0-standalone.html\",\n        \"https://www.gnu.org/licenses/old-licenses/gpl-2.0.txt\",\n        \"https://opensource.org/licenses/GPL-2.0\"\n      ],\n      \"isOsiApproved\": true,\n      \"isFsfLibre\": true\n    },\n    {\n      \"reference\": \"https://spdx.org/licenses/GPL-2.0-or-later.html\",\n      \"isDeprecatedLicenseId\": false,\n      \"detailsUrl\": \"https://spdx.org/licenses/GPL-2.0-or-later.json\",\n      \"referenceNumber\": 629,\n      \"name\": \"GNU General Public License v2.0 or later\",\n      \"licenseId\": \"GPL-2.0-or-later\",\n      \"seeAlso\": [\n        \"https://www.gnu.org/licenses/old-licenses/gpl-2.0-standalone.html\",\n        \"https://opensource.org/licenses/GPL-2.0\"\n      ],\n      \"isOsiApproved\": true,\n      \"isFsfLibre\": true\n    },\n    {\n      \"reference\": \"https://spdx.org/licenses/GPL-2.0-with-autoconf-exception.html\",\n      \"isDeprecatedLicenseId\": true,\n      \"detailsUrl\": \"https://spdx.org/licenses/GPL-2.0-with-autoconf-exception.json\",\n      \"referenceNumber\": 48,\n      \"name\": \"GNU General Public License v2.0 w/Autoconf exception\",\n      \"licenseId\": \"GPL-2.0-with-autoconf-exception\",\n      \"seeAlso\": [\n        \"http://ac-archive.sourceforge.net/doc/copyright.html\"\n      ],\n      \"isOsiApproved\": false\n    },\n    {\n      \"reference\": \"https://spdx.org/licenses/GPL-2.0-with-bison-exception.html\",\n      \"isDeprecatedLicenseId\": true,\n      \"detailsUrl\": \"https://spdx.org/licenses/GPL-2.0-with-bison-exception.json\",\n      \"referenceNumber\": 292,\n      \"name\": \"GNU General Public License v2.0 w/Bison exception\",\n      \"licenseId\": \"GPL-2.0-with-bison-exception\",\n      \"seeAlso\": [\n        \"http://git.savannah.gnu.org/cgit/bison.git/tree/data/yacc.c?id\\u003d193d7c7054ba7197b0789e14965b739162319b5e#n141\"\n      ],\n      \"isOsiApproved\": false\n    },\n    {\n      \"reference\": \"https://spdx.org/licenses/GPL-2.0-with-classpath-exception.html\",\n      \"isDeprecatedLicenseId\": true,\n      \"detailsUrl\": \"https://spdx.org/licenses/GPL-2.0-with-classpath-exception.json\",\n      \"referenceNumber\": 424,\n      \"name\": \"GNU General Public License v2.0 w/Classpath exception\",\n      \"licenseId\": \"GPL-2.0-with-classpath-exception\",\n      \"seeAlso\": [\n        \"https://www.gnu.org/software/classpath/license.html\"\n      ],\n      \"isOsiApproved\": false\n    },\n    {\n      \"reference\": \"https://spdx.org/licenses/GPL-2.0-with-font-exception.html\",\n      \"isDeprecatedLicenseId\": true,\n      \"detailsUrl\": \"https://spdx.org/licenses/GPL-2.0-with-font-exception.json\",\n      \"referenceNumber\": 438,\n      \"name\": \"GNU General Public License v2.0 w/Font exception\",\n      \"licenseId\": \"GPL-2.0-with-font-exception\",\n      \"seeAlso\": [\n        \"https://www.gnu.org/licenses/gpl-faq.html#FontException\"\n      ],\n      \"isOsiApproved\": false\n    },\n    {\n      \"reference\": \"https://spdx.org/licenses/GPL-2.0-with-GCC-exception.html\",\n      \"isDeprecatedLicenseId\": true,\n      \"detailsUrl\": \"https://spdx.org/licenses/GPL-2.0-with-GCC-exception.json\",\n      \"referenceNumber\": 76,\n      \"name\": \"GNU General Public License v2.0 w/GCC Runtime Library exception\",\n      \"licenseId\": \"GPL-2.0-with-GCC-exception\",\n      \"seeAlso\": [\n        \"https://gcc.gnu.org/git/?p\\u003dgcc.git;a\\u003dblob;f\\u003dgcc/libgcc1.c;h\\u003d762f5143fc6eed57b6797c82710f3538aa52b40b;hb\\u003dcb143a3ce4fb417c68f5fa2691a1b1b1053dfba9#l10\"\n      ],\n      \"isOsiApproved\": false\n    },\n    {\n      \"reference\": \"https://spdx.org/licenses/GPL-3.0.html\",\n      \"isDeprecatedLicenseId\": true,\n      \"detailsUrl\": \"https://spdx.org/licenses/GPL-3.0.json\",\n      \"referenceNumber\": 632,\n      \"name\": \"GNU General Public License v3.0 only\",\n      \"licenseId\": \"GPL-3.0\",\n      \"seeAlso\": [\n        \"https://www.gnu.org/licenses/gpl-3.0-standalone.html\",\n        \"https://opensource.org/licenses/GPL-3.0\"\n      ],\n      \"isOsiApproved\": true,\n      \"isFsfLibre\": true\n    },\n    {\n      \"reference\": \"https://spdx.org/licenses/GPL-3.0+.html\",\n      \"isDeprecatedLicenseId\": true,\n      \"detailsUrl\": \"https://spdx.org/licenses/GPL-3.0+.json\",\n      \"referenceNumber\": 72,\n      \"name\": \"GNU General Public License v3.0 or later\",\n      \"licenseId\": \"GPL-3.0+\",\n      \"seeAlso\": [\n        \"https://www.gnu.org/licenses/gpl-3.0-standalone.html\",\n        \"https://opensource.org/licenses/GPL-3.0\"\n      ],\n      \"isOsiApproved\": true,\n      \"isFsfLibre\": true\n    },\n    {\n      \"reference\": \"https://spdx.org/licenses/GPL-3.0-only.html\",\n      \"isDeprecatedLicenseId\": false,\n      \"detailsUrl\": \"https://spdx.org/licenses/GPL-3.0-only.json\",\n      \"referenceNumber\": 81,\n      \"name\": \"GNU General Public License v3.0 only\",\n      \"licenseId\": \"GPL-3.0-only\",\n      \"seeAlso\": [\n        \"https://www.gnu.org/licenses/gpl-3.0-standalone.html\",\n        \"https://opensource.org/licenses/GPL-3.0\"\n      ],\n      \"isOsiApproved\": true,\n      \"isFsfLibre\": true\n    },\n    {\n      \"reference\": \"https://spdx.org/licenses/GPL-3.0-or-later.html\",\n      \"isDeprecatedLicenseId\": false,\n      \"detailsUrl\": \"https://spdx.org/licenses/GPL-3.0-or-later.json\",\n      \"referenceNumber\": 378,\n      \"name\": \"GNU General Public License v3.0 or later\",\n      \"licenseId\": \"GPL-3.0-or-later\",\n      \"seeAlso\": [\n        \"https://www.gnu.org/licenses/gpl-3.0-standalone.html\",\n        \"https://opensource.org/licenses/GPL-3.0\"\n      ],\n      \"isOsiApproved\": true,\n      \"isFsfLibre\": true\n    },\n    {\n      \"reference\": \"https://spdx.org/licenses/GPL-3.0-with-autoconf-exception.html\",\n      \"isDeprecatedLicenseId\": true,\n      \"detailsUrl\": \"https://spdx.org/licenses/GPL-3.0-with-autoconf-exception.json\",\n      \"referenceNumber\": 122,\n      \"name\": \"GNU General Public License v3.0 w/Autoconf exception\",\n      \"licenseId\": \"GPL-3.0-with-autoconf-exception\",\n      \"seeAlso\": [\n        \"https://www.gnu.org/licenses/autoconf-exception-3.0.html\"\n      ],\n      \"isOsiApproved\": false\n    },\n    {\n      \"reference\": \"https://spdx.org/licenses/GPL-3.0-with-GCC-exception.html\",\n      \"isDeprecatedLicenseId\": true,\n      \"detailsUrl\": \"https://spdx.org/licenses/GPL-3.0-with-GCC-exception.json\",\n      \"referenceNumber\": 458,\n      \"name\": \"GNU General Public License v3.0 w/GCC Runtime Library exception\",\n      \"licenseId\": \"GPL-3.0-with-GCC-exception\",\n      \"seeAlso\": [\n        \"https://www.gnu.org/licenses/gcc-exception-3.1.html\"\n      ],\n      \"isOsiApproved\": true\n    },\n    {\n      \"reference\": \"https://spdx.org/licenses/Graphics-Gems.html\",\n      \"isDeprecatedLicenseId\": false,\n      \"detailsUrl\": \"https://spdx.org/licenses/Graphics-Gems.json\",\n      \"referenceNumber\": 147,\n      \"name\": \"Graphics Gems License\",\n      \"licenseId\": \"Graphics-Gems\",\n      \"seeAlso\": [\n        \"https://github.com/erich666/GraphicsGems/blob/master/LICENSE.md\"\n      ],\n      \"isOsiApproved\": false\n    },\n    {\n      \"reference\": \"https://spdx.org/licenses/gSOAP-1.3b.html\",\n      \"isDeprecatedLicenseId\": false,\n      \"detailsUrl\": \"https://spdx.org/licenses/gSOAP-1.3b.json\",\n      \"referenceNumber\": 576,\n      \"name\": \"gSOAP Public License v1.3b\",\n      \"licenseId\": \"gSOAP-1.3b\",\n      \"seeAlso\": [\n        \"http://www.cs.fsu.edu/~engelen/license.html\"\n      ],\n      \"isOsiApproved\": false\n    },\n    {\n      \"reference\": \"https://spdx.org/licenses/gtkbook.html\",\n      \"isDeprecatedLicenseId\": false,\n      \"detailsUrl\": \"https://spdx.org/licenses/gtkbook.json\",\n      \"referenceNumber\": 588,\n      \"name\": \"gtkbook License\",\n      \"licenseId\": \"gtkbook\",\n      \"seeAlso\": [\n        \"https://github.com/slogan621/gtkbook\",\n        \"https://github.com/oetiker/rrdtool-1.x/blob/master/src/plbasename.c#L8-L11\"\n      ],\n      \"isOsiApproved\": false\n    },\n    {\n      \"reference\": \"https://spdx.org/licenses/Gutmann.html\",\n      \"isDeprecatedLicenseId\": false,\n      \"detailsUrl\": \"https://spdx.org/licenses/Gutmann.json\",\n      \"referenceNumber\": 89,\n      \"name\": \"Gutmann License\",\n      \"licenseId\": \"Gutmann\",\n      \"seeAlso\": [\n        \"https://www.cs.auckland.ac.nz/~pgut001/dumpasn1.c\"\n      ],\n      \"isOsiApproved\": false\n    },\n    {\n      \"reference\": \"https://spdx.org/licenses/HaskellReport.html\",\n      \"isDeprecatedLicenseId\": false,\n      \"detailsUrl\": \"https://spdx.org/licenses/HaskellReport.json\",\n      \"referenceNumber\": 308,\n      \"name\": \"Haskell Language Report License\",\n      \"licenseId\": \"HaskellReport\",\n      \"seeAlso\": [\n        \"https://fedoraproject.org/wiki/Licensing/Haskell_Language_Report_License\"\n      ],\n      \"isOsiApproved\": false\n    },\n    {\n      \"reference\": \"https://spdx.org/licenses/hdparm.html\",\n      \"isDeprecatedLicenseId\": false,\n      \"detailsUrl\": \"https://spdx.org/licenses/hdparm.json\",\n      \"referenceNumber\": 581,\n      \"name\": \"hdparm License\",\n      \"licenseId\": \"hdparm\",\n      \"seeAlso\": [\n        \"https://github.com/Distrotech/hdparm/blob/4517550db29a91420fb2b020349523b1b4512df2/LICENSE.TXT\"\n      ],\n      \"isOsiApproved\": false\n    },\n    {\n      \"reference\": \"https://spdx.org/licenses/Hippocratic-2.1.html\",\n      \"isDeprecatedLicenseId\": false,\n      \"detailsUrl\": \"https://spdx.org/licenses/Hippocratic-2.1.json\",\n      \"referenceNumber\": 570,\n      \"name\": \"Hippocratic License 2.1\",\n      \"licenseId\": \"Hippocratic-2.1\",\n      \"seeAlso\": [\n        \"https://firstdonoharm.dev/version/2/1/license.html\",\n        \"https://github.com/EthicalSource/hippocratic-license/blob/58c0e646d64ff6fbee275bfe2b9492f914e3ab2a/LICENSE.txt\"\n      ],\n      \"isOsiApproved\": false\n    },\n    {\n      \"reference\": \"https://spdx.org/licenses/HP-1986.html\",\n      \"isDeprecatedLicenseId\": false,\n      \"detailsUrl\": \"https://spdx.org/licenses/HP-1986.json\",\n      \"referenceNumber\": 3,\n      \"name\": \"Hewlett-Packard 1986 License\",\n      \"licenseId\": \"HP-1986\",\n      \"seeAlso\": [\n        \"https://sourceware.org/git/?p\\u003dnewlib-cygwin.git;a\\u003dblob;f\\u003dnewlib/libc/machine/hppa/memchr.S;h\\u003d1cca3e5e8867aa4bffef1f75a5c1bba25c0c441e;hb\\u003dHEAD#l2\"\n      ],\n      \"isOsiApproved\": false\n    },\n    {\n      \"reference\": \"https://spdx.org/licenses/HP-1989.html\",\n      \"isDeprecatedLicenseId\": false,\n      \"detailsUrl\": \"https://spdx.org/licenses/HP-1989.json\",\n      \"referenceNumber\": 43,\n      \"name\": \"Hewlett-Packard 1989 License\",\n      \"licenseId\": \"HP-1989\",\n      \"seeAlso\": [\n        \"https://github.com/bleargh45/Data-UUID/blob/master/LICENSE\"\n      ],\n      \"isOsiApproved\": false\n    },\n    {\n      \"reference\": \"https://spdx.org/licenses/HPND.html\",\n      \"isDeprecatedLicenseId\": false,\n      \"detailsUrl\": \"https://spdx.org/licenses/HPND.json\",\n      \"referenceNumber\": 640,\n      \"name\": \"Historical Permission Notice and Disclaimer\",\n      \"licenseId\": \"HPND\",\n      \"seeAlso\": [\n        \"https://opensource.org/licenses/HPND\",\n        \"http://lists.opensource.org/pipermail/license-discuss_lists.opensource.org/2002-November/006304.html\"\n      ],\n      \"isOsiApproved\": true,\n      \"isFsfLibre\": true\n    },\n    {\n      \"reference\": \"https://spdx.org/licenses/HPND-DEC.html\",\n      \"isDeprecatedLicenseId\": false,\n      \"detailsUrl\": \"https://spdx.org/licenses/HPND-DEC.json\",\n      \"referenceNumber\": 44,\n      \"name\": \"Historical Permission Notice and Disclaimer - DEC variant\",\n      \"licenseId\": \"HPND-DEC\",\n      \"seeAlso\": [\n        \"https://gitlab.freedesktop.org/xorg/app/xkbcomp/-/blob/master/COPYING?ref_type\\u003dheads#L69\"\n      ],\n      \"isOsiApproved\": false\n    },\n    {\n      \"reference\": \"https://spdx.org/licenses/HPND-doc.html\",\n      \"isDeprecatedLicenseId\": false,\n      \"detailsUrl\": \"https://spdx.org/licenses/HPND-doc.json\",\n      \"referenceNumber\": 310,\n      \"name\": \"Historical Permission Notice and Disclaimer - documentation variant\",\n      \"licenseId\": \"HPND-doc\",\n      \"seeAlso\": [\n        \"https://gitlab.freedesktop.org/xorg/lib/libxext/-/blob/master/COPYING?ref_type\\u003dheads#L185-197\",\n        \"https://gitlab.freedesktop.org/xorg/lib/libxtst/-/blob/master/COPYING?ref_type\\u003dheads#L70-77\"\n      ],\n      \"isOsiApproved\": false\n    },\n    {\n      \"reference\": \"https://spdx.org/licenses/HPND-doc-sell.html\",\n      \"isDeprecatedLicenseId\": false,\n      \"detailsUrl\": \"https://spdx.org/licenses/HPND-doc-sell.json\",\n      \"referenceNumber\": 522,\n      \"name\": \"Historical Permission Notice and Disclaimer - documentation sell variant\",\n      \"licenseId\": \"HPND-doc-sell\",\n      \"seeAlso\": [\n        \"https://gitlab.freedesktop.org/xorg/lib/libxtst/-/blob/master/COPYING?ref_type\\u003dheads#L108-117\",\n        \"https://gitlab.freedesktop.org/xorg/lib/libxext/-/blob/master/COPYING?ref_type\\u003dheads#L153-162\"\n      ],\n      \"isOsiApproved\": false\n    },\n    {\n      \"reference\": \"https://spdx.org/licenses/HPND-export-US.html\",\n      \"isDeprecatedLicenseId\": false,\n      \"detailsUrl\": \"https://spdx.org/licenses/HPND-export-US.json\",\n      \"referenceNumber\": 305,\n      \"name\": \"HPND with US Government export control warning\",\n      \"licenseId\": \"HPND-export-US\",\n      \"seeAlso\": [\n        \"https://www.kermitproject.org/ck90.html#source\"\n      ],\n      \"isOsiApproved\": false\n    },\n    {\n      \"reference\": \"https://spdx.org/licenses/HPND-export-US-acknowledgement.html\",\n      \"isDeprecatedLicenseId\": false,\n      \"detailsUrl\": \"https://spdx.org/licenses/HPND-export-US-acknowledgement.json\",\n      \"referenceNumber\": 416,\n      \"name\": \"HPND with US Government export control warning and acknowledgment\",\n      \"licenseId\": \"HPND-export-US-acknowledgement\",\n      \"seeAlso\": [\n        \"https://github.com/krb5/krb5/blob/krb5-1.21.2-final/NOTICE#L831-L852\",\n        \"https://web.mit.edu/kerberos/krb5-1.21/doc/mitK5license.html\"\n      ],\n      \"isOsiApproved\": false\n    },\n    {\n      \"reference\": \"https://spdx.org/licenses/HPND-export-US-modify.html\",\n      \"isDeprecatedLicenseId\": false,\n      \"detailsUrl\": \"https://spdx.org/licenses/HPND-export-US-modify.json\",\n      \"referenceNumber\": 153,\n      \"name\": \"HPND with US Government export control warning and modification rqmt\",\n      \"licenseId\": \"HPND-export-US-modify\",\n      \"seeAlso\": [\n        \"https://github.com/krb5/krb5/blob/krb5-1.21.2-final/NOTICE#L1157-L1182\",\n        \"https://github.com/pythongssapi/k5test/blob/v0.10.3/K5TEST-LICENSE.txt\"\n      ],\n      \"isOsiApproved\": false\n    },\n    {\n      \"reference\": \"https://spdx.org/licenses/HPND-export2-US.html\",\n      \"isDeprecatedLicenseId\": false,\n      \"detailsUrl\": \"https://spdx.org/licenses/HPND-export2-US.json\",\n      \"referenceNumber\": 621,\n      \"name\": \"HPND with US Government export control and 2 disclaimers\",\n      \"licenseId\": \"HPND-export2-US\",\n      \"seeAlso\": [\n        \"https://github.com/krb5/krb5/blob/krb5-1.21.2-final/NOTICE#L111-L133\",\n        \"https://web.mit.edu/kerberos/krb5-1.21/doc/mitK5license.html\"\n      ],\n      \"isOsiApproved\": false\n    },\n    {\n      \"reference\": \"https://spdx.org/licenses/HPND-Fenneberg-Livingston.html\",\n      \"isDeprecatedLicenseId\": false,\n      \"detailsUrl\": \"https://spdx.org/licenses/HPND-Fenneberg-Livingston.json\",\n      \"referenceNumber\": 529,\n      \"name\": \"Historical Permission Notice and Disclaimer - Fenneberg-Livingston variant\",\n      \"licenseId\": \"HPND-Fenneberg-Livingston\",\n      \"seeAlso\": [\n        \"https://github.com/FreeRADIUS/freeradius-client/blob/master/COPYRIGHT#L32\",\n        \"https://github.com/radcli/radcli/blob/master/COPYRIGHT#L34\"\n      ],\n      \"isOsiApproved\": false\n    },\n    {\n      \"reference\": \"https://spdx.org/licenses/HPND-INRIA-IMAG.html\",\n      \"isDeprecatedLicenseId\": false,\n      \"detailsUrl\": \"https://spdx.org/licenses/HPND-INRIA-IMAG.json\",\n      \"referenceNumber\": 70,\n      \"name\": \"Historical Permission Notice and Disclaimer    - INRIA-IMAG variant\",\n      \"licenseId\": \"HPND-INRIA-IMAG\",\n      \"seeAlso\": [\n        \"https://github.com/ppp-project/ppp/blob/master/pppd/ipv6cp.c#L75-L83\"\n      ],\n      \"isOsiApproved\": false\n    },\n    {\n      \"reference\": \"https://spdx.org/licenses/HPND-Intel.html\",\n      \"isDeprecatedLicenseId\": false,\n      \"detailsUrl\": \"https://spdx.org/licenses/HPND-Intel.json\",\n      \"referenceNumber\": 526,\n      \"name\": \"Historical Permission Notice and Disclaimer - Intel variant\",\n      \"licenseId\": \"HPND-Intel\",\n      \"seeAlso\": [\n        \"https://sourceware.org/git/?p\\u003dnewlib-cygwin.git;a\\u003dblob;f\\u003dnewlib/libc/machine/i960/memcpy.S;hb\\u003dHEAD\"\n      ],\n      \"isOsiApproved\": false\n    },\n    {\n      \"reference\": \"https://spdx.org/licenses/HPND-Kevlin-Henney.html\",\n      \"isDeprecatedLicenseId\": false,\n      \"detailsUrl\": \"https://spdx.org/licenses/HPND-Kevlin-Henney.json\",\n      \"referenceNumber\": 559,\n      \"name\": \"Historical Permission Notice and Disclaimer - Kevlin Henney variant\",\n      \"licenseId\": \"HPND-Kevlin-Henney\",\n      \"seeAlso\": [\n        \"https://github.com/mruby/mruby/blob/83d12f8d52522cdb7c8cc46fad34821359f453e6/mrbgems/mruby-dir/src/Win/dirent.c#L127-L140\"\n      ],\n      \"isOsiApproved\": false\n    },\n    {\n      \"reference\": \"https://spdx.org/licenses/HPND-Markus-Kuhn.html\",\n      \"isDeprecatedLicenseId\": false,\n      \"detailsUrl\": \"https://spdx.org/licenses/HPND-Markus-Kuhn.json\",\n      \"referenceNumber\": 155,\n      \"name\": \"Historical Permission Notice and Disclaimer - Markus Kuhn variant\",\n      \"licenseId\": \"HPND-Markus-Kuhn\",\n      \"seeAlso\": [\n        \"https://www.cl.cam.ac.uk/~mgk25/ucs/wcwidth.c\",\n        \"https://sourceware.org/git/?p\\u003dbinutils-gdb.git;a\\u003dblob;f\\u003dreadline/readline/support/wcwidth.c;h\\u003d0f5ec995796f4813abbcf4972aec0378ab74722a;hb\\u003dHEAD#l55\"\n      ],\n      \"isOsiApproved\": false\n    },\n    {\n      \"reference\": \"https://spdx.org/licenses/HPND-merchantability-variant.html\",\n      \"isDeprecatedLicenseId\": false,\n      \"detailsUrl\": \"https://spdx.org/licenses/HPND-merchantability-variant.json\",\n      \"referenceNumber\": 407,\n      \"name\": \"Historical Permission Notice and Disclaimer - merchantability variant\",\n      \"licenseId\": \"HPND-merchantability-variant\",\n      \"seeAlso\": [\n        \"https://sourceware.org/git/?p\\u003dnewlib-cygwin.git;a\\u003dblob;f\\u003dnewlib/libc/misc/fini.c;hb\\u003dHEAD\"\n      ],\n      \"isOsiApproved\": false\n    },\n    {\n      \"reference\": \"https://spdx.org/licenses/HPND-MIT-disclaimer.html\",\n      \"isDeprecatedLicenseId\": false,\n      \"detailsUrl\": \"https://spdx.org/licenses/HPND-MIT-disclaimer.json\",\n      \"referenceNumber\": 75,\n      \"name\": \"Historical Permission Notice and Disclaimer with MIT disclaimer\",\n      \"licenseId\": \"HPND-MIT-disclaimer\",\n      \"seeAlso\": [\n        \"https://metacpan.org/release/NLNETLABS/Net-DNS-SEC-1.22/source/LICENSE\"\n      ],\n      \"isOsiApproved\": false\n    },\n    {\n      \"reference\": \"https://spdx.org/licenses/HPND-Pbmplus.html\",\n      \"isDeprecatedLicenseId\": false,\n      \"detailsUrl\": \"https://spdx.org/licenses/HPND-Pbmplus.json\",\n      \"referenceNumber\": 13,\n      \"name\": \"Historical Permission Notice and Disclaimer - Pbmplus variant\",\n      \"licenseId\": \"HPND-Pbmplus\",\n      \"seeAlso\": [\n        \"https://sourceforge.net/p/netpbm/code/HEAD/tree/super_stable/netpbm.c#l8\"\n      ],\n      \"isOsiApproved\": false\n    },\n    {\n      \"reference\": \"https://spdx.org/licenses/HPND-sell-MIT-disclaimer-xserver.html\",\n      \"isDeprecatedLicenseId\": false,\n      \"detailsUrl\": \"https://spdx.org/licenses/HPND-sell-MIT-disclaimer-xserver.json\",\n      \"referenceNumber\": 400,\n      \"name\": \"Historical Permission Notice and Disclaimer - sell xserver variant with MIT disclaimer\",\n      \"licenseId\": \"HPND-sell-MIT-disclaimer-xserver\",\n      \"seeAlso\": [\n        \"https://gitlab.freedesktop.org/xorg/xserver/-/blob/master/COPYING?ref_type\\u003dheads#L1781\"\n      ],\n      \"isOsiApproved\": false\n    },\n    {\n      \"reference\": \"https://spdx.org/licenses/HPND-sell-regexpr.html\",\n      \"isDeprecatedLicenseId\": false,\n      \"detailsUrl\": \"https://spdx.org/licenses/HPND-sell-regexpr.json\",\n      \"referenceNumber\": 11,\n      \"name\": \"Historical Permission Notice and Disclaimer - sell regexpr variant\",\n      \"licenseId\": \"HPND-sell-regexpr\",\n      \"seeAlso\": [\n        \"https://gitlab.com/bacula-org/bacula/-/blob/Branch-11.0/bacula/LICENSE-FOSS?ref_type\\u003dheads#L245\"\n      ],\n      \"isOsiApproved\": false\n    },\n    {\n      \"reference\": \"https://spdx.org/licenses/HPND-sell-variant.html\",\n      \"isDeprecatedLicenseId\": false,\n      \"detailsUrl\": \"https://spdx.org/licenses/HPND-sell-variant.json\",\n      \"referenceNumber\": 595,\n      \"name\": \"Historical Permission Notice and Disclaimer - sell variant\",\n      \"licenseId\": \"HPND-sell-variant\",\n      \"seeAlso\": [\n        \"https://git.kernel.org/pub/scm/linux/kernel/git/torvalds/linux.git/tree/net/sunrpc/auth_gss/gss_generic_token.c?h\\u003dv4.19\"\n      ],\n      \"isOsiApproved\": false\n    },\n    {\n      \"reference\": \"https://spdx.org/licenses/HPND-sell-variant-MIT-disclaimer.html\",\n      \"isDeprecatedLicenseId\": false,\n      \"detailsUrl\": \"https://spdx.org/licenses/HPND-sell-variant-MIT-disclaimer.json\",\n      \"referenceNumber\": 331,\n      \"name\": \"HPND sell variant with MIT disclaimer\",\n      \"licenseId\": \"HPND-sell-variant-MIT-disclaimer\",\n      \"seeAlso\": [\n        \"https://github.com/sigmavirus24/x11-ssh-askpass/blob/master/README\"\n      ],\n      \"isOsiApproved\": false\n    },\n    {\n      \"reference\": \"https://spdx.org/licenses/HPND-sell-variant-MIT-disclaimer-rev.html\",\n      \"isDeprecatedLicenseId\": false,\n      \"detailsUrl\": \"https://spdx.org/licenses/HPND-sell-variant-MIT-disclaimer-rev.json\",\n      \"referenceNumber\": 1,\n      \"name\": \"HPND sell variant with MIT disclaimer - reverse\",\n      \"licenseId\": \"HPND-sell-variant-MIT-disclaimer-rev\",\n      \"seeAlso\": [\n        \"https://github.com/sigmavirus24/x11-ssh-askpass/blob/master/dynlist.c\"\n      ],\n      \"isOsiApproved\": false\n    },\n    {\n      \"reference\": \"https://spdx.org/licenses/HPND-UC.html\",\n      \"isDeprecatedLicenseId\": false,\n      \"detailsUrl\": \"https://spdx.org/licenses/HPND-UC.json\",\n      \"referenceNumber\": 280,\n      \"name\": \"Historical Permission Notice and Disclaimer - University of California variant\",\n      \"licenseId\": \"HPND-UC\",\n      \"seeAlso\": [\n        \"https://core.tcl-lang.org/tk/file?name\\u003dcompat/unistd.h\"\n      ],\n      \"isOsiApproved\": false\n    },\n    {\n      \"reference\": \"https://spdx.org/licenses/HPND-UC-export-US.html\",\n      \"isDeprecatedLicenseId\": false,\n      \"detailsUrl\": \"https://spdx.org/licenses/HPND-UC-export-US.json\",\n      \"referenceNumber\": 215,\n      \"name\": \"Historical Permission Notice and Disclaimer - University of California, US export warning\",\n      \"licenseId\": \"HPND-UC-export-US\",\n      \"seeAlso\": [\n        \"https://github.com/RTimothyEdwards/magic/blob/master/LICENSE\"\n      ],\n      \"isOsiApproved\": false\n    },\n    {\n      \"reference\": \"https://spdx.org/licenses/HTMLTIDY.html\",\n      \"isDeprecatedLicenseId\": false,\n      \"detailsUrl\": \"https://spdx.org/licenses/HTMLTIDY.json\",\n      \"referenceNumber\": 545,\n      \"name\": \"HTML Tidy License\",\n      \"licenseId\": \"HTMLTIDY\",\n      \"seeAlso\": [\n        \"https://github.com/htacg/tidy-html5/blob/next/README/LICENSE.md\"\n      ],\n      \"isOsiApproved\": false\n    },\n    {\n      \"reference\": \"https://spdx.org/licenses/IBM-pibs.html\",\n      \"isDeprecatedLicenseId\": false,\n      \"detailsUrl\": \"https://spdx.org/licenses/IBM-pibs.json\",\n      \"referenceNumber\": 156,\n      \"name\": \"IBM PowerPC Initialization and Boot Software\",\n      \"licenseId\": \"IBM-pibs\",\n      \"seeAlso\": [\n        \"http://git.denx.de/?p\\u003du-boot.git;a\\u003dblob;f\\u003darch/powerpc/cpu/ppc4xx/miiphy.c;h\\u003d297155fdafa064b955e53e9832de93bfb0cfb85b;hb\\u003d9fab4bf4cc077c21e43941866f3f2c196f28670d\"\n      ],\n      \"isOsiApproved\": false\n    },\n    {\n      \"reference\": \"https://spdx.org/licenses/ICU.html\",\n      \"isDeprecatedLicenseId\": false,\n      \"detailsUrl\": \"https://spdx.org/licenses/ICU.json\",\n      \"referenceNumber\": 78,\n      \"name\": \"ICU License\",\n      \"licenseId\": \"ICU\",\n      \"seeAlso\": [\n        \"http://source.icu-project.org/repos/icu/icu/trunk/license.html\"\n      ],\n      \"isOsiApproved\": true\n    },\n    {\n      \"reference\": \"https://spdx.org/licenses/IEC-Code-Components-EULA.html\",\n      \"isDeprecatedLicenseId\": false,\n      \"detailsUrl\": \"https://spdx.org/licenses/IEC-Code-Components-EULA.json\",\n      \"referenceNumber\": 180,\n      \"name\": \"IEC    Code Components End-user licence agreement\",\n      \"licenseId\": \"IEC-Code-Components-EULA\",\n      \"seeAlso\": [\n        \"https://www.iec.ch/webstore/custserv/pdf/CC-EULA.pdf\",\n        \"https://www.iec.ch/CCv1\",\n        \"https://www.iec.ch/copyright\"\n      ],\n      \"isOsiApproved\": false\n    },\n    {\n      \"reference\": \"https://spdx.org/licenses/IJG.html\",\n      \"isDeprecatedLicenseId\": false,\n      \"detailsUrl\": \"https://spdx.org/licenses/IJG.json\",\n      \"referenceNumber\": 375,\n      \"name\": \"Independent JPEG Group License\",\n      \"licenseId\": \"IJG\",\n      \"seeAlso\": [\n        \"http://dev.w3.org/cvsweb/Amaya/libjpeg/Attic/README?rev\\u003d1.2\"\n      ],\n      \"isOsiApproved\": false,\n      \"isFsfLibre\": true\n    },\n    {\n      \"reference\": \"https://spdx.org/licenses/IJG-short.html\",\n      \"isDeprecatedLicenseId\": false,\n      \"detailsUrl\": \"https://spdx.org/licenses/IJG-short.json\",\n      \"referenceNumber\": 200,\n      \"name\": \"Independent JPEG Group License - short\",\n      \"licenseId\": \"IJG-short\",\n      \"seeAlso\": [\n        \"https://sourceforge.net/p/xmedcon/code/ci/master/tree/libs/ljpg/\"\n      ],\n      \"isOsiApproved\": false\n    },\n    {\n      \"reference\": \"https://spdx.org/licenses/ImageMagick.html\",\n      \"isDeprecatedLicenseId\": false,\n      \"detailsUrl\": \"https://spdx.org/licenses/ImageMagick.json\",\n      \"referenceNumber\": 25,\n      \"name\": \"ImageMagick License\",\n      \"licenseId\": \"ImageMagick\",\n      \"seeAlso\": [\n        \"http://www.imagemagick.org/script/license.php\"\n      ],\n      \"isOsiApproved\": false\n    },\n    {\n      \"reference\": \"https://spdx.org/licenses/iMatix.html\",\n      \"isDeprecatedLicenseId\": false,\n      \"detailsUrl\": \"https://spdx.org/licenses/iMatix.json\",\n      \"referenceNumber\": 547,\n      \"name\": \"iMatix Standard Function Library Agreement\",\n      \"licenseId\": \"iMatix\",\n      \"seeAlso\": [\n        \"http://legacy.imatix.com/html/sfl/sfl4.htm#license\"\n      ],\n      \"isOsiApproved\": false,\n      \"isFsfLibre\": true\n    },\n    {\n      \"reference\": \"https://spdx.org/licenses/Imlib2.html\",\n      \"isDeprecatedLicenseId\": false,\n      \"detailsUrl\": \"https://spdx.org/licenses/Imlib2.json\",\n      \"referenceNumber\": 174,\n      \"name\": \"Imlib2 License\",\n      \"licenseId\": \"Imlib2\",\n      \"seeAlso\": [\n        \"http://trac.enlightenment.org/e/browser/trunk/imlib2/COPYING\",\n        \"https://git.enlightenment.org/legacy/imlib2.git/tree/COPYING\"\n      ],\n      \"isOsiApproved\": false,\n      \"isFsfLibre\": true\n    },\n    {\n      \"reference\": \"https://spdx.org/licenses/Info-ZIP.html\",\n      \"isDeprecatedLicenseId\": false,\n      \"detailsUrl\": \"https://spdx.org/licenses/Info-ZIP.json\",\n      \"referenceNumber\": 137,\n      \"name\": \"Info-ZIP License\",\n      \"licenseId\": \"Info-ZIP\",\n      \"seeAlso\": [\n        \"http://www.info-zip.org/license.html\"\n      ],\n      \"isOsiApproved\": false\n    },\n    {\n      \"reference\": \"https://spdx.org/licenses/Inner-Net-2.0.html\",\n      \"isDeprecatedLicenseId\": false,\n      \"detailsUrl\": \"https://spdx.org/licenses/Inner-Net-2.0.json\",\n      \"referenceNumber\": 564,\n      \"name\": \"Inner Net License v2.0\",\n      \"licenseId\": \"Inner-Net-2.0\",\n      \"seeAlso\": [\n        \"https://fedoraproject.org/wiki/Licensing/Inner_Net_License\",\n        \"https://sourceware.org/git/?p\\u003dglibc.git;a\\u003dblob;f\\u003dLICENSES;h\\u003d530893b1dc9ea00755603c68fb36bd4fc38a7be8;hb\\u003dHEAD#l207\"\n      ],\n      \"isOsiApproved\": false\n    },\n    {\n      \"reference\": \"https://spdx.org/licenses/Intel.html\",\n      \"isDeprecatedLicenseId\": false,\n      \"detailsUrl\": \"https://spdx.org/licenses/Intel.json\",\n      \"referenceNumber\": 80,\n      \"name\": \"Intel Open Source License\",\n      \"licenseId\": \"Intel\",\n      \"seeAlso\": [\n        \"https://opensource.org/licenses/Intel\"\n      ],\n      \"isOsiApproved\": true,\n      \"isFsfLibre\": true\n    },\n    {\n      \"reference\": \"https://spdx.org/licenses/Intel-ACPI.html\",\n      \"isDeprecatedLicenseId\": false,\n      \"detailsUrl\": \"https://spdx.org/licenses/Intel-ACPI.json\",\n      \"referenceNumber\": 87,\n      \"name\": \"Intel ACPI Software License Agreement\",\n      \"licenseId\": \"Intel-ACPI\",\n      \"seeAlso\": [\n        \"https://fedoraproject.org/wiki/Licensing/Intel_ACPI_Software_License_Agreement\"\n      ],\n      \"isOsiApproved\": false\n    },\n    {\n      \"reference\": \"https://spdx.org/licenses/Interbase-1.0.html\",\n      \"isDeprecatedLicenseId\": false,\n      \"detailsUrl\": \"https://spdx.org/licenses/Interbase-1.0.json\",\n      \"referenceNumber\": 518,\n      \"name\": \"Interbase Public License v1.0\",\n      \"licenseId\": \"Interbase-1.0\",\n      \"seeAlso\": [\n        \"https://web.archive.org/web/20060319014854/http://info.borland.com/devsupport/interbase/opensource/IPL.html\"\n      ],\n      \"isOsiApproved\": false\n    },\n    {\n      \"reference\": \"https://spdx.org/licenses/IPA.html\",\n      \"isDeprecatedLicenseId\": false,\n      \"detailsUrl\": \"https://spdx.org/licenses/IPA.json\",\n      \"referenceNumber\": 14,\n      \"name\": \"IPA Font License\",\n      \"licenseId\": \"IPA\",\n      \"seeAlso\": [\n        \"https://opensource.org/licenses/IPA\"\n      ],\n      \"isOsiApproved\": true,\n      \"isFsfLibre\": true\n    },\n    {\n      \"reference\": \"https://spdx.org/licenses/IPL-1.0.html\",\n      \"isDeprecatedLicenseId\": false,\n      \"detailsUrl\": \"https://spdx.org/licenses/IPL-1.0.json\",\n      \"referenceNumber\": 205,\n      \"name\": \"IBM Public License v1.0\",\n      \"licenseId\": \"IPL-1.0\",\n      \"seeAlso\": [\n        \"https://opensource.org/licenses/IPL-1.0\"\n      ],\n      \"isOsiApproved\": true,\n      \"isFsfLibre\": true\n    },\n    {\n      \"reference\": \"https://spdx.org/licenses/ISC.html\",\n      \"isDeprecatedLicenseId\": false,\n      \"detailsUrl\": \"https://spdx.org/licenses/ISC.json\",\n      \"referenceNumber\": 457,\n      \"name\": \"ISC License\",\n      \"licenseId\": \"ISC\",\n      \"seeAlso\": [\n        \"https://www.isc.org/licenses/\",\n        \"https://www.isc.org/downloads/software-support-policy/isc-license/\",\n        \"https://opensource.org/licenses/ISC\"\n      ],\n      \"isOsiApproved\": true,\n      \"isFsfLibre\": true\n    },\n    {\n      \"reference\": \"https://spdx.org/licenses/ISC-Veillard.html\",\n      \"isDeprecatedLicenseId\": false,\n      \"detailsUrl\": \"https://spdx.org/licenses/ISC-Veillard.json\",\n      \"referenceNumber\": 372,\n      \"name\": \"ISC Veillard variant\",\n      \"licenseId\": \"ISC-Veillard\",\n      \"seeAlso\": [\n        \"https://raw.githubusercontent.com/GNOME/libxml2/4c2e7c651f6c2f0d1a74f350cbda95f7df3e7017/hash.c\",\n        \"https://github.com/GNOME/libxml2/blob/master/dict.c\",\n        \"https://sourceforge.net/p/ctrio/git/ci/master/tree/README\"\n      ],\n      \"isOsiApproved\": false\n    },\n    {\n      \"reference\": \"https://spdx.org/licenses/Jam.html\",\n      \"isDeprecatedLicenseId\": false,\n      \"detailsUrl\": \"https://spdx.org/licenses/Jam.json\",\n      \"referenceNumber\": 194,\n      \"name\": \"Jam License\",\n      \"licenseId\": \"Jam\",\n      \"seeAlso\": [\n        \"https://www.boost.org/doc/libs/1_35_0/doc/html/jam.html\",\n        \"https://web.archive.org/web/20160330173339/https://swarm.workshop.perforce.com/files/guest/perforce_software/jam/src/README\"\n      ],\n      \"isOsiApproved\": true\n    },\n    {\n      \"reference\": \"https://spdx.org/licenses/JasPer-2.0.html\",\n      \"isDeprecatedLicenseId\": false,\n      \"detailsUrl\": \"https://spdx.org/licenses/JasPer-2.0.json\",\n      \"referenceNumber\": 462,\n      \"name\": \"JasPer License\",\n      \"licenseId\": \"JasPer-2.0\",\n      \"seeAlso\": [\n        \"http://www.ece.uvic.ca/~mdadams/jasper/LICENSE\"\n      ],\n      \"isOsiApproved\": false\n    },\n    {\n      \"reference\": \"https://spdx.org/licenses/JPL-image.html\",\n      \"isDeprecatedLicenseId\": false,\n      \"detailsUrl\": \"https://spdx.org/licenses/JPL-image.json\",\n      \"referenceNumber\": 23,\n      \"name\": \"JPL Image Use Policy\",\n      \"licenseId\": \"JPL-image\",\n      \"seeAlso\": [\n        \"https://www.jpl.nasa.gov/jpl-image-use-policy\"\n      ],\n      \"isOsiApproved\": false\n    },\n    {\n      \"reference\": \"https://spdx.org/licenses/JPNIC.html\",\n      \"isDeprecatedLicenseId\": false,\n      \"detailsUrl\": \"https://spdx.org/licenses/JPNIC.json\",\n      \"referenceNumber\": 99,\n      \"name\": \"Japan Network Information Center License\",\n      \"licenseId\": \"JPNIC\",\n      \"seeAlso\": [\n        \"https://gitlab.isc.org/isc-projects/bind9/blob/master/COPYRIGHT#L366\"\n      ],\n      \"isOsiApproved\": false\n    },\n    {\n      \"reference\": \"https://spdx.org/licenses/JSON.html\",\n      \"isDeprecatedLicenseId\": false,\n      \"detailsUrl\": \"https://spdx.org/licenses/JSON.json\",\n      \"referenceNumber\": 323,\n      \"name\": \"JSON License\",\n      \"licenseId\": \"JSON\",\n      \"seeAlso\": [\n        \"http://www.json.org/license.html\"\n      ],\n      \"isOsiApproved\": false,\n      \"isFsfLibre\": false\n    },\n    {\n      \"reference\": \"https://spdx.org/licenses/Kastrup.html\",\n      \"isDeprecatedLicenseId\": false,\n      \"detailsUrl\": \"https://spdx.org/licenses/Kastrup.json\",\n      \"referenceNumber\": 600,\n      \"name\": \"Kastrup License\",\n      \"licenseId\": \"Kastrup\",\n      \"seeAlso\": [\n        \"https://ctan.math.utah.edu/ctan/tex-archive/macros/generic/kastrup/binhex.dtx\"\n      ],\n      \"isOsiApproved\": false\n    },\n    {\n      \"reference\": \"https://spdx.org/licenses/Kazlib.html\",\n      \"isDeprecatedLicenseId\": false,\n      \"detailsUrl\": \"https://spdx.org/licenses/Kazlib.json\",\n      \"referenceNumber\": 217,\n      \"name\": \"Kazlib License\",\n      \"licenseId\": \"Kazlib\",\n      \"seeAlso\": [\n        \"http://git.savannah.gnu.org/cgit/kazlib.git/tree/except.c?id\\u003d0062df360c2d17d57f6af19b0e444c51feb99036\"\n      ],\n      \"isOsiApproved\": false\n    },\n    {\n      \"reference\": \"https://spdx.org/licenses/Knuth-CTAN.html\",\n      \"isDeprecatedLicenseId\": false,\n      \"detailsUrl\": \"https://spdx.org/licenses/Knuth-CTAN.json\",\n      \"referenceNumber\": 347,\n      \"name\": \"Knuth CTAN License\",\n      \"licenseId\": \"Knuth-CTAN\",\n      \"seeAlso\": [\n        \"https://ctan.org/license/knuth\"\n      ],\n      \"isOsiApproved\": false\n    },\n    {\n      \"reference\": \"https://spdx.org/licenses/LAL-1.2.html\",\n      \"isDeprecatedLicenseId\": false,\n      \"detailsUrl\": \"https://spdx.org/licenses/LAL-1.2.json\",\n      \"referenceNumber\": 132,\n      \"name\": \"Licence Art Libre 1.2\",\n      \"licenseId\": \"LAL-1.2\",\n      \"seeAlso\": [\n        \"http://artlibre.org/licence/lal/licence-art-libre-12/\"\n      ],\n      \"isOsiApproved\": false\n    },\n    {\n      \"reference\": \"https://spdx.org/licenses/LAL-1.3.html\",\n      \"isDeprecatedLicenseId\": false,\n      \"detailsUrl\": \"https://spdx.org/licenses/LAL-1.3.json\",\n      \"referenceNumber\": 532,\n      \"name\": \"Licence Art Libre 1.3\",\n      \"licenseId\": \"LAL-1.3\",\n      \"seeAlso\": [\n        \"https://artlibre.org/\"\n      ],\n      \"isOsiApproved\": false\n    },\n    {\n      \"reference\": \"https://spdx.org/licenses/Latex2e.html\",\n      \"isDeprecatedLicenseId\": false,\n      \"detailsUrl\": \"https://spdx.org/licenses/Latex2e.json\",\n      \"referenceNumber\": 92,\n      \"name\": \"Latex2e License\",\n      \"licenseId\": \"Latex2e\",\n      \"seeAlso\": [\n        \"https://fedoraproject.org/wiki/Licensing/Latex2e\"\n      ],\n      \"isOsiApproved\": false\n    },\n    {\n      \"reference\": \"https://spdx.org/licenses/Latex2e-translated-notice.html\",\n      \"isDeprecatedLicenseId\": false,\n      \"detailsUrl\": \"https://spdx.org/licenses/Latex2e-translated-notice.json\",\n      \"referenceNumber\": 62,\n      \"name\": \"Latex2e with translated notice permission\",\n      \"licenseId\": \"Latex2e-translated-notice\",\n      \"seeAlso\": [\n        \"https://git.savannah.gnu.org/cgit/indent.git/tree/doc/indent.texi?id\\u003da74c6b4ee49397cf330b333da1042bffa60ed14f#n74\"\n      ],\n      \"isOsiApproved\": false\n    },\n    {\n      \"reference\": \"https://spdx.org/licenses/Leptonica.html\",\n      \"isDeprecatedLicenseId\": false,\n      \"detailsUrl\": \"https://spdx.org/licenses/Leptonica.json\",\n      \"referenceNumber\": 149,\n      \"name\": \"Leptonica License\",\n      \"licenseId\": \"Leptonica\",\n      \"seeAlso\": [\n        \"https://fedoraproject.org/wiki/Licensing/Leptonica\"\n      ],\n      \"isOsiApproved\": false\n    },\n    {\n      \"reference\": \"https://spdx.org/licenses/LGPL-2.0.html\",\n      \"isDeprecatedLicenseId\": true,\n      \"detailsUrl\": \"https://spdx.org/licenses/LGPL-2.0.json\",\n      \"referenceNumber\": 651,\n      \"name\": \"GNU Library General Public License v2 only\",\n      \"licenseId\": \"LGPL-2.0\",\n      \"seeAlso\": [\n        \"https://www.gnu.org/licenses/old-licenses/lgpl-2.0-standalone.html\"\n      ],\n      \"isOsiApproved\": true\n    },\n    {\n      \"reference\": \"https://spdx.org/licenses/LGPL-2.0+.html\",\n      \"isDeprecatedLicenseId\": true,\n      \"detailsUrl\": \"https://spdx.org/licenses/LGPL-2.0+.json\",\n      \"referenceNumber\": 84,\n      \"name\": \"GNU Library General Public License v2 or later\",\n      \"licenseId\": \"LGPL-2.0+\",\n      \"seeAlso\": [\n        \"https://www.gnu.org/licenses/old-licenses/lgpl-2.0-standalone.html\"\n      ],\n      \"isOsiApproved\": true\n    },\n    {\n      \"reference\": \"https://spdx.org/licenses/LGPL-2.0-only.html\",\n      \"isDeprecatedLicenseId\": false,\n      \"detailsUrl\": \"https://spdx.org/licenses/LGPL-2.0-only.json\",\n      \"referenceNumber\": 585,\n      \"name\": \"GNU Library General Public License v2 only\",\n      \"licenseId\": \"LGPL-2.0-only\",\n      \"seeAlso\": [\n        \"https://www.gnu.org/licenses/old-licenses/lgpl-2.0-standalone.html\"\n      ],\n      \"isOsiApproved\": true\n    },\n    {\n      \"reference\": \"https://spdx.org/licenses/LGPL-2.0-or-later.html\",\n      \"isDeprecatedLicenseId\": false,\n      \"detailsUrl\": \"https://spdx.org/licenses/LGPL-2.0-or-later.json\",\n      \"referenceNumber\": 345,\n      \"name\": \"GNU Library General Public License v2 or later\",\n      \"licenseId\": \"LGPL-2.0-or-later\",\n      \"seeAlso\": [\n        \"https://www.gnu.org/licenses/old-licenses/lgpl-2.0-standalone.html\"\n      ],\n      \"isOsiApproved\": true\n    },\n    {\n      \"reference\": \"https://spdx.org/licenses/LGPL-2.1.html\",\n      \"isDeprecatedLicenseId\": true,\n      \"detailsUrl\": \"https://spdx.org/licenses/LGPL-2.1.json\",\n      \"referenceNumber\": 653,\n      \"name\": \"GNU Lesser General Public License v2.1 only\",\n      \"licenseId\": \"LGPL-2.1\",\n      \"seeAlso\": [\n        \"https://www.gnu.org/licenses/old-licenses/lgpl-2.1-standalone.html\",\n        \"https://opensource.org/licenses/LGPL-2.1\"\n      ],\n      \"isOsiApproved\": true,\n      \"isFsfLibre\": true\n    },\n    {\n      \"reference\": \"https://spdx.org/licenses/LGPL-2.1+.html\",\n      \"isDeprecatedLicenseId\": true,\n      \"detailsUrl\": \"https://spdx.org/licenses/LGPL-2.1+.json\",\n      \"referenceNumber\": 428,\n      \"name\": \"GNU Lesser General Public License v2.1 or later\",\n      \"licenseId\": \"LGPL-2.1+\",\n      \"seeAlso\": [\n        \"https://www.gnu.org/licenses/old-licenses/lgpl-2.1-standalone.html\",\n        \"https://opensource.org/licenses/LGPL-2.1\"\n      ],\n      \"isOsiApproved\": true,\n      \"isFsfLibre\": true\n    },\n    {\n      \"reference\": \"https://spdx.org/licenses/LGPL-2.1-only.html\",\n      \"isDeprecatedLicenseId\": false,\n      \"detailsUrl\": \"https://spdx.org/licenses/LGPL-2.1-only.json\",\n      \"referenceNumber\": 429,\n      \"name\": \"GNU Lesser General Public License v2.1 only\",\n      \"licenseId\": \"LGPL-2.1-only\",\n      \"seeAlso\": [\n        \"https://www.gnu.org/licenses/old-licenses/lgpl-2.1-standalone.html\",\n        \"https://opensource.org/licenses/LGPL-2.1\"\n      ],\n      \"isOsiApproved\": true,\n      \"isFsfLibre\": true\n    },\n    {\n      \"reference\": \"https://spdx.org/licenses/LGPL-2.1-or-later.html\",\n      \"isDeprecatedLicenseId\": false,\n      \"detailsUrl\": \"https://spdx.org/licenses/LGPL-2.1-or-later.json\",\n      \"referenceNumber\": 160,\n      \"name\": \"GNU Lesser General Public License v2.1 or later\",\n      \"licenseId\": \"LGPL-2.1-or-later\",\n      \"seeAlso\": [\n        \"https://www.gnu.org/licenses/old-licenses/lgpl-2.1-standalone.html\",\n        \"https://opensource.org/licenses/LGPL-2.1\"\n      ],\n      \"isOsiApproved\": true,\n      \"isFsfLibre\": true\n    },\n    {\n      \"reference\": \"https://spdx.org/licenses/LGPL-3.0.html\",\n      \"isDeprecatedLicenseId\": true,\n      \"detailsUrl\": \"https://spdx.org/licenses/LGPL-3.0.json\",\n      \"referenceNumber\": 340,\n      \"name\": \"GNU Lesser General Public License v3.0 only\",\n      \"licenseId\": \"LGPL-3.0\",\n      \"seeAlso\": [\n        \"https://www.gnu.org/licenses/lgpl-3.0-standalone.html\",\n        \"https://www.gnu.org/licenses/lgpl+gpl-3.0.txt\",\n        \"https://opensource.org/licenses/LGPL-3.0\"\n      ],\n      \"isOsiApproved\": true,\n      \"isFsfLibre\": true\n    },\n    {\n      \"reference\": \"https://spdx.org/licenses/LGPL-3.0+.html\",\n      \"isDeprecatedLicenseId\": true,\n      \"detailsUrl\": \"https://spdx.org/licenses/LGPL-3.0+.json\",\n      \"referenceNumber\": 103,\n      \"name\": \"GNU Lesser General Public License v3.0 or later\",\n      \"licenseId\": \"LGPL-3.0+\",\n      \"seeAlso\": [\n        \"https://www.gnu.org/licenses/lgpl-3.0-standalone.html\",\n        \"https://www.gnu.org/licenses/lgpl+gpl-3.0.txt\",\n        \"https://opensource.org/licenses/LGPL-3.0\"\n      ],\n      \"isOsiApproved\": true,\n      \"isFsfLibre\": true\n    },\n    {\n      \"reference\": \"https://spdx.org/licenses/LGPL-3.0-only.html\",\n      \"isDeprecatedLicenseId\": false,\n      \"detailsUrl\": \"https://spdx.org/licenses/LGPL-3.0-only.json\",\n      \"referenceNumber\": 593,\n      \"name\": \"GNU Lesser General Public License v3.0 only\",\n      \"licenseId\": \"LGPL-3.0-only\",\n      \"seeAlso\": [\n        \"https://www.gnu.org/licenses/lgpl-3.0-standalone.html\",\n        \"https://www.gnu.org/licenses/lgpl+gpl-3.0.txt\",\n        \"https://opensource.org/licenses/LGPL-3.0\"\n      ],\n      \"isOsiApproved\": true,\n      \"isFsfLibre\": true\n    },\n    {\n      \"reference\": \"https://spdx.org/licenses/LGPL-3.0-or-later.html\",\n      \"isDeprecatedLicenseId\": false,\n      \"detailsUrl\": \"https://spdx.org/licenses/LGPL-3.0-or-later.json\",\n      \"referenceNumber\": 647,\n      \"name\": \"GNU Lesser General Public License v3.0 or later\",\n      \"licenseId\": \"LGPL-3.0-or-later\",\n      \"seeAlso\": [\n        \"https://www.gnu.org/licenses/lgpl-3.0-standalone.html\",\n        \"https://www.gnu.org/licenses/lgpl+gpl-3.0.txt\",\n        \"https://opensource.org/licenses/LGPL-3.0\"\n      ],\n      \"isOsiApproved\": true,\n      \"isFsfLibre\": true\n    },\n    {\n      \"reference\": \"https://spdx.org/licenses/LGPLLR.html\",\n      \"isDeprecatedLicenseId\": false,\n      \"detailsUrl\": \"https://spdx.org/licenses/LGPLLR.json\",\n      \"referenceNumber\": 476,\n      \"name\": \"Lesser General Public License For Linguistic Resources\",\n      \"licenseId\": \"LGPLLR\",\n      \"seeAlso\": [\n        \"http://www-igm.univ-mlv.fr/~unitex/lgpllr.html\"\n      ],\n      \"isOsiApproved\": false\n    },\n    {\n      \"reference\": \"https://spdx.org/licenses/Libpng.html\",\n      \"isDeprecatedLicenseId\": false,\n      \"detailsUrl\": \"https://spdx.org/licenses/Libpng.json\",\n      \"referenceNumber\": 128,\n      \"name\": \"libpng License\",\n      \"licenseId\": \"Libpng\",\n      \"seeAlso\": [\n        \"http://www.libpng.org/pub/png/src/libpng-LICENSE.txt\"\n      ],\n      \"isOsiApproved\": false\n    },\n    {\n      \"reference\": \"https://spdx.org/licenses/libpng-2.0.html\",\n      \"isDeprecatedLicenseId\": false,\n      \"detailsUrl\": \"https://spdx.org/licenses/libpng-2.0.json\",\n      \"referenceNumber\": 249,\n      \"name\": \"PNG Reference Library version 2\",\n      \"licenseId\": \"libpng-2.0\",\n      \"seeAlso\": [\n        \"http://www.libpng.org/pub/png/src/libpng-LICENSE.txt\"\n      ],\n      \"isOsiApproved\": false\n    },\n    {\n      \"reference\": \"https://spdx.org/licenses/libselinux-1.0.html\",\n      \"isDeprecatedLicenseId\": false,\n      \"detailsUrl\": \"https://spdx.org/licenses/libselinux-1.0.json\",\n      \"referenceNumber\": 63,\n      \"name\": \"libselinux public domain notice\",\n      \"licenseId\": \"libselinux-1.0\",\n      \"seeAlso\": [\n        \"https://github.com/SELinuxProject/selinux/blob/master/libselinux/LICENSE\"\n      ],\n      \"isOsiApproved\": false\n    },\n    {\n      \"reference\": \"https://spdx.org/licenses/libtiff.html\",\n      \"isDeprecatedLicenseId\": false,\n      \"detailsUrl\": \"https://spdx.org/licenses/libtiff.json\",\n      \"referenceNumber\": 437,\n      \"name\": \"libtiff License\",\n      \"licenseId\": \"libtiff\",\n      \"seeAlso\": [\n        \"https://fedoraproject.org/wiki/Licensing/libtiff\"\n      ],\n      \"isOsiApproved\": false\n    },\n    {\n      \"reference\": \"https://spdx.org/licenses/libutil-David-Nugent.html\",\n      \"isDeprecatedLicenseId\": false,\n      \"detailsUrl\": \"https://spdx.org/licenses/libutil-David-Nugent.json\",\n      \"referenceNumber\": 337,\n      \"name\": \"libutil David Nugent License\",\n      \"licenseId\": \"libutil-David-Nugent\",\n      \"seeAlso\": [\n        \"http://web.mit.edu/freebsd/head/lib/libutil/login_ok.3\",\n        \"https://cgit.freedesktop.org/libbsd/tree/man/setproctitle.3bsd\"\n      ],\n      \"isOsiApproved\": false\n    },\n    {\n      \"reference\": \"https://spdx.org/licenses/LiLiQ-P-1.1.html\",\n      \"isDeprecatedLicenseId\": false,\n      \"detailsUrl\": \"https://spdx.org/licenses/LiLiQ-P-1.1.json\",\n      \"referenceNumber\": 335,\n      \"name\": \"Licence Libre du Québec – Permissive version 1.1\",\n      \"licenseId\": \"LiLiQ-P-1.1\",\n      \"seeAlso\": [\n        \"https://forge.gouv.qc.ca/licence/fr/liliq-v1-1/\",\n        \"http://opensource.org/licenses/LiLiQ-P-1.1\"\n      ],\n      \"isOsiApproved\": true\n    },\n    {\n      \"reference\": \"https://spdx.org/licenses/LiLiQ-R-1.1.html\",\n      \"isDeprecatedLicenseId\": false,\n      \"detailsUrl\": \"https://spdx.org/licenses/LiLiQ-R-1.1.json\",\n      \"referenceNumber\": 282,\n      \"name\": \"Licence Libre du Québec – Réciprocité version 1.1\",\n      \"licenseId\": \"LiLiQ-R-1.1\",\n      \"seeAlso\": [\n        \"https://www.forge.gouv.qc.ca/participez/licence-logicielle/licence-libre-du-quebec-liliq-en-francais/licence-libre-du-quebec-reciprocite-liliq-r-v1-1/\",\n        \"http://opensource.org/licenses/LiLiQ-R-1.1\"\n      ],\n      \"isOsiApproved\": true\n    },\n    {\n      \"reference\": \"https://spdx.org/licenses/LiLiQ-Rplus-1.1.html\",\n      \"isDeprecatedLicenseId\": false,\n      \"detailsUrl\": \"https://spdx.org/licenses/LiLiQ-Rplus-1.1.json\",\n      \"referenceNumber\": 578,\n      \"name\": \"Licence Libre du Québec – Réciprocité forte version 1.1\",\n      \"licenseId\": \"LiLiQ-Rplus-1.1\",\n      \"seeAlso\": [\n        \"https://www.forge.gouv.qc.ca/participez/licence-logicielle/licence-libre-du-quebec-liliq-en-francais/licence-libre-du-quebec-reciprocite-forte-liliq-r-v1-1/\",\n        \"http://opensource.org/licenses/LiLiQ-Rplus-1.1\"\n      ],\n      \"isOsiApproved\": true\n    },\n    {\n      \"reference\": \"https://spdx.org/licenses/Linux-man-pages-1-para.html\",\n      \"isDeprecatedLicenseId\": false,\n      \"detailsUrl\": \"https://spdx.org/licenses/Linux-man-pages-1-para.json\",\n      \"referenceNumber\": 350,\n      \"name\": \"Linux man-pages - 1 paragraph\",\n      \"licenseId\": \"Linux-man-pages-1-para\",\n      \"seeAlso\": [\n        \"https://git.kernel.org/pub/scm/docs/man-pages/man-pages.git/tree/man2/getcpu.2#n4\"\n      ],\n      \"isOsiApproved\": false\n    },\n    {\n      \"reference\": \"https://spdx.org/licenses/Linux-man-pages-copyleft.html\",\n      \"isDeprecatedLicenseId\": false,\n      \"detailsUrl\": \"https://spdx.org/licenses/Linux-man-pages-copyleft.json\",\n      \"referenceNumber\": 467,\n      \"name\": \"Linux man-pages Copyleft\",\n      \"licenseId\": \"Linux-man-pages-copyleft\",\n      \"seeAlso\": [\n        \"https://www.kernel.org/doc/man-pages/licenses.html\"\n      ],\n      \"isOsiApproved\": false\n    },\n    {\n      \"reference\": \"https://spdx.org/licenses/Linux-man-pages-copyleft-2-para.html\",\n      \"isDeprecatedLicenseId\": false,\n      \"detailsUrl\": \"https://spdx.org/licenses/Linux-man-pages-copyleft-2-para.json\",\n      \"referenceNumber\": 618,\n      \"name\": \"Linux man-pages Copyleft - 2 paragraphs\",\n      \"licenseId\": \"Linux-man-pages-copyleft-2-para\",\n      \"seeAlso\": [\n        \"https://git.kernel.org/pub/scm/docs/man-pages/man-pages.git/tree/man2/move_pages.2#n5\",\n        \"https://git.kernel.org/pub/scm/docs/man-pages/man-pages.git/tree/man2/migrate_pages.2#n8\"\n      ],\n      \"isOsiApproved\": false\n    },\n    {\n      \"reference\": \"https://spdx.org/licenses/Linux-man-pages-copyleft-var.html\",\n      \"isDeprecatedLicenseId\": false,\n      \"detailsUrl\": \"https://spdx.org/licenses/Linux-man-pages-copyleft-var.json\",\n      \"referenceNumber\": 244,\n      \"name\": \"Linux man-pages Copyleft Variant\",\n      \"licenseId\": \"Linux-man-pages-copyleft-var\",\n      \"seeAlso\": [\n        \"https://git.kernel.org/pub/scm/docs/man-pages/man-pages.git/tree/man2/set_mempolicy.2#n5\"\n      ],\n      \"isOsiApproved\": false\n    },\n    {\n      \"reference\": \"https://spdx.org/licenses/Linux-OpenIB.html\",\n      \"isDeprecatedLicenseId\": false,\n      \"detailsUrl\": \"https://spdx.org/licenses/Linux-OpenIB.json\",\n      \"referenceNumber\": 301,\n      \"name\": \"Linux Kernel Variant of OpenIB.org license\",\n      \"licenseId\": \"Linux-OpenIB\",\n      \"seeAlso\": [\n        \"https://git.kernel.org/pub/scm/linux/kernel/git/torvalds/linux.git/tree/drivers/infiniband/core/sa.h\"\n      ],\n      \"isOsiApproved\": false\n    },\n    {\n      \"reference\": \"https://spdx.org/licenses/LOOP.html\",\n      \"isDeprecatedLicenseId\": false,\n      \"detailsUrl\": \"https://spdx.org/licenses/LOOP.json\",\n      \"referenceNumber\": 320,\n      \"name\": \"Common Lisp LOOP License\",\n      \"licenseId\": \"LOOP\",\n      \"seeAlso\": [\n        \"https://gitlab.com/embeddable-common-lisp/ecl/-/blob/develop/src/lsp/loop.lsp\",\n        \"http://git.savannah.gnu.org/cgit/gcl.git/tree/gcl/lsp/gcl_loop.lsp?h\\u003dVersion_2_6_13pre\",\n        \"https://sourceforge.net/p/sbcl/sbcl/ci/master/tree/src/code/loop.lisp\",\n        \"https://github.com/cl-adams/adams/blob/master/LICENSE.md\",\n        \"https://github.com/blakemcbride/eclipse-lisp/blob/master/lisp/loop.lisp\",\n        \"https://gitlab.common-lisp.net/cmucl/cmucl/-/blob/master/src/code/loop.lisp\"\n      ],\n      \"isOsiApproved\": false\n    },\n    {\n      \"reference\": \"https://spdx.org/licenses/LPD-document.html\",\n      \"isDeprecatedLicenseId\": false,\n      \"detailsUrl\": \"https://spdx.org/licenses/LPD-document.json\",\n      \"referenceNumber\": 627,\n      \"name\": \"LPD Documentation License\",\n      \"licenseId\": \"LPD-document\",\n      \"seeAlso\": [\n        \"https://github.com/Cyan4973/xxHash/blob/dev/doc/xxhash_spec.md\",\n        \"https://www.ietf.org/rfc/rfc1952.txt\"\n      ],\n      \"isOsiApproved\": false\n    },\n    {\n      \"reference\": \"https://spdx.org/licenses/LPL-1.0.html\",\n      \"isDeprecatedLicenseId\": false,\n      \"detailsUrl\": \"https://spdx.org/licenses/LPL-1.0.json\",\n      \"referenceNumber\": 30,\n      \"name\": \"Lucent Public License Version 1.0\",\n      \"licenseId\": \"LPL-1.0\",\n      \"seeAlso\": [\n        \"https://opensource.org/licenses/LPL-1.0\"\n      ],\n      \"isOsiApproved\": true\n    },\n    {\n      \"reference\": \"https://spdx.org/licenses/LPL-1.02.html\",\n      \"isDeprecatedLicenseId\": false,\n      \"detailsUrl\": \"https://spdx.org/licenses/LPL-1.02.json\",\n      \"referenceNumber\": 53,\n      \"name\": \"Lucent Public License v1.02\",\n      \"licenseId\": \"LPL-1.02\",\n      \"seeAlso\": [\n        \"http://plan9.bell-labs.com/plan9/license.html\",\n        \"https://opensource.org/licenses/LPL-1.02\"\n      ],\n      \"isOsiApproved\": true,\n      \"isFsfLibre\": true\n    },\n    {\n      \"reference\": \"https://spdx.org/licenses/LPPL-1.0.html\",\n      \"isDeprecatedLicenseId\": false,\n      \"detailsUrl\": \"https://spdx.org/licenses/LPPL-1.0.json\",\n      \"referenceNumber\": 104,\n      \"name\": \"LaTeX Project Public License v1.0\",\n      \"licenseId\": \"LPPL-1.0\",\n      \"seeAlso\": [\n        \"http://www.latex-project.org/lppl/lppl-1-0.txt\"\n      ],\n      \"isOsiApproved\": false\n    },\n    {\n      \"reference\": \"https://spdx.org/licenses/LPPL-1.1.html\",\n      \"isDeprecatedLicenseId\": false,\n      \"detailsUrl\": \"https://spdx.org/licenses/LPPL-1.1.json\",\n      \"referenceNumber\": 419,\n      \"name\": \"LaTeX Project Public License v1.1\",\n      \"licenseId\": \"LPPL-1.1\",\n      \"seeAlso\": [\n        \"http://www.latex-project.org/lppl/lppl-1-1.txt\"\n      ],\n      \"isOsiApproved\": false\n    },\n    {\n      \"reference\": \"https://spdx.org/licenses/LPPL-1.2.html\",\n      \"isDeprecatedLicenseId\": false,\n      \"detailsUrl\": \"https://spdx.org/licenses/LPPL-1.2.json\",\n      \"referenceNumber\": 285,\n      \"name\": \"LaTeX Project Public License v1.2\",\n      \"licenseId\": \"LPPL-1.2\",\n      \"seeAlso\": [\n        \"http://www.latex-project.org/lppl/lppl-1-2.txt\"\n      ],\n      \"isOsiApproved\": false,\n      \"isFsfLibre\": true\n    },\n    {\n      \"reference\": \"https://spdx.org/licenses/LPPL-1.3a.html\",\n      \"isDeprecatedLicenseId\": false,\n      \"detailsUrl\": \"https://spdx.org/licenses/LPPL-1.3a.json\",\n      \"referenceNumber\": 534,\n      \"name\": \"LaTeX Project Public License v1.3a\",\n      \"licenseId\": \"LPPL-1.3a\",\n      \"seeAlso\": [\n        \"http://www.latex-project.org/lppl/lppl-1-3a.txt\"\n      ],\n      \"isOsiApproved\": false,\n      \"isFsfLibre\": true\n    },\n    {\n      \"reference\": \"https://spdx.org/licenses/LPPL-1.3c.html\",\n      \"isDeprecatedLicenseId\": false,\n      \"detailsUrl\": \"https://spdx.org/licenses/LPPL-1.3c.json\",\n      \"referenceNumber\": 91,\n      \"name\": \"LaTeX Project Public License v1.3c\",\n      \"licenseId\": \"LPPL-1.3c\",\n      \"seeAlso\": [\n        \"http://www.latex-project.org/lppl/lppl-1-3c.txt\",\n        \"https://opensource.org/licenses/LPPL-1.3c\"\n      ],\n      \"isOsiApproved\": true\n    },\n    {\n      \"reference\": \"https://spdx.org/licenses/lsof.html\",\n      \"isDeprecatedLicenseId\": false,\n      \"detailsUrl\": \"https://spdx.org/licenses/lsof.json\",\n      \"referenceNumber\": 250,\n      \"name\": \"lsof License\",\n      \"licenseId\": \"lsof\",\n      \"seeAlso\": [\n        \"https://github.com/lsof-org/lsof/blob/master/COPYING\"\n      ],\n      \"isOsiApproved\": false\n    },\n    {\n      \"reference\": \"https://spdx.org/licenses/Lucida-Bitmap-Fonts.html\",\n      \"isDeprecatedLicenseId\": false,\n      \"detailsUrl\": \"https://spdx.org/licenses/Lucida-Bitmap-Fonts.json\",\n      \"referenceNumber\": 260,\n      \"name\": \"Lucida Bitmap Fonts License\",\n      \"licenseId\": \"Lucida-Bitmap-Fonts\",\n      \"seeAlso\": [\n        \"https://gitlab.freedesktop.org/xorg/font/bh-100dpi/-/blob/master/COPYING?ref_type\\u003dheads\"\n      ],\n      \"isOsiApproved\": false\n    },\n    {\n      \"reference\": \"https://spdx.org/licenses/LZMA-SDK-9.11-to-9.20.html\",\n      \"isDeprecatedLicenseId\": false,\n      \"detailsUrl\": \"https://spdx.org/licenses/LZMA-SDK-9.11-to-9.20.json\",\n      \"referenceNumber\": 395,\n      \"name\": \"LZMA SDK License (versions 9.11 to 9.20)\",\n      \"licenseId\": \"LZMA-SDK-9.11-to-9.20\",\n      \"seeAlso\": [\n        \"https://www.7-zip.org/sdk.html\",\n        \"https://sourceforge.net/projects/sevenzip/files/LZMA%20SDK/\"\n      ],\n      \"isOsiApproved\": false\n    },\n    {\n      \"reference\": \"https://spdx.org/licenses/LZMA-SDK-9.22.html\",\n      \"isDeprecatedLicenseId\": false,\n      \"detailsUrl\": \"https://spdx.org/licenses/LZMA-SDK-9.22.json\",\n      \"referenceNumber\": 59,\n      \"name\": \"LZMA SDK License (versions 9.22 and beyond)\",\n      \"licenseId\": \"LZMA-SDK-9.22\",\n      \"seeAlso\": [\n        \"https://www.7-zip.org/sdk.html\",\n        \"https://sourceforge.net/projects/sevenzip/files/LZMA%20SDK/\"\n      ],\n      \"isOsiApproved\": false\n    },\n    {\n      \"reference\": \"https://spdx.org/licenses/Mackerras-3-Clause.html\",\n      \"isDeprecatedLicenseId\": false,\n      \"detailsUrl\": \"https://spdx.org/licenses/Mackerras-3-Clause.json\",\n      \"referenceNumber\": 612,\n      \"name\": \"Mackerras 3-Clause License\",\n      \"licenseId\": \"Mackerras-3-Clause\",\n      \"seeAlso\": [\n        \"https://github.com/ppp-project/ppp/blob/master/pppd/chap_ms.c#L6-L28\"\n      ],\n      \"isOsiApproved\": false\n    },\n    {\n      \"reference\": \"https://spdx.org/licenses/Mackerras-3-Clause-acknowledgment.html\",\n      \"isDeprecatedLicenseId\": false,\n      \"detailsUrl\": \"https://spdx.org/licenses/Mackerras-3-Clause-acknowledgment.json\",\n      \"referenceNumber\": 304,\n      \"name\": \"Mackerras 3-Clause - acknowledgment variant\",\n      \"licenseId\": \"Mackerras-3-Clause-acknowledgment\",\n      \"seeAlso\": [\n        \"https://github.com/ppp-project/ppp/blob/master/pppd/auth.c#L6-L28\"\n      ],\n      \"isOsiApproved\": false\n    },\n    {\n      \"reference\": \"https://spdx.org/licenses/magaz.html\",\n      \"isDeprecatedLicenseId\": false,\n      \"detailsUrl\": \"https://spdx.org/licenses/magaz.json\",\n      \"referenceNumber\": 479,\n      \"name\": \"magaz License\",\n      \"licenseId\": \"magaz\",\n      \"seeAlso\": [\n        \"https://mirrors.nic.cz/tex-archive/macros/latex/contrib/magaz/magaz.tex\"\n      ],\n      \"isOsiApproved\": false\n    },\n    {\n      \"reference\": \"https://spdx.org/licenses/mailprio.html\",\n      \"isDeprecatedLicenseId\": false,\n      \"detailsUrl\": \"https://spdx.org/licenses/mailprio.json\",\n      \"referenceNumber\": 481,\n      \"name\": \"mailprio License\",\n      \"licenseId\": \"mailprio\",\n      \"seeAlso\": [\n        \"https://fossies.org/linux/sendmail/contrib/mailprio\"\n      ],\n      \"isOsiApproved\": false\n    },\n    {\n      \"reference\": \"https://spdx.org/licenses/MakeIndex.html\",\n      \"isDeprecatedLicenseId\": false,\n      \"detailsUrl\": \"https://spdx.org/licenses/MakeIndex.json\",\n      \"referenceNumber\": 73,\n      \"name\": \"MakeIndex License\",\n      \"licenseId\": \"MakeIndex\",\n      \"seeAlso\": [\n        \"https://fedoraproject.org/wiki/Licensing/MakeIndex\"\n      ],\n      \"isOsiApproved\": false\n    },\n    {\n      \"reference\": \"https://spdx.org/licenses/Martin-Birgmeier.html\",\n      \"isDeprecatedLicenseId\": false,\n      \"detailsUrl\": \"https://spdx.org/licenses/Martin-Birgmeier.json\",\n      \"referenceNumber\": 643,\n      \"name\": \"Martin Birgmeier License\",\n      \"licenseId\": \"Martin-Birgmeier\",\n      \"seeAlso\": [\n        \"https://github.com/Perl/perl5/blob/blead/util.c#L6136\"\n      ],\n      \"isOsiApproved\": false\n    },\n    {\n      \"reference\": \"https://spdx.org/licenses/McPhee-slideshow.html\",\n      \"isDeprecatedLicenseId\": false,\n      \"detailsUrl\": \"https://spdx.org/licenses/McPhee-slideshow.json\",\n      \"referenceNumber\": 105,\n      \"name\": \"McPhee Slideshow License\",\n      \"licenseId\": \"McPhee-slideshow\",\n      \"seeAlso\": [\n        \"https://mirror.las.iastate.edu/tex-archive/graphics/metapost/contrib/macros/slideshow/slideshow.mp\"\n      ],\n      \"isOsiApproved\": false\n    },\n    {\n      \"reference\": \"https://spdx.org/licenses/metamail.html\",\n      \"isDeprecatedLicenseId\": false,\n      \"detailsUrl\": \"https://spdx.org/licenses/metamail.json\",\n      \"referenceNumber\": 171,\n      \"name\": \"metamail License\",\n      \"licenseId\": \"metamail\",\n      \"seeAlso\": [\n        \"https://github.com/Dual-Life/mime-base64/blob/master/Base64.xs#L12\"\n      ],\n      \"isOsiApproved\": false\n    },\n    {\n      \"reference\": \"https://spdx.org/licenses/Minpack.html\",\n      \"isDeprecatedLicenseId\": false,\n      \"detailsUrl\": \"https://spdx.org/licenses/Minpack.json\",\n      \"referenceNumber\": 655,\n      \"name\": \"Minpack License\",\n      \"licenseId\": \"Minpack\",\n      \"seeAlso\": [\n        \"http://www.netlib.org/minpack/disclaimer\",\n        \"https://gitlab.com/libeigen/eigen/-/blob/master/COPYING.MINPACK\"\n      ],\n      \"isOsiApproved\": false\n    },\n    {\n      \"reference\": \"https://spdx.org/licenses/MirOS.html\",\n      \"isDeprecatedLicenseId\": false,\n      \"detailsUrl\": \"https://spdx.org/licenses/MirOS.json\",\n      \"referenceNumber\": 293,\n      \"name\": \"The MirOS Licence\",\n      \"licenseId\": \"MirOS\",\n      \"seeAlso\": [\n        \"https://opensource.org/licenses/MirOS\"\n      ],\n      \"isOsiApproved\": true\n    },\n    {\n      \"reference\": \"https://spdx.org/licenses/MIT.html\",\n      \"isDeprecatedLicenseId\": false,\n      \"detailsUrl\": \"https://spdx.org/licenses/MIT.json\",\n      \"referenceNumber\": 243,\n      \"name\": \"MIT License\",\n      \"licenseId\": \"MIT\",\n      \"seeAlso\": [\n        \"https://opensource.org/license/mit/\"\n      ],\n      \"isOsiApproved\": true,\n      \"isFsfLibre\": true\n    },\n    {\n      \"reference\": \"https://spdx.org/licenses/MIT-0.html\",\n      \"isDeprecatedLicenseId\": false,\n      \"detailsUrl\": \"https://spdx.org/licenses/MIT-0.json\",\n      \"referenceNumber\": 469,\n      \"name\": \"MIT No Attribution\",\n      \"licenseId\": \"MIT-0\",\n      \"seeAlso\": [\n        \"https://github.com/aws/mit-0\",\n        \"https://romanrm.net/mit-zero\",\n        \"https://github.com/awsdocs/aws-cloud9-user-guide/blob/master/LICENSE-SAMPLECODE\"\n      ],\n      \"isOsiApproved\": true\n    },\n    {\n      \"reference\": \"https://spdx.org/licenses/MIT-advertising.html\",\n      \"isDeprecatedLicenseId\": false,\n      \"detailsUrl\": \"https://spdx.org/licenses/MIT-advertising.json\",\n      \"referenceNumber\": 253,\n      \"name\": \"Enlightenment License (e16)\",\n      \"licenseId\": \"MIT-advertising\",\n      \"seeAlso\": [\n        \"https://fedoraproject.org/wiki/Licensing/MIT_With_Advertising\"\n      ],\n      \"isOsiApproved\": false\n    },\n    {\n      \"reference\": \"https://spdx.org/licenses/MIT-CMU.html\",\n      \"isDeprecatedLicenseId\": false,\n      \"detailsUrl\": \"https://spdx.org/licenses/MIT-CMU.json\",\n      \"referenceNumber\": 601,\n      \"name\": \"CMU License\",\n      \"licenseId\": \"MIT-CMU\",\n      \"seeAlso\": [\n        \"https://fedoraproject.org/wiki/Licensing:MIT?rd\\u003dLicensing/MIT#CMU_Style\",\n        \"https://github.com/python-pillow/Pillow/blob/fffb426092c8db24a5f4b6df243a8a3c01fb63cd/LICENSE\"\n      ],\n      \"isOsiApproved\": false\n    },\n    {\n      \"reference\": \"https://spdx.org/licenses/MIT-enna.html\",\n      \"isDeprecatedLicenseId\": false,\n      \"detailsUrl\": \"https://spdx.org/licenses/MIT-enna.json\",\n      \"referenceNumber\": 19,\n      \"name\": \"enna License\",\n      \"licenseId\": \"MIT-enna\",\n      \"seeAlso\": [\n        \"https://fedoraproject.org/wiki/Licensing/MIT#enna\"\n      ],\n      \"isOsiApproved\": false\n    },\n    {\n      \"reference\": \"https://spdx.org/licenses/MIT-feh.html\",\n      \"isDeprecatedLicenseId\": false,\n      \"detailsUrl\": \"https://spdx.org/licenses/MIT-feh.json\",\n      \"referenceNumber\": 516,\n      \"name\": \"feh License\",\n      \"licenseId\": \"MIT-feh\",\n      \"seeAlso\": [\n        \"https://fedoraproject.org/wiki/Licensing/MIT#feh\"\n      ],\n      \"isOsiApproved\": false\n    },\n    {\n      \"reference\": \"https://spdx.org/licenses/MIT-Festival.html\",\n      \"isDeprecatedLicenseId\": false,\n      \"detailsUrl\": \"https://spdx.org/licenses/MIT-Festival.json\",\n      \"referenceNumber\": 140,\n      \"name\": \"MIT Festival Variant\",\n      \"licenseId\": \"MIT-Festival\",\n      \"seeAlso\": [\n        \"https://github.com/festvox/flite/blob/master/COPYING\",\n        \"https://github.com/festvox/speech_tools/blob/master/COPYING\"\n      ],\n      \"isOsiApproved\": false\n    },\n    {\n      \"reference\": \"https://spdx.org/licenses/MIT-Khronos-old.html\",\n      \"isDeprecatedLicenseId\": false,\n      \"detailsUrl\": \"https://spdx.org/licenses/MIT-Khronos-old.json\",\n      \"referenceNumber\": 294,\n      \"name\": \"MIT Khronos - old variant\",\n      \"licenseId\": \"MIT-Khronos-old\",\n      \"seeAlso\": [\n        \"https://github.com/KhronosGroup/SPIRV-Cross/blob/main/LICENSES/LicenseRef-KhronosFreeUse.txt\"\n      ],\n      \"isOsiApproved\": false\n    },\n    {\n      \"reference\": \"https://spdx.org/licenses/MIT-Modern-Variant.html\",\n      \"isDeprecatedLicenseId\": false,\n      \"detailsUrl\": \"https://spdx.org/licenses/MIT-Modern-Variant.json\",\n      \"referenceNumber\": 277,\n      \"name\": \"MIT License Modern Variant\",\n      \"licenseId\": \"MIT-Modern-Variant\",\n      \"seeAlso\": [\n        \"https://fedoraproject.org/wiki/Licensing:MIT#Modern_Variants\",\n        \"https://ptolemy.berkeley.edu/copyright.htm\",\n        \"https://pirlwww.lpl.arizona.edu/resources/guide/software/PerlTk/Tixlic.html\"\n      ],\n      \"isOsiApproved\": true\n    },\n    {\n      \"reference\": \"https://spdx.org/licenses/MIT-open-group.html\",\n      \"isDeprecatedLicenseId\": false,\n      \"detailsUrl\": \"https://spdx.org/licenses/MIT-open-group.json\",\n      \"referenceNumber\": 511,\n      \"name\": \"MIT Open Group variant\",\n      \"licenseId\": \"MIT-open-group\",\n      \"seeAlso\": [\n        \"https://gitlab.freedesktop.org/xorg/app/iceauth/-/blob/master/COPYING\",\n        \"https://gitlab.freedesktop.org/xorg/app/xvinfo/-/blob/master/COPYING\",\n        \"https://gitlab.freedesktop.org/xorg/app/xsetroot/-/blob/master/COPYING\",\n        \"https://gitlab.freedesktop.org/xorg/app/xauth/-/blob/master/COPYING\"\n      ],\n      \"isOsiApproved\": false\n    },\n    {\n      \"reference\": \"https://spdx.org/licenses/MIT-testregex.html\",\n      \"isDeprecatedLicenseId\": false,\n      \"detailsUrl\": \"https://spdx.org/licenses/MIT-testregex.json\",\n      \"referenceNumber\": 389,\n      \"name\": \"MIT testregex Variant\",\n      \"licenseId\": \"MIT-testregex\",\n      \"seeAlso\": [\n        \"https://github.com/dotnet/runtime/blob/55e1ac7c07df62c4108d4acedf78f77574470ce5/src/libraries/System.Text.RegularExpressions/tests/FunctionalTests/AttRegexTests.cs#L12-L28\"\n      ],\n      \"isOsiApproved\": false\n    },\n    {\n      \"reference\": \"https://spdx.org/licenses/MIT-Wu.html\",\n      \"isDeprecatedLicenseId\": false,\n      \"detailsUrl\": \"https://spdx.org/licenses/MIT-Wu.json\",\n      \"referenceNumber\": 486,\n      \"name\": \"MIT Tom Wu Variant\",\n      \"licenseId\": \"MIT-Wu\",\n      \"seeAlso\": [\n        \"https://github.com/chromium/octane/blob/master/crypto.js\"\n      ],\n      \"isOsiApproved\": false\n    },\n    {\n      \"reference\": \"https://spdx.org/licenses/MITNFA.html\",\n      \"isDeprecatedLicenseId\": false,\n      \"detailsUrl\": \"https://spdx.org/licenses/MITNFA.json\",\n      \"referenceNumber\": 571,\n      \"name\": \"MIT +no-false-attribs license\",\n      \"licenseId\": \"MITNFA\",\n      \"seeAlso\": [\n        \"https://fedoraproject.org/wiki/Licensing/MITNFA\"\n      ],\n      \"isOsiApproved\": false\n    },\n    {\n      \"reference\": \"https://spdx.org/licenses/MMIXware.html\",\n      \"isDeprecatedLicenseId\": false,\n      \"detailsUrl\": \"https://spdx.org/licenses/MMIXware.json\",\n      \"referenceNumber\": 199,\n      \"name\": \"MMIXware License\",\n      \"licenseId\": \"MMIXware\",\n      \"seeAlso\": [\n        \"https://gitlab.lrz.de/mmix/mmixware/-/blob/master/boilerplate.w\"\n      ],\n      \"isOsiApproved\": false\n    },\n    {\n      \"reference\": \"https://spdx.org/licenses/Motosoto.html\",\n      \"isDeprecatedLicenseId\": false,\n      \"detailsUrl\": \"https://spdx.org/licenses/Motosoto.json\",\n      \"referenceNumber\": 209,\n      \"name\": \"Motosoto License\",\n      \"licenseId\": \"Motosoto\",\n      \"seeAlso\": [\n        \"https://opensource.org/licenses/Motosoto\"\n      ],\n      \"isOsiApproved\": true\n    },\n    {\n      \"reference\": \"https://spdx.org/licenses/MPEG-SSG.html\",\n      \"isDeprecatedLicenseId\": false,\n      \"detailsUrl\": \"https://spdx.org/licenses/MPEG-SSG.json\",\n      \"referenceNumber\": 65,\n      \"name\": \"MPEG Software Simulation\",\n      \"licenseId\": \"MPEG-SSG\",\n      \"seeAlso\": [\n        \"https://sourceforge.net/p/netpbm/code/HEAD/tree/super_stable/converter/ppm/ppmtompeg/jrevdct.c#l1189\"\n      ],\n      \"isOsiApproved\": false\n    },\n    {\n      \"reference\": \"https://spdx.org/licenses/mpi-permissive.html\",\n      \"isDeprecatedLicenseId\": false,\n      \"detailsUrl\": \"https://spdx.org/licenses/mpi-permissive.json\",\n      \"referenceNumber\": 636,\n      \"name\": \"mpi Permissive License\",\n      \"licenseId\": \"mpi-permissive\",\n      \"seeAlso\": [\n        \"https://sources.debian.org/src/openmpi/4.1.0-10/ompi/debuggers/msgq_interface.h/?hl\\u003d19#L19\"\n      ],\n      \"isOsiApproved\": false\n    },\n    {\n      \"reference\": \"https://spdx.org/licenses/mpich2.html\",\n      \"isDeprecatedLicenseId\": false,\n      \"detailsUrl\": \"https://spdx.org/licenses/mpich2.json\",\n      \"referenceNumber\": 451,\n      \"name\": \"mpich2 License\",\n      \"licenseId\": \"mpich2\",\n      \"seeAlso\": [\n        \"https://fedoraproject.org/wiki/Licensing/MIT\"\n      ],\n      \"isOsiApproved\": false\n    },\n    {\n      \"reference\": \"https://spdx.org/licenses/MPL-1.0.html\",\n      \"isDeprecatedLicenseId\": false,\n      \"detailsUrl\": \"https://spdx.org/licenses/MPL-1.0.json\",\n      \"referenceNumber\": 382,\n      \"name\": \"Mozilla Public License 1.0\",\n      \"licenseId\": \"MPL-1.0\",\n      \"seeAlso\": [\n        \"http://www.mozilla.org/MPL/MPL-1.0.html\",\n        \"https://opensource.org/licenses/MPL-1.0\"\n      ],\n      \"isOsiApproved\": true\n    },\n    {\n      \"reference\": \"https://spdx.org/licenses/MPL-1.1.html\",\n      \"isDeprecatedLicenseId\": false,\n      \"detailsUrl\": \"https://spdx.org/licenses/MPL-1.1.json\",\n      \"referenceNumber\": 279,\n      \"name\": \"Mozilla Public License 1.1\",\n      \"licenseId\": \"MPL-1.1\",\n      \"seeAlso\": [\n        \"http://www.mozilla.org/MPL/MPL-1.1.html\",\n        \"https://opensource.org/licenses/MPL-1.1\"\n      ],\n      \"isOsiApproved\": true,\n      \"isFsfLibre\": true\n    },\n    {\n      \"reference\": \"https://spdx.org/licenses/MPL-2.0.html\",\n      \"isDeprecatedLicenseId\": false,\n      \"detailsUrl\": \"https://spdx.org/licenses/MPL-2.0.json\",\n      \"referenceNumber\": 298,\n      \"name\": \"Mozilla Public License 2.0\",\n      \"licenseId\": \"MPL-2.0\",\n      \"seeAlso\": [\n        \"https://www.mozilla.org/MPL/2.0/\",\n        \"https://opensource.org/licenses/MPL-2.0\"\n      ],\n      \"isOsiApproved\": true,\n      \"isFsfLibre\": true\n    },\n    {\n      \"reference\": \"https://spdx.org/licenses/MPL-2.0-no-copyleft-exception.html\",\n      \"isDeprecatedLicenseId\": false,\n      \"detailsUrl\": \"https://spdx.org/licenses/MPL-2.0-no-copyleft-exception.json\",\n      \"referenceNumber\": 288,\n      \"name\": \"Mozilla Public License 2.0 (no copyleft exception)\",\n      \"licenseId\": \"MPL-2.0-no-copyleft-exception\",\n      \"seeAlso\": [\n        \"https://www.mozilla.org/MPL/2.0/\",\n        \"https://opensource.org/licenses/MPL-2.0\"\n      ],\n      \"isOsiApproved\": true\n    },\n    {\n      \"reference\": \"https://spdx.org/licenses/mplus.html\",\n      \"isDeprecatedLicenseId\": false,\n      \"detailsUrl\": \"https://spdx.org/licenses/mplus.json\",\n      \"referenceNumber\": 342,\n      \"name\": \"mplus Font License\",\n      \"licenseId\": \"mplus\",\n      \"seeAlso\": [\n        \"https://fedoraproject.org/wiki/Licensing:Mplus?rd\\u003dLicensing/mplus\"\n      ],\n      \"isOsiApproved\": false\n    },\n    {\n      \"reference\": \"https://spdx.org/licenses/MS-LPL.html\",\n      \"isDeprecatedLicenseId\": false,\n      \"detailsUrl\": \"https://spdx.org/licenses/MS-LPL.json\",\n      \"referenceNumber\": 421,\n      \"name\": \"Microsoft Limited Public License\",\n      \"licenseId\": \"MS-LPL\",\n      \"seeAlso\": [\n        \"https://www.openhub.net/licenses/mslpl\",\n        \"https://github.com/gabegundy/atlserver/blob/master/License.txt\",\n        \"https://en.wikipedia.org/wiki/Shared_Source_Initiative#Microsoft_Limited_Public_License_(Ms-LPL)\"\n      ],\n      \"isOsiApproved\": false\n    },\n    {\n      \"reference\": \"https://spdx.org/licenses/MS-PL.html\",\n      \"isDeprecatedLicenseId\": false,\n      \"detailsUrl\": \"https://spdx.org/licenses/MS-PL.json\",\n      \"referenceNumber\": 613,\n      \"name\": \"Microsoft Public License\",\n      \"licenseId\": \"MS-PL\",\n      \"seeAlso\": [\n        \"http://www.microsoft.com/opensource/licenses.mspx\",\n        \"https://opensource.org/licenses/MS-PL\"\n      ],\n      \"isOsiApproved\": true,\n      \"isFsfLibre\": true\n    },\n    {\n      \"reference\": \"https://spdx.org/licenses/MS-RL.html\",\n      \"isDeprecatedLicenseId\": false,\n      \"detailsUrl\": \"https://spdx.org/licenses/MS-RL.json\",\n      \"referenceNumber\": 398,\n      \"name\": \"Microsoft Reciprocal License\",\n      \"licenseId\": \"MS-RL\",\n      \"seeAlso\": [\n        \"http://www.microsoft.com/opensource/licenses.mspx\",\n        \"https://opensource.org/licenses/MS-RL\"\n      ],\n      \"isOsiApproved\": true,\n      \"isFsfLibre\": true\n    },\n    {\n      \"reference\": \"https://spdx.org/licenses/MTLL.html\",\n      \"isDeprecatedLicenseId\": false,\n      \"detailsUrl\": \"https://spdx.org/licenses/MTLL.json\",\n      \"referenceNumber\": 594,\n      \"name\": \"Matrix Template Library License\",\n      \"licenseId\": \"MTLL\",\n      \"seeAlso\": [\n        \"https://fedoraproject.org/wiki/Licensing/Matrix_Template_Library_License\"\n      ],\n      \"isOsiApproved\": false\n    },\n    {\n      \"reference\": \"https://spdx.org/licenses/MulanPSL-1.0.html\",\n      \"isDeprecatedLicenseId\": false,\n      \"detailsUrl\": \"https://spdx.org/licenses/MulanPSL-1.0.json\",\n      \"referenceNumber\": 64,\n      \"name\": \"Mulan Permissive Software License, Version 1\",\n      \"licenseId\": \"MulanPSL-1.0\",\n      \"seeAlso\": [\n        \"https://license.coscl.org.cn/MulanPSL/\",\n        \"https://github.com/yuwenlong/longphp/blob/25dfb70cc2a466dc4bb55ba30901cbce08d164b5/LICENSE\"\n      ],\n      \"isOsiApproved\": false\n    },\n    {\n      \"reference\": \"https://spdx.org/licenses/MulanPSL-2.0.html\",\n      \"isDeprecatedLicenseId\": false,\n      \"detailsUrl\": \"https://spdx.org/licenses/MulanPSL-2.0.json\",\n      \"referenceNumber\": 383,\n      \"name\": \"Mulan Permissive Software License, Version 2\",\n      \"licenseId\": \"MulanPSL-2.0\",\n      \"seeAlso\": [\n        \"https://license.coscl.org.cn/MulanPSL2\"\n      ],\n      \"isOsiApproved\": true\n    },\n    {\n      \"reference\": \"https://spdx.org/licenses/Multics.html\",\n      \"isDeprecatedLicenseId\": false,\n      \"detailsUrl\": \"https://spdx.org/licenses/Multics.json\",\n      \"referenceNumber\": 102,\n      \"name\": \"Multics License\",\n      \"licenseId\": \"Multics\",\n      \"seeAlso\": [\n        \"https://opensource.org/licenses/Multics\"\n      ],\n      \"isOsiApproved\": true\n    },\n    {\n      \"reference\": \"https://spdx.org/licenses/Mup.html\",\n      \"isDeprecatedLicenseId\": false,\n      \"detailsUrl\": \"https://spdx.org/licenses/Mup.json\",\n      \"referenceNumber\": 18,\n      \"name\": \"Mup License\",\n      \"licenseId\": \"Mup\",\n      \"seeAlso\": [\n        \"https://fedoraproject.org/wiki/Licensing/Mup\"\n      ],\n      \"isOsiApproved\": false\n    },\n    {\n      \"reference\": \"https://spdx.org/licenses/NAIST-2003.html\",\n      \"isDeprecatedLicenseId\": false,\n      \"detailsUrl\": \"https://spdx.org/licenses/NAIST-2003.json\",\n      \"referenceNumber\": 307,\n      \"name\": \"Nara Institute of Science and Technology License (2003)\",\n      \"licenseId\": \"NAIST-2003\",\n      \"seeAlso\": [\n        \"https://enterprise.dejacode.com/licenses/public/naist-2003/#license-text\",\n        \"https://github.com/nodejs/node/blob/4a19cc8947b1bba2b2d27816ec3d0edf9b28e503/LICENSE#L343\"\n      ],\n      \"isOsiApproved\": false\n    },\n    {\n      \"reference\": \"https://spdx.org/licenses/NASA-1.3.html\",\n      \"isDeprecatedLicenseId\": false,\n      \"detailsUrl\": \"https://spdx.org/licenses/NASA-1.3.json\",\n      \"referenceNumber\": 495,\n      \"name\": \"NASA Open Source Agreement 1.3\",\n      \"licenseId\": \"NASA-1.3\",\n      \"seeAlso\": [\n        \"http://ti.arc.nasa.gov/opensource/nosa/\",\n        \"https://opensource.org/licenses/NASA-1.3\"\n      ],\n      \"isOsiApproved\": true,\n      \"isFsfLibre\": false\n    },\n    {\n      \"reference\": \"https://spdx.org/licenses/Naumen.html\",\n      \"isDeprecatedLicenseId\": false,\n      \"detailsUrl\": \"https://spdx.org/licenses/Naumen.json\",\n      \"referenceNumber\": 69,\n      \"name\": \"Naumen Public License\",\n      \"licenseId\": \"Naumen\",\n      \"seeAlso\": [\n        \"https://opensource.org/licenses/Naumen\"\n      ],\n      \"isOsiApproved\": true\n    },\n    {\n      \"reference\": \"https://spdx.org/licenses/NBPL-1.0.html\",\n      \"isDeprecatedLicenseId\": false,\n      \"detailsUrl\": \"https://spdx.org/licenses/NBPL-1.0.json\",\n      \"referenceNumber\": 409,\n      \"name\": \"Net Boolean Public License v1\",\n      \"licenseId\": \"NBPL-1.0\",\n      \"seeAlso\": [\n        \"http://www.openldap.org/devel/gitweb.cgi?p\\u003dopenldap.git;a\\u003dblob;f\\u003dLICENSE;hb\\u003d37b4b3f6cc4bf34e1d3dec61e69914b9819d8894\"\n      ],\n      \"isOsiApproved\": false\n    },\n    {\n      \"reference\": \"https://spdx.org/licenses/NCBI-PD.html\",\n      \"isDeprecatedLicenseId\": false,\n      \"detailsUrl\": \"https://spdx.org/licenses/NCBI-PD.json\",\n      \"referenceNumber\": 491,\n      \"name\": \"NCBI Public Domain Notice\",\n      \"licenseId\": \"NCBI-PD\",\n      \"seeAlso\": [\n        \"https://github.com/ncbi/sra-tools/blob/e8e5b6af4edc460156ad9ce5902d0779cffbf685/LICENSE\",\n        \"https://github.com/ncbi/datasets/blob/0ea4cd16b61e5b799d9cc55aecfa016d6c9bd2bf/LICENSE.md\",\n        \"https://github.com/ncbi/gprobe/blob/de64d30fee8b4c4013094d7d3139ea89b5dd1ace/LICENSE\",\n        \"https://github.com/ncbi/egapx/blob/08930b9dec0c69b2d1a05e5153c7b95ef0a3eb0f/LICENSE\",\n        \"https://github.com/ncbi/datasets/blob/master/LICENSE.md\"\n      ],\n      \"isOsiApproved\": false\n    },\n    {\n      \"reference\": \"https://spdx.org/licenses/NCGL-UK-2.0.html\",\n      \"isDeprecatedLicenseId\": false,\n      \"detailsUrl\": \"https://spdx.org/licenses/NCGL-UK-2.0.json\",\n      \"referenceNumber\": 517,\n      \"name\": \"Non-Commercial Government Licence\",\n      \"licenseId\": \"NCGL-UK-2.0\",\n      \"seeAlso\": [\n        \"http://www.nationalarchives.gov.uk/doc/non-commercial-government-licence/version/2/\"\n      ],\n      \"isOsiApproved\": false\n    },\n    {\n      \"reference\": \"https://spdx.org/licenses/NCL.html\",\n      \"isDeprecatedLicenseId\": false,\n      \"detailsUrl\": \"https://spdx.org/licenses/NCL.json\",\n      \"referenceNumber\": 406,\n      \"name\": \"NCL Source Code License\",\n      \"licenseId\": \"NCL\",\n      \"seeAlso\": [\n        \"https://gitlab.freedesktop.org/pipewire/pipewire/-/blob/master/src/modules/module-filter-chain/pffft.c?ref_type\\u003dheads#L1-52\"\n      ],\n      \"isOsiApproved\": false\n    },\n    {\n      \"reference\": \"https://spdx.org/licenses/NCSA.html\",\n      \"isDeprecatedLicenseId\": false,\n      \"detailsUrl\": \"https://spdx.org/licenses/NCSA.json\",\n      \"referenceNumber\": 41,\n      \"name\": \"University of Illinois/NCSA Open Source License\",\n      \"licenseId\": \"NCSA\",\n      \"seeAlso\": [\n        \"http://otm.illinois.edu/uiuc_openSource\",\n        \"https://opensource.org/licenses/NCSA\"\n      ],\n      \"isOsiApproved\": true,\n      \"isFsfLibre\": true\n    },\n    {\n      \"reference\": \"https://spdx.org/licenses/Net-SNMP.html\",\n      \"isDeprecatedLicenseId\": false,\n      \"detailsUrl\": \"https://spdx.org/licenses/Net-SNMP.json\",\n      \"referenceNumber\": 287,\n      \"name\": \"Net-SNMP License\",\n      \"licenseId\": \"Net-SNMP\",\n      \"seeAlso\": [\n        \"http://net-snmp.sourceforge.net/about/license.html\"\n      ],\n      \"isOsiApproved\": false\n    },\n    {\n      \"reference\": \"https://spdx.org/licenses/NetCDF.html\",\n      \"isDeprecatedLicenseId\": false,\n      \"detailsUrl\": \"https://spdx.org/licenses/NetCDF.json\",\n      \"referenceNumber\": 514,\n      \"name\": \"NetCDF license\",\n      \"licenseId\": \"NetCDF\",\n      \"seeAlso\": [\n        \"http://www.unidata.ucar.edu/software/netcdf/copyright.html\"\n      ],\n      \"isOsiApproved\": false\n    },\n    {\n      \"reference\": \"https://spdx.org/licenses/Newsletr.html\",\n      \"isDeprecatedLicenseId\": false,\n      \"detailsUrl\": \"https://spdx.org/licenses/Newsletr.json\",\n      \"referenceNumber\": 283,\n      \"name\": \"Newsletr License\",\n      \"licenseId\": \"Newsletr\",\n      \"seeAlso\": [\n        \"https://fedoraproject.org/wiki/Licensing/Newsletr\"\n      ],\n      \"isOsiApproved\": false\n    },\n    {\n      \"reference\": \"https://spdx.org/licenses/NGPL.html\",\n      \"isDeprecatedLicenseId\": false,\n      \"detailsUrl\": \"https://spdx.org/licenses/NGPL.json\",\n      \"referenceNumber\": 555,\n      \"name\": \"Nethack General Public License\",\n      \"licenseId\": \"NGPL\",\n      \"seeAlso\": [\n        \"https://opensource.org/licenses/NGPL\"\n      ],\n      \"isOsiApproved\": true\n    },\n    {\n      \"reference\": \"https://spdx.org/licenses/NICTA-1.0.html\",\n      \"isDeprecatedLicenseId\": false,\n      \"detailsUrl\": \"https://spdx.org/licenses/NICTA-1.0.json\",\n      \"referenceNumber\": 116,\n      \"name\": \"NICTA Public Software License, Version 1.0\",\n      \"licenseId\": \"NICTA-1.0\",\n      \"seeAlso\": [\n        \"https://opensource.apple.com/source/mDNSResponder/mDNSResponder-320.10/mDNSPosix/nss_ReadMe.txt\"\n      ],\n      \"isOsiApproved\": false\n    },\n    {\n      \"reference\": \"https://spdx.org/licenses/NIST-PD.html\",\n      \"isDeprecatedLicenseId\": false,\n      \"detailsUrl\": \"https://spdx.org/licenses/NIST-PD.json\",\n      \"referenceNumber\": 602,\n      \"name\": \"NIST Public Domain Notice\",\n      \"licenseId\": \"NIST-PD\",\n      \"seeAlso\": [\n        \"https://github.com/tcheneau/simpleRPL/blob/e645e69e38dd4e3ccfeceb2db8cba05b7c2e0cd3/LICENSE.txt\",\n        \"https://github.com/tcheneau/Routing/blob/f09f46fcfe636107f22f2c98348188a65a135d98/README.md\"\n      ],\n      \"isOsiApproved\": false\n    },\n    {\n      \"reference\": \"https://spdx.org/licenses/NIST-PD-fallback.html\",\n      \"isDeprecatedLicenseId\": false,\n      \"detailsUrl\": \"https://spdx.org/licenses/NIST-PD-fallback.json\",\n      \"referenceNumber\": 223,\n      \"name\": \"NIST Public Domain Notice with license fallback\",\n      \"licenseId\": \"NIST-PD-fallback\",\n      \"seeAlso\": [\n        \"https://github.com/usnistgov/jsip/blob/59700e6926cbe96c5cdae897d9a7d2656b42abe3/LICENSE\",\n        \"https://github.com/usnistgov/fipy/blob/86aaa5c2ba2c6f1be19593c5986071cf6568cc34/LICENSE.rst\"\n      ],\n      \"isOsiApproved\": false\n    },\n    {\n      \"reference\": \"https://spdx.org/licenses/NIST-Software.html\",\n      \"isDeprecatedLicenseId\": false,\n      \"detailsUrl\": \"https://spdx.org/licenses/NIST-Software.json\",\n      \"referenceNumber\": 248,\n      \"name\": \"NIST Software License\",\n      \"licenseId\": \"NIST-Software\",\n      \"seeAlso\": [\n        \"https://github.com/open-quantum-safe/liboqs/blob/40b01fdbb270f8614fde30e65d30e9da18c02393/src/common/rand/rand_nist.c#L1-L15\"\n      ],\n      \"isOsiApproved\": false\n    },\n    {\n      \"reference\": \"https://spdx.org/licenses/NLOD-1.0.html\",\n      \"isDeprecatedLicenseId\": false,\n      \"detailsUrl\": \"https://spdx.org/licenses/NLOD-1.0.json\",\n      \"referenceNumber\": 565,\n      \"name\": \"Norwegian Licence for Open Government Data (NLOD) 1.0\",\n      \"licenseId\": \"NLOD-1.0\",\n      \"seeAlso\": [\n        \"http://data.norge.no/nlod/en/1.0\"\n      ],\n      \"isOsiApproved\": false\n    },\n    {\n      \"reference\": \"https://spdx.org/licenses/NLOD-2.0.html\",\n      \"isDeprecatedLicenseId\": false,\n      \"detailsUrl\": \"https://spdx.org/licenses/NLOD-2.0.json\",\n      \"referenceNumber\": 177,\n      \"name\": \"Norwegian Licence for Open Government Data (NLOD) 2.0\",\n      \"licenseId\": \"NLOD-2.0\",\n      \"seeAlso\": [\n        \"http://data.norge.no/nlod/en/2.0\"\n      ],\n      \"isOsiApproved\": false\n    },\n    {\n      \"reference\": \"https://spdx.org/licenses/NLPL.html\",\n      \"isDeprecatedLicenseId\": false,\n      \"detailsUrl\": \"https://spdx.org/licenses/NLPL.json\",\n      \"referenceNumber\": 322,\n      \"name\": \"No Limit Public License\",\n      \"licenseId\": \"NLPL\",\n      \"seeAlso\": [\n        \"https://fedoraproject.org/wiki/Licensing/NLPL\"\n      ],\n      \"isOsiApproved\": false\n    },\n    {\n      \"reference\": \"https://spdx.org/licenses/Nokia.html\",\n      \"isDeprecatedLicenseId\": false,\n      \"detailsUrl\": \"https://spdx.org/licenses/Nokia.json\",\n      \"referenceNumber\": 376,\n      \"name\": \"Nokia Open Source License\",\n      \"licenseId\": \"Nokia\",\n      \"seeAlso\": [\n        \"https://opensource.org/licenses/nokia\"\n      ],\n      \"isOsiApproved\": true,\n      \"isFsfLibre\": true\n    },\n    {\n      \"reference\": \"https://spdx.org/licenses/NOSL.html\",\n      \"isDeprecatedLicenseId\": false,\n      \"detailsUrl\": \"https://spdx.org/licenses/NOSL.json\",\n      \"referenceNumber\": 182,\n      \"name\": \"Netizen Open Source License\",\n      \"licenseId\": \"NOSL\",\n      \"seeAlso\": [\n        \"http://bits.netizen.com.au/licenses/NOSL/nosl.txt\"\n      ],\n      \"isOsiApproved\": false,\n      \"isFsfLibre\": true\n    },\n    {\n      \"reference\": \"https://spdx.org/licenses/Noweb.html\",\n      \"isDeprecatedLicenseId\": false,\n      \"detailsUrl\": \"https://spdx.org/licenses/Noweb.json\",\n      \"referenceNumber\": 6,\n      \"name\": \"Noweb License\",\n      \"licenseId\": \"Noweb\",\n      \"seeAlso\": [\n        \"https://fedoraproject.org/wiki/Licensing/Noweb\"\n      ],\n      \"isOsiApproved\": false\n    },\n    {\n      \"reference\": \"https://spdx.org/licenses/NPL-1.0.html\",\n      \"isDeprecatedLicenseId\": false,\n      \"detailsUrl\": \"https://spdx.org/licenses/NPL-1.0.json\",\n      \"referenceNumber\": 257,\n      \"name\": \"Netscape Public License v1.0\",\n      \"licenseId\": \"NPL-1.0\",\n      \"seeAlso\": [\n        \"http://www.mozilla.org/MPL/NPL/1.0/\"\n      ],\n      \"isOsiApproved\": false,\n      \"isFsfLibre\": true\n    },\n    {\n      \"reference\": \"https://spdx.org/licenses/NPL-1.1.html\",\n      \"isDeprecatedLicenseId\": false,\n      \"detailsUrl\": \"https://spdx.org/licenses/NPL-1.1.json\",\n      \"referenceNumber\": 54,\n      \"name\": \"Netscape Public License v1.1\",\n      \"licenseId\": \"NPL-1.1\",\n      \"seeAlso\": [\n        \"http://www.mozilla.org/MPL/NPL/1.1/\"\n      ],\n      \"isOsiApproved\": false,\n      \"isFsfLibre\": true\n    },\n    {\n      \"reference\": \"https://spdx.org/licenses/NPOSL-3.0.html\",\n      \"isDeprecatedLicenseId\": false,\n      \"detailsUrl\": \"https://spdx.org/licenses/NPOSL-3.0.json\",\n      \"referenceNumber\": 656,\n      \"name\": \"Non-Profit Open Software License 3.0\",\n      \"licenseId\": \"NPOSL-3.0\",\n      \"seeAlso\": [\n        \"https://opensource.org/licenses/NOSL3.0\"\n      ],\n      \"isOsiApproved\": true\n    },\n    {\n      \"reference\": \"https://spdx.org/licenses/NRL.html\",\n      \"isDeprecatedLicenseId\": false,\n      \"detailsUrl\": \"https://spdx.org/licenses/NRL.json\",\n      \"referenceNumber\": 284,\n      \"name\": \"NRL License\",\n      \"licenseId\": \"NRL\",\n      \"seeAlso\": [\n        \"http://web.mit.edu/network/isakmp/nrllicense.html\"\n      ],\n      \"isOsiApproved\": false\n    },\n    {\n      \"reference\": \"https://spdx.org/licenses/NTP.html\",\n      \"isDeprecatedLicenseId\": false,\n      \"detailsUrl\": \"https://spdx.org/licenses/NTP.json\",\n      \"referenceNumber\": 196,\n      \"name\": \"NTP License\",\n      \"licenseId\": \"NTP\",\n      \"seeAlso\": [\n        \"https://opensource.org/licenses/NTP\"\n      ],\n      \"isOsiApproved\": true\n    },\n    {\n      \"reference\": \"https://spdx.org/licenses/NTP-0.html\",\n      \"isDeprecatedLicenseId\": false,\n      \"detailsUrl\": \"https://spdx.org/licenses/NTP-0.json\",\n      \"referenceNumber\": 197,\n      \"name\": \"NTP No Attribution\",\n      \"licenseId\": \"NTP-0\",\n      \"seeAlso\": [\n        \"https://github.com/tytso/e2fsprogs/blob/master/lib/et/et_name.c\"\n      ],\n      \"isOsiApproved\": false\n    },\n    {\n      \"reference\": \"https://spdx.org/licenses/Nunit.html\",\n      \"isDeprecatedLicenseId\": true,\n      \"detailsUrl\": \"https://spdx.org/licenses/Nunit.json\",\n      \"referenceNumber\": 207,\n      \"name\": \"Nunit License\",\n      \"licenseId\": \"Nunit\",\n      \"seeAlso\": [\n        \"https://fedoraproject.org/wiki/Licensing/Nunit\"\n      ],\n      \"isOsiApproved\": false,\n      \"isFsfLibre\": true\n    },\n    {\n      \"reference\": \"https://spdx.org/licenses/O-UDA-1.0.html\",\n      \"isDeprecatedLicenseId\": false,\n      \"detailsUrl\": \"https://spdx.org/licenses/O-UDA-1.0.json\",\n      \"referenceNumber\": 366,\n      \"name\": \"Open Use of Data Agreement v1.0\",\n      \"licenseId\": \"O-UDA-1.0\",\n      \"seeAlso\": [\n        \"https://github.com/microsoft/Open-Use-of-Data-Agreement/blob/v1.0/O-UDA-1.0.md\",\n        \"https://cdla.dev/open-use-of-data-agreement-v1-0/\"\n      ],\n      \"isOsiApproved\": false\n    },\n    {\n      \"reference\": \"https://spdx.org/licenses/OAR.html\",\n      \"isDeprecatedLicenseId\": false,\n      \"detailsUrl\": \"https://spdx.org/licenses/OAR.json\",\n      \"referenceNumber\": 357,\n      \"name\": \"OAR License\",\n      \"licenseId\": \"OAR\",\n      \"seeAlso\": [\n        \"https://sourceware.org/git/?p\\u003dnewlib-cygwin.git;a\\u003dblob;f\\u003dnewlib/libc/string/strsignal.c;hb\\u003dHEAD#l35\"\n      ],\n      \"isOsiApproved\": false\n    },\n    {\n      \"reference\": \"https://spdx.org/licenses/OCCT-PL.html\",\n      \"isDeprecatedLicenseId\": false,\n      \"detailsUrl\": \"https://spdx.org/licenses/OCCT-PL.json\",\n      \"referenceNumber\": 484,\n      \"name\": \"Open CASCADE Technology Public License\",\n      \"licenseId\": \"OCCT-PL\",\n      \"seeAlso\": [\n        \"http://www.opencascade.com/content/occt-public-license\"\n      ],\n      \"isOsiApproved\": false\n    },\n    {\n      \"reference\": \"https://spdx.org/licenses/OCLC-2.0.html\",\n      \"isDeprecatedLicenseId\": false,\n      \"detailsUrl\": \"https://spdx.org/licenses/OCLC-2.0.json\",\n      \"referenceNumber\": 170,\n      \"name\": \"OCLC Research Public License 2.0\",\n      \"licenseId\": \"OCLC-2.0\",\n      \"seeAlso\": [\n        \"http://www.oclc.org/research/activities/software/license/v2final.htm\",\n        \"https://opensource.org/licenses/OCLC-2.0\"\n      ],\n      \"isOsiApproved\": true\n    },\n    {\n      \"reference\": \"https://spdx.org/licenses/ODbL-1.0.html\",\n      \"isDeprecatedLicenseId\": false,\n      \"detailsUrl\": \"https://spdx.org/licenses/ODbL-1.0.json\",\n      \"referenceNumber\": 631,\n      \"name\": \"Open Data Commons Open Database License v1.0\",\n      \"licenseId\": \"ODbL-1.0\",\n      \"seeAlso\": [\n        \"http://www.opendatacommons.org/licenses/odbl/1.0/\",\n        \"https://opendatacommons.org/licenses/odbl/1-0/\"\n      ],\n      \"isOsiApproved\": false,\n      \"isFsfLibre\": true\n    },\n    {\n      \"reference\": \"https://spdx.org/licenses/ODC-By-1.0.html\",\n      \"isDeprecatedLicenseId\": false,\n      \"detailsUrl\": \"https://spdx.org/licenses/ODC-By-1.0.json\",\n      \"referenceNumber\": 505,\n      \"name\": \"Open Data Commons Attribution License v1.0\",\n      \"licenseId\": \"ODC-By-1.0\",\n      \"seeAlso\": [\n        \"https://opendatacommons.org/licenses/by/1.0/\"\n      ],\n      \"isOsiApproved\": false\n    },\n    {\n      \"reference\": \"https://spdx.org/licenses/OFFIS.html\",\n      \"isDeprecatedLicenseId\": false,\n      \"detailsUrl\": \"https://spdx.org/licenses/OFFIS.json\",\n      \"referenceNumber\": 489,\n      \"name\": \"OFFIS License\",\n      \"licenseId\": \"OFFIS\",\n      \"seeAlso\": [\n        \"https://sourceforge.net/p/xmedcon/code/ci/master/tree/libs/dicom/README\"\n      ],\n      \"isOsiApproved\": false\n    },\n    {\n      \"reference\": \"https://spdx.org/licenses/OFL-1.0.html\",\n      \"isDeprecatedLicenseId\": false,\n      \"detailsUrl\": \"https://spdx.org/licenses/OFL-1.0.json\",\n      \"referenceNumber\": 24,\n      \"name\": \"SIL Open Font License 1.0\",\n      \"licenseId\": \"OFL-1.0\",\n      \"seeAlso\": [\n        \"http://scripts.sil.org/cms/scripts/page.php?item_id\\u003dOFL10_web\"\n      ],\n      \"isOsiApproved\": false,\n      \"isFsfLibre\": true\n    },\n    {\n      \"reference\": \"https://spdx.org/licenses/OFL-1.0-no-RFN.html\",\n      \"isDeprecatedLicenseId\": false,\n      \"detailsUrl\": \"https://spdx.org/licenses/OFL-1.0-no-RFN.json\",\n      \"referenceNumber\": 325,\n      \"name\": \"SIL Open Font License 1.0 with no Reserved Font Name\",\n      \"licenseId\": \"OFL-1.0-no-RFN\",\n      \"seeAlso\": [\n        \"http://scripts.sil.org/cms/scripts/page.php?item_id\\u003dOFL10_web\"\n      ],\n      \"isOsiApproved\": false\n    },\n    {\n      \"reference\": \"https://spdx.org/licenses/OFL-1.0-RFN.html\",\n      \"isDeprecatedLicenseId\": false,\n      \"detailsUrl\": \"https://spdx.org/licenses/OFL-1.0-RFN.json\",\n      \"referenceNumber\": 162,\n      \"name\": \"SIL Open Font License 1.0 with Reserved Font Name\",\n      \"licenseId\": \"OFL-1.0-RFN\",\n      \"seeAlso\": [\n        \"http://scripts.sil.org/cms/scripts/page.php?item_id\\u003dOFL10_web\"\n      ],\n      \"isOsiApproved\": false\n    },\n    {\n      \"reference\": \"https://spdx.org/licenses/OFL-1.1.html\",\n      \"isDeprecatedLicenseId\": false,\n      \"detailsUrl\": \"https://spdx.org/licenses/OFL-1.1.json\",\n      \"referenceNumber\": 240,\n      \"name\": \"SIL Open Font License 1.1\",\n      \"licenseId\": \"OFL-1.1\",\n      \"seeAlso\": [\n        \"http://scripts.sil.org/cms/scripts/page.php?item_id\\u003dOFL_web\",\n        \"https://opensource.org/licenses/OFL-1.1\"\n      ],\n      \"isOsiApproved\": true,\n      \"isFsfLibre\": true\n    },\n    {\n      \"reference\": \"https://spdx.org/licenses/OFL-1.1-no-RFN.html\",\n      \"isDeprecatedLicenseId\": false,\n      \"detailsUrl\": \"https://spdx.org/licenses/OFL-1.1-no-RFN.json\",\n      \"referenceNumber\": 157,\n      \"name\": \"SIL Open Font License 1.1 with no Reserved Font Name\",\n      \"licenseId\": \"OFL-1.1-no-RFN\",\n      \"seeAlso\": [\n        \"http://scripts.sil.org/cms/scripts/page.php?item_id\\u003dOFL_web\",\n        \"https://opensource.org/licenses/OFL-1.1\"\n      ],\n      \"isOsiApproved\": true\n    },\n    {\n      \"reference\": \"https://spdx.org/licenses/OFL-1.1-RFN.html\",\n      \"isDeprecatedLicenseId\": false,\n      \"detailsUrl\": \"https://spdx.org/licenses/OFL-1.1-RFN.json\",\n      \"referenceNumber\": 537,\n      \"name\": \"SIL Open Font License 1.1 with Reserved Font Name\",\n      \"licenseId\": \"OFL-1.1-RFN\",\n      \"seeAlso\": [\n        \"http://scripts.sil.org/cms/scripts/page.php?item_id\\u003dOFL_web\",\n        \"https://opensource.org/licenses/OFL-1.1\"\n      ],\n      \"isOsiApproved\": true\n    },\n    {\n      \"reference\": \"https://spdx.org/licenses/OGC-1.0.html\",\n      \"isDeprecatedLicenseId\": false,\n      \"detailsUrl\": \"https://spdx.org/licenses/OGC-1.0.json\",\n      \"referenceNumber\": 465,\n      \"name\": \"OGC Software License, Version 1.0\",\n      \"licenseId\": \"OGC-1.0\",\n      \"seeAlso\": [\n        \"https://www.ogc.org/ogc/software/1.0\"\n      ],\n      \"isOsiApproved\": false\n    },\n    {\n      \"reference\": \"https://spdx.org/licenses/OGDL-Taiwan-1.0.html\",\n      \"isDeprecatedLicenseId\": false,\n      \"detailsUrl\": \"https://spdx.org/licenses/OGDL-Taiwan-1.0.json\",\n      \"referenceNumber\": 8,\n      \"name\": \"Taiwan Open Government Data License, version 1.0\",\n      \"licenseId\": \"OGDL-Taiwan-1.0\",\n      \"seeAlso\": [\n        \"https://data.gov.tw/license\"\n      ],\n      \"isOsiApproved\": false\n    },\n    {\n      \"reference\": \"https://spdx.org/licenses/OGL-Canada-2.0.html\",\n      \"isDeprecatedLicenseId\": false,\n      \"detailsUrl\": \"https://spdx.org/licenses/OGL-Canada-2.0.json\",\n      \"referenceNumber\": 9,\n      \"name\": \"Open Government Licence - Canada\",\n      \"licenseId\": \"OGL-Canada-2.0\",\n      \"seeAlso\": [\n        \"https://open.canada.ca/en/open-government-licence-canada\"\n      ],\n      \"isOsiApproved\": false\n    },\n    {\n      \"reference\": \"https://spdx.org/licenses/OGL-UK-1.0.html\",\n      \"isDeprecatedLicenseId\": false,\n      \"detailsUrl\": \"https://spdx.org/licenses/OGL-UK-1.0.json\",\n      \"referenceNumber\": 221,\n      \"name\": \"Open Government Licence v1.0\",\n      \"licenseId\": \"OGL-UK-1.0\",\n      \"seeAlso\": [\n        \"http://www.nationalarchives.gov.uk/doc/open-government-licence/version/1/\"\n      ],\n      \"isOsiApproved\": false\n    },\n    {\n      \"reference\": \"https://spdx.org/licenses/OGL-UK-2.0.html\",\n      \"isDeprecatedLicenseId\": false,\n      \"detailsUrl\": \"https://spdx.org/licenses/OGL-UK-2.0.json\",\n      \"referenceNumber\": 369,\n      \"name\": \"Open Government Licence v2.0\",\n      \"licenseId\": \"OGL-UK-2.0\",\n      \"seeAlso\": [\n        \"http://www.nationalarchives.gov.uk/doc/open-government-licence/version/2/\"\n      ],\n      \"isOsiApproved\": false\n    },\n    {\n      \"reference\": \"https://spdx.org/licenses/OGL-UK-3.0.html\",\n      \"isDeprecatedLicenseId\": false,\n      \"detailsUrl\": \"https://spdx.org/licenses/OGL-UK-3.0.json\",\n      \"referenceNumber\": 455,\n      \"name\": \"Open Government Licence v3.0\",\n      \"licenseId\": \"OGL-UK-3.0\",\n      \"seeAlso\": [\n        \"http://www.nationalarchives.gov.uk/doc/open-government-licence/version/3/\"\n      ],\n      \"isOsiApproved\": false\n    },\n    {\n      \"reference\": \"https://spdx.org/licenses/OGTSL.html\",\n      \"isDeprecatedLicenseId\": false,\n      \"detailsUrl\": \"https://spdx.org/licenses/OGTSL.json\",\n      \"referenceNumber\": 235,\n      \"name\": \"Open Group Test Suite License\",\n      \"licenseId\": \"OGTSL\",\n      \"seeAlso\": [\n        \"http://www.opengroup.org/testing/downloads/The_Open_Group_TSL.txt\",\n        \"https://opensource.org/licenses/OGTSL\"\n      ],\n      \"isOsiApproved\": true\n    },\n    {\n      \"reference\": \"https://spdx.org/licenses/OLDAP-1.1.html\",\n      \"isDeprecatedLicenseId\": false,\n      \"detailsUrl\": \"https://spdx.org/licenses/OLDAP-1.1.json\",\n      \"referenceNumber\": 111,\n      \"name\": \"Open LDAP Public License v1.1\",\n      \"licenseId\": \"OLDAP-1.1\",\n      \"seeAlso\": [\n        \"http://www.openldap.org/devel/gitweb.cgi?p\\u003dopenldap.git;a\\u003dblob;f\\u003dLICENSE;hb\\u003d806557a5ad59804ef3a44d5abfbe91d706b0791f\"\n      ],\n      \"isOsiApproved\": false\n    },\n    {\n      \"reference\": \"https://spdx.org/licenses/OLDAP-1.2.html\",\n      \"isDeprecatedLicenseId\": false,\n      \"detailsUrl\": \"https://spdx.org/licenses/OLDAP-1.2.json\",\n      \"referenceNumber\": 164,\n      \"name\": \"Open LDAP Public License v1.2\",\n      \"licenseId\": \"OLDAP-1.2\",\n      \"seeAlso\": [\n        \"http://www.openldap.org/devel/gitweb.cgi?p\\u003dopenldap.git;a\\u003dblob;f\\u003dLICENSE;hb\\u003d42b0383c50c299977b5893ee695cf4e486fb0dc7\"\n      ],\n      \"isOsiApproved\": false\n    },\n    {\n      \"reference\": \"https://spdx.org/licenses/OLDAP-1.3.html\",\n      \"isDeprecatedLicenseId\": false,\n      \"detailsUrl\": \"https://spdx.org/licenses/OLDAP-1.3.json\",\n      \"referenceNumber\": 55,\n      \"name\": \"Open LDAP Public License v1.3\",\n      \"licenseId\": \"OLDAP-1.3\",\n      \"seeAlso\": [\n        \"http://www.openldap.org/devel/gitweb.cgi?p\\u003dopenldap.git;a\\u003dblob;f\\u003dLICENSE;hb\\u003de5f8117f0ce088d0bd7a8e18ddf37eaa40eb09b1\"\n      ],\n      \"isOsiApproved\": false\n    },\n    {\n      \"reference\": \"https://spdx.org/licenses/OLDAP-1.4.html\",\n      \"isDeprecatedLicenseId\": false,\n      \"detailsUrl\": \"https://spdx.org/licenses/OLDAP-1.4.json\",\n      \"referenceNumber\": 439,\n      \"name\": \"Open LDAP Public License v1.4\",\n      \"licenseId\": \"OLDAP-1.4\",\n      \"seeAlso\": [\n        \"http://www.openldap.org/devel/gitweb.cgi?p\\u003dopenldap.git;a\\u003dblob;f\\u003dLICENSE;hb\\u003dc9f95c2f3f2ffb5e0ae55fe7388af75547660941\"\n      ],\n      \"isOsiApproved\": false\n    },\n    {\n      \"reference\": \"https://spdx.org/licenses/OLDAP-2.0.html\",\n      \"isDeprecatedLicenseId\": false,\n      \"detailsUrl\": \"https://spdx.org/licenses/OLDAP-2.0.json\",\n      \"referenceNumber\": 90,\n      \"name\": \"Open LDAP Public License v2.0 (or possibly 2.0A and 2.0B)\",\n      \"licenseId\": \"OLDAP-2.0\",\n      \"seeAlso\": [\n        \"http://www.openldap.org/devel/gitweb.cgi?p\\u003dopenldap.git;a\\u003dblob;f\\u003dLICENSE;hb\\u003dcbf50f4e1185a21abd4c0a54d3f4341fe28f36ea\"\n      ],\n      \"isOsiApproved\": false\n    },\n    {\n      \"reference\": \"https://spdx.org/licenses/OLDAP-2.0.1.html\",\n      \"isDeprecatedLicenseId\": false,\n      \"detailsUrl\": \"https://spdx.org/licenses/OLDAP-2.0.1.json\",\n      \"referenceNumber\": 4,\n      \"name\": \"Open LDAP Public License v2.0.1\",\n      \"licenseId\": \"OLDAP-2.0.1\",\n      \"seeAlso\": [\n        \"http://www.openldap.org/devel/gitweb.cgi?p\\u003dopenldap.git;a\\u003dblob;f\\u003dLICENSE;hb\\u003db6d68acd14e51ca3aab4428bf26522aa74873f0e\"\n      ],\n      \"isOsiApproved\": false\n    },\n    {\n      \"reference\": \"https://spdx.org/licenses/OLDAP-2.1.html\",\n      \"isDeprecatedLicenseId\": false,\n      \"detailsUrl\": \"https://spdx.org/licenses/OLDAP-2.1.json\",\n      \"referenceNumber\": 543,\n      \"name\": \"Open LDAP Public License v2.1\",\n      \"licenseId\": \"OLDAP-2.1\",\n      \"seeAlso\": [\n        \"http://www.openldap.org/devel/gitweb.cgi?p\\u003dopenldap.git;a\\u003dblob;f\\u003dLICENSE;hb\\u003db0d176738e96a0d3b9f85cb51e140a86f21be715\"\n      ],\n      \"isOsiApproved\": false\n    },\n    {\n      \"reference\": \"https://spdx.org/licenses/OLDAP-2.2.html\",\n      \"isDeprecatedLicenseId\": false,\n      \"detailsUrl\": \"https://spdx.org/licenses/OLDAP-2.2.json\",\n      \"referenceNumber\": 630,\n      \"name\": \"Open LDAP Public License v2.2\",\n      \"licenseId\": \"OLDAP-2.2\",\n      \"seeAlso\": [\n        \"http://www.openldap.org/devel/gitweb.cgi?p\\u003dopenldap.git;a\\u003dblob;f\\u003dLICENSE;hb\\u003d470b0c18ec67621c85881b2733057fecf4a1acc3\"\n      ],\n      \"isOsiApproved\": false\n    },\n    {\n      \"reference\": \"https://spdx.org/licenses/OLDAP-2.2.1.html\",\n      \"isDeprecatedLicenseId\": false,\n      \"detailsUrl\": \"https://spdx.org/licenses/OLDAP-2.2.1.json\",\n      \"referenceNumber\": 597,\n      \"name\": \"Open LDAP Public License v2.2.1\",\n      \"licenseId\": \"OLDAP-2.2.1\",\n      \"seeAlso\": [\n        \"http://www.openldap.org/devel/gitweb.cgi?p\\u003dopenldap.git;a\\u003dblob;f\\u003dLICENSE;hb\\u003d4bc786f34b50aa301be6f5600f58a980070f481e\"\n      ],\n      \"isOsiApproved\": false\n    },\n    {\n      \"reference\": \"https://spdx.org/licenses/OLDAP-2.2.2.html\",\n      \"isDeprecatedLicenseId\": false,\n      \"detailsUrl\": \"https://spdx.org/licenses/OLDAP-2.2.2.json\",\n      \"referenceNumber\": 67,\n      \"name\": \"Open LDAP Public License 2.2.2\",\n      \"licenseId\": \"OLDAP-2.2.2\",\n      \"seeAlso\": [\n        \"http://www.openldap.org/devel/gitweb.cgi?p\\u003dopenldap.git;a\\u003dblob;f\\u003dLICENSE;hb\\u003ddf2cc1e21eb7c160695f5b7cffd6296c151ba188\"\n      ],\n      \"isOsiApproved\": false\n    },\n    {\n      \"reference\": \"https://spdx.org/licenses/OLDAP-2.3.html\",\n      \"isDeprecatedLicenseId\": false,\n      \"detailsUrl\": \"https://spdx.org/licenses/OLDAP-2.3.json\",\n      \"referenceNumber\": 328,\n      \"name\": \"Open LDAP Public License v2.3\",\n      \"licenseId\": \"OLDAP-2.3\",\n      \"seeAlso\": [\n        \"http://www.openldap.org/devel/gitweb.cgi?p\\u003dopenldap.git;a\\u003dblob;f\\u003dLICENSE;hb\\u003dd32cf54a32d581ab475d23c810b0a7fbaf8d63c3\"\n      ],\n      \"isOsiApproved\": false,\n      \"isFsfLibre\": true\n    },\n    {\n      \"reference\": \"https://spdx.org/licenses/OLDAP-2.4.html\",\n      \"isDeprecatedLicenseId\": false,\n      \"detailsUrl\": \"https://spdx.org/licenses/OLDAP-2.4.json\",\n      \"referenceNumber\": 108,\n      \"name\": \"Open LDAP Public License v2.4\",\n      \"licenseId\": \"OLDAP-2.4\",\n      \"seeAlso\": [\n        \"http://www.openldap.org/devel/gitweb.cgi?p\\u003dopenldap.git;a\\u003dblob;f\\u003dLICENSE;hb\\u003dcd1284c4a91a8a380d904eee68d1583f989ed386\"\n      ],\n      \"isOsiApproved\": false\n    },\n    {\n      \"reference\": \"https://spdx.org/licenses/OLDAP-2.5.html\",\n      \"isDeprecatedLicenseId\": false,\n      \"detailsUrl\": \"https://spdx.org/licenses/OLDAP-2.5.json\",\n      \"referenceNumber\": 657,\n      \"name\": \"Open LDAP Public License v2.5\",\n      \"licenseId\": \"OLDAP-2.5\",\n      \"seeAlso\": [\n        \"http://www.openldap.org/devel/gitweb.cgi?p\\u003dopenldap.git;a\\u003dblob;f\\u003dLICENSE;hb\\u003d6852b9d90022e8593c98205413380536b1b5a7cf\"\n      ],\n      \"isOsiApproved\": false\n    },\n    {\n      \"reference\": \"https://spdx.org/licenses/OLDAP-2.6.html\",\n      \"isDeprecatedLicenseId\": false,\n      \"detailsUrl\": \"https://spdx.org/licenses/OLDAP-2.6.json\",\n      \"referenceNumber\": 634,\n      \"name\": \"Open LDAP Public License v2.6\",\n      \"licenseId\": \"OLDAP-2.6\",\n      \"seeAlso\": [\n        \"http://www.openldap.org/devel/gitweb.cgi?p\\u003dopenldap.git;a\\u003dblob;f\\u003dLICENSE;hb\\u003d1cae062821881f41b73012ba816434897abf4205\"\n      ],\n      \"isOsiApproved\": false\n    },\n    {\n      \"reference\": \"https://spdx.org/licenses/OLDAP-2.7.html\",\n      \"isDeprecatedLicenseId\": false,\n      \"detailsUrl\": \"https://spdx.org/licenses/OLDAP-2.7.json\",\n      \"referenceNumber\": 193,\n      \"name\": \"Open LDAP Public License v2.7\",\n      \"licenseId\": \"OLDAP-2.7\",\n      \"seeAlso\": [\n        \"http://www.openldap.org/devel/gitweb.cgi?p\\u003dopenldap.git;a\\u003dblob;f\\u003dLICENSE;hb\\u003d47c2415c1df81556eeb39be6cad458ef87c534a2\"\n      ],\n      \"isOsiApproved\": false,\n      \"isFsfLibre\": true\n    },\n    {\n      \"reference\": \"https://spdx.org/licenses/OLDAP-2.8.html\",\n      \"isDeprecatedLicenseId\": false,\n      \"detailsUrl\": \"https://spdx.org/licenses/OLDAP-2.8.json\",\n      \"referenceNumber\": 447,\n      \"name\": \"Open LDAP Public License v2.8\",\n      \"licenseId\": \"OLDAP-2.8\",\n      \"seeAlso\": [\n        \"http://www.openldap.org/software/release/license.html\"\n      ],\n      \"isOsiApproved\": true\n    },\n    {\n      \"reference\": \"https://spdx.org/licenses/OLFL-1.3.html\",\n      \"isDeprecatedLicenseId\": false,\n      \"detailsUrl\": \"https://spdx.org/licenses/OLFL-1.3.json\",\n      \"referenceNumber\": 531,\n      \"name\": \"Open Logistics Foundation License Version 1.3\",\n      \"licenseId\": \"OLFL-1.3\",\n      \"seeAlso\": [\n        \"https://openlogisticsfoundation.org/licenses/\",\n        \"https://opensource.org/license/olfl-1-3/\"\n      ],\n      \"isOsiApproved\": true\n    },\n    {\n      \"reference\": \"https://spdx.org/licenses/OML.html\",\n      \"isDeprecatedLicenseId\": false,\n      \"detailsUrl\": \"https://spdx.org/licenses/OML.json\",\n      \"referenceNumber\": 101,\n      \"name\": \"Open Market License\",\n      \"licenseId\": \"OML\",\n      \"seeAlso\": [\n        \"https://fedoraproject.org/wiki/Licensing/Open_Market_License\"\n      ],\n      \"isOsiApproved\": false\n    },\n    {\n      \"reference\": \"https://spdx.org/licenses/OpenPBS-2.3.html\",\n      \"isDeprecatedLicenseId\": false,\n      \"detailsUrl\": \"https://spdx.org/licenses/OpenPBS-2.3.json\",\n      \"referenceNumber\": 286,\n      \"name\": \"OpenPBS v2.3 Software License\",\n      \"licenseId\": \"OpenPBS-2.3\",\n      \"seeAlso\": [\n        \"https://github.com/adaptivecomputing/torque/blob/master/PBS_License.txt\",\n        \"https://www.mcs.anl.gov/research/projects/openpbs/PBS_License.txt\"\n      ],\n      \"isOsiApproved\": false\n    },\n    {\n      \"reference\": \"https://spdx.org/licenses/OpenSSL.html\",\n      \"isDeprecatedLicenseId\": false,\n      \"detailsUrl\": \"https://spdx.org/licenses/OpenSSL.json\",\n      \"referenceNumber\": 591,\n      \"name\": \"OpenSSL License\",\n      \"licenseId\": \"OpenSSL\",\n      \"seeAlso\": [\n        \"http://www.openssl.org/source/license.html\"\n      ],\n      \"isOsiApproved\": false,\n      \"isFsfLibre\": true\n    },\n    {\n      \"reference\": \"https://spdx.org/licenses/OpenSSL-standalone.html\",\n      \"isDeprecatedLicenseId\": false,\n      \"detailsUrl\": \"https://spdx.org/licenses/OpenSSL-standalone.json\",\n      \"referenceNumber\": 611,\n      \"name\": \"OpenSSL License - standalone\",\n      \"licenseId\": \"OpenSSL-standalone\",\n      \"seeAlso\": [\n        \"https://library.netapp.com/ecm/ecm_download_file/ECMP1196395\",\n        \"https://hstechdocs.helpsystems.com/manuals/globalscape/archive/cuteftp6/open_ssl_license_agreement.htm\"\n      ],\n      \"isOsiApproved\": false\n    },\n    {\n      \"reference\": \"https://spdx.org/licenses/OpenVision.html\",\n      \"isDeprecatedLicenseId\": false,\n      \"detailsUrl\": \"https://spdx.org/licenses/OpenVision.json\",\n      \"referenceNumber\": 563,\n      \"name\": \"OpenVision License\",\n      \"licenseId\": \"OpenVision\",\n      \"seeAlso\": [\n        \"https://github.com/krb5/krb5/blob/krb5-1.21.2-final/NOTICE#L66-L98\",\n        \"https://web.mit.edu/kerberos/krb5-1.21/doc/mitK5license.html\",\n        \"https://fedoraproject.org/wiki/Licensing:MIT#OpenVision_Variant\"\n      ],\n      \"isOsiApproved\": false\n    },\n    {\n      \"reference\": \"https://spdx.org/licenses/OPL-1.0.html\",\n      \"isDeprecatedLicenseId\": false,\n      \"detailsUrl\": \"https://spdx.org/licenses/OPL-1.0.json\",\n      \"referenceNumber\": 179,\n      \"name\": \"Open Public License v1.0\",\n      \"licenseId\": \"OPL-1.0\",\n      \"seeAlso\": [\n        \"http://old.koalateam.com/jackaroo/OPL_1_0.TXT\",\n        \"https://fedoraproject.org/wiki/Licensing/Open_Public_License\"\n      ],\n      \"isOsiApproved\": false,\n      \"isFsfLibre\": false\n    },\n    {\n      \"reference\": \"https://spdx.org/licenses/OPL-UK-3.0.html\",\n      \"isDeprecatedLicenseId\": false,\n      \"detailsUrl\": \"https://spdx.org/licenses/OPL-UK-3.0.json\",\n      \"referenceNumber\": 464,\n      \"name\": \"United    Kingdom Open Parliament Licence v3.0\",\n      \"licenseId\": \"OPL-UK-3.0\",\n      \"seeAlso\": [\n        \"https://www.parliament.uk/site-information/copyright-parliament/open-parliament-licence/\"\n      ],\n      \"isOsiApproved\": false\n    },\n    {\n      \"reference\": \"https://spdx.org/licenses/OPUBL-1.0.html\",\n      \"isDeprecatedLicenseId\": false,\n      \"detailsUrl\": \"https://spdx.org/licenses/OPUBL-1.0.json\",\n      \"referenceNumber\": 210,\n      \"name\": \"Open Publication License v1.0\",\n      \"licenseId\": \"OPUBL-1.0\",\n      \"seeAlso\": [\n        \"http://opencontent.org/openpub/\",\n        \"https://www.debian.org/opl\",\n        \"https://www.ctan.org/license/opl\"\n      ],\n      \"isOsiApproved\": false\n    },\n    {\n      \"reference\": \"https://spdx.org/licenses/OSET-PL-2.1.html\",\n      \"isDeprecatedLicenseId\": false,\n      \"detailsUrl\": \"https://spdx.org/licenses/OSET-PL-2.1.json\",\n      \"referenceNumber\": 392,\n      \"name\": \"OSET Public License version 2.1\",\n      \"licenseId\": \"OSET-PL-2.1\",\n      \"seeAlso\": [\n        \"http://www.osetfoundation.org/public-license\",\n        \"https://opensource.org/licenses/OPL-2.1\"\n      ],\n      \"isOsiApproved\": true\n    },\n    {\n      \"reference\": \"https://spdx.org/licenses/OSL-1.0.html\",\n      \"isDeprecatedLicenseId\": false,\n      \"detailsUrl\": \"https://spdx.org/licenses/OSL-1.0.json\",\n      \"referenceNumber\": 619,\n      \"name\": \"Open Software License 1.0\",\n      \"licenseId\": \"OSL-1.0\",\n      \"seeAlso\": [\n        \"https://opensource.org/licenses/OSL-1.0\"\n      ],\n      \"isOsiApproved\": true,\n      \"isFsfLibre\": true\n    },\n    {\n      \"reference\": \"https://spdx.org/licenses/OSL-1.1.html\",\n      \"isDeprecatedLicenseId\": false,\n      \"detailsUrl\": \"https://spdx.org/licenses/OSL-1.1.json\",\n      \"referenceNumber\": 158,\n      \"name\": \"Open Software License 1.1\",\n      \"licenseId\": \"OSL-1.1\",\n      \"seeAlso\": [\n        \"https://fedoraproject.org/wiki/Licensing/OSL1.1\"\n      ],\n      \"isOsiApproved\": false,\n      \"isFsfLibre\": true\n    },\n    {\n      \"reference\": \"https://spdx.org/licenses/OSL-2.0.html\",\n      \"isDeprecatedLicenseId\": false,\n      \"detailsUrl\": \"https://spdx.org/licenses/OSL-2.0.json\",\n      \"referenceNumber\": 77,\n      \"name\": \"Open Software License 2.0\",\n      \"licenseId\": \"OSL-2.0\",\n      \"seeAlso\": [\n        \"http://web.archive.org/web/20041020171434/http://www.rosenlaw.com/osl2.0.html\"\n      ],\n      \"isOsiApproved\": true,\n      \"isFsfLibre\": true\n    },\n    {\n      \"reference\": \"https://spdx.org/licenses/OSL-2.1.html\",\n      \"isDeprecatedLicenseId\": false,\n      \"detailsUrl\": \"https://spdx.org/licenses/OSL-2.1.json\",\n      \"referenceNumber\": 471,\n      \"name\": \"Open Software License 2.1\",\n      \"licenseId\": \"OSL-2.1\",\n      \"seeAlso\": [\n        \"http://web.archive.org/web/20050212003940/http://www.rosenlaw.com/osl21.htm\",\n        \"https://opensource.org/licenses/OSL-2.1\"\n      ],\n      \"isOsiApproved\": true,\n      \"isFsfLibre\": true\n    },\n    {\n      \"reference\": \"https://spdx.org/licenses/OSL-3.0.html\",\n      \"isDeprecatedLicenseId\": false,\n      \"detailsUrl\": \"https://spdx.org/licenses/OSL-3.0.json\",\n      \"referenceNumber\": 231,\n      \"name\": \"Open Software License 3.0\",\n      \"licenseId\": \"OSL-3.0\",\n      \"seeAlso\": [\n        \"https://web.archive.org/web/20120101081418/http://rosenlaw.com:80/OSL3.0.htm\",\n        \"https://opensource.org/licenses/OSL-3.0\"\n      ],\n      \"isOsiApproved\": true,\n      \"isFsfLibre\": true\n    },\n    {\n      \"reference\": \"https://spdx.org/licenses/PADL.html\",\n      \"isDeprecatedLicenseId\": false,\n      \"detailsUrl\": \"https://spdx.org/licenses/PADL.json\",\n      \"referenceNumber\": 477,\n      \"name\": \"PADL License\",\n      \"licenseId\": \"PADL\",\n      \"seeAlso\": [\n        \"https://git.openldap.org/openldap/openldap/-/blob/master/libraries/libldap/os-local.c?ref_type\\u003dheads#L19-23\"\n      ],\n      \"isOsiApproved\": false\n    },\n    {\n      \"reference\": \"https://spdx.org/licenses/Parity-6.0.0.html\",\n      \"isDeprecatedLicenseId\": false,\n      \"detailsUrl\": \"https://spdx.org/licenses/Parity-6.0.0.json\",\n      \"referenceNumber\": 472,\n      \"name\": \"The Parity Public License 6.0.0\",\n      \"licenseId\": \"Parity-6.0.0\",\n      \"seeAlso\": [\n        \"https://paritylicense.com/versions/6.0.0.html\"\n      ],\n      \"isOsiApproved\": false\n    },\n    {\n      \"reference\": \"https://spdx.org/licenses/Parity-7.0.0.html\",\n      \"isDeprecatedLicenseId\": false,\n      \"detailsUrl\": \"https://spdx.org/licenses/Parity-7.0.0.json\",\n      \"referenceNumber\": 68,\n      \"name\": \"The Parity Public License 7.0.0\",\n      \"licenseId\": \"Parity-7.0.0\",\n      \"seeAlso\": [\n        \"https://paritylicense.com/versions/7.0.0.html\"\n      ],\n      \"isOsiApproved\": false\n    },\n    {\n      \"reference\": \"https://spdx.org/licenses/PDDL-1.0.html\",\n      \"isDeprecatedLicenseId\": false,\n      \"detailsUrl\": \"https://spdx.org/licenses/PDDL-1.0.json\",\n      \"referenceNumber\": 474,\n      \"name\": \"Open Data Commons Public Domain Dedication \\u0026 License 1.0\",\n      \"licenseId\": \"PDDL-1.0\",\n      \"seeAlso\": [\n        \"http://opendatacommons.org/licenses/pddl/1.0/\",\n        \"https://opendatacommons.org/licenses/pddl/\"\n      ],\n      \"isOsiApproved\": false\n    },\n    {\n      \"reference\": \"https://spdx.org/licenses/PHP-3.0.html\",\n      \"isDeprecatedLicenseId\": false,\n      \"detailsUrl\": \"https://spdx.org/licenses/PHP-3.0.json\",\n      \"referenceNumber\": 133,\n      \"name\": \"PHP License v3.0\",\n      \"licenseId\": \"PHP-3.0\",\n      \"seeAlso\": [\n        \"http://www.php.net/license/3_0.txt\",\n        \"https://opensource.org/licenses/PHP-3.0\"\n      ],\n      \"isOsiApproved\": true\n    },\n    {\n      \"reference\": \"https://spdx.org/licenses/PHP-3.01.html\",\n      \"isDeprecatedLicenseId\": false,\n      \"detailsUrl\": \"https://spdx.org/licenses/PHP-3.01.json\",\n      \"referenceNumber\": 488,\n      \"name\": \"PHP License v3.01\",\n      \"licenseId\": \"PHP-3.01\",\n      \"seeAlso\": [\n        \"http://www.php.net/license/3_01.txt\"\n      ],\n      \"isOsiApproved\": true,\n      \"isFsfLibre\": true\n    },\n    {\n      \"reference\": \"https://spdx.org/licenses/Pixar.html\",\n      \"isDeprecatedLicenseId\": false,\n      \"detailsUrl\": \"https://spdx.org/licenses/Pixar.json\",\n      \"referenceNumber\": 363,\n      \"name\": \"Pixar License\",\n      \"licenseId\": \"Pixar\",\n      \"seeAlso\": [\n        \"https://github.com/PixarAnimationStudios/OpenSubdiv/raw/v3_5_0/LICENSE.txt\",\n        \"https://graphics.pixar.com/opensubdiv/docs/license.html\",\n        \"https://github.com/PixarAnimationStudios/OpenSubdiv/blob/v3_5_0/opensubdiv/version.cpp#L2-L22\"\n      ],\n      \"isOsiApproved\": false\n    },\n    {\n      \"reference\": \"https://spdx.org/licenses/pkgconf.html\",\n      \"isDeprecatedLicenseId\": false,\n      \"detailsUrl\": \"https://spdx.org/licenses/pkgconf.json\",\n      \"referenceNumber\": 259,\n      \"name\": \"pkgconf License\",\n      \"licenseId\": \"pkgconf\",\n      \"seeAlso\": [\n        \"https://github.com/pkgconf/pkgconf/blob/master/cli/main.c#L8\"\n      ],\n      \"isOsiApproved\": false\n    },\n    {\n      \"reference\": \"https://spdx.org/licenses/Plexus.html\",\n      \"isDeprecatedLicenseId\": false,\n      \"detailsUrl\": \"https://spdx.org/licenses/Plexus.json\",\n      \"referenceNumber\": 309,\n      \"name\": \"Plexus Classworlds License\",\n      \"licenseId\": \"Plexus\",\n      \"seeAlso\": [\n        \"https://fedoraproject.org/wiki/Licensing/Plexus_Classworlds_License\"\n      ],\n      \"isOsiApproved\": false\n    },\n    {\n      \"reference\": \"https://spdx.org/licenses/pnmstitch.html\",\n      \"isDeprecatedLicenseId\": false,\n      \"detailsUrl\": \"https://spdx.org/licenses/pnmstitch.json\",\n      \"referenceNumber\": 626,\n      \"name\": \"pnmstitch License\",\n      \"licenseId\": \"pnmstitch\",\n      \"seeAlso\": [\n        \"https://sourceforge.net/p/netpbm/code/HEAD/tree/super_stable/editor/pnmstitch.c#l2\"\n      ],\n      \"isOsiApproved\": false\n    },\n    {\n      \"reference\": \"https://spdx.org/licenses/PolyForm-Noncommercial-1.0.0.html\",\n      \"isDeprecatedLicenseId\": false,\n      \"detailsUrl\": \"https://spdx.org/licenses/PolyForm-Noncommercial-1.0.0.json\",\n      \"referenceNumber\": 359,\n      \"name\": \"PolyForm Noncommercial License 1.0.0\",\n      \"licenseId\": \"PolyForm-Noncommercial-1.0.0\",\n      \"seeAlso\": [\n        \"https://polyformproject.org/licenses/noncommercial/1.0.0\"\n      ],\n      \"isOsiApproved\": false\n    },\n    {\n      \"reference\": \"https://spdx.org/licenses/PolyForm-Small-Business-1.0.0.html\",\n      \"isDeprecatedLicenseId\": false,\n      \"detailsUrl\": \"https://spdx.org/licenses/PolyForm-Small-Business-1.0.0.json\",\n      \"referenceNumber\": 290,\n      \"name\": \"PolyForm Small Business License 1.0.0\",\n      \"licenseId\": \"PolyForm-Small-Business-1.0.0\",\n      \"seeAlso\": [\n        \"https://polyformproject.org/licenses/small-business/1.0.0\"\n      ],\n      \"isOsiApproved\": false\n    },\n    {\n      \"reference\": \"https://spdx.org/licenses/PostgreSQL.html\",\n      \"isDeprecatedLicenseId\": false,\n      \"detailsUrl\": \"https://spdx.org/licenses/PostgreSQL.json\",\n      \"referenceNumber\": 239,\n      \"name\": \"PostgreSQL License\",\n      \"licenseId\": \"PostgreSQL\",\n      \"seeAlso\": [\n        \"http://www.postgresql.org/about/licence\",\n        \"https://opensource.org/licenses/PostgreSQL\"\n      ],\n      \"isOsiApproved\": true\n    },\n    {\n      \"reference\": \"https://spdx.org/licenses/PPL.html\",\n      \"isDeprecatedLicenseId\": false,\n      \"detailsUrl\": \"https://spdx.org/licenses/PPL.json\",\n      \"referenceNumber\": 614,\n      \"name\": \"Peer Production License\",\n      \"licenseId\": \"PPL\",\n      \"seeAlso\": [\n        \"https://wiki.p2pfoundation.net/Peer_Production_License\",\n        \"http://www.networkcultures.org/_uploads/%233notebook_telekommunist.pdf\"\n      ],\n      \"isOsiApproved\": false,\n      \"isFsfLibre\": false\n    },\n    {\n      \"reference\": \"https://spdx.org/licenses/PSF-2.0.html\",\n      \"isDeprecatedLicenseId\": false,\n      \"detailsUrl\": \"https://spdx.org/licenses/PSF-2.0.json\",\n      \"referenceNumber\": 459,\n      \"name\": \"Python Software Foundation License 2.0\",\n      \"licenseId\": \"PSF-2.0\",\n      \"seeAlso\": [\n        \"https://opensource.org/licenses/Python-2.0\"\n      ],\n      \"isOsiApproved\": false\n    },\n    {\n      \"reference\": \"https://spdx.org/licenses/psfrag.html\",\n      \"isDeprecatedLicenseId\": false,\n      \"detailsUrl\": \"https://spdx.org/licenses/psfrag.json\",\n      \"referenceNumber\": 460,\n      \"name\": \"psfrag License\",\n      \"licenseId\": \"psfrag\",\n      \"seeAlso\": [\n        \"https://fedoraproject.org/wiki/Licensing/psfrag\"\n      ],\n      \"isOsiApproved\": false\n    },\n    {\n      \"reference\": \"https://spdx.org/licenses/psutils.html\",\n      \"isDeprecatedLicenseId\": false,\n      \"detailsUrl\": \"https://spdx.org/licenses/psutils.json\",\n      \"referenceNumber\": 401,\n      \"name\": \"psutils License\",\n      \"licenseId\": \"psutils\",\n      \"seeAlso\": [\n        \"https://fedoraproject.org/wiki/Licensing/psutils\"\n      ],\n      \"isOsiApproved\": false\n    },\n    {\n      \"reference\": \"https://spdx.org/licenses/Python-2.0.html\",\n      \"isDeprecatedLicenseId\": false,\n      \"detailsUrl\": \"https://spdx.org/licenses/Python-2.0.json\",\n      \"referenceNumber\": 261,\n      \"name\": \"Python License 2.0\",\n      \"licenseId\": \"Python-2.0\",\n      \"seeAlso\": [\n        \"https://opensource.org/licenses/Python-2.0\"\n      ],\n      \"isOsiApproved\": true,\n      \"isFsfLibre\": true\n    },\n    {\n      \"reference\": \"https://spdx.org/licenses/Python-2.0.1.html\",\n      \"isDeprecatedLicenseId\": false,\n      \"detailsUrl\": \"https://spdx.org/licenses/Python-2.0.1.json\",\n      \"referenceNumber\": 268,\n      \"name\": \"Python License 2.0.1\",\n      \"licenseId\": \"Python-2.0.1\",\n      \"seeAlso\": [\n        \"https://www.python.org/download/releases/2.0.1/license/\",\n        \"https://docs.python.org/3/license.html\",\n        \"https://github.com/python/cpython/blob/main/LICENSE\"\n      ],\n      \"isOsiApproved\": false\n    },\n    {\n      \"reference\": \"https://spdx.org/licenses/python-ldap.html\",\n      \"isDeprecatedLicenseId\": false,\n      \"detailsUrl\": \"https://spdx.org/licenses/python-ldap.json\",\n      \"referenceNumber\": 302,\n      \"name\": \"Python ldap License\",\n      \"licenseId\": \"python-ldap\",\n      \"seeAlso\": [\n        \"https://github.com/python-ldap/python-ldap/blob/main/LICENCE\"\n      ],\n      \"isOsiApproved\": false\n    },\n    {\n      \"reference\": \"https://spdx.org/licenses/Qhull.html\",\n      \"isDeprecatedLicenseId\": false,\n      \"detailsUrl\": \"https://spdx.org/licenses/Qhull.json\",\n      \"referenceNumber\": 56,\n      \"name\": \"Qhull License\",\n      \"licenseId\": \"Qhull\",\n      \"seeAlso\": [\n        \"https://fedoraproject.org/wiki/Licensing/Qhull\"\n      ],\n      \"isOsiApproved\": false\n    },\n    {\n      \"reference\": \"https://spdx.org/licenses/QPL-1.0.html\",\n      \"isDeprecatedLicenseId\": false,\n      \"detailsUrl\": \"https://spdx.org/licenses/QPL-1.0.json\",\n      \"referenceNumber\": 635,\n      \"name\": \"Q Public License 1.0\",\n      \"licenseId\": \"QPL-1.0\",\n      \"seeAlso\": [\n        \"http://doc.qt.nokia.com/3.3/license.html\",\n        \"https://opensource.org/licenses/QPL-1.0\",\n        \"https://doc.qt.io/archives/3.3/license.html\"\n      ],\n      \"isOsiApproved\": true,\n      \"isFsfLibre\": true\n    },\n    {\n      \"reference\": \"https://spdx.org/licenses/QPL-1.0-INRIA-2004.html\",\n      \"isDeprecatedLicenseId\": false,\n      \"detailsUrl\": \"https://spdx.org/licenses/QPL-1.0-INRIA-2004.json\",\n      \"referenceNumber\": 46,\n      \"name\": \"Q Public License 1.0 - INRIA 2004 variant\",\n      \"licenseId\": \"QPL-1.0-INRIA-2004\",\n      \"seeAlso\": [\n        \"https://github.com/maranget/hevea/blob/master/LICENSE\"\n      ],\n      \"isOsiApproved\": false\n    },\n    {\n      \"reference\": \"https://spdx.org/licenses/radvd.html\",\n      \"isDeprecatedLicenseId\": false,\n      \"detailsUrl\": \"https://spdx.org/licenses/radvd.json\",\n      \"referenceNumber\": 195,\n      \"name\": \"radvd License\",\n      \"licenseId\": \"radvd\",\n      \"seeAlso\": [\n        \"https://github.com/radvd-project/radvd/blob/master/COPYRIGHT\"\n      ],\n      \"isOsiApproved\": false\n    },\n    {\n      \"reference\": \"https://spdx.org/licenses/Rdisc.html\",\n      \"isDeprecatedLicenseId\": false,\n      \"detailsUrl\": \"https://spdx.org/licenses/Rdisc.json\",\n      \"referenceNumber\": 408,\n      \"name\": \"Rdisc License\",\n      \"licenseId\": \"Rdisc\",\n      \"seeAlso\": [\n        \"https://fedoraproject.org/wiki/Licensing/Rdisc_License\"\n      ],\n      \"isOsiApproved\": false\n    },\n    {\n      \"reference\": \"https://spdx.org/licenses/RHeCos-1.1.html\",\n      \"isDeprecatedLicenseId\": false,\n      \"detailsUrl\": \"https://spdx.org/licenses/RHeCos-1.1.json\",\n      \"referenceNumber\": 539,\n      \"name\": \"Red Hat eCos Public License v1.1\",\n      \"licenseId\": \"RHeCos-1.1\",\n      \"seeAlso\": [\n        \"http://ecos.sourceware.org/old-license.html\"\n      ],\n      \"isOsiApproved\": false,\n      \"isFsfLibre\": false\n    },\n    {\n      \"reference\": \"https://spdx.org/licenses/RPL-1.1.html\",\n      \"isDeprecatedLicenseId\": false,\n      \"detailsUrl\": \"https://spdx.org/licenses/RPL-1.1.json\",\n      \"referenceNumber\": 255,\n      \"name\": \"Reciprocal Public License 1.1\",\n      \"licenseId\": \"RPL-1.1\",\n      \"seeAlso\": [\n        \"https://opensource.org/licenses/RPL-1.1\"\n      ],\n      \"isOsiApproved\": true\n    },\n    {\n      \"reference\": \"https://spdx.org/licenses/RPL-1.5.html\",\n      \"isDeprecatedLicenseId\": false,\n      \"detailsUrl\": \"https://spdx.org/licenses/RPL-1.5.json\",\n      \"referenceNumber\": 436,\n      \"name\": \"Reciprocal Public License 1.5\",\n      \"licenseId\": \"RPL-1.5\",\n      \"seeAlso\": [\n        \"https://opensource.org/licenses/RPL-1.5\"\n      ],\n      \"isOsiApproved\": true\n    },\n    {\n      \"reference\": \"https://spdx.org/licenses/RPSL-1.0.html\",\n      \"isDeprecatedLicenseId\": false,\n      \"detailsUrl\": \"https://spdx.org/licenses/RPSL-1.0.json\",\n      \"referenceNumber\": 341,\n      \"name\": \"RealNetworks Public Source License v1.0\",\n      \"licenseId\": \"RPSL-1.0\",\n      \"seeAlso\": [\n        \"https://helixcommunity.org/content/rpsl\",\n        \"https://opensource.org/licenses/RPSL-1.0\"\n      ],\n      \"isOsiApproved\": true,\n      \"isFsfLibre\": true\n    },\n    {\n      \"reference\": \"https://spdx.org/licenses/RSA-MD.html\",\n      \"isDeprecatedLicenseId\": false,\n      \"detailsUrl\": \"https://spdx.org/licenses/RSA-MD.json\",\n      \"referenceNumber\": 314,\n      \"name\": \"RSA Message-Digest License\",\n      \"licenseId\": \"RSA-MD\",\n      \"seeAlso\": [\n        \"http://www.faqs.org/rfcs/rfc1321.html\"\n      ],\n      \"isOsiApproved\": false\n    },\n    {\n      \"reference\": \"https://spdx.org/licenses/RSCPL.html\",\n      \"isDeprecatedLicenseId\": false,\n      \"detailsUrl\": \"https://spdx.org/licenses/RSCPL.json\",\n      \"referenceNumber\": 553,\n      \"name\": \"Ricoh Source Code Public License\",\n      \"licenseId\": \"RSCPL\",\n      \"seeAlso\": [\n        \"http://wayback.archive.org/web/20060715140826/http://www.risource.org/RPL/RPL-1.0A.shtml\",\n        \"https://opensource.org/licenses/RSCPL\"\n      ],\n      \"isOsiApproved\": true\n    },\n    {\n      \"reference\": \"https://spdx.org/licenses/Ruby.html\",\n      \"isDeprecatedLicenseId\": false,\n      \"detailsUrl\": \"https://spdx.org/licenses/Ruby.json\",\n      \"referenceNumber\": 35,\n      \"name\": \"Ruby License\",\n      \"licenseId\": \"Ruby\",\n      \"seeAlso\": [\n        \"https://www.ruby-lang.org/en/about/license.txt\"\n      ],\n      \"isOsiApproved\": false,\n      \"isFsfLibre\": true\n    },\n    {\n      \"reference\": \"https://spdx.org/licenses/SAX-PD.html\",\n      \"isDeprecatedLicenseId\": false,\n      \"detailsUrl\": \"https://spdx.org/licenses/SAX-PD.json\",\n      \"referenceNumber\": 329,\n      \"name\": \"Sax Public Domain Notice\",\n      \"licenseId\": \"SAX-PD\",\n      \"seeAlso\": [\n        \"http://www.saxproject.org/copying.html\"\n      ],\n      \"isOsiApproved\": false\n    },\n    {\n      \"reference\": \"https://spdx.org/licenses/SAX-PD-2.0.html\",\n      \"isDeprecatedLicenseId\": false,\n      \"detailsUrl\": \"https://spdx.org/licenses/SAX-PD-2.0.json\",\n      \"referenceNumber\": 188,\n      \"name\": \"Sax Public Domain Notice 2.0\",\n      \"licenseId\": \"SAX-PD-2.0\",\n      \"seeAlso\": [\n        \"http://www.saxproject.org/copying.html\"\n      ],\n      \"isOsiApproved\": false\n    },\n    {\n      \"reference\": \"https://spdx.org/licenses/Saxpath.html\",\n      \"isDeprecatedLicenseId\": false,\n      \"detailsUrl\": \"https://spdx.org/licenses/Saxpath.json\",\n      \"referenceNumber\": 487,\n      \"name\": \"Saxpath License\",\n      \"licenseId\": \"Saxpath\",\n      \"seeAlso\": [\n        \"https://fedoraproject.org/wiki/Licensing/Saxpath_License\"\n      ],\n      \"isOsiApproved\": false\n    },\n    {\n      \"reference\": \"https://spdx.org/licenses/SCEA.html\",\n      \"isDeprecatedLicenseId\": false,\n      \"detailsUrl\": \"https://spdx.org/licenses/SCEA.json\",\n      \"referenceNumber\": 187,\n      \"name\": \"SCEA Shared Source License\",\n      \"licenseId\": \"SCEA\",\n      \"seeAlso\": [\n        \"http://research.scea.com/scea_shared_source_license.html\"\n      ],\n      \"isOsiApproved\": false\n    },\n    {\n      \"reference\": \"https://spdx.org/licenses/SchemeReport.html\",\n      \"isDeprecatedLicenseId\": false,\n      \"detailsUrl\": \"https://spdx.org/licenses/SchemeReport.json\",\n      \"referenceNumber\": 189,\n      \"name\": \"Scheme Language Report License\",\n      \"licenseId\": \"SchemeReport\",\n      \"seeAlso\": [],\n      \"isOsiApproved\": false\n    },\n    {\n      \"reference\": \"https://spdx.org/licenses/Sendmail.html\",\n      \"isDeprecatedLicenseId\": false,\n      \"detailsUrl\": \"https://spdx.org/licenses/Sendmail.json\",\n      \"referenceNumber\": 586,\n      \"name\": \"Sendmail License\",\n      \"licenseId\": \"Sendmail\",\n      \"seeAlso\": [\n        \"http://www.sendmail.com/pdfs/open_source/sendmail_license.pdf\",\n        \"https://web.archive.org/web/20160322142305/https://www.sendmail.com/pdfs/open_source/sendmail_license.pdf\"\n      ],\n      \"isOsiApproved\": false\n    },\n    {\n      \"reference\": \"https://spdx.org/licenses/Sendmail-8.23.html\",\n      \"isDeprecatedLicenseId\": false,\n      \"detailsUrl\": \"https://spdx.org/licenses/Sendmail-8.23.json\",\n      \"referenceNumber\": 502,\n      \"name\": \"Sendmail License 8.23\",\n      \"licenseId\": \"Sendmail-8.23\",\n      \"seeAlso\": [\n        \"https://www.proofpoint.com/sites/default/files/sendmail-license.pdf\",\n        \"https://web.archive.org/web/20181003101040/https://www.proofpoint.com/sites/default/files/sendmail-license.pdf\"\n      ],\n      \"isOsiApproved\": false\n    },\n    {\n      \"reference\": \"https://spdx.org/licenses/SGI-B-1.0.html\",\n      \"isDeprecatedLicenseId\": false,\n      \"detailsUrl\": \"https://spdx.org/licenses/SGI-B-1.0.json\",\n      \"referenceNumber\": 296,\n      \"name\": \"SGI Free Software License B v1.0\",\n      \"licenseId\": \"SGI-B-1.0\",\n      \"seeAlso\": [\n        \"http://oss.sgi.com/projects/FreeB/SGIFreeSWLicB.1.0.html\"\n      ],\n      \"isOsiApproved\": false\n    },\n    {\n      \"reference\": \"https://spdx.org/licenses/SGI-B-1.1.html\",\n      \"isDeprecatedLicenseId\": false,\n      \"detailsUrl\": \"https://spdx.org/licenses/SGI-B-1.1.json\",\n      \"referenceNumber\": 312,\n      \"name\": \"SGI Free Software License B v1.1\",\n      \"licenseId\": \"SGI-B-1.1\",\n      \"seeAlso\": [\n        \"http://oss.sgi.com/projects/FreeB/\"\n      ],\n      \"isOsiApproved\": false\n    },\n    {\n      \"reference\": \"https://spdx.org/licenses/SGI-B-2.0.html\",\n      \"isDeprecatedLicenseId\": false,\n      \"detailsUrl\": \"https://spdx.org/licenses/SGI-B-2.0.json\",\n      \"referenceNumber\": 33,\n      \"name\": \"SGI Free Software License B v2.0\",\n      \"licenseId\": \"SGI-B-2.0\",\n      \"seeAlso\": [\n        \"http://oss.sgi.com/projects/FreeB/SGIFreeSWLicB.2.0.pdf\"\n      ],\n      \"isOsiApproved\": false,\n      \"isFsfLibre\": true\n    },\n    {\n      \"reference\": \"https://spdx.org/licenses/SGI-OpenGL.html\",\n      \"isDeprecatedLicenseId\": false,\n      \"detailsUrl\": \"https://spdx.org/licenses/SGI-OpenGL.json\",\n      \"referenceNumber\": 333,\n      \"name\": \"SGI OpenGL License\",\n      \"licenseId\": \"SGI-OpenGL\",\n      \"seeAlso\": [\n        \"https://gitlab.freedesktop.org/mesa/glw/-/blob/master/README?ref_type\\u003dheads\"\n      ],\n      \"isOsiApproved\": false\n    },\n    {\n      \"reference\": \"https://spdx.org/licenses/SGP4.html\",\n      \"isDeprecatedLicenseId\": false,\n      \"detailsUrl\": \"https://spdx.org/licenses/SGP4.json\",\n      \"referenceNumber\": 49,\n      \"name\": \"SGP4 Permission Notice\",\n      \"licenseId\": \"SGP4\",\n      \"seeAlso\": [\n        \"https://celestrak.org/publications/AIAA/2006-6753/faq.php\"\n      ],\n      \"isOsiApproved\": false\n    },\n    {\n      \"reference\": \"https://spdx.org/licenses/SHL-0.5.html\",\n      \"isDeprecatedLicenseId\": false,\n      \"detailsUrl\": \"https://spdx.org/licenses/SHL-0.5.json\",\n      \"referenceNumber\": 227,\n      \"name\": \"Solderpad Hardware License v0.5\",\n      \"licenseId\": \"SHL-0.5\",\n      \"seeAlso\": [\n        \"https://solderpad.org/licenses/SHL-0.5/\"\n      ],\n      \"isOsiApproved\": false\n    },\n    {\n      \"reference\": \"https://spdx.org/licenses/SHL-0.51.html\",\n      \"isDeprecatedLicenseId\": false,\n      \"detailsUrl\": \"https://spdx.org/licenses/SHL-0.51.json\",\n      \"referenceNumber\": 348,\n      \"name\": \"Solderpad Hardware License, Version 0.51\",\n      \"licenseId\": \"SHL-0.51\",\n      \"seeAlso\": [\n        \"https://solderpad.org/licenses/SHL-0.51/\"\n      ],\n      \"isOsiApproved\": false\n    },\n    {\n      \"reference\": \"https://spdx.org/licenses/SimPL-2.0.html\",\n      \"isDeprecatedLicenseId\": false,\n      \"detailsUrl\": \"https://spdx.org/licenses/SimPL-2.0.json\",\n      \"referenceNumber\": 161,\n      \"name\": \"Simple Public License 2.0\",\n      \"licenseId\": \"SimPL-2.0\",\n      \"seeAlso\": [\n        \"https://opensource.org/licenses/SimPL-2.0\"\n      ],\n      \"isOsiApproved\": true\n    },\n    {\n      \"reference\": \"https://spdx.org/licenses/SISSL.html\",\n      \"isDeprecatedLicenseId\": false,\n      \"detailsUrl\": \"https://spdx.org/licenses/SISSL.json\",\n      \"referenceNumber\": 650,\n      \"name\": \"Sun Industry Standards Source License v1.1\",\n      \"licenseId\": \"SISSL\",\n      \"seeAlso\": [\n        \"http://www.openoffice.org/licenses/sissl_license.html\",\n        \"https://opensource.org/licenses/SISSL\"\n      ],\n      \"isOsiApproved\": true,\n      \"isFsfLibre\": true\n    },\n    {\n      \"reference\": \"https://spdx.org/licenses/SISSL-1.2.html\",\n      \"isDeprecatedLicenseId\": false,\n      \"detailsUrl\": \"https://spdx.org/licenses/SISSL-1.2.json\",\n      \"referenceNumber\": 112,\n      \"name\": \"Sun Industry Standards Source License v1.2\",\n      \"licenseId\": \"SISSL-1.2\",\n      \"seeAlso\": [\n        \"http://gridscheduler.sourceforge.net/Gridengine_SISSL_license.html\"\n      ],\n      \"isOsiApproved\": false\n    },\n    {\n      \"reference\": \"https://spdx.org/licenses/SL.html\",\n      \"isDeprecatedLicenseId\": false,\n      \"detailsUrl\": \"https://spdx.org/licenses/SL.json\",\n      \"referenceNumber\": 628,\n      \"name\": \"SL License\",\n      \"licenseId\": \"SL\",\n      \"seeAlso\": [\n        \"https://github.com/mtoyoda/sl/blob/master/LICENSE\"\n      ],\n      \"isOsiApproved\": false\n    },\n    {\n      \"reference\": \"https://spdx.org/licenses/Sleepycat.html\",\n      \"isDeprecatedLicenseId\": false,\n      \"detailsUrl\": \"https://spdx.org/licenses/Sleepycat.json\",\n      \"referenceNumber\": 527,\n      \"name\": \"Sleepycat License\",\n      \"licenseId\": \"Sleepycat\",\n      \"seeAlso\": [\n        \"https://opensource.org/licenses/Sleepycat\"\n      ],\n      \"isOsiApproved\": true,\n      \"isFsfLibre\": true\n    },\n    {\n      \"reference\": \"https://spdx.org/licenses/SMLNJ.html\",\n      \"isDeprecatedLicenseId\": false,\n      \"detailsUrl\": \"https://spdx.org/licenses/SMLNJ.json\",\n      \"referenceNumber\": 0,\n      \"name\": \"Standard ML of New Jersey License\",\n      \"licenseId\": \"SMLNJ\",\n      \"seeAlso\": [\n        \"https://www.smlnj.org/license.html\"\n      ],\n      \"isOsiApproved\": false,\n      \"isFsfLibre\": true\n    },\n    {\n      \"reference\": \"https://spdx.org/licenses/SMPPL.html\",\n      \"isDeprecatedLicenseId\": false,\n      \"detailsUrl\": \"https://spdx.org/licenses/SMPPL.json\",\n      \"referenceNumber\": 32,\n      \"name\": \"Secure Messaging Protocol Public License\",\n      \"licenseId\": \"SMPPL\",\n      \"seeAlso\": [\n        \"https://github.com/dcblake/SMP/blob/master/Documentation/License.txt\"\n      ],\n      \"isOsiApproved\": false\n    },\n    {\n      \"reference\": \"https://spdx.org/licenses/SNIA.html\",\n      \"isDeprecatedLicenseId\": false,\n      \"detailsUrl\": \"https://spdx.org/licenses/SNIA.json\",\n      \"referenceNumber\": 163,\n      \"name\": \"SNIA Public License 1.1\",\n      \"licenseId\": \"SNIA\",\n      \"seeAlso\": [\n        \"https://fedoraproject.org/wiki/Licensing/SNIA_Public_License\"\n      ],\n      \"isOsiApproved\": false\n    },\n    {\n      \"reference\": \"https://spdx.org/licenses/snprintf.html\",\n      \"isDeprecatedLicenseId\": false,\n      \"detailsUrl\": \"https://spdx.org/licenses/snprintf.json\",\n      \"referenceNumber\": 218,\n      \"name\": \"snprintf License\",\n      \"licenseId\": \"snprintf\",\n      \"seeAlso\": [\n        \"https://github.com/openssh/openssh-portable/blob/master/openbsd-compat/bsd-snprintf.c#L2\"\n      ],\n      \"isOsiApproved\": false\n    },\n    {\n      \"reference\": \"https://spdx.org/licenses/softSurfer.html\",\n      \"isDeprecatedLicenseId\": false,\n      \"detailsUrl\": \"https://spdx.org/licenses/softSurfer.json\",\n      \"referenceNumber\": 583,\n      \"name\": \"softSurfer License\",\n      \"licenseId\": \"softSurfer\",\n      \"seeAlso\": [\n        \"https://github.com/mm2/Little-CMS/blob/master/src/cmssm.c#L207\",\n        \"https://fedoraproject.org/wiki/Licensing/softSurfer\"\n      ],\n      \"isOsiApproved\": false\n    },\n    {\n      \"reference\": \"https://spdx.org/licenses/Soundex.html\",\n      \"isDeprecatedLicenseId\": false,\n      \"detailsUrl\": \"https://spdx.org/licenses/Soundex.json\",\n      \"referenceNumber\": 145,\n      \"name\": \"Soundex License\",\n      \"licenseId\": \"Soundex\",\n      \"seeAlso\": [\n        \"https://metacpan.org/release/RJBS/Text-Soundex-3.05/source/Soundex.pm#L3-11\"\n      ],\n      \"isOsiApproved\": false\n    },\n    {\n      \"reference\": \"https://spdx.org/licenses/Spencer-86.html\",\n      \"isDeprecatedLicenseId\": false,\n      \"detailsUrl\": \"https://spdx.org/licenses/Spencer-86.json\",\n      \"referenceNumber\": 83,\n      \"name\": \"Spencer License 86\",\n      \"licenseId\": \"Spencer-86\",\n      \"seeAlso\": [\n        \"https://fedoraproject.org/wiki/Licensing/Henry_Spencer_Reg-Ex_Library_License\"\n      ],\n      \"isOsiApproved\": false\n    },\n    {\n      \"reference\": \"https://spdx.org/licenses/Spencer-94.html\",\n      \"isDeprecatedLicenseId\": false,\n      \"detailsUrl\": \"https://spdx.org/licenses/Spencer-94.json\",\n      \"referenceNumber\": 330,\n      \"name\": \"Spencer License 94\",\n      \"licenseId\": \"Spencer-94\",\n      \"seeAlso\": [\n        \"https://fedoraproject.org/wiki/Licensing/Henry_Spencer_Reg-Ex_Library_License\",\n        \"https://metacpan.org/release/KNOK/File-MMagic-1.30/source/COPYING#L28\"\n      ],\n      \"isOsiApproved\": false\n    },\n    {\n      \"reference\": \"https://spdx.org/licenses/Spencer-99.html\",\n      \"isDeprecatedLicenseId\": false,\n      \"detailsUrl\": \"https://spdx.org/licenses/Spencer-99.json\",\n      \"referenceNumber\": 496,\n      \"name\": \"Spencer License 99\",\n      \"licenseId\": \"Spencer-99\",\n      \"seeAlso\": [\n        \"http://www.opensource.apple.com/source/tcl/tcl-5/tcl/generic/regfronts.c\"\n      ],\n      \"isOsiApproved\": false\n    },\n    {\n      \"reference\": \"https://spdx.org/licenses/SPL-1.0.html\",\n      \"isDeprecatedLicenseId\": false,\n      \"detailsUrl\": \"https://spdx.org/licenses/SPL-1.0.json\",\n      \"referenceNumber\": 351,\n      \"name\": \"Sun Public License v1.0\",\n      \"licenseId\": \"SPL-1.0\",\n      \"seeAlso\": [\n        \"https://opensource.org/licenses/SPL-1.0\"\n      ],\n      \"isOsiApproved\": true,\n      \"isFsfLibre\": true\n    },\n    {\n      \"reference\": \"https://spdx.org/licenses/ssh-keyscan.html\",\n      \"isDeprecatedLicenseId\": false,\n      \"detailsUrl\": \"https://spdx.org/licenses/ssh-keyscan.json\",\n      \"referenceNumber\": 220,\n      \"name\": \"ssh-keyscan License\",\n      \"licenseId\": \"ssh-keyscan\",\n      \"seeAlso\": [\n        \"https://github.com/openssh/openssh-portable/blob/master/LICENCE#L82\"\n      ],\n      \"isOsiApproved\": false\n    },\n    {\n      \"reference\": \"https://spdx.org/licenses/SSH-OpenSSH.html\",\n      \"isDeprecatedLicenseId\": false,\n      \"detailsUrl\": \"https://spdx.org/licenses/SSH-OpenSSH.json\",\n      \"referenceNumber\": 88,\n      \"name\": \"SSH OpenSSH license\",\n      \"licenseId\": \"SSH-OpenSSH\",\n      \"seeAlso\": [\n        \"https://github.com/openssh/openssh-portable/blob/1b11ea7c58cd5c59838b5fa574cd456d6047b2d4/LICENCE#L10\"\n      ],\n      \"isOsiApproved\": false\n    },\n    {\n      \"reference\": \"https://spdx.org/licenses/SSH-short.html\",\n      \"isDeprecatedLicenseId\": false,\n      \"detailsUrl\": \"https://spdx.org/licenses/SSH-short.json\",\n      \"referenceNumber\": 498,\n      \"name\": \"SSH short notice\",\n      \"licenseId\": \"SSH-short\",\n      \"seeAlso\": [\n        \"https://github.com/openssh/openssh-portable/blob/1b11ea7c58cd5c59838b5fa574cd456d6047b2d4/pathnames.h\",\n        \"http://web.mit.edu/kolya/.f/root/athena.mit.edu/sipb.mit.edu/project/openssh/OldFiles/src/openssh-2.9.9p2/ssh-add.1\",\n        \"https://joinup.ec.europa.eu/svn/lesoll/trunk/italc/lib/src/dsa_key.cpp\"\n      ],\n      \"isOsiApproved\": false\n    },\n    {\n      \"reference\": \"https://spdx.org/licenses/SSLeay-standalone.html\",\n      \"isDeprecatedLicenseId\": false,\n      \"detailsUrl\": \"https://spdx.org/licenses/SSLeay-standalone.json\",\n      \"referenceNumber\": 238,\n      \"name\": \"SSLeay License - standalone\",\n      \"licenseId\": \"SSLeay-standalone\",\n      \"seeAlso\": [\n        \"https://www.tq-group.com/filedownloads/files/software-license-conditions/OriginalSSLeay/OriginalSSLeay.pdf\"\n      ],\n      \"isOsiApproved\": false\n    },\n    {\n      \"reference\": \"https://spdx.org/licenses/SSPL-1.0.html\",\n      \"isDeprecatedLicenseId\": false,\n      \"detailsUrl\": \"https://spdx.org/licenses/SSPL-1.0.json\",\n      \"referenceNumber\": 16,\n      \"name\": \"Server Side Public License, v 1\",\n      \"licenseId\": \"SSPL-1.0\",\n      \"seeAlso\": [\n        \"https://www.mongodb.com/licensing/server-side-public-license\"\n      ],\n      \"isOsiApproved\": false\n    },\n    {\n      \"reference\": \"https://spdx.org/licenses/StandardML-NJ.html\",\n      \"isDeprecatedLicenseId\": true,\n      \"detailsUrl\": \"https://spdx.org/licenses/StandardML-NJ.json\",\n      \"referenceNumber\": 214,\n      \"name\": \"Standard ML of New Jersey License\",\n      \"licenseId\": \"StandardML-NJ\",\n      \"seeAlso\": [\n        \"https://www.smlnj.org/license.html\"\n      ],\n      \"isOsiApproved\": false,\n      \"isFsfLibre\": true\n    },\n    {\n      \"reference\": \"https://spdx.org/licenses/SugarCRM-1.1.3.html\",\n      \"isDeprecatedLicenseId\": false,\n      \"detailsUrl\": \"https://spdx.org/licenses/SugarCRM-1.1.3.json\",\n      \"referenceNumber\": 379,\n      \"name\": \"SugarCRM Public License v1.1.3\",\n      \"licenseId\": \"SugarCRM-1.1.3\",\n      \"seeAlso\": [\n        \"http://www.sugarcrm.com/crm/SPL\"\n      ],\n      \"isOsiApproved\": false\n    },\n    {\n      \"reference\": \"https://spdx.org/licenses/Sun-PPP.html\",\n      \"isDeprecatedLicenseId\": false,\n      \"detailsUrl\": \"https://spdx.org/licenses/Sun-PPP.json\",\n      \"referenceNumber\": 434,\n      \"name\": \"Sun PPP License\",\n      \"licenseId\": \"Sun-PPP\",\n      \"seeAlso\": [\n        \"https://github.com/ppp-project/ppp/blob/master/pppd/eap.c#L7-L16\"\n      ],\n      \"isOsiApproved\": false\n    },\n    {\n      \"reference\": \"https://spdx.org/licenses/Sun-PPP-2000.html\",\n      \"isDeprecatedLicenseId\": false,\n      \"detailsUrl\": \"https://spdx.org/licenses/Sun-PPP-2000.json\",\n      \"referenceNumber\": 12,\n      \"name\": \"Sun PPP License (2000)\",\n      \"licenseId\": \"Sun-PPP-2000\",\n      \"seeAlso\": [\n        \"https://github.com/ppp-project/ppp/blob/master/modules/ppp_ahdlc.c#L7-L19\"\n      ],\n      \"isOsiApproved\": false\n    },\n    {\n      \"reference\": \"https://spdx.org/licenses/SunPro.html\",\n      \"isDeprecatedLicenseId\": false,\n      \"detailsUrl\": \"https://spdx.org/licenses/SunPro.json\",\n      \"referenceNumber\": 315,\n      \"name\": \"SunPro License\",\n      \"licenseId\": \"SunPro\",\n      \"seeAlso\": [\n        \"https://github.com/freebsd/freebsd-src/blob/main/lib/msun/src/e_acosh.c\",\n        \"https://github.com/freebsd/freebsd-src/blob/main/lib/msun/src/e_lgammal.c\"\n      ],\n      \"isOsiApproved\": false\n    },\n    {\n      \"reference\": \"https://spdx.org/licenses/SWL.html\",\n      \"isDeprecatedLicenseId\": false,\n      \"detailsUrl\": \"https://spdx.org/licenses/SWL.json\",\n      \"referenceNumber\": 609,\n      \"name\": \"Scheme Widget Library (SWL) Software License Agreement\",\n      \"licenseId\": \"SWL\",\n      \"seeAlso\": [\n        \"https://fedoraproject.org/wiki/Licensing/SWL\"\n      ],\n      \"isOsiApproved\": false\n    },\n    {\n      \"reference\": \"https://spdx.org/licenses/swrule.html\",\n      \"isDeprecatedLicenseId\": false,\n      \"detailsUrl\": \"https://spdx.org/licenses/swrule.json\",\n      \"referenceNumber\": 31,\n      \"name\": \"swrule License\",\n      \"licenseId\": \"swrule\",\n      \"seeAlso\": [\n        \"https://ctan.math.utah.edu/ctan/tex-archive/macros/generic/misc/swrule.sty\"\n      ],\n      \"isOsiApproved\": false\n    },\n    {\n      \"reference\": \"https://spdx.org/licenses/Symlinks.html\",\n      \"isDeprecatedLicenseId\": false,\n      \"detailsUrl\": \"https://spdx.org/licenses/Symlinks.json\",\n      \"referenceNumber\": 212,\n      \"name\": \"Symlinks License\",\n      \"licenseId\": \"Symlinks\",\n      \"seeAlso\": [\n        \"https://www.mail-archive.com/debian-bugs-rc@lists.debian.org/msg11494.html\"\n      ],\n      \"isOsiApproved\": false\n    },\n    {\n      \"reference\": \"https://spdx.org/licenses/TAPR-OHL-1.0.html\",\n      \"isDeprecatedLicenseId\": false,\n      \"detailsUrl\": \"https://spdx.org/licenses/TAPR-OHL-1.0.json\",\n      \"referenceNumber\": 622,\n      \"name\": \"TAPR Open Hardware License v1.0\",\n      \"licenseId\": \"TAPR-OHL-1.0\",\n      \"seeAlso\": [\n        \"https://www.tapr.org/OHL\"\n      ],\n      \"isOsiApproved\": false\n    },\n    {\n      \"reference\": \"https://spdx.org/licenses/TCL.html\",\n      \"isDeprecatedLicenseId\": false,\n      \"detailsUrl\": \"https://spdx.org/licenses/TCL.json\",\n      \"referenceNumber\": 353,\n      \"name\": \"TCL/TK License\",\n      \"licenseId\": \"TCL\",\n      \"seeAlso\": [\n        \"http://www.tcl.tk/software/tcltk/license.html\",\n        \"https://fedoraproject.org/wiki/Licensing/TCL\"\n      ],\n      \"isOsiApproved\": false\n    },\n    {\n      \"reference\": \"https://spdx.org/licenses/TCP-wrappers.html\",\n      \"isDeprecatedLicenseId\": false,\n      \"detailsUrl\": \"https://spdx.org/licenses/TCP-wrappers.json\",\n      \"referenceNumber\": 617,\n      \"name\": \"TCP Wrappers License\",\n      \"licenseId\": \"TCP-wrappers\",\n      \"seeAlso\": [\n        \"http://rc.quest.com/topics/openssh/license.php#tcpwrappers\"\n      ],\n      \"isOsiApproved\": false\n    },\n    {\n      \"reference\": \"https://spdx.org/licenses/TermReadKey.html\",\n      \"isDeprecatedLicenseId\": false,\n      \"detailsUrl\": \"https://spdx.org/licenses/TermReadKey.json\",\n      \"referenceNumber\": 246,\n      \"name\": \"TermReadKey License\",\n      \"licenseId\": \"TermReadKey\",\n      \"seeAlso\": [\n        \"https://github.com/jonathanstowe/TermReadKey/blob/master/README#L9-L10\"\n      ],\n      \"isOsiApproved\": false\n    },\n    {\n      \"reference\": \"https://spdx.org/licenses/TGPPL-1.0.html\",\n      \"isDeprecatedLicenseId\": false,\n      \"detailsUrl\": \"https://spdx.org/licenses/TGPPL-1.0.json\",\n      \"referenceNumber\": 219,\n      \"name\": \"Transitive Grace Period Public Licence 1.0\",\n      \"licenseId\": \"TGPPL-1.0\",\n      \"seeAlso\": [\n        \"https://fedoraproject.org/wiki/Licensing/TGPPL\",\n        \"https://tahoe-lafs.org/trac/tahoe-lafs/browser/trunk/COPYING.TGPPL.rst\"\n      ],\n      \"isOsiApproved\": false\n    },\n    {\n      \"reference\": \"https://spdx.org/licenses/threeparttable.html\",\n      \"isDeprecatedLicenseId\": false,\n      \"detailsUrl\": \"https://spdx.org/licenses/threeparttable.json\",\n      \"referenceNumber\": 311,\n      \"name\": \"threeparttable License\",\n      \"licenseId\": \"threeparttable\",\n      \"seeAlso\": [\n        \"https://fedoraproject.org/wiki/Licensing/Threeparttable\"\n      ],\n      \"isOsiApproved\": false\n    },\n    {\n      \"reference\": \"https://spdx.org/licenses/TMate.html\",\n      \"isDeprecatedLicenseId\": false,\n      \"detailsUrl\": \"https://spdx.org/licenses/TMate.json\",\n      \"referenceNumber\": 60,\n      \"name\": \"TMate Open Source License\",\n      \"licenseId\": \"TMate\",\n      \"seeAlso\": [\n        \"http://svnkit.com/license.html\"\n      ],\n      \"isOsiApproved\": false\n    },\n    {\n      \"reference\": \"https://spdx.org/licenses/TORQUE-1.1.html\",\n      \"isDeprecatedLicenseId\": false,\n      \"detailsUrl\": \"https://spdx.org/licenses/TORQUE-1.1.json\",\n      \"referenceNumber\": 40,\n      \"name\": \"TORQUE v2.5+ Software License v1.1\",\n      \"licenseId\": \"TORQUE-1.1\",\n      \"seeAlso\": [\n        \"https://fedoraproject.org/wiki/Licensing/TORQUEv1.1\"\n      ],\n      \"isOsiApproved\": false\n    },\n    {\n      \"reference\": \"https://spdx.org/licenses/TOSL.html\",\n      \"isDeprecatedLicenseId\": false,\n      \"detailsUrl\": \"https://spdx.org/licenses/TOSL.json\",\n      \"referenceNumber\": 423,\n      \"name\": \"Trusster Open Source License\",\n      \"licenseId\": \"TOSL\",\n      \"seeAlso\": [\n        \"https://fedoraproject.org/wiki/Licensing/TOSL\"\n      ],\n      \"isOsiApproved\": false\n    },\n    {\n      \"reference\": \"https://spdx.org/licenses/TPDL.html\",\n      \"isDeprecatedLicenseId\": false,\n      \"detailsUrl\": \"https://spdx.org/licenses/TPDL.json\",\n      \"referenceNumber\": 356,\n      \"name\": \"Time::ParseDate License\",\n      \"licenseId\": \"TPDL\",\n      \"seeAlso\": [\n        \"https://metacpan.org/pod/Time::ParseDate#LICENSE\"\n      ],\n      \"isOsiApproved\": false\n    },\n    {\n      \"reference\": \"https://spdx.org/licenses/TPL-1.0.html\",\n      \"isDeprecatedLicenseId\": false,\n      \"detailsUrl\": \"https://spdx.org/licenses/TPL-1.0.json\",\n      \"referenceNumber\": 377,\n      \"name\": \"THOR Public License 1.0\",\n      \"licenseId\": \"TPL-1.0\",\n      \"seeAlso\": [\n        \"https://fedoraproject.org/wiki/Licensing:ThorPublicLicense\"\n      ],\n      \"isOsiApproved\": false\n    },\n    {\n      \"reference\": \"https://spdx.org/licenses/TTWL.html\",\n      \"isDeprecatedLicenseId\": false,\n      \"detailsUrl\": \"https://spdx.org/licenses/TTWL.json\",\n      \"referenceNumber\": 343,\n      \"name\": \"Text-Tabs+Wrap License\",\n      \"licenseId\": \"TTWL\",\n      \"seeAlso\": [\n        \"https://fedoraproject.org/wiki/Licensing/TTWL\",\n        \"https://github.com/ap/Text-Tabs/blob/master/lib.modern/Text/Tabs.pm#L148\"\n      ],\n      \"isOsiApproved\": false\n    },\n    {\n      \"reference\": \"https://spdx.org/licenses/TTYP0.html\",\n      \"isDeprecatedLicenseId\": false,\n      \"detailsUrl\": \"https://spdx.org/licenses/TTYP0.json\",\n      \"referenceNumber\": 540,\n      \"name\": \"TTYP0 License\",\n      \"licenseId\": \"TTYP0\",\n      \"seeAlso\": [\n        \"https://people.mpi-inf.mpg.de/~uwe/misc/uw-ttyp0/\"\n      ],\n      \"isOsiApproved\": false\n    },\n    {\n      \"reference\": \"https://spdx.org/licenses/TU-Berlin-1.0.html\",\n      \"isDeprecatedLicenseId\": false,\n      \"detailsUrl\": \"https://spdx.org/licenses/TU-Berlin-1.0.json\",\n      \"referenceNumber\": 167,\n      \"name\": \"Technische Universitaet Berlin License 1.0\",\n      \"licenseId\": \"TU-Berlin-1.0\",\n      \"seeAlso\": [\n        \"https://github.com/swh/ladspa/blob/7bf6f3799fdba70fda297c2d8fd9f526803d9680/gsm/COPYRIGHT\"\n      ],\n      \"isOsiApproved\": false\n    },\n    {\n      \"reference\": \"https://spdx.org/licenses/TU-Berlin-2.0.html\",\n      \"isDeprecatedLicenseId\": false,\n      \"detailsUrl\": \"https://spdx.org/licenses/TU-Berlin-2.0.json\",\n      \"referenceNumber\": 475,\n      \"name\": \"Technische Universitaet Berlin License 2.0\",\n      \"licenseId\": \"TU-Berlin-2.0\",\n      \"seeAlso\": [\n        \"https://github.com/CorsixTH/deps/blob/fd339a9f526d1d9c9f01ccf39e438a015da50035/licences/libgsm.txt\"\n      ],\n      \"isOsiApproved\": false\n    },\n    {\n      \"reference\": \"https://spdx.org/licenses/UCAR.html\",\n      \"isDeprecatedLicenseId\": false,\n      \"detailsUrl\": \"https://spdx.org/licenses/UCAR.json\",\n      \"referenceNumber\": 20,\n      \"name\": \"UCAR License\",\n      \"licenseId\": \"UCAR\",\n      \"seeAlso\": [\n        \"https://github.com/Unidata/UDUNITS-2/blob/master/COPYRIGHT\"\n      ],\n      \"isOsiApproved\": false\n    },\n    {\n      \"reference\": \"https://spdx.org/licenses/UCL-1.0.html\",\n      \"isDeprecatedLicenseId\": false,\n      \"detailsUrl\": \"https://spdx.org/licenses/UCL-1.0.json\",\n      \"referenceNumber\": 106,\n      \"name\": \"Upstream Compatibility License v1.0\",\n      \"licenseId\": \"UCL-1.0\",\n      \"seeAlso\": [\n        \"https://opensource.org/licenses/UCL-1.0\"\n      ],\n      \"isOsiApproved\": true\n    },\n    {\n      \"reference\": \"https://spdx.org/licenses/ulem.html\",\n      \"isDeprecatedLicenseId\": false,\n      \"detailsUrl\": \"https://spdx.org/licenses/ulem.json\",\n      \"referenceNumber\": 360,\n      \"name\": \"ulem License\",\n      \"licenseId\": \"ulem\",\n      \"seeAlso\": [\n        \"https://mirrors.ctan.org/macros/latex/contrib/ulem/README\"\n      ],\n      \"isOsiApproved\": false\n    },\n    {\n      \"reference\": \"https://spdx.org/licenses/UMich-Merit.html\",\n      \"isDeprecatedLicenseId\": false,\n      \"detailsUrl\": \"https://spdx.org/licenses/UMich-Merit.json\",\n      \"referenceNumber\": 274,\n      \"name\": \"Michigan/Merit Networks License\",\n      \"licenseId\": \"UMich-Merit\",\n      \"seeAlso\": [\n        \"https://github.com/radcli/radcli/blob/master/COPYRIGHT#L64\"\n      ],\n      \"isOsiApproved\": false\n    },\n    {\n      \"reference\": \"https://spdx.org/licenses/Unicode-3.0.html\",\n      \"isDeprecatedLicenseId\": false,\n      \"detailsUrl\": \"https://spdx.org/licenses/Unicode-3.0.json\",\n      \"referenceNumber\": 557,\n      \"name\": \"Unicode License v3\",\n      \"licenseId\": \"Unicode-3.0\",\n      \"seeAlso\": [\n        \"https://www.unicode.org/license.txt\"\n      ],\n      \"isOsiApproved\": true\n    },\n    {\n      \"reference\": \"https://spdx.org/licenses/Unicode-DFS-2015.html\",\n      \"isDeprecatedLicenseId\": false,\n      \"detailsUrl\": \"https://spdx.org/licenses/Unicode-DFS-2015.json\",\n      \"referenceNumber\": 202,\n      \"name\": \"Unicode License Agreement - Data Files and Software (2015)\",\n      \"licenseId\": \"Unicode-DFS-2015\",\n      \"seeAlso\": [\n        \"https://web.archive.org/web/20151224134844/http://unicode.org/copyright.html\"\n      ],\n      \"isOsiApproved\": false\n    },\n    {\n      \"reference\": \"https://spdx.org/licenses/Unicode-DFS-2016.html\",\n      \"isDeprecatedLicenseId\": false,\n      \"detailsUrl\": \"https://spdx.org/licenses/Unicode-DFS-2016.json\",\n      \"referenceNumber\": 410,\n      \"name\": \"Unicode License Agreement - Data Files and Software (2016)\",\n      \"licenseId\": \"Unicode-DFS-2016\",\n      \"seeAlso\": [\n        \"https://www.unicode.org/license.txt\",\n        \"http://web.archive.org/web/20160823201924/http://www.unicode.org/copyright.html#License\",\n        \"http://www.unicode.org/copyright.html\"\n      ],\n      \"isOsiApproved\": true\n    },\n    {\n      \"reference\": \"https://spdx.org/licenses/Unicode-TOU.html\",\n      \"isDeprecatedLicenseId\": false,\n      \"detailsUrl\": \"https://spdx.org/licenses/Unicode-TOU.json\",\n      \"referenceNumber\": 473,\n      \"name\": \"Unicode Terms of Use\",\n      \"licenseId\": \"Unicode-TOU\",\n      \"seeAlso\": [\n        \"http://web.archive.org/web/20140704074106/http://www.unicode.org/copyright.html\",\n        \"http://www.unicode.org/copyright.html\"\n      ],\n      \"isOsiApproved\": false\n    },\n    {\n      \"reference\": \"https://spdx.org/licenses/UnixCrypt.html\",\n      \"isDeprecatedLicenseId\": false,\n      \"detailsUrl\": \"https://spdx.org/licenses/UnixCrypt.json\",\n      \"referenceNumber\": 176,\n      \"name\": \"UnixCrypt License\",\n      \"licenseId\": \"UnixCrypt\",\n      \"seeAlso\": [\n        \"https://foss.heptapod.net/python-libs/passlib/-/blob/branch/stable/LICENSE#L70\",\n        \"https://opensource.apple.com/source/JBoss/JBoss-737/jboss-all/jetty/src/main/org/mortbay/util/UnixCrypt.java.auto.html\",\n        \"https://archive.eclipse.org/jetty/8.0.1.v20110908/xref/org/eclipse/jetty/http/security/UnixCrypt.html\"\n      ],\n      \"isOsiApproved\": false\n    },\n    {\n      \"reference\": \"https://spdx.org/licenses/Unlicense.html\",\n      \"isDeprecatedLicenseId\": false,\n      \"detailsUrl\": \"https://spdx.org/licenses/Unlicense.json\",\n      \"referenceNumber\": 364,\n      \"name\": \"The Unlicense\",\n      \"licenseId\": \"Unlicense\",\n      \"seeAlso\": [\n        \"https://unlicense.org/\"\n      ],\n      \"isOsiApproved\": true,\n      \"isFsfLibre\": true\n    },\n    {\n      \"reference\": \"https://spdx.org/licenses/UPL-1.0.html\",\n      \"isDeprecatedLicenseId\": false,\n      \"detailsUrl\": \"https://spdx.org/licenses/UPL-1.0.json\",\n      \"referenceNumber\": 384,\n      \"name\": \"Universal Permissive License v1.0\",\n      \"licenseId\": \"UPL-1.0\",\n      \"seeAlso\": [\n        \"https://opensource.org/licenses/UPL\"\n      ],\n      \"isOsiApproved\": true,\n      \"isFsfLibre\": true\n    },\n    {\n      \"reference\": \"https://spdx.org/licenses/URT-RLE.html\",\n      \"isDeprecatedLicenseId\": false,\n      \"detailsUrl\": \"https://spdx.org/licenses/URT-RLE.json\",\n      \"referenceNumber\": 185,\n      \"name\": \"Utah Raster Toolkit Run Length Encoded License\",\n      \"licenseId\": \"URT-RLE\",\n      \"seeAlso\": [\n        \"https://sourceforge.net/p/netpbm/code/HEAD/tree/super_stable/converter/other/pnmtorle.c\",\n        \"https://sourceforge.net/p/netpbm/code/HEAD/tree/super_stable/converter/other/rletopnm.c\"\n      ],\n      \"isOsiApproved\": false\n    },\n    {\n      \"reference\": \"https://spdx.org/licenses/Vim.html\",\n      \"isDeprecatedLicenseId\": false,\n      \"detailsUrl\": \"https://spdx.org/licenses/Vim.json\",\n      \"referenceNumber\": 432,\n      \"name\": \"Vim License\",\n      \"licenseId\": \"Vim\",\n      \"seeAlso\": [\n        \"http://vimdoc.sourceforge.net/htmldoc/uganda.html\"\n      ],\n      \"isOsiApproved\": false,\n      \"isFsfLibre\": true\n    },\n    {\n      \"reference\": \"https://spdx.org/licenses/VOSTROM.html\",\n      \"isDeprecatedLicenseId\": false,\n      \"detailsUrl\": \"https://spdx.org/licenses/VOSTROM.json\",\n      \"referenceNumber\": 528,\n      \"name\": \"VOSTROM Public License for Open Source\",\n      \"licenseId\": \"VOSTROM\",\n      \"seeAlso\": [\n        \"https://fedoraproject.org/wiki/Licensing/VOSTROM\"\n      ],\n      \"isOsiApproved\": false\n    },\n    {\n      \"reference\": \"https://spdx.org/licenses/VSL-1.0.html\",\n      \"isDeprecatedLicenseId\": false,\n      \"detailsUrl\": \"https://spdx.org/licenses/VSL-1.0.json\",\n      \"referenceNumber\": 567,\n      \"name\": \"Vovida Software License v1.0\",\n      \"licenseId\": \"VSL-1.0\",\n      \"seeAlso\": [\n        \"https://opensource.org/licenses/VSL-1.0\"\n      ],\n      \"isOsiApproved\": true\n    },\n    {\n      \"reference\": \"https://spdx.org/licenses/W3C.html\",\n      \"isDeprecatedLicenseId\": false,\n      \"detailsUrl\": \"https://spdx.org/licenses/W3C.json\",\n      \"referenceNumber\": 148,\n      \"name\": \"W3C Software Notice and License (2002-12-31)\",\n      \"licenseId\": \"W3C\",\n      \"seeAlso\": [\n        \"http://www.w3.org/Consortium/Legal/2002/copyright-software-20021231.html\",\n        \"https://opensource.org/licenses/W3C\"\n      ],\n      \"isOsiApproved\": true,\n      \"isFsfLibre\": true\n    },\n    {\n      \"reference\": \"https://spdx.org/licenses/W3C-19980720.html\",\n      \"isDeprecatedLicenseId\": false,\n      \"detailsUrl\": \"https://spdx.org/licenses/W3C-19980720.json\",\n      \"referenceNumber\": 403,\n      \"name\": \"W3C Software Notice and License (1998-07-20)\",\n      \"licenseId\": \"W3C-19980720\",\n      \"seeAlso\": [\n        \"http://www.w3.org/Consortium/Legal/copyright-software-19980720.html\"\n      ],\n      \"isOsiApproved\": false\n    },\n    {\n      \"reference\": \"https://spdx.org/licenses/W3C-20150513.html\",\n      \"isDeprecatedLicenseId\": false,\n      \"detailsUrl\": \"https://spdx.org/licenses/W3C-20150513.json\",\n      \"referenceNumber\": 344,\n      \"name\": \"W3C Software Notice and Document License (2015-05-13)\",\n      \"licenseId\": \"W3C-20150513\",\n      \"seeAlso\": [\n        \"https://www.w3.org/Consortium/Legal/2015/copyright-software-and-document\",\n        \"https://www.w3.org/copyright/software-license-2015/\",\n        \"https://www.w3.org/copyright/software-license-2023/\"\n      ],\n      \"isOsiApproved\": false\n    },\n    {\n      \"reference\": \"https://spdx.org/licenses/w3m.html\",\n      \"isDeprecatedLicenseId\": false,\n      \"detailsUrl\": \"https://spdx.org/licenses/w3m.json\",\n      \"referenceNumber\": 497,\n      \"name\": \"w3m License\",\n      \"licenseId\": \"w3m\",\n      \"seeAlso\": [\n        \"https://github.com/tats/w3m/blob/master/COPYING\"\n      ],\n      \"isOsiApproved\": false\n    },\n    {\n      \"reference\": \"https://spdx.org/licenses/Watcom-1.0.html\",\n      \"isDeprecatedLicenseId\": false,\n      \"detailsUrl\": \"https://spdx.org/licenses/Watcom-1.0.json\",\n      \"referenceNumber\": 38,\n      \"name\": \"Sybase Open Watcom Public License 1.0\",\n      \"licenseId\": \"Watcom-1.0\",\n      \"seeAlso\": [\n        \"https://opensource.org/licenses/Watcom-1.0\"\n      ],\n      \"isOsiApproved\": true,\n      \"isFsfLibre\": false\n    },\n    {\n      \"reference\": \"https://spdx.org/licenses/Widget-Workshop.html\",\n      \"isDeprecatedLicenseId\": false,\n      \"detailsUrl\": \"https://spdx.org/licenses/Widget-Workshop.json\",\n      \"referenceNumber\": 229,\n      \"name\": \"Widget Workshop License\",\n      \"licenseId\": \"Widget-Workshop\",\n      \"seeAlso\": [\n        \"https://github.com/novnc/noVNC/blob/master/core/crypto/des.js#L24\"\n      ],\n      \"isOsiApproved\": false\n    },\n    {\n      \"reference\": \"https://spdx.org/licenses/Wsuipa.html\",\n      \"isDeprecatedLicenseId\": false,\n      \"detailsUrl\": \"https://spdx.org/licenses/Wsuipa.json\",\n      \"referenceNumber\": 548,\n      \"name\": \"Wsuipa License\",\n      \"licenseId\": \"Wsuipa\",\n      \"seeAlso\": [\n        \"https://fedoraproject.org/wiki/Licensing/Wsuipa\"\n      ],\n      \"isOsiApproved\": false\n    },\n    {\n      \"reference\": \"https://spdx.org/licenses/WTFPL.html\",\n      \"isDeprecatedLicenseId\": false,\n      \"detailsUrl\": \"https://spdx.org/licenses/WTFPL.json\",\n      \"referenceNumber\": 289,\n      \"name\": \"Do What The F*ck You Want To Public License\",\n      \"licenseId\": \"WTFPL\",\n      \"seeAlso\": [\n        \"http://www.wtfpl.net/about/\",\n        \"http://sam.zoy.org/wtfpl/COPYING\"\n      ],\n      \"isOsiApproved\": false,\n      \"isFsfLibre\": true\n    },\n    {\n      \"reference\": \"https://spdx.org/licenses/wxWindows.html\",\n      \"isDeprecatedLicenseId\": true,\n      \"detailsUrl\": \"https://spdx.org/licenses/wxWindows.json\",\n      \"referenceNumber\": 338,\n      \"name\": \"wxWindows Library License\",\n      \"licenseId\": \"wxWindows\",\n      \"seeAlso\": [\n        \"https://opensource.org/licenses/WXwindows\"\n      ],\n      \"isOsiApproved\": true\n    },\n    {\n      \"reference\": \"https://spdx.org/licenses/X11.html\",\n      \"isDeprecatedLicenseId\": false,\n      \"detailsUrl\": \"https://spdx.org/licenses/X11.json\",\n      \"referenceNumber\": 449,\n      \"name\": \"X11 License\",\n      \"licenseId\": \"X11\",\n      \"seeAlso\": [\n        \"http://www.xfree86.org/3.3.6/COPYRIGHT2.html#3\"\n      ],\n      \"isOsiApproved\": false,\n      \"isFsfLibre\": true\n    },\n    {\n      \"reference\": \"https://spdx.org/licenses/X11-distribute-modifications-variant.html\",\n      \"isDeprecatedLicenseId\": false,\n      \"detailsUrl\": \"https://spdx.org/licenses/X11-distribute-modifications-variant.json\",\n      \"referenceNumber\": 587,\n      \"name\": \"X11 License Distribution Modification Variant\",\n      \"licenseId\": \"X11-distribute-modifications-variant\",\n      \"seeAlso\": [\n        \"https://github.com/mirror/ncurses/blob/master/COPYING\"\n      ],\n      \"isOsiApproved\": false\n    },\n    {\n      \"reference\": \"https://spdx.org/licenses/Xdebug-1.03.html\",\n      \"isDeprecatedLicenseId\": false,\n      \"detailsUrl\": \"https://spdx.org/licenses/Xdebug-1.03.json\",\n      \"referenceNumber\": 327,\n      \"name\": \"Xdebug License v 1.03\",\n      \"licenseId\": \"Xdebug-1.03\",\n      \"seeAlso\": [\n        \"https://github.com/xdebug/xdebug/blob/master/LICENSE\"\n      ],\n      \"isOsiApproved\": false\n    },\n    {\n      \"reference\": \"https://spdx.org/licenses/Xerox.html\",\n      \"isDeprecatedLicenseId\": false,\n      \"detailsUrl\": \"https://spdx.org/licenses/Xerox.json\",\n      \"referenceNumber\": 204,\n      \"name\": \"Xerox License\",\n      \"licenseId\": \"Xerox\",\n      \"seeAlso\": [\n        \"https://fedoraproject.org/wiki/Licensing/Xerox\"\n      ],\n      \"isOsiApproved\": false\n    },\n    {\n      \"reference\": \"https://spdx.org/licenses/Xfig.html\",\n      \"isDeprecatedLicenseId\": false,\n      \"detailsUrl\": \"https://spdx.org/licenses/Xfig.json\",\n      \"referenceNumber\": 175,\n      \"name\": \"Xfig License\",\n      \"licenseId\": \"Xfig\",\n      \"seeAlso\": [\n        \"https://github.com/Distrotech/transfig/blob/master/transfig/transfig.c\",\n        \"https://fedoraproject.org/wiki/Licensing:MIT#Xfig_Variant\",\n        \"https://sourceforge.net/p/mcj/xfig/ci/master/tree/src/Makefile.am\"\n      ],\n      \"isOsiApproved\": false\n    },\n    {\n      \"reference\": \"https://spdx.org/licenses/XFree86-1.1.html\",\n      \"isDeprecatedLicenseId\": false,\n      \"detailsUrl\": \"https://spdx.org/licenses/XFree86-1.1.json\",\n      \"referenceNumber\": 542,\n      \"name\": \"XFree86 License 1.1\",\n      \"licenseId\": \"XFree86-1.1\",\n      \"seeAlso\": [\n        \"http://www.xfree86.org/current/LICENSE4.html\"\n      ],\n      \"isOsiApproved\": false,\n      \"isFsfLibre\": true\n    },\n    {\n      \"reference\": \"https://spdx.org/licenses/xinetd.html\",\n      \"isDeprecatedLicenseId\": false,\n      \"detailsUrl\": \"https://spdx.org/licenses/xinetd.json\",\n      \"referenceNumber\": 596,\n      \"name\": \"xinetd License\",\n      \"licenseId\": \"xinetd\",\n      \"seeAlso\": [\n        \"https://fedoraproject.org/wiki/Licensing/Xinetd_License\"\n      ],\n      \"isOsiApproved\": false,\n      \"isFsfLibre\": true\n    },\n    {\n      \"reference\": \"https://spdx.org/licenses/xkeyboard-config-Zinoviev.html\",\n      \"isDeprecatedLicenseId\": false,\n      \"detailsUrl\": \"https://spdx.org/licenses/xkeyboard-config-Zinoviev.json\",\n      \"referenceNumber\": 413,\n      \"name\": \"xkeyboard-config Zinoviev License\",\n      \"licenseId\": \"xkeyboard-config-Zinoviev\",\n      \"seeAlso\": [\n        \"https://gitlab.freedesktop.org/xkeyboard-config/xkeyboard-config/-/blob/master/COPYING?ref_type\\u003dheads#L178\"\n      ],\n      \"isOsiApproved\": false\n    },\n    {\n      \"reference\": \"https://spdx.org/licenses/xlock.html\",\n      \"isDeprecatedLicenseId\": false,\n      \"detailsUrl\": \"https://spdx.org/licenses/xlock.json\",\n      \"referenceNumber\": 606,\n      \"name\": \"xlock License\",\n      \"licenseId\": \"xlock\",\n      \"seeAlso\": [\n        \"https://fossies.org/linux/tiff/contrib/ras/ras2tif.c\"\n      ],\n      \"isOsiApproved\": false\n    },\n    {\n      \"reference\": \"https://spdx.org/licenses/Xnet.html\",\n      \"isDeprecatedLicenseId\": false,\n      \"detailsUrl\": \"https://spdx.org/licenses/Xnet.json\",\n      \"referenceNumber\": 191,\n      \"name\": \"X.Net License\",\n      \"licenseId\": \"Xnet\",\n      \"seeAlso\": [\n        \"https://opensource.org/licenses/Xnet\"\n      ],\n      \"isOsiApproved\": true\n    },\n    {\n      \"reference\": \"https://spdx.org/licenses/xpp.html\",\n      \"isDeprecatedLicenseId\": false,\n      \"detailsUrl\": \"https://spdx.org/licenses/xpp.json\",\n      \"referenceNumber\": 492,\n      \"name\": \"XPP License\",\n      \"licenseId\": \"xpp\",\n      \"seeAlso\": [\n        \"https://fedoraproject.org/wiki/Licensing/xpp\"\n      ],\n      \"isOsiApproved\": false\n    },\n    {\n      \"reference\": \"https://spdx.org/licenses/XSkat.html\",\n      \"isDeprecatedLicenseId\": false,\n      \"detailsUrl\": \"https://spdx.org/licenses/XSkat.json\",\n      \"referenceNumber\": 129,\n      \"name\": \"XSkat License\",\n      \"licenseId\": \"XSkat\",\n      \"seeAlso\": [\n        \"https://fedoraproject.org/wiki/Licensing/XSkat_License\"\n      ],\n      \"isOsiApproved\": false\n    },\n    {\n      \"reference\": \"https://spdx.org/licenses/xzoom.html\",\n      \"isDeprecatedLicenseId\": false,\n      \"detailsUrl\": \"https://spdx.org/licenses/xzoom.json\",\n      \"referenceNumber\": 520,\n      \"name\": \"xzoom License\",\n      \"licenseId\": \"xzoom\",\n      \"seeAlso\": [\n        \"https://metadata.ftp-master.debian.org/changelogs//main/x/xzoom/xzoom_0.3-27_copyright\"\n      ],\n      \"isOsiApproved\": false\n    },\n    {\n      \"reference\": \"https://spdx.org/licenses/YPL-1.0.html\",\n      \"isDeprecatedLicenseId\": false,\n      \"detailsUrl\": \"https://spdx.org/licenses/YPL-1.0.json\",\n      \"referenceNumber\": 34,\n      \"name\": \"Yahoo! Public License v1.0\",\n      \"licenseId\": \"YPL-1.0\",\n      \"seeAlso\": [\n        \"http://www.zimbra.com/license/yahoo_public_license_1.0.html\"\n      ],\n      \"isOsiApproved\": false\n    },\n    {\n      \"reference\": \"https://spdx.org/licenses/YPL-1.1.html\",\n      \"isDeprecatedLicenseId\": false,\n      \"detailsUrl\": \"https://spdx.org/licenses/YPL-1.1.json\",\n      \"referenceNumber\": 300,\n      \"name\": \"Yahoo! Public License v1.1\",\n      \"licenseId\": \"YPL-1.1\",\n      \"seeAlso\": [\n        \"http://www.zimbra.com/license/yahoo_public_license_1.1.html\"\n      ],\n      \"isOsiApproved\": false,\n      \"isFsfLibre\": true\n    },\n    {\n      \"reference\": \"https://spdx.org/licenses/Zed.html\",\n      \"isDeprecatedLicenseId\": false,\n      \"detailsUrl\": \"https://spdx.org/licenses/Zed.json\",\n      \"referenceNumber\": 79,\n      \"name\": \"Zed License\",\n      \"licenseId\": \"Zed\",\n      \"seeAlso\": [\n        \"https://fedoraproject.org/wiki/Licensing/Zed\"\n      ],\n      \"isOsiApproved\": false\n    },\n    {\n      \"reference\": \"https://spdx.org/licenses/Zeeff.html\",\n      \"isDeprecatedLicenseId\": false,\n      \"detailsUrl\": \"https://spdx.org/licenses/Zeeff.json\",\n      \"referenceNumber\": 386,\n      \"name\": \"Zeeff License\",\n      \"licenseId\": \"Zeeff\",\n      \"seeAlso\": [\n        \"ftp://ftp.tin.org/pub/news/utils/newsx/newsx-1.6.tar.gz\"\n      ],\n      \"isOsiApproved\": false\n    },\n    {\n      \"reference\": \"https://spdx.org/licenses/Zend-2.0.html\",\n      \"isDeprecatedLicenseId\": false,\n      \"detailsUrl\": \"https://spdx.org/licenses/Zend-2.0.json\",\n      \"referenceNumber\": 50,\n      \"name\": \"Zend License v2.0\",\n      \"licenseId\": \"Zend-2.0\",\n      \"seeAlso\": [\n        \"https://web.archive.org/web/20130517195954/http://www.zend.com/license/2_00.txt\"\n      ],\n      \"isOsiApproved\": false,\n      \"isFsfLibre\": true\n    },\n    {\n      \"reference\": \"https://spdx.org/licenses/Zimbra-1.3.html\",\n      \"isDeprecatedLicenseId\": false,\n      \"detailsUrl\": \"https://spdx.org/licenses/Zimbra-1.3.json\",\n      \"referenceNumber\": 265,\n      \"name\": \"Zimbra Public License v1.3\",\n      \"licenseId\": \"Zimbra-1.3\",\n      \"seeAlso\": [\n        \"http://web.archive.org/web/20100302225219/http://www.zimbra.com/license/zimbra-public-license-1-3.html\"\n      ],\n      \"isOsiApproved\": false,\n      \"isFsfLibre\": true\n    },\n    {\n      \"reference\": \"https://spdx.org/licenses/Zimbra-1.4.html\",\n      \"isDeprecatedLicenseId\": false,\n      \"detailsUrl\": \"https://spdx.org/licenses/Zimbra-1.4.json\",\n      \"referenceNumber\": 100,\n      \"name\": \"Zimbra Public License v1.4\",\n      \"licenseId\": \"Zimbra-1.4\",\n      \"seeAlso\": [\n        \"http://www.zimbra.com/legal/zimbra-public-license-1-4\"\n      ],\n      \"isOsiApproved\": false\n    },\n    {\n      \"reference\": \"https://spdx.org/licenses/Zlib.html\",\n      \"isDeprecatedLicenseId\": false,\n      \"detailsUrl\": \"https://spdx.org/licenses/Zlib.json\",\n      \"referenceNumber\": 131,\n      \"name\": \"zlib License\",\n      \"licenseId\": \"Zlib\",\n      \"seeAlso\": [\n        \"http://www.zlib.net/zlib_license.html\",\n        \"https://opensource.org/licenses/Zlib\"\n      ],\n      \"isOsiApproved\": true,\n      \"isFsfLibre\": true\n    },\n    {\n      \"reference\": \"https://spdx.org/licenses/zlib-acknowledgement.html\",\n      \"isDeprecatedLicenseId\": false,\n      \"detailsUrl\": \"https://spdx.org/licenses/zlib-acknowledgement.json\",\n      \"referenceNumber\": 642,\n      \"name\": \"zlib/libpng License with Acknowledgement\",\n      \"licenseId\": \"zlib-acknowledgement\",\n      \"seeAlso\": [\n        \"https://fedoraproject.org/wiki/Licensing/ZlibWithAcknowledgement\"\n      ],\n      \"isOsiApproved\": false\n    },\n    {\n      \"reference\": \"https://spdx.org/licenses/ZPL-1.1.html\",\n      \"isDeprecatedLicenseId\": false,\n      \"detailsUrl\": \"https://spdx.org/licenses/ZPL-1.1.json\",\n      \"referenceNumber\": 575,\n      \"name\": \"Zope Public License 1.1\",\n      \"licenseId\": \"ZPL-1.1\",\n      \"seeAlso\": [\n        \"http://old.zope.org/Resources/License/ZPL-1.1\"\n      ],\n      \"isOsiApproved\": false\n    },\n    {\n      \"reference\": \"https://spdx.org/licenses/ZPL-2.0.html\",\n      \"isDeprecatedLicenseId\": false,\n      \"detailsUrl\": \"https://spdx.org/licenses/ZPL-2.0.json\",\n      \"referenceNumber\": 412,\n      \"name\": \"Zope Public License 2.0\",\n      \"licenseId\": \"ZPL-2.0\",\n      \"seeAlso\": [\n        \"http://old.zope.org/Resources/License/ZPL-2.0\",\n        \"https://opensource.org/licenses/ZPL-2.0\"\n      ],\n      \"isOsiApproved\": true,\n      \"isFsfLibre\": true\n    },\n    {\n      \"reference\": \"https://spdx.org/licenses/ZPL-2.1.html\",\n      \"isDeprecatedLicenseId\": false,\n      \"detailsUrl\": \"https://spdx.org/licenses/ZPL-2.1.json\",\n      \"referenceNumber\": 82,\n      \"name\": \"Zope Public License 2.1\",\n      \"licenseId\": \"ZPL-2.1\",\n      \"seeAlso\": [\n        \"http://old.zope.org/Resources/ZPL/\"\n      ],\n      \"isOsiApproved\": true,\n      \"isFsfLibre\": true\n    }\n  ],\n  \"releaseDate\": \"2024-06-28\"\n}"  # b5a3b2e 28/06/2024
  # "https://github.com/spdx/license-list-data/blob/41edd7ee3a28604391226c7472299c7f600c6cae/json/licenses.json"
  n1 = Empty String/Path?(string/path="VIP License Type in") -> (empty?=w6:bool)
  n2 = case shown="False" w6 {
    tunnel: [w12 refnum<class "CycloneDX License.lvclass">[] []] -> w8
    tunnel: "VIP License Type in" -> [w14 _]
    tunnel: [w25 w69] -> w5
    tunnel: "SPDX License List (JSON) (\"\" = use built-in)" -> [w24 _]
    tunnel: "error in (no error)" -> [w23 w69]
    tunnel: w2 -> [w21 _]
    tunnel: "Additional Custom Aliases (empty = defaults only)" -> [w11 _]
    frame False {
      n3 = call "Default VIP Aliases.vi"() -> ("Custom Aliases (empty = defaults only)"=w9:T1[])  [unwired: 11 in]
      n4 = Empty String/Path?(string/path=w24) -> (empty?=w22:bool)
      n5 = Build Array (concatenate)(w9, w11) -> (w10:T1[])
      n6 = case shown="False" w22 {
        tunnel: w24 -> [w36 _]
        tunnel: w23 -> [w35 w38]
        tunnel: w21 -> [_ w37]
        tunnel: [w34 w37] -> w18
        tunnel: [w33 w38] -> w20
        frame False {
          n7 = Read from Text File(file (use dialog)=w36, error in=w35) -> (text=w34:string, error out=w33:errorcluster)  [unwired: 2 in, 2 out]
        }
        frame True {
        }
      }
      n8 = for {
        tunnel: w10 -> [w32] mode=indexing
        tunnel: w14 -> [w30]
        tunnel: [w27] -> w13 mode=concatenating if=w26
        n9 = Unbundle By Name(w32) -> ("SPDX IDs"=w27:string[], "VIP String"=w31:string)
        n10 = To Lower Case(string=w31) -> (all lower case string=w29:string)
        n11 = To Lower Case(string=w30) -> (all lower case string=w28:string)
        n12 = Equal?(x=w29, y=w28) -> (x = y?=w26:bool)
      }
      n13 = call "Find Item (as LVtype).vim"("$Path or Item Name"="$.licenses", "error in (no error)"=w20, "Data Type and Default Value"=cluster{"licenseId":string, "name":string}[] [], "JSON"=w18) -> ("error out"=w16:errorcluster, "Data"=w17:cluster{"licenseId":string, "name":string}[])  [unwired: 4 in, 2 out]
      n14 = for {
        tunnel: w17 -> [w44]
        tunnel: w13 -> [w40] mode=indexing
        shift-right: [w45] -> w25
        shift-left: w16 -> [w42]
        tunnel: [w39] -> w12 mode=indexing
        n15 = for {
          tunnel: w44 -> [w47] mode=indexing
          tunnel: w40 -> [w52]
          tunnel: [w46] -> w43
          tunnel: [w47] -> w41
          stop <- w46 stop-if-true
          n16 = Unbundle By Name(w47) -> ("licenseId"=w55:string, "name"=w53:string)
          n17 = To Lower Case(string=w52) -> (all lower case string=w49:string)
          n18 = To Lower Case(string=w55) -> (all lower case string=w51:string)
          n19 = To Lower Case(string=w53) -> (all lower case string=w50:string)
          n20 = Equal?(x=w49, y=w51) -> (x = y?=w54:bool)
          n21 = Equal?(x=w49, y=w50) -> (x = y?=w48:bool)
          n22 = Or(x=w54, y=w48) -> (x .or. y?=w46:bool)
        }
        n23 = case shown="True" w43 {
          tunnel: [w59 w64] -> w39
          tunnel: [w58 w65] -> w45
          tunnel: w40 -> [w57 _]
          tunnel: w42 -> [w56 w68]
          tunnel: w41 -> [_ w63]
          frame False {
            n24 = call "New License by Name.vi"("error in (no error)"=w56, "License Name"=w57) -> ("error out"=w58:errorcluster, "CycloneDX License out"=w59:refnum<class "CycloneDX License.lvclass">)  [unwired: 8 in]
          }
          frame True {
            n25 = Unbundle By Name(w63) -> ("licenseId"=w62:string, "name"=w61:string)
            n26 = call "New License by SPDX ID.vi"("error in (no error)"=w68, "SPDX License ID"=w62) -> ("error out"=w66:errorcluster, "CycloneDX License out"=w67:refnum<class "CycloneDX License.lvclass">)  [unwired: 8 in]
            n27 = call "Set Item (Anything).vi"("error in (no error)"=w66, "Value"=w61, "Object (or Item) Path"="name", "CycloneDX SBOM in"=w67) -> ("error out"=w65:errorcluster, "CycloneDX SBOM out"=w64:refnum<class "CycloneDX License.lvclass">)  [unwired: 6 in]
          }
        }
      }
    }
    frame True {
    }
  }
  "License(s) out" <- w8
  "error out" <- w5
